vi "Clock.vi"() -> ()   [LabVIEW 2021]
doc: "Clock ver. 1 by 113550153. \nAll right reserved."
uses:
  <vilib>/sound2/lvsound2.llb/Sound Data Format.ctl
  <vilib>/sound2/lvsound2.llb/Sound File Position.ctl
  <vilib>/sound2/lvsound2.llb/Sound Output Write (DBL).vi
  <vilib>/sound2/lvsound2.llb/Sound File Read (DBL).vi
  <vilib>/sound2/lvsound2.llb/Sound File Read Open.vi
panel:
  in  "12/24":bool
  in  "Sample No. x":i32
  out "Sound playing":bool
  in  "Reset button 2":bool
  out "Chronograph":bool
  in  "Notice Content":string
  in  "Voice File":path
  in  "Alarm clock":dbl(knob) scale=0.0..12.0
  in  "Record Button":bool
  in  "GO Button":bool
  in  "Alarm clock mode\nVoice--Screen Notice":bool
  in  "Alarm clock\nOff--On":bool
  in  "Second":i32(knob) scale=0.0..59.0
  in  "Minute":i32(knob) scale=0.0..59.0
  in  "Hour":i32(knob) scale=0.0..23.0
  in  "Reset button":bool
  in  "Mode button":bool
  out "2D Picture":picture
  in  "stop":bool
  # "由於程式稍大，按下開始當下可能會略卡幾秒鐘(Labview啟動)，請見諒~\n使用說明:\n1. Mode Change按鍵: 按下後依次切換顯示的功能 (手錶->時間設定->鬧鐘設定->碼表模式)\n    手錶: 三個指針由長到短分別顯示秒針、分針、時針，第四個短指針則是鬧鐘時間\n    時間設定: 按下Reset後會設定為當下指針所顯示的時間，可用旋鈕調整三個指針\n    鬧鐘設定: 透過旋鈕按鍵調整鬧鐘時間，依照傳統鬧鐘顯示標準(時針制，不分AM/PM)，且\n                    可調整鬧鐘提醒模式、聲音檔案或文字提示內容，可用\"鬧鐘開關\"關閉聲音提醒\n    碼表模式: 按下GO後開始執行，按下Record則會顯示按下當下的秒數 (碼表會繼續跑) (參考\n                    短跑比賽碼表設計)，再按一次則會跳回目前秒數，Reset碼表歸零\n2. 顯示說明(七位顯示器與觀景窗): 依照當前的模式顯示內容\n    手錶: 顯示目前時間\n    時間設定: 顯示目前欲設定的時間\n    鬧鐘設定: 顯示目前欲設定的鬧鐘時間\n    碼表模式: 顯示目前秒數，若按下Record則顯示按下當下的秒數\n    觀景窗: 根據七位顯示器的時間顯示其對應的天色狀況\n3. 可透過按鍵切換24/12時制顯示"
  # "目前模式:"
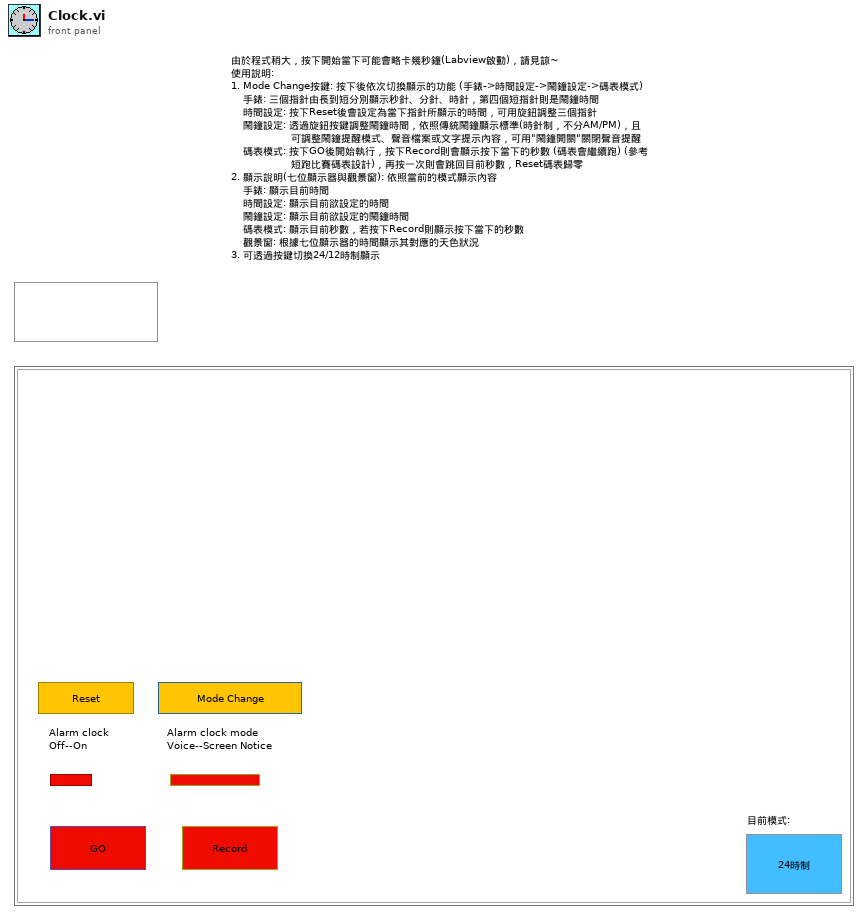
[diagram p1: front panel]
types:
  T1 = cluster{"Width":u16, "Style":enum32{"Solid", "Dash", "Dot", "DashDot", "DashDotDot"}}
  T2 = cluster{"left":i16, "top":i16, "right":i16, "bottom":i16}
  T3 = cluster{"Width":i16, "Style":enum32{"Solid", "Dash", "Dot", "DashDot", "DashDotDot"}}
  T4 = typedef "Sound Data Format.ctl" = cluster{"sample rate (S/s)":dbl, "number of channels":i32, "bits per sample":i32}
  T5 = typedef "Sound Output Task ID.ctl" = u32
  T6 = typedef "LVDateTimeRec.ctl" = cluster{"fractional second":dbl, "second":i32, "minute":i32, "hour":i32, "day of month":i32, "month":i32, "year":i32, "day of week":i32, "day of year":i32, "DST":i32}
  T7 = typedef "Sound File Position.ctl" = u16
  T8 = typedef "Sound File Refnum.ctl" = refnum<file>
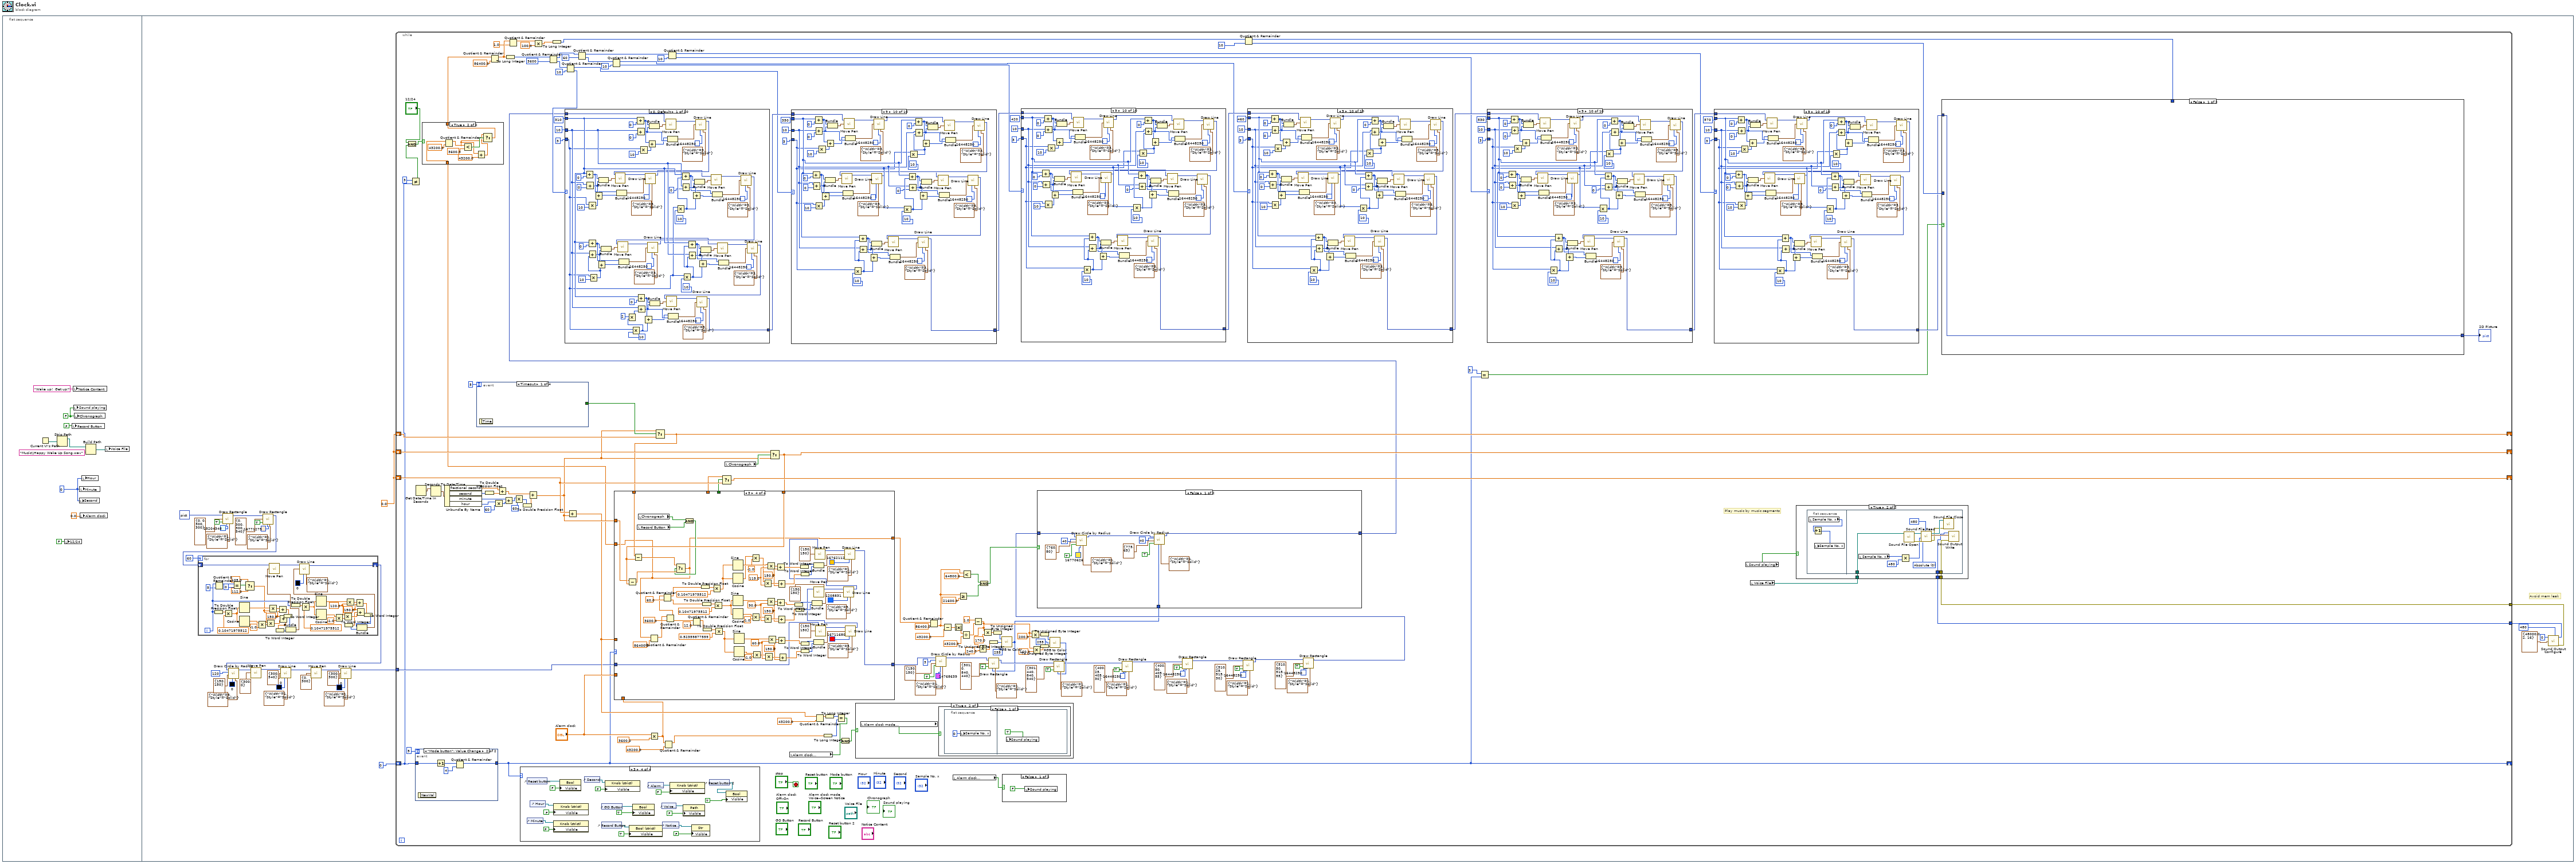
[diagram p0: block diagram]
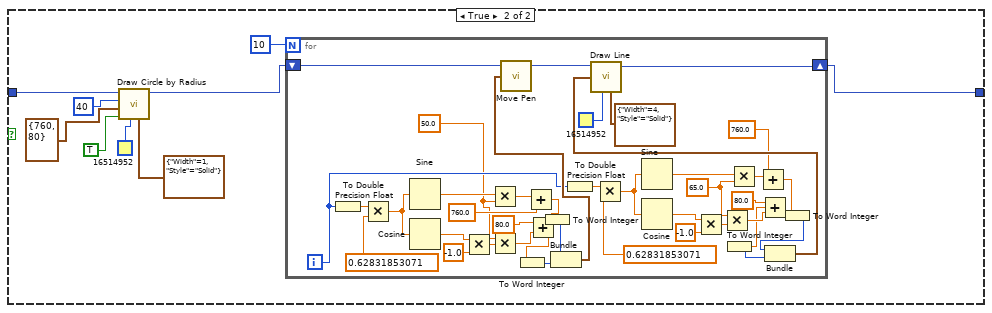
[diagram p2: hidden frame]
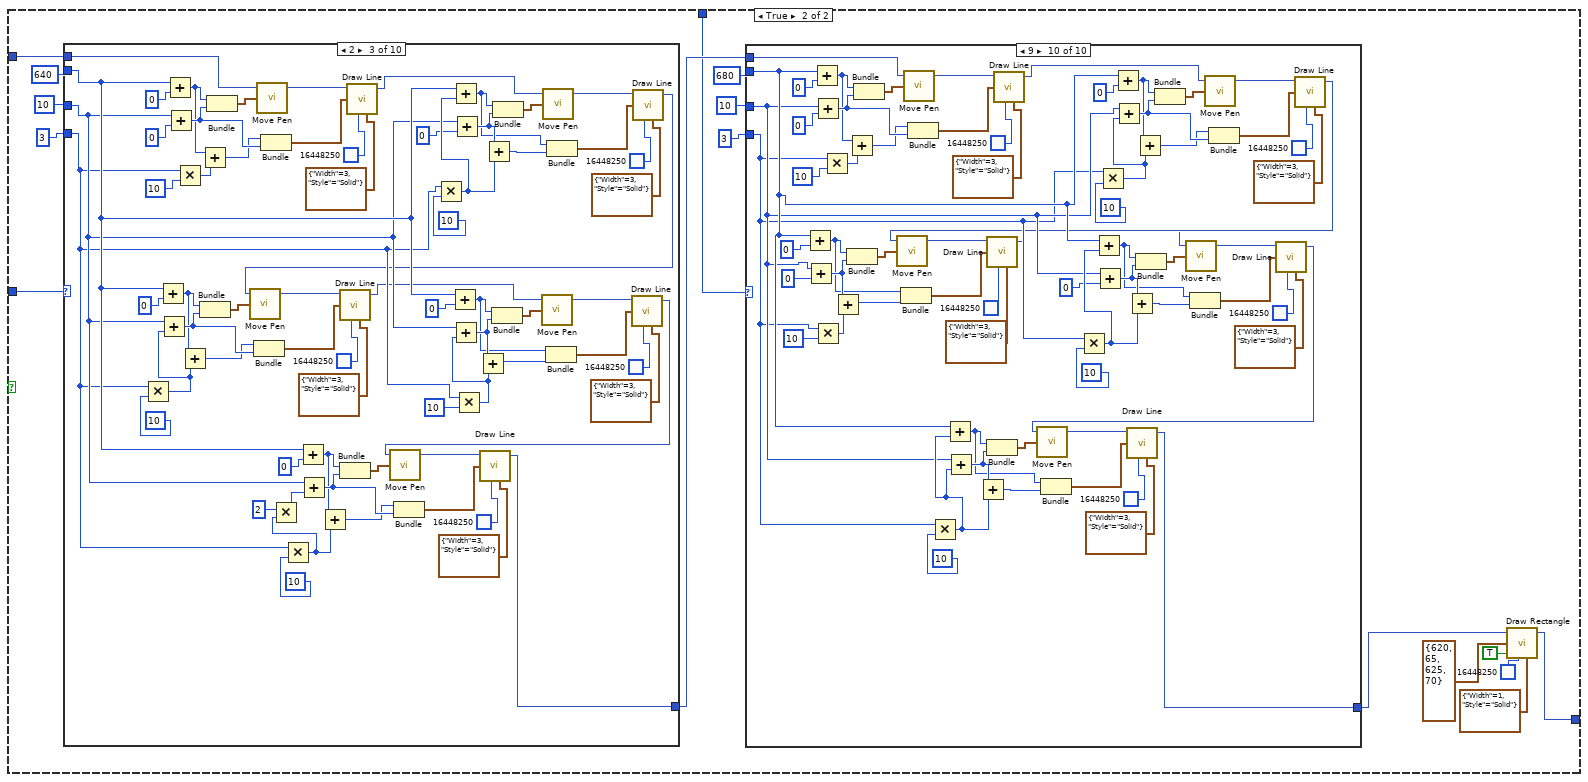
[diagram p4: hidden frame]
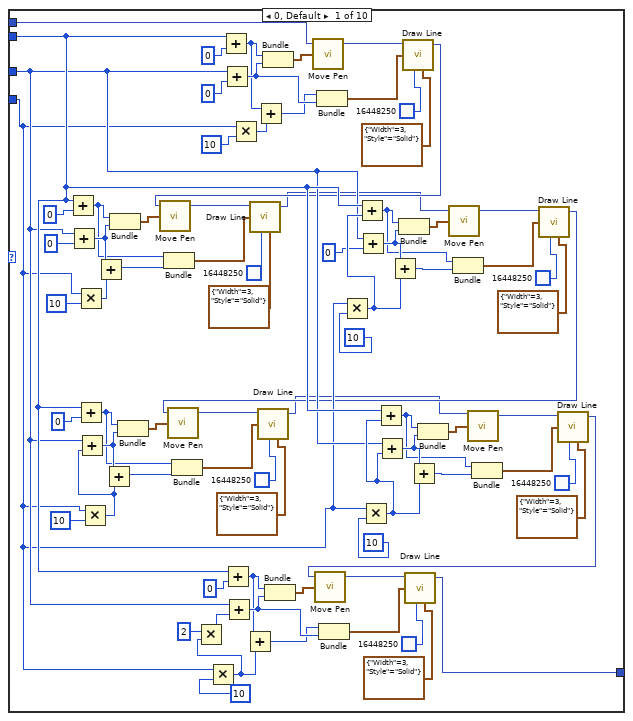
[diagram p5: hidden frame]
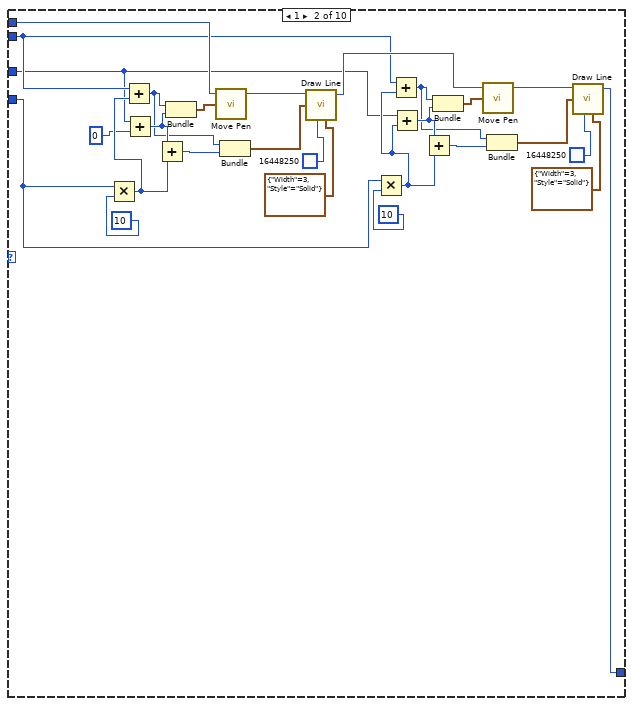
[diagram p6: hidden frame]
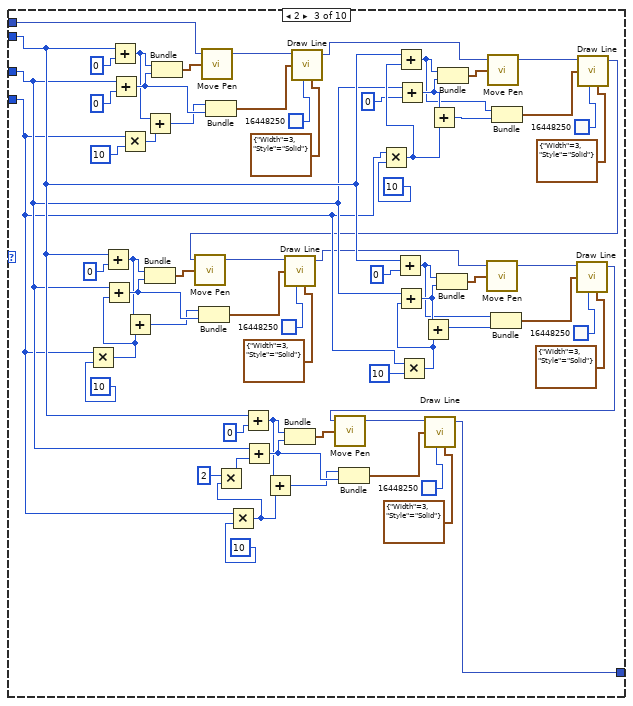
[diagram p7: hidden frame]
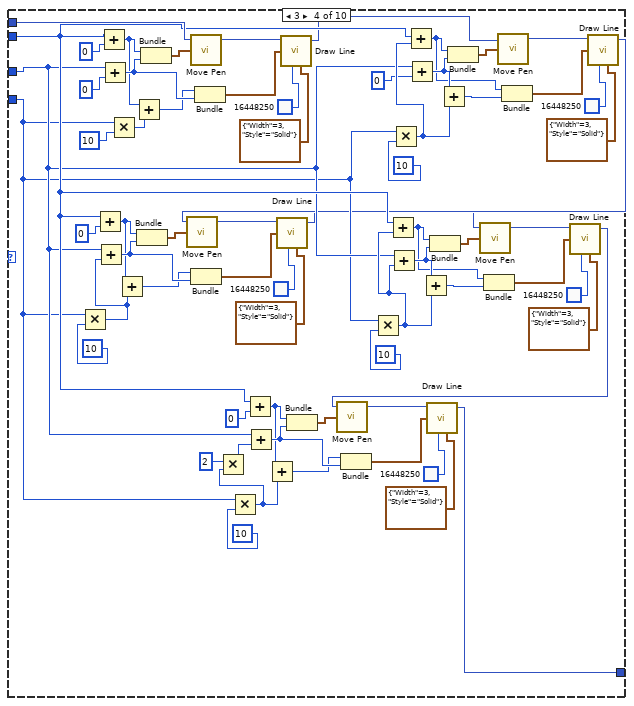
[diagram p8: hidden frame]
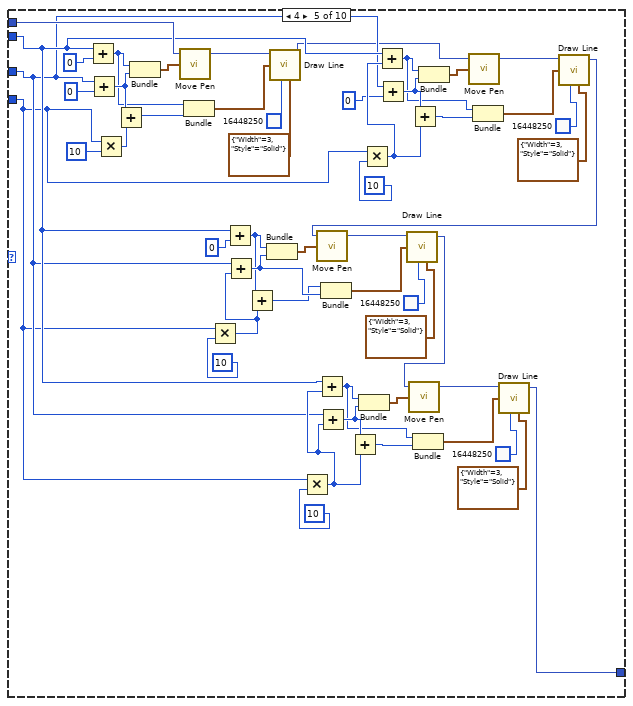
[diagram p9: hidden frame]
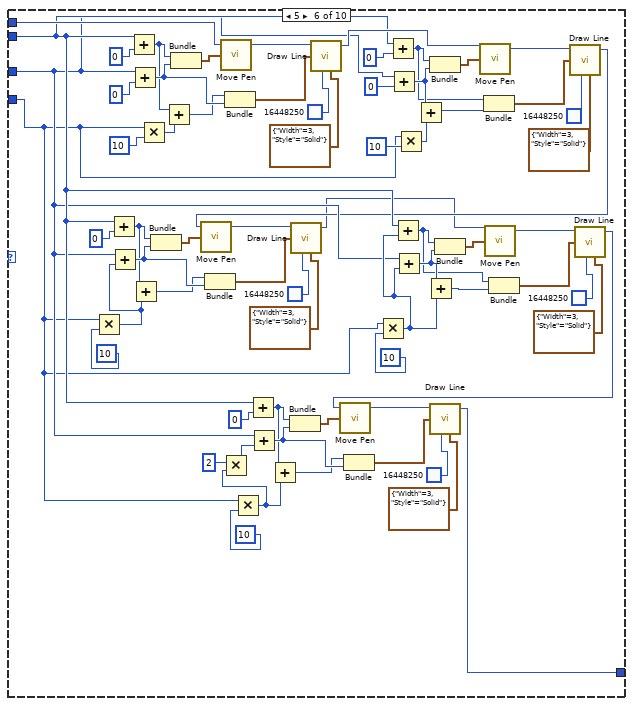
[diagram p10: hidden frame]
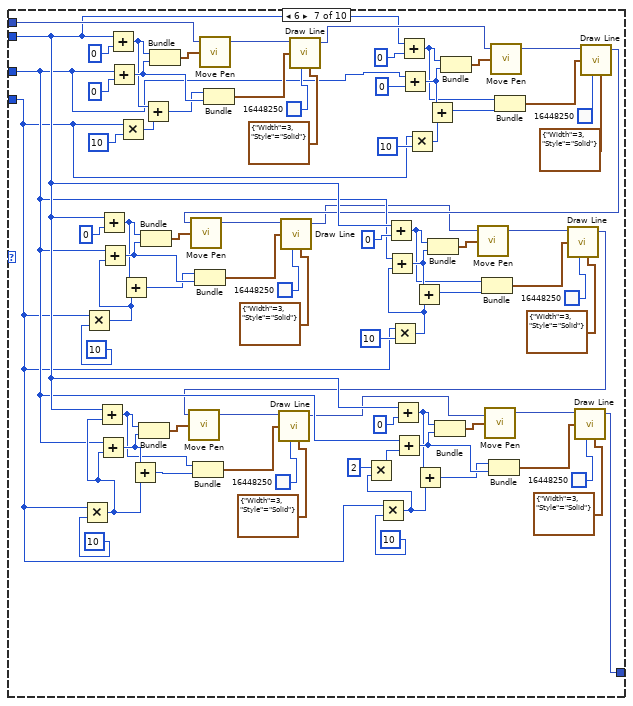
[diagram p11: hidden frame]
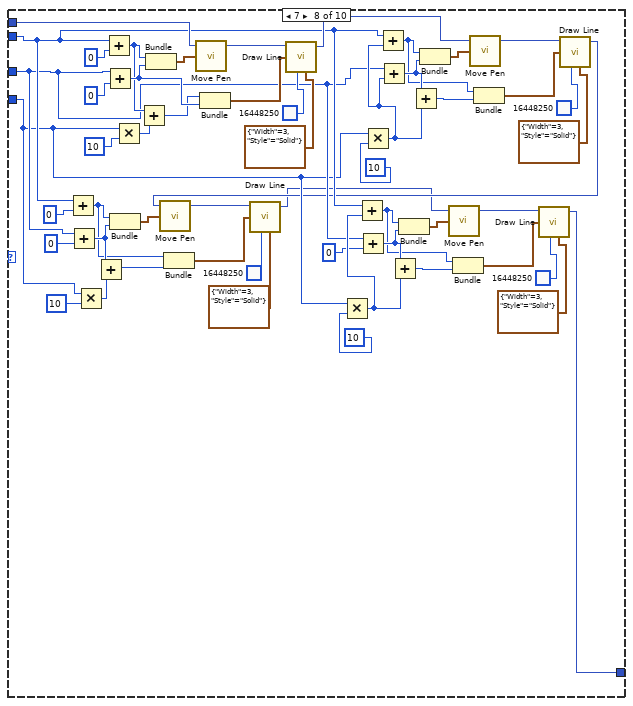
[diagram p12: hidden frame]
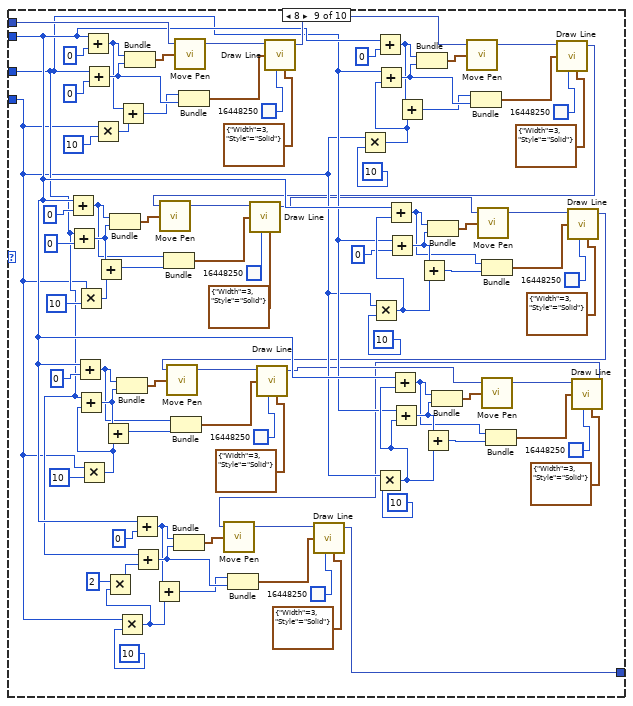
[diagram p13: hidden frame]
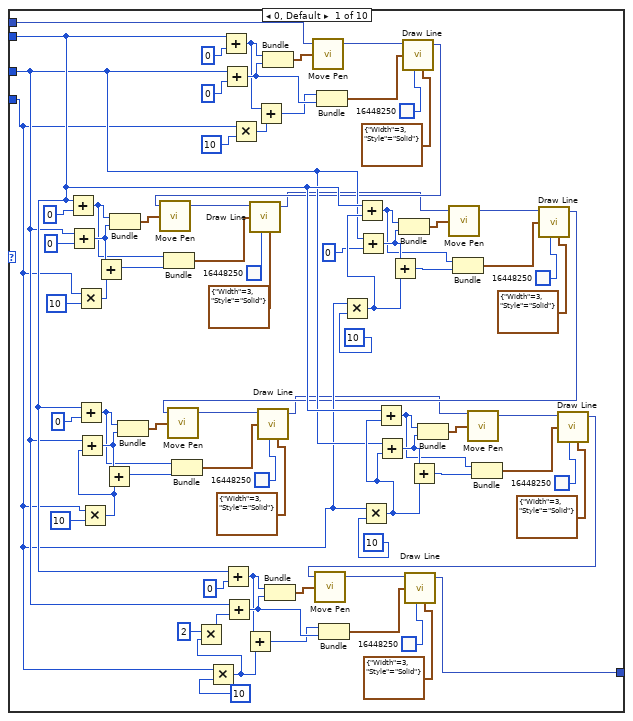
[diagram p14: hidden frame]
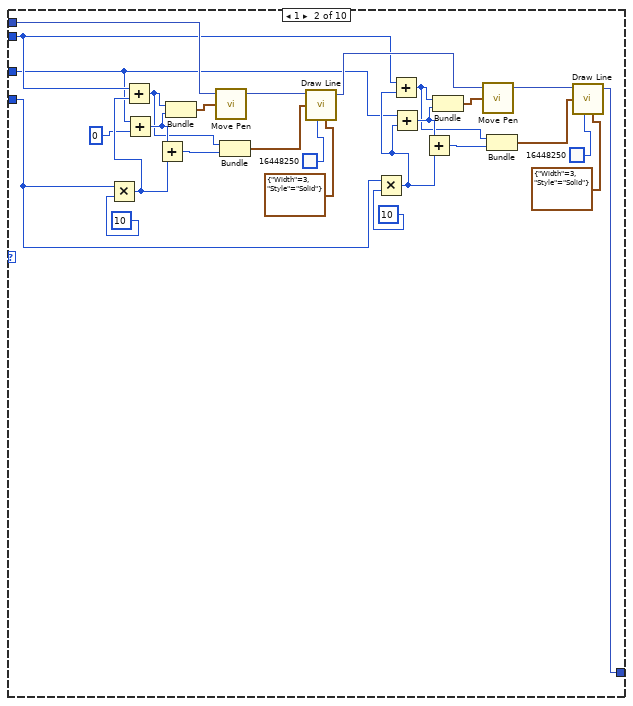
[diagram p15: hidden frame]
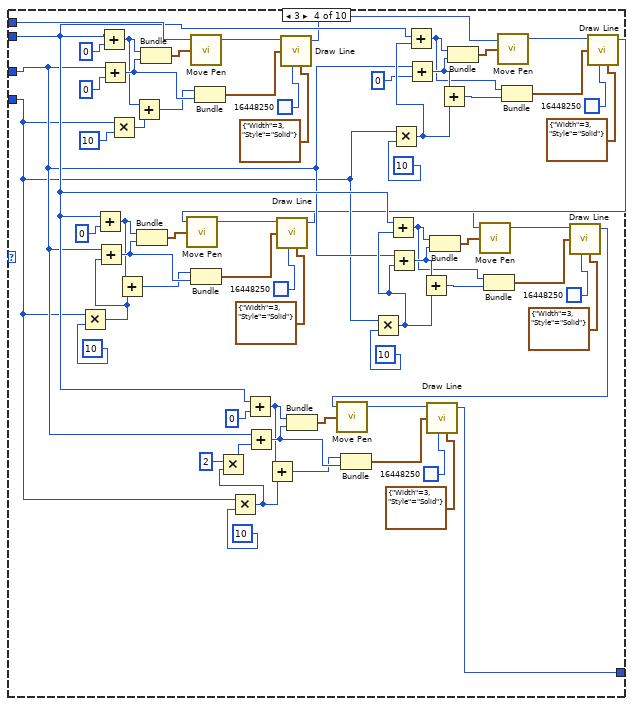
[diagram p16: hidden frame]
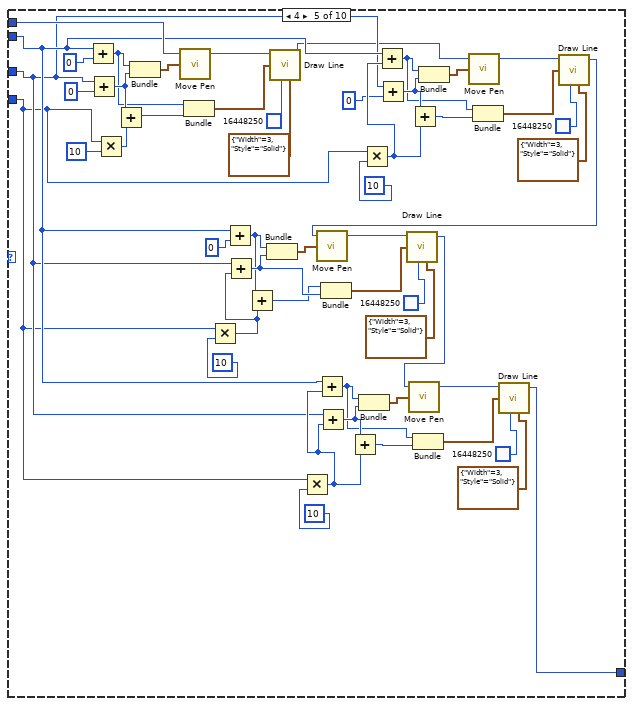
[diagram p17: hidden frame]
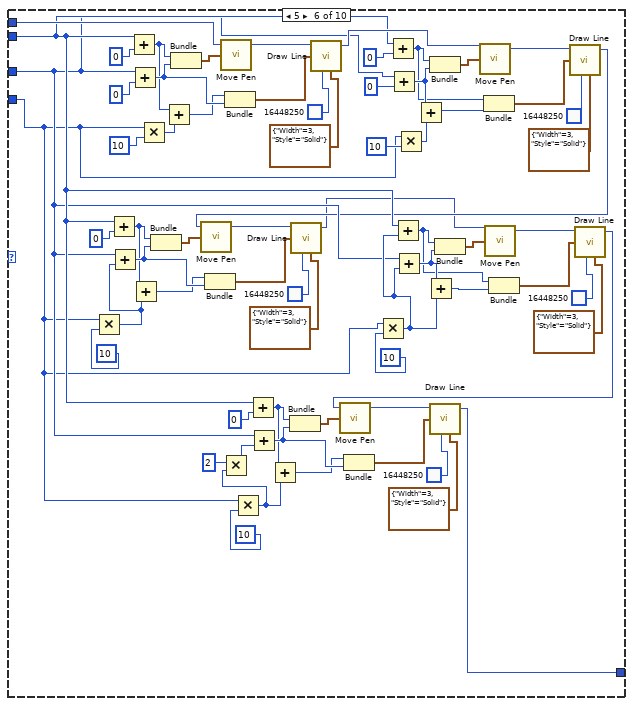
[diagram p18: hidden frame]
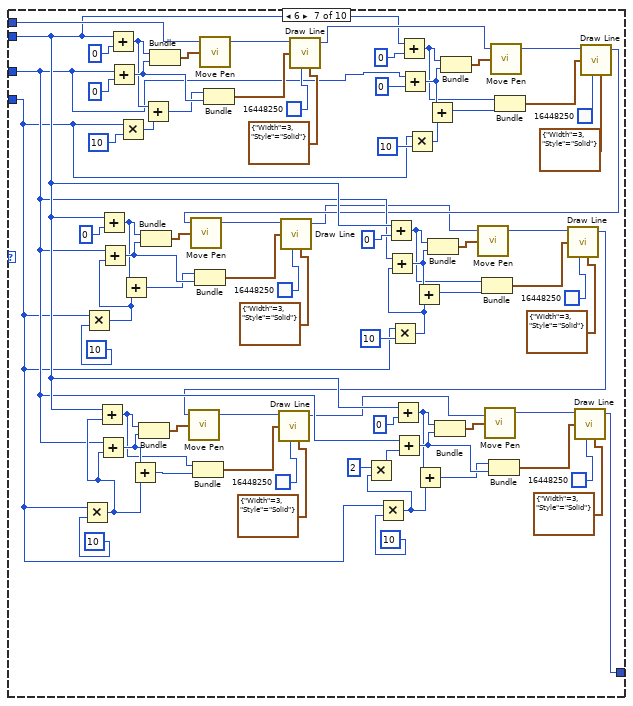
[diagram p19: hidden frame]
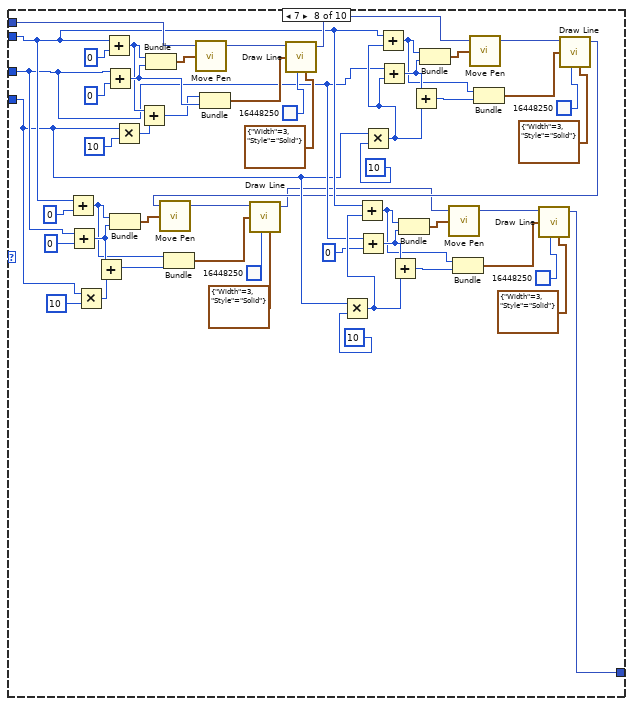
[diagram p20: hidden frame]
diagram:
  n1 = flat-sequence {
    frame #0 {
      w3 = 0
      w10 = FALSE
      n2 = Current VI's Path() -> (path=w8:path)
      n3 = Strip Path(path=w8) -> (stripped path=w7:path)  [unwired: 1 out]
      n4 = local write "12/24"(FALSE ("12/24")) -> ()
      n5 = local write "Record Button"(FALSE ("Record Button")) -> ()
      n6 = local write "Notice Content"("Wake up!  Get up!" ("Notice Content")) -> ()
      n7 = local write "Sound playing"(w10) -> ()
      n8 = local write "Chronograph"(w10) -> ()
      n9 = local write "Second"(w3) -> ()
      n10 = local write "Minute"(w3) -> ()
      n11 = local write "Alarm clock"(0.0 ("Alarm clock")) -> ()
      n12 = local write "Hour"(w3) -> ()
      n13 = Build Path(base path=w7, name or relative path="Music\\Happy Wake Up Song.wav") -> (appended path=w5:path)
      n14 = local write "Voice File"(w5) -> ()
    }
    frame #1 {
      w46 = 0.0
      # "Avoid mem leak"
      n15 = call <vilib>:"Draw Rectangle.vi"("picture"=picture data[5B], "rect"=T2 {"left"=0, "top"=0, "right"=300, "bottom"=300}, "fill?(F)"=TRUE, "color(black)"=u32 15204348, "pen"=T3 {"Width"=1, "Style"=enum."Solid"}) -> ("new picture"=w39:picture)  [unwired: 4 in]
      n16 = call <vilib>:"Draw Rectangle.vi"("picture"=w39, "rect"=T2 {"left"=0, "top"=300, "right"=300, "bottom"=540}, "fill?(F)"=TRUE, "color(black)"=u32 16771279, "pen"=T3 {"Width"=1, "Style"=enum."Solid"}) -> ("new picture"=w40:picture)  [unwired: 4 in]
      n17 = for {
        N: 60 -> [_]
        shift-right: [w65] -> w11
        shift-left: w40 -> [w66]
        i -> [w55]
        w71 = 120.0 ("y")
        w73 = 150.0 ("y")
        w85 = 150.0 ("y")
        n18 = To Double Precision Float(number=w55) -> (double precision float=w82:dbl)
        n19 = Quotient & Remainder(x=w55, y=5) -> (x-y*floor(x/y)=w53:i32)  [unwired: 1 out]
        n20 = Multiply(x=w82, y=0.10471975512) -> (x*y=w91:dbl)
        n21 = Equal?(x=w53, y=0) -> (x = y?=w51:bool)
        n22 = Sine(x=w91) -> (sin(x)=w89:dbl)
        n23 = Cosine(x=w91) -> (cos(x)=w90:dbl)
        n24 = Select(t=105.0, s=w51, f=112.0) -> (s? t:f=w48:dbl)
        n25 = Multiply(x=w90, y=-1.0) -> (x*y=w83:dbl)
        n26 = Multiply(x=w48, y=w83) -> (x*y=w84:dbl)
        n27 = Multiply(x=w89, y=w48) -> (x*y=w88:dbl)
        n28 = Add(x=w88, y=w85) -> (x+y=w68:dbl)
        n29 = Add(x=w85, y=w84) -> (x+y=w67:dbl)
        n30 = To Word Integer(number=w67) -> (16bit integer=w62:i16)
        n31 = To Word Integer(number=w68) -> (16bit integer=w63:i16)
        n32 = Bundle(w63, w62) -> (w64:cluster{i16, i16})  [unwired: 1 in]
        n33 = call <vilib>:"Move Pen.vi"("new position"=w64, "picture"=w66) -> ("new picture"=w81:picture)  [unwired: 3 in]
        n34 = To Double Precision Float(number=w55) -> (double precision float=w69:dbl)
        n35 = Multiply(x=w69, y=0.10471975512) -> (x*y=w78:dbl)
        n36 = Sine(x=w78) -> (sin(x)=w76:dbl)
        n37 = Cosine(x=w78) -> (cos(x)=w77:dbl)
        n38 = Multiply(x=w77, y=-1.0) -> (x*y=w72:dbl)
        n39 = Multiply(x=w71, y=w72) -> (x*y=w74:dbl)
        n40 = Multiply(x=w76, y=w71) -> (x*y=w75:dbl)
        n41 = Add(x=w75, y=w73) -> (x+y=w61:dbl)
        n42 = Add(x=w73, y=w74) -> (x+y=w60:dbl)
        n43 = To Word Integer(number=w60) -> (16bit integer=w58:i16)
        n44 = To Word Integer(number=w61) -> (16bit integer=w59:i16)
        n45 = Bundle(w59, w58) -> (w57:cluster{i16, i16})  [unwired: 1 in]
        n46 = call <vilib>:"Draw Line.vi"("picture"=w81, "end point"=w57, "color(black)"=u32 0, "pen"=T1 {"Width"=1, "Style"=enum."Solid"}) -> ("new picture"=w65:picture)  [unwired: 5 in]
      }
      n47 = call <vilib>:"Draw Circle by Radius.vi"("pen"=T1 {"Width"=3, "Style"=enum."Solid"}, "color(black)"=u32 0, "pixel center"=cluster{"horizontal":i16, "vertical":i16} {"horizontal"=150, "vertical"=150}, "radius"=i16 120, "picture"=w11) -> ("new picture"=w25:picture)  [unwired: 6 in]
      n48 = call <vilib>:"Move Pen.vi"("new position"=cluster{"x":i16, "y":i16} {"x"=300, "y"=0}, "picture"=w25) -> ("new picture"=w26:picture)  [unwired: 3 in]
      n49 = call <vilib>:"Draw Line.vi"("picture"=w26, "end point"=cluster{"x":i16, "y":i16} {"x"=300, "y"=540}, "color(black)"=u32 0, "pen"=T1 {"Width"=1, "Style"=enum."Solid"}) -> ("new picture"=w28:picture)  [unwired: 5 in]
      n50 = call <vilib>:"Move Pen.vi"("new position"=cluster{"x":i16, "y":i16} {"x"=0, "y"=300}, "picture"=w28) -> ("new picture"=w27:picture)  [unwired: 3 in]
      n51 = call <vilib>:"Draw Line.vi"("picture"=w27, "end point"=cluster{"x":i16, "y":i16} {"x"=300, "y"=300}, "color(black)"=u32 0, "pen"=T1 {"Width"=1, "Style"=enum."Solid"}) -> ("new picture"=w12:picture)  [unwired: 5 in]
      n52 = call <vilib>:"Sound Output Configure.vi"("number of samples/ch"=480, "sound format"=T4 {"sample rate (S/s)"=48000.0, "number of channels"=2, "bits per sample"=16}, "device ID"=u32 0) -> ("error out"=w42:errorcluster, "task ID"=w41:T5)  [unwired: 7 in]
      n53 = while {
        shift-right: [w113] -> _
        shift-left: 0 -> [w93]
        shift-right: [w250] -> _
        shift-left: w46 -> [w251]
        shift-right: [w239] -> _
        shift-left: w46 -> [w247]
        shift-right: [w236] -> _
        shift-left: w46 -> [w240]
        tunnel: w42 -> [w220]
        tunnel: w41 -> [w219]
        tunnel: w12 -> [w125]
        stop <- "stop" stop-if-true
        # "Play music by music segments"
        n54 = Not Equal?(x=3, y=w93) -> (x != y?=w94:bool)
        n55 = And(x="12/24", y=w94) -> (x .and. y?=w95:bool)
        n56 = event shown="[1] \"Mode button\": Value Change" {
          selector: _ -> [_ _]
          dyn-events: _ -> [_ _]
          timeout: 5 -> [_ _]
          tunnel: [w6002 w6003] -> w113
          tunnel: w93 -> [w6002 w6006]
          event Timeout {
            n57 = event-data() -> ()  [unwired: 1 in, 1 out]
          }
          event "Mode button": Value Change {
            n58 = event-data() -> ()  [unwired: 1 in, 1 out]
            n59 = Increment(x=w6006) -> (x+1=w6005:i32)
            n60 = Quotient & Remainder(x=w6005, y=4) -> (x-y*floor(x/y)=w6003:i32)  [unwired: 1 out]
          }
        }
        n61 = Get Date/Time In Seconds() -> (seconds since 1Jan1904=w266:timestamp)
        n62 = Seconds To Date/Time(time stamp (now)=w266) -> (date time rec=w264:T6)  [unwired: 1 in]
        n63 = Unbundle By Name(w264) -> ("fractional second"=w243:dbl, "second"=w244:i32, "minute"=w260:i32, "hour"=w263:i32)
        n64 = event shown="[0] Timeout" {
          selector: _ -> [_ _ _ _]
          dyn-events: _ -> [_ _ _ _]
          timeout: 5 -> [_ _ _ _]
          tunnel: [_ _ _ TRUE] -> w237
          event Timeout {
            n65 = event-data() -> ()  [unwired: 1 in, 1 out]
          }
          event "Reset button 2": Value Change {
            w5542 = FALSE
            n66 = event-data() -> ()  [unwired: 1 in, 1 out]
            n67 = local write "Record Button"(w5542) -> ()
            n68 = local write "Chronograph"(w5542) -> ()
          }
          event "GO Button": Value Change {
            n69 = event-data() -> ()  [unwired: 1 in, 1 out]
            n70 = flat-sequence {
              frame #0 {
                n71 = local write "Record Button"(FALSE) -> ()
              }
              frame #1 {
                n72 = local write "Chronograph"(TRUE) -> ()
              }
            }
          }
          event "Record Button": Value Change {
            n73 = event-data() -> ()  [unwired: 1 in, 1 out]
          }
        }
        n74 = To Double Precision Float(number=w244) -> (double precision float=w242:dbl)
        n75 = Multiply(x=w263, y=60) -> (x*y=w261:i32)
        n76 = Add(x=w243, y=w242) -> (x+y=w245:dbl)
        n77 = Add(x=w260, y=w261) -> (x+y=w259:i32)
        n78 = Multiply(x=w259, y=60) -> (x*y=w257:i32)
        n79 = case shown="3" w113 {
          frame 0, Default {
            n80 = control-ref of="Reset button"() -> (w5941:refnum<vi>)
            n81 = control-ref of="Minute"() -> (w5935:refnum<vi>)
            n82 = control-ref of="Hour"() -> (w5938:refnum<vi>)
            n83 = property on="Property Node" class="Knob (strict)"(reference=w5935, "Visible"=FALSE) -> ()  [unwired: 1 in, 2 out]
            n84 = property on="Property Node" class="Knob (strict)"(reference=w5938, "Visible"=FALSE) -> ()  [unwired: 1 in, 2 out]
            n85 = property on="Property Node" class="Bool"(reference=w5941, "Visible"=FALSE) -> ()  [unwired: 1 in, 2 out]
            n86 = control-ref of="Second"() -> (w5934:refnum<vi>)
            n87 = control-ref of="Record Button"() -> (w5930:refnum<vi>)
            n88 = control-ref of="GO Button"() -> (w5932:refnum<vi>)
            n89 = property on="Property Node" class="Knob (strict)"(reference=w5934, "Visible"=FALSE) -> ()  [unwired: 1 in, 2 out]
            n90 = property on="Property Node" class="Bool (strict)"(reference=w5930, "Visible"=FALSE) -> ()  [unwired: 1 in, 2 out]
            n91 = property on="Property Node" class="Bool"(reference=w5932, "Visible"=FALSE) -> ()  [unwired: 1 in, 2 out]
            n92 = control-ref of="Alarm clock"() -> (w5928:refnum<vi>)
            n93 = control-ref of="Voice File"() -> (w5926:refnum<vi>)
            n94 = control-ref of="Notice Content"() -> (w5924:refnum<vi>)
            n95 = property on="Property Node" class="Knob (strict)"(reference=w5928, "Visible"=FALSE) -> ()  [unwired: 1 in, 2 out]
            n96 = property on="Property Node" class="Path"(reference=w5926, "Visible"=FALSE) -> ()  [unwired: 1 in, 2 out]
            n97 = property on="Property Node" class="Str"(reference=w5924, "Visible"=FALSE) -> ()  [unwired: 1 in, 2 out]
            n98 = control-ref of="Reset button 2"() -> (w5922:refnum<vi>)
            n99 = property on="Property Node" class="Bool"(reference=w5922, "Visible"=FALSE) -> ()  [unwired: 1 in, 2 out]
          }
          frame 1 {
            n100 = control-ref of="Reset button"() -> (w5961:refnum<vi>)
            n101 = control-ref of="Minute"() -> (w5955:refnum<vi>)
            n102 = control-ref of="Hour"() -> (w5958:refnum<vi>)
            n103 = property on="Property Node" class="Knob (strict)"(reference=w5955, "Visible"=TRUE) -> ()  [unwired: 1 in, 2 out]
            n104 = property on="Property Node" class="Knob (strict)"(reference=w5958, "Visible"=TRUE) -> ()  [unwired: 1 in, 2 out]
            n105 = property on="Property Node" class="Bool"(reference=w5961, "Visible"=TRUE) -> ()  [unwired: 1 in, 2 out]
            n106 = control-ref of="Second"() -> (w5954:refnum<vi>)
            n107 = control-ref of="Record Button"() -> (w5950:refnum<vi>)
            n108 = control-ref of="GO Button"() -> (w5952:refnum<vi>)
            n109 = property on="Property Node" class="Knob (strict)"(reference=w5954, "Visible"=TRUE) -> ()  [unwired: 1 in, 2 out]
            n110 = property on="Property Node" class="Bool (strict)"(reference=w5950, "Visible"=FALSE) -> ()  [unwired: 1 in, 2 out]
            n111 = property on="Property Node" class="Bool"(reference=w5952, "Visible"=FALSE) -> ()  [unwired: 1 in, 2 out]
            n112 = control-ref of="Alarm clock"() -> (w5948:refnum<vi>)
            n113 = control-ref of="Voice File"() -> (w5946:refnum<vi>)
            n114 = control-ref of="Notice Content"() -> (w5944:refnum<vi>)
            n115 = property on="Property Node" class="Knob (strict)"(reference=w5948, "Visible"=FALSE) -> ()  [unwired: 1 in, 2 out]
            n116 = property on="Property Node" class="Path"(reference=w5946, "Visible"=FALSE) -> ()  [unwired: 1 in, 2 out]
            n117 = property on="Property Node" class="Str"(reference=w5944, "Visible"=FALSE) -> ()  [unwired: 1 in, 2 out]
            n118 = control-ref of="Reset button 2"() -> (w5942:refnum<vi>)
            n119 = property on="Property Node" class="Bool"(reference=w5942, "Visible"=FALSE) -> ()  [unwired: 1 in, 2 out]
          }
          frame 2 {
            n120 = control-ref of="Reset button"() -> (w5981:refnum<vi>)
            n121 = control-ref of="Minute"() -> (w5975:refnum<vi>)
            n122 = control-ref of="Hour"() -> (w5978:refnum<vi>)
            n123 = property on="Property Node" class="Knob (strict)"(reference=w5975, "Visible"=FALSE) -> ()  [unwired: 1 in, 2 out]
            n124 = property on="Property Node" class="Knob (strict)"(reference=w5978, "Visible"=FALSE) -> ()  [unwired: 1 in, 2 out]
            n125 = property on="Property Node" class="Bool"(reference=w5981, "Visible"=FALSE) -> ()  [unwired: 1 in, 2 out]
            n126 = control-ref of="Second"() -> (w5974:refnum<vi>)
            n127 = control-ref of="Record Button"() -> (w5970:refnum<vi>)
            n128 = control-ref of="GO Button"() -> (w5972:refnum<vi>)
            n129 = property on="Property Node" class="Knob (strict)"(reference=w5974, "Visible"=FALSE) -> ()  [unwired: 1 in, 2 out]
            n130 = property on="Property Node" class="Bool (strict)"(reference=w5970, "Visible"=FALSE) -> ()  [unwired: 1 in, 2 out]
            n131 = property on="Property Node" class="Bool"(reference=w5972, "Visible"=FALSE) -> ()  [unwired: 1 in, 2 out]
            n132 = control-ref of="Alarm clock"() -> (w5968:refnum<vi>)
            n133 = control-ref of="Voice File"() -> (w5966:refnum<vi>)
            n134 = control-ref of="Notice Content"() -> (w5964:refnum<vi>)
            n135 = property on="Property Node" class="Knob (strict)"(reference=w5968, "Visible"=TRUE) -> ()  [unwired: 1 in, 2 out]
            n136 = property on="Property Node" class="Path"(reference=w5966, "Visible"=TRUE) -> ()  [unwired: 1 in, 2 out]
            n137 = property on="Property Node" class="Str"(reference=w5964, "Visible"=TRUE) -> ()  [unwired: 1 in, 2 out]
            n138 = control-ref of="Reset button 2"() -> (w5962:refnum<vi>)
            n139 = property on="Property Node" class="Bool"(reference=w5962, "Visible"=FALSE) -> ()  [unwired: 1 in, 2 out]
          }
          frame 3 {
            n140 = control-ref of="Reset button"() -> (w6001:refnum<vi>)
            n141 = control-ref of="Minute"() -> (w5995:refnum<vi>)
            n142 = control-ref of="Hour"() -> (w5998:refnum<vi>)
            n143 = property on="Property Node" class="Knob (strict)"(reference=w5995, "Visible"=FALSE) -> ()  [unwired: 1 in, 2 out]
            n144 = property on="Property Node" class="Knob (strict)"(reference=w5998, "Visible"=FALSE) -> ()  [unwired: 1 in, 2 out]
            n145 = property on="Property Node" class="Bool"(reference=w6001, "Visible"=FALSE) -> ()  [unwired: 1 in, 2 out]
            n146 = control-ref of="Second"() -> (w5994:refnum<vi>)
            n147 = control-ref of="Record Button"() -> (w5990:refnum<vi>)
            n148 = control-ref of="GO Button"() -> (w5992:refnum<vi>)
            n149 = property on="Property Node" class="Knob (strict)"(reference=w5994, "Visible"=FALSE) -> ()  [unwired: 1 in, 2 out]
            n150 = property on="Property Node" class="Bool (strict)"(reference=w5990, "Visible"=TRUE) -> ()  [unwired: 1 in, 2 out]
            n151 = property on="Property Node" class="Bool"(reference=w5992, "Visible"=TRUE) -> ()  [unwired: 1 in, 2 out]
            n152 = control-ref of="Alarm clock"() -> (w5988:refnum<vi>)
            n153 = control-ref of="Voice File"() -> (w5986:refnum<vi>)
            n154 = control-ref of="Notice Content"() -> (w5984:refnum<vi>)
            n155 = property on="Property Node" class="Knob (strict)"(reference=w5988, "Visible"=FALSE) -> ()  [unwired: 1 in, 2 out]
            n156 = property on="Property Node" class="Path"(reference=w5986, "Visible"=FALSE) -> ()  [unwired: 1 in, 2 out]
            n157 = property on="Property Node" class="Str"(reference=w5984, "Visible"=FALSE) -> ()  [unwired: 1 in, 2 out]
            n158 = control-ref of="Reset button 2"() -> (w5982:refnum<vi>)
            n159 = property on="Property Node" class="Bool"(reference=w5982, "Visible"=TRUE) -> ()  [unwired: 1 in, 2 out]
          }
        }
        n160 = To Double Precision Float(number=w257) -> (double precision float=w241:dbl)
        n161 = Add(x=w245, y=w241) -> (x+y=w183:dbl)
        n162 = Add(x=w251, y=w183) -> (x+y=w162:dbl)
        n163 = Multiply(x="Alarm clock", y=3600.0) -> (x*y=w108:dbl)
        n164 = Select(t=w183, s=w237, f=w240) -> (s? t:f=w236:dbl)
        n165 = Quotient & Remainder(x=w108, y=43200.0) -> (x-y*floor(x/y)=w110:dbl)  [unwired: 1 out]
        n166 = local read "Chronograph"() -> (w246:bool)
        n167 = Select(t=w247, s=w246, f=w183) -> (s? t:f=w239:dbl)
        n168 = case shown="3" w113 {
          tunnel: w125 -> [w5554 w5651 w5748 w5850]
          tunnel: [w5553 w5650 w5749 w5851] -> w224
          tunnel: w162 -> [w5551 w5648 _ _]
          tunnel: "Alarm clock" -> [w5581 w5678 _ _]
          tunnel: [_ _ w5750 _] -> w249
          tunnel: w183 -> [_ _ w5752 w5840]
          tunnel: [_ _ w5751 _] -> w248
          tunnel: w239 -> [_ _ _ w5846]
          tunnel: w236 -> [_ _ _ w5845]
          tunnel: [w5551 w5647 w5744 w5839] -> w106
          tunnel: w108 -> [_ w5647 _ _]
          tunnel: [w5551 w5647 w5744 w5839] -> w109
          frame 0, Default {
            w5592 = 40.0 ("y")
            w5591 = 150.0 ("y")
            w5620 = 60.0 ("y")
            w5619 = 150.0 ("y")
            w5631 = 90.0 ("y")
            w5630 = 150.0 ("y")
            w5635 = 115.0 ("y")
            w5634 = 150.0 ("y")
            n169 = Quotient & Remainder(x=w5551, y=86400.0) -> (x-y*floor(x/y)=w5642:dbl)  [unwired: 1 out]
            n170 = Multiply(x=w5581, y=0.52359877559) -> (x*y=w5582:dbl)
            n171 = Quotient & Remainder(x=w5642, y=3600.0) -> (x-y*floor(x/y)=w5643:dbl, floor(x/y)=w5628:dbl)
            n172 = Quotient & Remainder(x=w5643, y=60.0) -> (x-y*floor(x/y)=w5623:dbl, floor(x/y)=w5624:dbl)
            n173 = Sine(x=w5582) -> (sin(x)=w5560:dbl)
            n174 = Cosine(x=w5582) -> (cos(x)=w5557:dbl)
            n175 = Multiply(x=w5557, y=-1.0) -> (x*y=w5558:dbl)
            n176 = Quotient & Remainder(x=w5628, y=12.0) -> (x-y*floor(x/y)=w5627:dbl)  [unwired: 1 out]
            n177 = To Double Precision Float(number=w5623) -> (double precision float=w5625:dbl)
            n178 = Multiply(x=w5558, y=w5592) -> (x*y=w5593:dbl)
            n179 = To Double Precision Float(number=w5624) -> (double precision float=w5638:dbl)
            n180 = To Double Precision Float(number=w5627) -> (double precision float=w5640:dbl)
            n181 = Multiply(x=w5560, y=w5592) -> (x*y=w5594:dbl)
            n182 = Multiply(x=w5625, y=0.10471975512) -> (x*y=w5618:dbl)
            n183 = Multiply(x=w5638, y=0.10471975512) -> (x*y=w5617:dbl)
            n184 = Multiply(x=w5640, y=0.52359877559) -> (x*y=w5616:dbl)
            n185 = Add(x=w5594, y=w5591) -> (x+y=w5574:dbl)
            n186 = Add(x=w5593, y=w5591) -> (x+y=w5573:dbl)
            n187 = To Word Integer(number=w5574) -> (16bit integer=w5586:i16)
            n188 = To Word Integer(number=w5573) -> (16bit integer=w5585:i16)
            n189 = Sine(x=w5618) -> (sin(x)=w5572:dbl)
            n190 = Cosine(x=w5618) -> (cos(x)=w5570:dbl)
            n191 = Sine(x=w5617) -> (sin(x)=w5568:dbl)
            n192 = Cosine(x=w5617) -> (cos(x)=w5565:dbl)
            n193 = Sine(x=w5616) -> (sin(x)=w5564:dbl)
            n194 = Cosine(x=w5616) -> (cos(x)=w5562:dbl)
            n195 = Bundle(w5586, w5585) -> (w5584:cluster{i16, i16})  [unwired: 1 in]
            n196 = Multiply(x=w5570, y=-1.0) -> (x*y=w5569:dbl)
            n197 = Multiply(x=w5565, y=-1.0) -> (x*y=w5566:dbl)
            n198 = Multiply(x=w5562, y=-1.0) -> (x*y=w5561:dbl)
            n199 = Multiply(x=w5569, y=w5635) -> (x*y=w5636:dbl)
            n200 = Multiply(x=w5566, y=w5631) -> (x*y=w5632:dbl)
            n201 = Multiply(x=w5561, y=w5620) -> (x*y=w5621:dbl)
            n202 = Multiply(x=w5572, y=w5635) -> (x*y=w5637:dbl)
            n203 = Multiply(x=w5568, y=w5631) -> (x*y=w5633:dbl)
            n204 = Multiply(x=w5564, y=w5620) -> (x*y=w5622:dbl)
            n205 = Add(x=w5637, y=w5634) -> (x+y=w5580:dbl)
            n206 = Add(x=w5633, y=w5630) -> (x+y=w5578:dbl)
            n207 = Add(x=w5636, y=w5634) -> (x+y=w5579:dbl)
            n208 = Add(x=w5632, y=w5630) -> (x+y=w5577:dbl)
            n209 = Add(x=w5622, y=w5619) -> (x+y=w5576:dbl)
            n210 = Add(x=w5621, y=w5619) -> (x+y=w5575:dbl)
            n211 = To Word Integer(number=w5578) -> (16bit integer=w5604:i16)
            n212 = To Word Integer(number=w5577) -> (16bit integer=w5603:i16)
            n213 = To Word Integer(number=w5580) -> (16bit integer=w5611:i16)
            n214 = To Word Integer(number=w5579) -> (16bit integer=w5610:i16)
            n215 = To Word Integer(number=w5576) -> (16bit integer=w5597:i16)
            n216 = To Word Integer(number=w5575) -> (16bit integer=w5596:i16)
            n217 = Bundle(w5604, w5603) -> (w5602:cluster{i16, i16})  [unwired: 1 in]
            n218 = Bundle(w5611, w5610) -> (w5609:cluster{i16, i16})  [unwired: 1 in]
            n219 = Bundle(w5597, w5596) -> (w5595:cluster{i16, i16})  [unwired: 1 in]
            n220 = call <vilib>:"Move Pen.vi"("new position"=cluster{"x":i16, "y":i16} {"x"=150, "y"=150}, "picture"=w5554) -> ("new picture"=w5599:picture)  [unwired: 3 in]
            n221 = call <vilib>:"Draw Line.vi"("picture"=w5599, "end point"=w5595, "color(black)"=u32 16711680, "pen"=T1 {"Width"=5, "Style"=enum."Solid"}) -> ("new picture"=w5556:picture)  [unwired: 5 in]
            n222 = call <vilib>:"Move Pen.vi"("new position"=cluster{"x":i16, "y":i16} {"x"=150, "y"=150}, "picture"=w5556) -> ("new picture"=w5606:picture)  [unwired: 3 in]
            n223 = call <vilib>:"Draw Line.vi"("picture"=w5606, "end point"=w5602, "color(black)"=u32 1208831, "pen"=T1 {"Width"=3, "Style"=enum."Solid"}) -> ("new picture"=w5555:picture)  [unwired: 5 in]
            n224 = call <vilib>:"Move Pen.vi"("new position"=cluster{"x":i16, "y":i16} {"x"=150, "y"=150}, "picture"=w5555) -> ("new picture"=w5613:picture)  [unwired: 3 in]
            n225 = call <vilib>:"Draw Line.vi"("picture"=w5613, "end point"=w5609, "color(black)"=u32 16762112, "pen"=T1 {"Width"=1, "Style"=enum."Solid"}) -> ("new picture"=w5552:picture)  [unwired: 5 in]
            n226 = call <vilib>:"Move Pen.vi"("new position"=cluster{"x":i16, "y":i16} {"x"=150, "y"=150}, "picture"=w5552) -> ("new picture"=w5588:picture)  [unwired: 3 in]
            n227 = call <vilib>:"Draw Line.vi"("picture"=w5588, "end point"=w5584, "color(black)"=u32 16318208, "pen"=T1 {"Width"=2, "Style"=enum."Solid"}) -> ("new picture"=w5553:picture)  [unwired: 5 in]
          }
          frame 2 {
            w5689 = 40.0 ("y")
            w5688 = 150.0 ("y")
            w5717 = 60.0 ("y")
            w5716 = 150.0 ("y")
            w5728 = 90.0 ("y")
            w5727 = 150.0 ("y")
            w5732 = 115.0 ("y")
            w5731 = 150.0 ("y")
            n228 = Quotient & Remainder(x=w5648, y=86400.0) -> (x-y*floor(x/y)=w5739:dbl)  [unwired: 1 out]
            n229 = Multiply(x=w5678, y=0.52359877559) -> (x*y=w5679:dbl)
            n230 = Quotient & Remainder(x=w5739, y=3600.0) -> (x-y*floor(x/y)=w5740:dbl, floor(x/y)=w5725:dbl)
            n231 = Quotient & Remainder(x=w5740, y=60.0) -> (x-y*floor(x/y)=w5720:dbl, floor(x/y)=w5721:dbl)
            n232 = Sine(x=w5679) -> (sin(x)=w5657:dbl)
            n233 = Cosine(x=w5679) -> (cos(x)=w5654:dbl)
            n234 = Multiply(x=w5654, y=-1.0) -> (x*y=w5655:dbl)
            n235 = Quotient & Remainder(x=w5725, y=12.0) -> (x-y*floor(x/y)=w5724:dbl)  [unwired: 1 out]
            n236 = To Double Precision Float(number=w5720) -> (double precision float=w5722:dbl)
            n237 = Multiply(x=w5655, y=w5689) -> (x*y=w5690:dbl)
            n238 = To Double Precision Float(number=w5721) -> (double precision float=w5735:dbl)
            n239 = To Double Precision Float(number=w5724) -> (double precision float=w5737:dbl)
            n240 = Multiply(x=w5657, y=w5689) -> (x*y=w5691:dbl)
            n241 = Multiply(x=w5722, y=0.10471975512) -> (x*y=w5715:dbl)
            n242 = Multiply(x=w5735, y=0.10471975512) -> (x*y=w5714:dbl)
            n243 = Multiply(x=w5737, y=0.52359877559) -> (x*y=w5713:dbl)
            n244 = Add(x=w5691, y=w5688) -> (x+y=w5671:dbl)
            n245 = Add(x=w5690, y=w5688) -> (x+y=w5670:dbl)
            n246 = To Word Integer(number=w5671) -> (16bit integer=w5683:i16)
            n247 = To Word Integer(number=w5670) -> (16bit integer=w5682:i16)
            n248 = Sine(x=w5715) -> (sin(x)=w5669:dbl)
            n249 = Cosine(x=w5715) -> (cos(x)=w5667:dbl)
            n250 = Sine(x=w5714) -> (sin(x)=w5665:dbl)
            n251 = Cosine(x=w5714) -> (cos(x)=w5662:dbl)
            n252 = Sine(x=w5713) -> (sin(x)=w5661:dbl)
            n253 = Cosine(x=w5713) -> (cos(x)=w5659:dbl)
            n254 = Bundle(w5683, w5682) -> (w5681:cluster{i16, i16})  [unwired: 1 in]
            n255 = Multiply(x=w5667, y=-1.0) -> (x*y=w5666:dbl)
            n256 = Multiply(x=w5662, y=-1.0) -> (x*y=w5663:dbl)
            n257 = Multiply(x=w5659, y=-1.0) -> (x*y=w5658:dbl)
            n258 = Multiply(x=w5666, y=w5732) -> (x*y=w5733:dbl)
            n259 = Multiply(x=w5663, y=w5728) -> (x*y=w5729:dbl)
            n260 = Multiply(x=w5658, y=w5717) -> (x*y=w5718:dbl)
            n261 = Multiply(x=w5669, y=w5732) -> (x*y=w5734:dbl)
            n262 = Multiply(x=w5665, y=w5728) -> (x*y=w5730:dbl)
            n263 = Multiply(x=w5661, y=w5717) -> (x*y=w5719:dbl)
            n264 = Add(x=w5734, y=w5731) -> (x+y=w5677:dbl)
            n265 = Add(x=w5730, y=w5727) -> (x+y=w5675:dbl)
            n266 = Add(x=w5733, y=w5731) -> (x+y=w5676:dbl)
            n267 = Add(x=w5729, y=w5727) -> (x+y=w5674:dbl)
            n268 = Add(x=w5719, y=w5716) -> (x+y=w5673:dbl)
            n269 = Add(x=w5718, y=w5716) -> (x+y=w5672:dbl)
            n270 = To Word Integer(number=w5675) -> (16bit integer=w5701:i16)
            n271 = To Word Integer(number=w5674) -> (16bit integer=w5700:i16)
            n272 = To Word Integer(number=w5677) -> (16bit integer=w5708:i16)
            n273 = To Word Integer(number=w5676) -> (16bit integer=w5707:i16)
            n274 = To Word Integer(number=w5673) -> (16bit integer=w5694:i16)
            n275 = To Word Integer(number=w5672) -> (16bit integer=w5693:i16)
            n276 = Bundle(w5701, w5700) -> (w5699:cluster{i16, i16})  [unwired: 1 in]
            n277 = Bundle(w5708, w5707) -> (w5706:cluster{i16, i16})  [unwired: 1 in]
            n278 = Bundle(w5694, w5693) -> (w5692:cluster{i16, i16})  [unwired: 1 in]
            n279 = call <vilib>:"Move Pen.vi"("new position"=cluster{"x":i16, "y":i16} {"x"=150, "y"=150}, "picture"=w5651) -> ("new picture"=w5696:picture)  [unwired: 3 in]
            n280 = call <vilib>:"Draw Line.vi"("picture"=w5696, "end point"=w5692, "color(black)"=u32 16711680, "pen"=T1 {"Width"=5, "Style"=enum."Solid"}) -> ("new picture"=w5653:picture)  [unwired: 5 in]
            n281 = call <vilib>:"Move Pen.vi"("new position"=cluster{"x":i16, "y":i16} {"x"=150, "y"=150}, "picture"=w5653) -> ("new picture"=w5703:picture)  [unwired: 3 in]
            n282 = call <vilib>:"Draw Line.vi"("picture"=w5703, "end point"=w5699, "color(black)"=u32 1208831, "pen"=T1 {"Width"=3, "Style"=enum."Solid"}) -> ("new picture"=w5652:picture)  [unwired: 5 in]
            n283 = call <vilib>:"Move Pen.vi"("new position"=cluster{"x":i16, "y":i16} {"x"=150, "y"=150}, "picture"=w5652) -> ("new picture"=w5710:picture)  [unwired: 3 in]
            n284 = call <vilib>:"Draw Line.vi"("picture"=w5710, "end point"=w5706, "color(black)"=u32 16762112, "pen"=T1 {"Width"=1, "Style"=enum."Solid"}) -> ("new picture"=w5649:picture)  [unwired: 5 in]
            n285 = call <vilib>:"Move Pen.vi"("new position"=cluster{"x":i16, "y":i16} {"x"=150, "y"=150}, "picture"=w5649) -> ("new picture"=w5685:picture)  [unwired: 3 in]
            n286 = call <vilib>:"Draw Line.vi"("picture"=w5685, "end point"=w5681, "color(black)"=u32 16318208, "pen"=T1 {"Width"=2, "Style"=enum."Solid"}) -> ("new picture"=w5650:picture)  [unwired: 5 in]
          }
          frame 1 {
            w5805 = 60.0 ("y")
            w5804 = 150.0 ("y")
            w5816 = 90.0 ("y")
            w5815 = 150.0 ("y")
            w5820 = 115.0 ("y")
            w5819 = 150.0 ("y")
            n287 = local read "Hour"() -> (w5756:i32)
            n288 = local read "Minute"() -> (w5755:i32)
            n289 = Multiply(x=w5756, y=60) -> (x*y=w5759:i32)
            n290 = local read "Second"() -> (w5754:i32)
            n291 = Add(x=w5755, y=w5759) -> (x+y=w5760:i32)
            n292 = Multiply(x=w5760, y=60) -> (x*y=w5761:i32)
            n293 = Add(x=w5754, y=w5761) -> (x+y=w5745:i32)
            n294 = To Double Precision Float(number=w5745) -> (double precision float=w5744:dbl)
            n295 = event shown="[1] \"Reset button\": Value Change" {
              selector: _ -> [_ _]
              dyn-events: _ -> [_ _]
              timeout: 3 -> [_ _]
              tunnel: w5745 -> [_ w5838]
              tunnel: w5752 -> [_ w5837]
              tunnel: [_ w5834] -> w5751
              tunnel: [_ TRUE ("s")] -> w5750
              event Timeout {
                n296 = event-data() -> ()  [unwired: 1 in, 1 out]
              }
              event "Reset button": Value Change {
                n297 = event-data() -> ()  [unwired: 1 in, 1 out]
                n298 = To Double Precision Float(number=w5838) -> (double precision float=w5832:dbl)
                n299 = Subtract(x=w5832, y=w5837) -> (x-y=w5835:dbl)
                n300 = Add(x=86400.0, y=w5835) -> (x+y=w5834:dbl)
              }
            }
            n301 = Quotient & Remainder(x=w5745, y=86400) -> (x-y*floor(x/y)=w5827:i32)  [unwired: 1 out]
            n302 = Quotient & Remainder(x=w5827, y=3600) -> (x-y*floor(x/y)=w5828:i32, floor(x/y)=w5813:i32)
            n303 = Quotient & Remainder(x=w5828, y=60) -> (x-y*floor(x/y)=w5808:i32, floor(x/y)=w5809:i32)
            n304 = Quotient & Remainder(x=w5813, y=12) -> (x-y*floor(x/y)=w5812:i32)  [unwired: 1 out]
            n305 = To Double Precision Float(number=w5808) -> (double precision float=w5810:dbl)
            n306 = To Double Precision Float(number=w5809) -> (double precision float=w5823:dbl)
            n307 = To Double Precision Float(number=w5812) -> (double precision float=w5825:dbl)
            n308 = Multiply(x=w5810, y=0.10471975512) -> (x*y=w5803:dbl)
            n309 = Multiply(x=w5823, y=0.10471975512) -> (x*y=w5802:dbl)
            n310 = Multiply(x=w5825, y=0.52359877559) -> (x*y=w5801:dbl)
            n311 = Sine(x=w5803) -> (sin(x)=w5773:dbl)
            n312 = Cosine(x=w5803) -> (cos(x)=w5771:dbl)
            n313 = Sine(x=w5802) -> (sin(x)=w5769:dbl)
            n314 = Cosine(x=w5802) -> (cos(x)=w5766:dbl)
            n315 = Sine(x=w5801) -> (sin(x)=w5765:dbl)
            n316 = Cosine(x=w5801) -> (cos(x)=w5763:dbl)
            n317 = Multiply(x=w5771, y=-1.0) -> (x*y=w5770:dbl)
            n318 = Multiply(x=w5766, y=-1.0) -> (x*y=w5767:dbl)
            n319 = Multiply(x=w5763, y=-1.0) -> (x*y=w5762:dbl)
            n320 = Multiply(x=w5770, y=w5820) -> (x*y=w5821:dbl)
            n321 = Multiply(x=w5767, y=w5816) -> (x*y=w5817:dbl)
            n322 = Multiply(x=w5762, y=w5805) -> (x*y=w5806:dbl)
            n323 = Multiply(x=w5773, y=w5820) -> (x*y=w5822:dbl)
            n324 = Multiply(x=w5769, y=w5816) -> (x*y=w5818:dbl)
            n325 = Multiply(x=w5765, y=w5805) -> (x*y=w5807:dbl)
            n326 = Add(x=w5822, y=w5819) -> (x+y=w5779:dbl)
            n327 = Add(x=w5818, y=w5815) -> (x+y=w5777:dbl)
            n328 = Add(x=w5821, y=w5819) -> (x+y=w5778:dbl)
            n329 = Add(x=w5817, y=w5815) -> (x+y=w5776:dbl)
            n330 = Add(x=w5807, y=w5804) -> (x+y=w5775:dbl)
            n331 = Add(x=w5806, y=w5804) -> (x+y=w5774:dbl)
            n332 = To Word Integer(number=w5777) -> (16bit integer=w5789:i16)
            n333 = To Word Integer(number=w5776) -> (16bit integer=w5788:i16)
            n334 = To Word Integer(number=w5779) -> (16bit integer=w5796:i16)
            n335 = To Word Integer(number=w5778) -> (16bit integer=w5795:i16)
            n336 = To Word Integer(number=w5775) -> (16bit integer=w5782:i16)
            n337 = To Word Integer(number=w5774) -> (16bit integer=w5781:i16)
            n338 = Bundle(w5789, w5788) -> (w5787:cluster{i16, i16})  [unwired: 1 in]
            n339 = Bundle(w5796, w5795) -> (w5794:cluster{i16, i16})  [unwired: 1 in]
            n340 = Bundle(w5782, w5781) -> (w5780:cluster{i16, i16})  [unwired: 1 in]
            n341 = call <vilib>:"Move Pen.vi"("new position"=cluster{"x":i16, "y":i16} {"x"=150, "y"=150}, "picture"=w5748) -> ("new picture"=w5784:picture)  [unwired: 3 in]
            n342 = call <vilib>:"Draw Line.vi"("picture"=w5784, "end point"=w5780, "color(black)"=u32 16711680, "pen"=T1 {"Width"=5, "Style"=enum."Solid"}) -> ("new picture"=w5747:picture)  [unwired: 5 in]
            n343 = call <vilib>:"Move Pen.vi"("new position"=cluster{"x":i16, "y":i16} {"x"=150, "y"=150}, "picture"=w5747) -> ("new picture"=w5791:picture)  [unwired: 3 in]
            n344 = call <vilib>:"Draw Line.vi"("picture"=w5791, "end point"=w5787, "color(black)"=u32 1208831, "pen"=T1 {"Width"=3, "Style"=enum."Solid"}) -> ("new picture"=w5746:picture)  [unwired: 5 in]
            n345 = call <vilib>:"Move Pen.vi"("new position"=cluster{"x":i16, "y":i16} {"x"=150, "y"=150}, "picture"=w5746) -> ("new picture"=w5798:picture)  [unwired: 3 in]
            n346 = call <vilib>:"Draw Line.vi"("picture"=w5798, "end point"=w5794, "color(black)"=u32 16762112, "pen"=T1 {"Width"=1, "Style"=enum."Solid"}) -> ("new picture"=w5749:picture)  [unwired: 5 in]
          }
          frame 3 {
            w5895 = 60.0 ("y")
            w5894 = 150.0 ("y")
            w5906 = 90.0 ("y")
            w5905 = 150.0 ("y")
            w5910 = 115.0 ("y")
            w5909 = 150.0 ("y")
            n347 = Subtract(x=w5840, y=w5846) -> (x-y=w5847:dbl)
            n348 = Subtract(x=w5845, y=w5846) -> (x-y=w5844:dbl)
            n349 = local read "Record Button"() -> (w5843:bool)
            n350 = local read "Chronograph"() -> (w5841:bool)
            n351 = And(x=w5841, y=w5843) -> (x .and. y?=w5842:bool)
            n352 = Select(t=w5844, s=w5842, f=w5847) -> (s? t:f=w5839:dbl)
            n353 = Quotient & Remainder(x=w5839, y=86400.0) -> (x-y*floor(x/y)=w5917:dbl)  [unwired: 1 out]
            n354 = Quotient & Remainder(x=w5917, y=3600.0) -> (x-y*floor(x/y)=w5918:dbl, floor(x/y)=w5903:dbl)
            n355 = Quotient & Remainder(x=w5918, y=60.0) -> (x-y*floor(x/y)=w5898:dbl, floor(x/y)=w5899:dbl)
            n356 = Quotient & Remainder(x=w5903, y=12.0) -> (x-y*floor(x/y)=w5902:dbl)  [unwired: 1 out]
            n357 = To Double Precision Float(number=w5898) -> (double precision float=w5900:dbl)
            n358 = To Double Precision Float(number=w5899) -> (double precision float=w5913:dbl)
            n359 = To Double Precision Float(number=w5902) -> (double precision float=w5915:dbl)
            n360 = Multiply(x=w5900, y=0.10471975512) -> (x*y=w5893:dbl)
            n361 = Multiply(x=w5913, y=0.10471975512) -> (x*y=w5892:dbl)
            n362 = Multiply(x=w5915, y=0.52359877559) -> (x*y=w5891:dbl)
            n363 = Sine(x=w5893) -> (sin(x)=w5863:dbl)
            n364 = Cosine(x=w5893) -> (cos(x)=w5861:dbl)
            n365 = Sine(x=w5892) -> (sin(x)=w5859:dbl)
            n366 = Cosine(x=w5892) -> (cos(x)=w5856:dbl)
            n367 = Sine(x=w5891) -> (sin(x)=w5855:dbl)
            n368 = Cosine(x=w5891) -> (cos(x)=w5853:dbl)
            n369 = Multiply(x=w5861, y=-1.0) -> (x*y=w5860:dbl)
            n370 = Multiply(x=w5856, y=-1.0) -> (x*y=w5857:dbl)
            n371 = Multiply(x=w5853, y=-1.0) -> (x*y=w5852:dbl)
            n372 = Multiply(x=w5860, y=w5910) -> (x*y=w5911:dbl)
            n373 = Multiply(x=w5857, y=w5906) -> (x*y=w5907:dbl)
            n374 = Multiply(x=w5852, y=w5895) -> (x*y=w5896:dbl)
            n375 = Multiply(x=w5863, y=w5910) -> (x*y=w5912:dbl)
            n376 = Multiply(x=w5859, y=w5906) -> (x*y=w5908:dbl)
            n377 = Multiply(x=w5855, y=w5895) -> (x*y=w5897:dbl)
            n378 = Add(x=w5912, y=w5909) -> (x+y=w5869:dbl)
            n379 = Add(x=w5908, y=w5905) -> (x+y=w5867:dbl)
            n380 = Add(x=w5911, y=w5909) -> (x+y=w5868:dbl)
            n381 = Add(x=w5907, y=w5905) -> (x+y=w5866:dbl)
            n382 = Add(x=w5897, y=w5894) -> (x+y=w5865:dbl)
            n383 = Add(x=w5896, y=w5894) -> (x+y=w5864:dbl)
            n384 = To Word Integer(number=w5867) -> (16bit integer=w5879:i16)
            n385 = To Word Integer(number=w5866) -> (16bit integer=w5878:i16)
            n386 = To Word Integer(number=w5869) -> (16bit integer=w5886:i16)
            n387 = To Word Integer(number=w5868) -> (16bit integer=w5885:i16)
            n388 = To Word Integer(number=w5865) -> (16bit integer=w5872:i16)
            n389 = To Word Integer(number=w5864) -> (16bit integer=w5871:i16)
            n390 = Bundle(w5879, w5878) -> (w5877:cluster{i16, i16})  [unwired: 1 in]
            n391 = Bundle(w5886, w5885) -> (w5884:cluster{i16, i16})  [unwired: 1 in]
            n392 = Bundle(w5872, w5871) -> (w5870:cluster{i16, i16})  [unwired: 1 in]
            n393 = call <vilib>:"Move Pen.vi"("new position"=cluster{"x":i16, "y":i16} {"x"=150, "y"=150}, "picture"=w5850) -> ("new picture"=w5874:picture)  [unwired: 3 in]
            n394 = call <vilib>:"Draw Line.vi"("picture"=w5874, "end point"=w5870, "color(black)"=u32 16711680, "pen"=T1 {"Width"=5, "Style"=enum."Solid"}) -> ("new picture"=w5849:picture)  [unwired: 5 in]
            n395 = call <vilib>:"Move Pen.vi"("new position"=cluster{"x":i16, "y":i16} {"x"=150, "y"=150}, "picture"=w5849) -> ("new picture"=w5881:picture)  [unwired: 3 in]
            n396 = call <vilib>:"Draw Line.vi"("picture"=w5881, "end point"=w5877, "color(black)"=u32 1208831, "pen"=T1 {"Width"=3, "Style"=enum."Solid"}) -> ("new picture"=w5848:picture)  [unwired: 5 in]
            n397 = call <vilib>:"Move Pen.vi"("new position"=cluster{"x":i16, "y":i16} {"x"=150, "y"=150}, "picture"=w5848) -> ("new picture"=w5888:picture)  [unwired: 3 in]
            n398 = call <vilib>:"Draw Line.vi"("picture"=w5888, "end point"=w5884, "color(black)"=u32 16762112, "pen"=T1 {"Width"=1, "Style"=enum."Solid"}) -> ("new picture"=w5851:picture)  [unwired: 5 in]
          }
        }
        n399 = case shown="True" w95 {
          tunnel: [w329 w331] -> w107
          tunnel: w106 -> [w329 w336]
          frame False {
          }
          frame True {
            n400 = Quotient & Remainder(x=w336, y=43200.0) -> (x-y*floor(x/y)=w330:dbl)  [unwired: 1 out]
            n401 = Less?(x=w330, y=3600.0) -> (x < y?=w333:bool)
            n402 = Add(x=w330, y=43200.0) -> (x+y=w332:dbl)
            n403 = Select(t=w332, s=w333, f=w330) -> (s? t:f=w331:dbl)
          }
        }
        n404 = Quotient & Remainder(x=w107, y=86400.0) -> (x-y*floor(x/y)=w124:dbl)  [unwired: 1 out]
        n405 = To Long Integer(number=w124) -> (32bit integer=w159:i32)
        n406 = Quotient & Remainder(x=w124, y=1.0) -> (x-y*floor(x/y)=w122:dbl)  [unwired: 1 out]
        n407 = Multiply(x=w122, y=100.0) -> (x*y=w120:dbl)
        n408 = Quotient & Remainder(x=w159, y=3600) -> (x-y*floor(x/y)=w158:i32, floor(x/y)=w156:i32)
        n409 = To Long Integer(number=w120) -> (32bit integer=w119:i32)
        n410 = Quotient & Remainder(x=w156, y=10) -> (x-y*floor(x/y)=w150:i32, floor(x/y)=w151:i32)
        n411 = Quotient & Remainder(x=w158, y=60) -> (x-y*floor(x/y)=w152:i32, floor(x/y)=w153:i32)
        n412 = Quotient & Remainder(x=w153, y=10) -> (x-y*floor(x/y)=w148:i32, floor(x/y)=w149:i32)
        n413 = Quotient & Remainder(x=w152, y=10) -> (x-y*floor(x/y)=w146:i32, floor(x/y)=w147:i32)
        n414 = Select(t=w248, s=w249, f=w251) -> (s? t:f=w250:dbl)
        n415 = local read "Alarm clock\nOff--On"() -> (w233:bool)
        n416 = Quotient & Remainder(x=w162, y=43200.0) -> (x-y*floor(x/y)=w253:dbl)  [unwired: 1 out]
        n417 = To Long Integer(number=w110) -> (32bit integer=w230:i32)
        n418 = To Long Integer(number=w253) -> (32bit integer=w231:i32)
        n419 = Equal?(x=w231, y=w230) -> (x = y?=w234:bool)
        n420 = And(x=w234, y=w233) -> (x .and. y?=w232:bool)
        n421 = case shown="True" w232 {
          frame False {
          }
          frame True {
            n422 = local read "Alarm clock mode\nVoice--Screen Notice"() -> (w5546:bool)
            n423 = case shown="False" w5546 {
              frame False {
                n424 = flat-sequence {
                  frame #0 {
                    n425 = local write "Sample No. x"(0 ("Sample No. x")) -> ()
                  }
                  frame #1 {
                    n426 = local write "Sound playing"(TRUE) -> ()
                  }
                }
              }
              frame True {
                n427 = local read "Notice Content"() -> (w5550:string)
                n428 = One Button Dialog(message=w5550, button name ("OK")="Got it!") -> ()  [unwired: 1 out]
              }
            }
          }
        }
        n429 = Quotient & Remainder(x=w109, y=86400.0) -> (x-y*floor(x/y)=w101:dbl)  [unwired: 1 out]
        n430 = call <vilib>:"Draw Circle by Radius.vi"("pen"=T1 {"Width"=1, "Style"=enum."Solid"}, "color(black)"=u32 14768639, "fill?(F)"=TRUE, "pixel center"=cluster{"horizontal":i16, "vertical":i16} {"horizontal"=150, "vertical"=150}, "radius"=i16 3, "picture"=w224) -> ("new picture"=w215:picture)  [unwired: 5 in]
        n431 = Subtract(x=w101, y=43200.0) -> (x-y=w207:dbl)
        n432 = local read "Alarm clock\nOff--On"() -> (w235:bool)
        n433 = Absolute Value(x=w207) -> (abs(x)=w206:dbl)
        n434 = Greater Or Equal?(x=w101, y=21600.0) -> (x >= y?=w104:bool)
        n435 = Divide(x=w206, y=43200.0) -> (x/y=w201:dbl)
        n436 = Less?(x=w101, y=64800.0) -> (x < y?=w103:bool)
        n437 = Subtract(x=1.0, y=w201) -> (x-y=w190:dbl)
        n438 = Multiply(x=w190, y=240.0) -> (x*y=w197:dbl)
        n439 = And(x=w103, y=w104) -> (x .and. y?=w100:bool)
        n440 = Multiply(x=w190, y=170.0) -> (x*y=w198:dbl)
        n441 = To Unsigned Byte Integer(number=w197) -> (unsigned 8bit integer=w196:u8)
        n442 = To Unsigned Byte Integer(number=w198) -> (unsigned 8bit integer=w195:u8)
        n443 = call <vilib>:"RGB to Color.vi"("B"=u8 255, "G"=w196, "R"=w195) -> ("Color"=w97:u32)
        n444 = call <vilib>:"Draw Rectangle.vi"("picture"=w215, "rect"=T2 {"left"=301, "top"=0, "right"=840, "bottom"=440}, "fill?(F)"=TRUE, "color(black)"=w97, "pen"=T3 {"Width"=1, "Style"=enum."Solid"}) -> ("new picture"=w211:picture)  [unwired: 4 in]
        n445 = case shown="False" w235 {
          frame False {
            n446 = local write "Sound playing"(FALSE) -> ()
          }
          frame True {
          }
        }
        n447 = Multiply(x=w190, y=200.0) -> (x*y=w194:dbl)
        n448 = Multiply(x=w190, y=160.0) -> (x*y=w193:dbl)
        n449 = To Unsigned Byte Integer(number=w194) -> (unsigned 8bit integer=w189:u8)
        n450 = To Unsigned Byte Integer(number=w193) -> (unsigned 8bit integer=w188:u8)
        n451 = call <vilib>:"RGB to Color.vi"("B"=w188, "G"=u8 255, "R"=w189) -> ("Color"=w210:u32)
        n452 = call <vilib>:"Draw Rectangle.vi"("picture"=w211, "rect"=T2 {"left"=301, "top"=440, "right"=840, "bottom"=540}, "fill?(F)"=TRUE, "color(black)"=w210, "pen"=T3 {"Width"=1, "Style"=enum."Solid"}) -> ("new picture"=w137:picture)  [unwired: 4 in]
        n453 = call <vilib>:"Draw Rectangle.vi"("picture"=w137, "rect"=T2 {"left"=400, "top"=25, "right"=405, "bottom"=30}, "fill?(F)"=TRUE, "color(black)"=u32 16448250, "pen"=T3 {"Width"=1, "Style"=enum."Solid"}) -> ("new picture"=w136:picture)  [unwired: 4 in]
        n454 = call <vilib>:"Draw Rectangle.vi"("picture"=w136, "rect"=T2 {"left"=400, "top"=50, "right"=405, "bottom"=55}, "fill?(F)"=TRUE, "color(black)"=u32 16448250, "pen"=T3 {"Width"=1, "Style"=enum."Solid"}) -> ("new picture"=w126:picture)  [unwired: 4 in]
        n455 = call <vilib>:"Draw Rectangle.vi"("picture"=w126, "rect"=T2 {"left"=510, "top"=25, "right"=515, "bottom"=30}, "fill?(F)"=TRUE, "color(black)"=u32 16448250, "pen"=T3 {"Width"=1, "Style"=enum."Solid"}) -> ("new picture"=w127:picture)  [unwired: 4 in]
        n456 = Quotient & Remainder(x=w119, y=10) -> (x-y*floor(x/y)=w116:i32, floor(x/y)=w117:i32)
        n457 = call <vilib>:"Draw Rectangle.vi"("picture"=w127, "rect"=T2 {"left"=510, "top"=50, "right"=515, "bottom"=55}, "fill?(F)"=TRUE, "color(black)"=u32 16448250, "pen"=T3 {"Width"=1, "Style"=enum."Solid"}) -> ("new picture"=w99:picture)  [unwired: 4 in]
        n458 = case shown="False" w100 {
          tunnel: w99 -> [w274 w283]
          tunnel: [w267 w280] -> w98
          tunnel: w97 -> [w268 _]
          frame False {
            n459 = call <vilib>:"Draw Circle by Radius.vi"("pen"=T1 {"Width"=1, "Style"=enum."Solid"}, "color(black)"=u32 16770626, "fill?(F)"=TRUE, "pixel center"=cluster{"horizontal":i16, "vertical":i16} {"horizontal"=760, "vertical"=80}, "radius"=i16 40, "picture"=w274) -> ("new picture"=w269:picture)  [unwired: 5 in]
            n460 = call <vilib>:"Draw Circle by Radius.vi"("pen"=T1 {"Width"=1, "Style"=enum."Solid"}, "color(black)"=w268, "fill?(F)"=TRUE, "pixel center"=cluster{"horizontal":i16, "vertical":i16} {"horizontal"=775, "vertical"=65}, "radius"=i16 40, "picture"=w269) -> ("new picture"=w267:picture)  [unwired: 5 in]
          }
          frame True {
            n461 = call <vilib>:"Draw Circle by Radius.vi"("pen"=T1 {"Width"=1, "Style"=enum."Solid"}, "color(black)"=u32 16514952, "fill?(F)"=TRUE, "pixel center"=cluster{"horizontal":i16, "vertical":i16} {"horizontal"=760, "vertical"=80}, "radius"=i16 40, "picture"=w283) -> ("new picture"=w281:picture)  [unwired: 5 in]
            n462 = for {
              N: 10 -> [_]
              shift-right: [w303] -> w280
              shift-left: w281 -> [w304]
              i -> [w293]
              w291 = 50.0 ("x")
              w309 = 65.0 ("y")
              n463 = To Double Precision Float(number=w293) -> (double precision float=w319:dbl)
              n464 = Multiply(x=w319, y=0.62831853071) -> (x*y=w328:dbl)
              n465 = Sine(x=w328) -> (sin(x)=w326:dbl)
              n466 = Cosine(x=w328) -> (cos(x)=w327:dbl)
              n467 = Multiply(x=w327, y=-1.0) -> (x*y=w320:dbl)
              n468 = Multiply(x=w326, y=w291) -> (x*y=w325:dbl)
              n469 = Multiply(x=w291, y=w320) -> (x*y=w321:dbl)
              n470 = Add(x=w325, y=760.0) -> (x+y=w306:dbl)
              n471 = Add(x=80.0 ("y"), y=w321) -> (x+y=w305:dbl)
              n472 = To Word Integer(number=w305) -> (16bit integer=w300:i16)
              n473 = To Word Integer(number=w306) -> (16bit integer=w301:i16)
              n474 = Bundle(w301, w300) -> (w302:cluster{i16, i16})  [unwired: 1 in]
              n475 = call <vilib>:"Move Pen.vi"("new position"=w302, "picture"=w304) -> ("new picture"=w318:picture)  [unwired: 3 in]
              n476 = To Double Precision Float(number=w293) -> (double precision float=w307:dbl)
              n477 = Multiply(x=w307, y=0.62831853071) -> (x*y=w315:dbl)
              n478 = Sine(x=w315) -> (sin(x)=w313:dbl)
              n479 = Cosine(x=w315) -> (cos(x)=w314:dbl)
              n480 = Multiply(x=w314, y=-1.0) -> (x*y=w310:dbl)
              n481 = Multiply(x=w309, y=w310) -> (x*y=w311:dbl)
              n482 = Multiply(x=w313, y=w309) -> (x*y=w312:dbl)
              n483 = Add(x=w312, y=760.0) -> (x+y=w299:dbl)
              n484 = Add(x=80.0, y=w311) -> (x+y=w298:dbl)
              n485 = To Word Integer(number=w298) -> (16bit integer=w296:i16)
              n486 = To Word Integer(number=w299) -> (16bit integer=w297:i16)
              n487 = Bundle(w297, w296) -> (w295:cluster{i16, i16})  [unwired: 1 in]
              n488 = call <vilib>:"Draw Line.vi"("picture"=w318, "end point"=w295, "color(black)"=u32 16514952, "pen"=T1 {"Width"=4, "Style"=enum."Solid"}) -> ("new picture"=w303:picture)  [unwired: 5 in]
            }
          }
        }
        n489 = case shown="0, Default" w151 {
          tunnel: 310 -> [w4885 w4959 w4989 w5057 w5122 w5174 w5242 w5319 w5375 w5464]
          tunnel: 10 -> [w4884 w4958 w4988 w5056 w5121 w5173 w5241 w5318 w5374 w5463]
          tunnel: 3 -> [w4883 w4957 w4987 w5055 w5120 w5172 w5240 w5317 w5373 w5462]
          tunnel: w98 -> [w4886 w4961 w4991 w5058 w5123 w5176 w5244 w5321 w5377 w5466]
          tunnel: [w4877 w4956 w4983 w5050 w5116 w5168 w5235 w5314 w5367 w5458] -> w179
          frame 0, Default {
            n490 = Add(x=w4885, y=0) -> (x+y=w4941:i32)
            n491 = Add(x=w4884, y=0) -> (x+y=w4942:i32)
            n492 = Multiply(x=w4883, y=10) -> (x*y=w4940:i32)
            n493 = Add(x=w4885, y=0) -> (x+y=w4907:i32)
            n494 = Multiply(x=w4883, y=10) -> (x*y=w4910:i32)
            n495 = Add(x=w4884, y=w4910) -> (x+y=w4908:i32)
            n496 = Add(x=w4942, y=w4940) -> (x+y=w4943:i32)
            n497 = Add(x=w4908, y=w4910) -> (x+y=w4909:i32)
            n498 = Bundle(w4941, w4942) -> (w4938:cluster{i32, i32})  [unwired: 1 in]
            n499 = Bundle(w4907, w4908) -> (w4905:cluster{i32, i32})  [unwired: 1 in]
            n500 = Bundle(w4941, w4943) -> (w4939:cluster{i32, i32})  [unwired: 1 in]
            n501 = Bundle(w4907, w4909) -> (w4906:cluster{i32, i32})  [unwired: 1 in]
            n502 = Multiply(x=w4883, y=10) -> (x*y=w4898:i32)
            n503 = Multiply(x=2, y=w4898) -> (x*y=w4899:i32)
            n504 = Add(x=w4885, y=0) -> (x+y=w4953:i32)
            n505 = Add(x=w4884, y=0) -> (x+y=w4954:i32)
            n506 = Add(x=w4885, y=0) -> (x+y=w4895:i32)
            n507 = Add(x=w4884, y=w4899) -> (x+y=w4897:i32)
            n508 = Multiply(x=w4883, y=10) -> (x*y=w4951:i32)
            n509 = Add(x=w4895, y=w4898) -> (x+y=w4894:i32)
            n510 = Add(x=w4953, y=w4951) -> (x+y=w4952:i32)
            n511 = Bundle(w4953, w4954) -> (w4950:cluster{i32, i32})  [unwired: 1 in]
            n512 = Bundle(w4895, w4897) -> (w4893:cluster{i32, i32})  [unwired: 1 in]
            n513 = call <vilib>:"Move Pen.vi"("new position"=w4950, "picture"=w4886) -> ("new picture"=w4949:picture)  [unwired: 3 in]
            n514 = Bundle(w4952, w4954) -> (w4955:cluster{i32, i32})  [unwired: 1 in]
            n515 = Bundle(w4894, w4897) -> (w4896:cluster{i32, i32})  [unwired: 1 in]
            n516 = Multiply(x=w4883, y=10) -> (x*y=w4928:i32)
            n517 = Add(x=w4885, y=w4928) -> (x+y=w4929:i32)
            n518 = Add(x=w4884, y=0) -> (x+y=w4931:i32)
            n519 = Multiply(x=w4883, y=10) -> (x*y=w4920:i32)
            n520 = Add(x=w4885, y=w4920) -> (x+y=w4917:i32)
            n521 = Add(x=w4884, y=w4920) -> (x+y=w4919:i32)
            n522 = Add(x=w4931, y=w4928) -> (x+y=w4930:i32)
            n523 = Bundle(w4929, w4931) -> (w4926:cluster{i32, i32})  [unwired: 1 in]
            n524 = call <vilib>:"Draw Line.vi"("picture"=w4949, "end point"=w4955, "color(black)"=u32 16448250, "pen"=T1 {"Width"=3, "Style"=enum."Solid"}) -> ("new picture"=w4882:picture)  [unwired: 5 in]
            n525 = call <vilib>:"Move Pen.vi"("new position"=w4938, "picture"=w4882) -> ("new picture"=w4937:picture)  [unwired: 3 in]
            n526 = call <vilib>:"Draw Line.vi"("picture"=w4937, "end point"=w4939, "color(black)"=u32 16448250, "pen"=T1 {"Width"=3, "Style"=enum."Solid"}) -> ("new picture"=w4881:picture)  [unwired: 5 in]
            n527 = Add(x=w4919, y=w4920) -> (x+y=w4918:i32)
            n528 = Bundle(w4917, w4919) -> (w4915:cluster{i32, i32})  [unwired: 1 in]
            n529 = call <vilib>:"Move Pen.vi"("new position"=w4926, "picture"=w4881) -> ("new picture"=w4925:picture)  [unwired: 3 in]
            n530 = Bundle(w4929, w4930) -> (w4927:cluster{i32, i32})  [unwired: 1 in]
            n531 = Bundle(w4917, w4918) -> (w4916:cluster{i32, i32})  [unwired: 1 in]
            n532 = call <vilib>:"Draw Line.vi"("picture"=w4925, "end point"=w4927, "color(black)"=u32 16448250, "pen"=T1 {"Width"=3, "Style"=enum."Solid"}) -> ("new picture"=w4880:picture)  [unwired: 5 in]
            n533 = call <vilib>:"Move Pen.vi"("new position"=w4905, "picture"=w4880) -> ("new picture"=w4904:picture)  [unwired: 3 in]
            n534 = call <vilib>:"Draw Line.vi"("picture"=w4904, "end point"=w4906, "color(black)"=u32 16448250, "pen"=T1 {"Width"=3, "Style"=enum."Solid"}) -> ("new picture"=w4879:picture)  [unwired: 5 in]
            n535 = call <vilib>:"Move Pen.vi"("new position"=w4915, "picture"=w4879) -> ("new picture"=w4914:picture)  [unwired: 3 in]
            n536 = call <vilib>:"Draw Line.vi"("picture"=w4914, "end point"=w4916, "color(black)"=u32 16448250, "pen"=T1 {"Width"=3, "Style"=enum."Solid"}) -> ("new picture"=w4878:picture)  [unwired: 5 in]
            n537 = call <vilib>:"Move Pen.vi"("new position"=w4893, "picture"=w4878) -> ("new picture"=w4892:picture)  [unwired: 3 in]
            n538 = call <vilib>:"Draw Line.vi"("picture"=w4892, "end point"=w4896, "color(black)"=u32 16448250, "pen"=T1 {"Width"=3, "Style"=enum."Solid"}) -> ("new picture"=w4877:picture)  [unwired: 5 in]
          }
          frame 1 {
            n539 = Multiply(x=w4957, y=10) -> (x*y=w4979:i32)
            n540 = Add(x=w4959, y=w4979) -> (x+y=w4980:i32)
            n541 = Add(x=w4958, y=0) -> (x+y=w4982:i32)
            n542 = Add(x=w4982, y=w4979) -> (x+y=w4981:i32)
            n543 = Bundle(w4980, w4982) -> (w4977:cluster{i32, i32})  [unwired: 1 in]
            n544 = call <vilib>:"Move Pen.vi"("new position"=w4977, "picture"=w4961) -> ("new picture"=w4976:picture)  [unwired: 3 in]
            n545 = Bundle(w4980, w4981) -> (w4978:cluster{i32, i32})  [unwired: 1 in]
            n546 = call <vilib>:"Draw Line.vi"("picture"=w4976, "end point"=w4978, "color(black)"=u32 16448250, "pen"=T1 {"Width"=3, "Style"=enum."Solid"}) -> ("new picture"=w4960:picture)  [unwired: 5 in]
            n547 = Multiply(x=w4957, y=10) -> (x*y=w4971:i32)
            n548 = Add(x=w4959, y=w4971) -> (x+y=w4968:i32)
            n549 = Add(x=w4958, y=w4971) -> (x+y=w4970:i32)
            n550 = Add(x=w4970, y=w4971) -> (x+y=w4969:i32)
            n551 = Bundle(w4968, w4970) -> (w4966:cluster{i32, i32})  [unwired: 1 in]
            n552 = call <vilib>:"Move Pen.vi"("new position"=w4966, "picture"=w4960) -> ("new picture"=w4965:picture)  [unwired: 3 in]
            n553 = Bundle(w4968, w4969) -> (w4967:cluster{i32, i32})  [unwired: 1 in]
            n554 = call <vilib>:"Draw Line.vi"("picture"=w4965, "end point"=w4967, "color(black)"=u32 16448250, "pen"=T1 {"Width"=3, "Style"=enum."Solid"}) -> ("new picture"=w4956:picture)  [unwired: 5 in]
          }
          frame 2 {
            n555 = Multiply(x=w4987, y=10) -> (x*y=w5025:i32)
            n556 = Add(x=w4989, y=0) -> (x+y=w5023:i32)
            n557 = Add(x=w4988, y=w5025) -> (x+y=w5026:i32)
            n558 = Add(x=w4989, y=0) -> (x+y=w5047:i32)
            n559 = Add(x=w4988, y=0) -> (x+y=w5048:i32)
            n560 = Multiply(x=w4987, y=10) -> (x*y=w5045:i32)
            n561 = Add(x=w5023, y=w5025) -> (x+y=w5022:i32)
            n562 = Add(x=w5047, y=w5045) -> (x+y=w5046:i32)
            n563 = Bundle(w5023, w5026) -> (w5021:cluster{i32, i32})  [unwired: 1 in]
            n564 = Bundle(w5047, w5048) -> (w5044:cluster{i32, i32})  [unwired: 1 in]
            n565 = Bundle(w5022, w5026) -> (w5024:cluster{i32, i32})  [unwired: 1 in]
            n566 = call <vilib>:"Move Pen.vi"("new position"=w5044, "picture"=w4991) -> ("new picture"=w5043:picture)  [unwired: 3 in]
            n567 = Bundle(w5046, w5048) -> (w5049:cluster{i32, i32})  [unwired: 1 in]
            n568 = Multiply(x=w4987, y=10) -> (x*y=w5003:i32)
            n569 = Multiply(x=2, y=w5003) -> (x*y=w5004:i32)
            n570 = Add(x=w4989, y=0) -> (x+y=w5000:i32)
            n571 = Add(x=w4988, y=w5004) -> (x+y=w5002:i32)
            n572 = Add(x=w5000, y=w5003) -> (x+y=w4999:i32)
            n573 = Bundle(w5000, w5002) -> (w4998:cluster{i32, i32})  [unwired: 1 in]
            n574 = call <vilib>:"Draw Line.vi"("picture"=w5043, "end point"=w5049, "color(black)"=u32 16448250, "pen"=T1 {"Width"=3, "Style"=enum."Solid"}) -> ("new picture"=w4990:picture)  [unwired: 5 in]
            n575 = Bundle(w4999, w5002) -> (w5001:cluster{i32, i32})  [unwired: 1 in]
            n576 = Multiply(x=w4987, y=10) -> (x*y=w5034:i32)
            n577 = Add(x=w4989, y=0) -> (x+y=w5012:i32)
            n578 = Add(x=w4989, y=w5034) -> (x+y=w5035:i32)
            n579 = Add(x=w4988, y=0) -> (x+y=w5037:i32)
            n580 = Multiply(x=w4987, y=10) -> (x*y=w5015:i32)
            n581 = Add(x=w4988, y=w5015) -> (x+y=w5013:i32)
            n582 = Add(x=w5013, y=w5015) -> (x+y=w5014:i32)
            n583 = Add(x=w5037, y=w5034) -> (x+y=w5036:i32)
            n584 = Bundle(w5012, w5013) -> (w5010:cluster{i32, i32})  [unwired: 1 in]
            n585 = Bundle(w5035, w5037) -> (w5032:cluster{i32, i32})  [unwired: 1 in]
            n586 = call <vilib>:"Move Pen.vi"("new position"=w5032, "picture"=w4990) -> ("new picture"=w5031:picture)  [unwired: 3 in]
            n587 = Bundle(w5012, w5014) -> (w5011:cluster{i32, i32})  [unwired: 1 in]
            n588 = Bundle(w5035, w5036) -> (w5033:cluster{i32, i32})  [unwired: 1 in]
            n589 = call <vilib>:"Draw Line.vi"("picture"=w5031, "end point"=w5033, "color(black)"=u32 16448250, "pen"=T1 {"Width"=3, "Style"=enum."Solid"}) -> ("new picture"=w4986:picture)  [unwired: 5 in]
            n590 = call <vilib>:"Move Pen.vi"("new position"=w5021, "picture"=w4986) -> ("new picture"=w5020:picture)  [unwired: 3 in]
            n591 = call <vilib>:"Draw Line.vi"("picture"=w5020, "end point"=w5024, "color(black)"=u32 16448250, "pen"=T1 {"Width"=3, "Style"=enum."Solid"}) -> ("new picture"=w4985:picture)  [unwired: 5 in]
            n592 = call <vilib>:"Move Pen.vi"("new position"=w5010, "picture"=w4985) -> ("new picture"=w5009:picture)  [unwired: 3 in]
            n593 = call <vilib>:"Draw Line.vi"("picture"=w5009, "end point"=w5011, "color(black)"=u32 16448250, "pen"=T1 {"Width"=3, "Style"=enum."Solid"}) -> ("new picture"=w4984:picture)  [unwired: 5 in]
            n594 = call <vilib>:"Move Pen.vi"("new position"=w4998, "picture"=w4984) -> ("new picture"=w4997:picture)  [unwired: 3 in]
            n595 = call <vilib>:"Draw Line.vi"("picture"=w4997, "end point"=w5001, "color(black)"=u32 16448250, "pen"=T1 {"Width"=3, "Style"=enum."Solid"}) -> ("new picture"=w4983:picture)  [unwired: 5 in]
          }
          frame 3 {
            n596 = Multiply(x=w5055, y=10) -> (x*y=w5091:i32)
            n597 = Add(x=w5057, y=0) -> (x+y=w5089:i32)
            n598 = Add(x=w5056, y=w5091) -> (x+y=w5092:i32)
            n599 = Add(x=w5057, y=0) -> (x+y=w5113:i32)
            n600 = Add(x=w5056, y=0) -> (x+y=w5114:i32)
            n601 = Multiply(x=w5055, y=10) -> (x*y=w5111:i32)
            n602 = Add(x=w5089, y=w5091) -> (x+y=w5088:i32)
            n603 = Add(x=w5113, y=w5111) -> (x+y=w5112:i32)
            n604 = Bundle(w5089, w5092) -> (w5087:cluster{i32, i32})  [unwired: 1 in]
            n605 = Bundle(w5113, w5114) -> (w5110:cluster{i32, i32})  [unwired: 1 in]
            n606 = call <vilib>:"Move Pen.vi"("new position"=w5110, "picture"=w5058) -> ("new picture"=w5109:picture)  [unwired: 3 in]
            n607 = Bundle(w5088, w5092) -> (w5090:cluster{i32, i32})  [unwired: 1 in]
            n608 = Bundle(w5112, w5114) -> (w5115:cluster{i32, i32})  [unwired: 1 in]
            n609 = Multiply(x=w5055, y=10) -> (x*y=w5070:i32)
            n610 = Multiply(x=2, y=w5070) -> (x*y=w5071:i32)
            n611 = Add(x=w5057, y=0) -> (x+y=w5067:i32)
            n612 = Add(x=w5056, y=w5071) -> (x+y=w5069:i32)
            n613 = Add(x=w5067, y=w5070) -> (x+y=w5066:i32)
            n614 = call <vilib>:"Draw Line.vi"("picture"=w5109, "end point"=w5115, "color(black)"=u32 16448250, "pen"=T1 {"Width"=3, "Style"=enum."Solid"}) -> ("new picture"=w5054:picture)  [unwired: 5 in]
            n615 = Bundle(w5067, w5069) -> (w5065:cluster{i32, i32})  [unwired: 1 in]
            n616 = Bundle(w5066, w5069) -> (w5068:cluster{i32, i32})  [unwired: 1 in]
            n617 = Multiply(x=w5055, y=10) -> (x*y=w5081:i32)
            n618 = Add(x=w5057, y=w5081) -> (x+y=w5078:i32)
            n619 = Add(x=w5056, y=w5081) -> (x+y=w5080:i32)
            n620 = Multiply(x=w5055, y=10) -> (x*y=w5100:i32)
            n621 = Add(x=w5057, y=w5100) -> (x+y=w5101:i32)
            n622 = Add(x=w5056, y=0) -> (x+y=w5103:i32)
            n623 = Add(x=w5080, y=w5081) -> (x+y=w5079:i32)
            n624 = Bundle(w5078, w5080) -> (w5076:cluster{i32, i32})  [unwired: 1 in]
            n625 = Add(x=w5103, y=w5100) -> (x+y=w5102:i32)
            n626 = Bundle(w5101, w5103) -> (w5098:cluster{i32, i32})  [unwired: 1 in]
            n627 = Bundle(w5078, w5079) -> (w5077:cluster{i32, i32})  [unwired: 1 in]
            n628 = call <vilib>:"Move Pen.vi"("new position"=w5098, "picture"=w5054) -> ("new picture"=w5097:picture)  [unwired: 3 in]
            n629 = Bundle(w5101, w5102) -> (w5099:cluster{i32, i32})  [unwired: 1 in]
            n630 = call <vilib>:"Draw Line.vi"("picture"=w5097, "end point"=w5099, "color(black)"=u32 16448250, "pen"=T1 {"Width"=3, "Style"=enum."Solid"}) -> ("new picture"=w5053:picture)  [unwired: 5 in]
            n631 = call <vilib>:"Move Pen.vi"("new position"=w5087, "picture"=w5053) -> ("new picture"=w5086:picture)  [unwired: 3 in]
            n632 = call <vilib>:"Draw Line.vi"("picture"=w5086, "end point"=w5090, "color(black)"=u32 16448250, "pen"=T1 {"Width"=3, "Style"=enum."Solid"}) -> ("new picture"=w5052:picture)  [unwired: 5 in]
            n633 = call <vilib>:"Move Pen.vi"("new position"=w5076, "picture"=w5052) -> ("new picture"=w5075:picture)  [unwired: 3 in]
            n634 = call <vilib>:"Draw Line.vi"("picture"=w5075, "end point"=w5077, "color(black)"=u32 16448250, "pen"=T1 {"Width"=3, "Style"=enum."Solid"}) -> ("new picture"=w5051:picture)  [unwired: 5 in]
            n635 = call <vilib>:"Move Pen.vi"("new position"=w5065, "picture"=w5051) -> ("new picture"=w5064:picture)  [unwired: 3 in]
            n636 = call <vilib>:"Draw Line.vi"("picture"=w5064, "end point"=w5068, "color(black)"=u32 16448250, "pen"=T1 {"Width"=3, "Style"=enum."Solid"}) -> ("new picture"=w5050:picture)  [unwired: 5 in]
          }
          frame 4 {
            n637 = Add(x=w5122, y=0) -> (x+y=w5165:i32)
            n638 = Add(x=w5121, y=0) -> (x+y=w5166:i32)
            n639 = Multiply(x=w5120, y=10) -> (x*y=w5164:i32)
            n640 = Add(x=w5166, y=w5164) -> (x+y=w5167:i32)
            n641 = Bundle(w5165, w5166) -> (w5162:cluster{i32, i32})  [unwired: 1 in]
            n642 = call <vilib>:"Move Pen.vi"("new position"=w5162, "picture"=w5123) -> ("new picture"=w5161:picture)  [unwired: 3 in]
            n643 = Bundle(w5165, w5167) -> (w5163:cluster{i32, i32})  [unwired: 1 in]
            n644 = Multiply(x=w5120, y=10) -> (x*y=w5143:i32)
            n645 = Add(x=w5122, y=0) -> (x+y=w5141:i32)
            n646 = Add(x=w5121, y=w5143) -> (x+y=w5144:i32)
            n647 = Add(x=w5141, y=w5143) -> (x+y=w5140:i32)
            n648 = Bundle(w5141, w5144) -> (w5139:cluster{i32, i32})  [unwired: 1 in]
            n649 = call <vilib>:"Draw Line.vi"("picture"=w5161, "end point"=w5163, "color(black)"=u32 16448250, "pen"=T1 {"Width"=3, "Style"=enum."Solid"}) -> ("new picture"=w5117:picture)  [unwired: 5 in]
            n650 = Multiply(x=w5120, y=10) -> (x*y=w5133:i32)
            n651 = Add(x=w5122, y=w5133) -> (x+y=w5130:i32)
            n652 = Add(x=w5121, y=w5133) -> (x+y=w5132:i32)
            n653 = Bundle(w5140, w5144) -> (w5142:cluster{i32, i32})  [unwired: 1 in]
            n654 = Add(x=w5132, y=w5133) -> (x+y=w5131:i32)
            n655 = Bundle(w5130, w5132) -> (w5128:cluster{i32, i32})  [unwired: 1 in]
            n656 = Multiply(x=w5120, y=10) -> (x*y=w5152:i32)
            n657 = Add(x=w5122, y=w5152) -> (x+y=w5153:i32)
            n658 = Add(x=w5121, y=0) -> (x+y=w5155:i32)
            n659 = Add(x=w5155, y=w5152) -> (x+y=w5154:i32)
            n660 = Bundle(w5130, w5131) -> (w5129:cluster{i32, i32})  [unwired: 1 in]
            n661 = Bundle(w5153, w5155) -> (w5150:cluster{i32, i32})  [unwired: 1 in]
            n662 = call <vilib>:"Move Pen.vi"("new position"=w5150, "picture"=w5117) -> ("new picture"=w5149:picture)  [unwired: 3 in]
            n663 = Bundle(w5153, w5154) -> (w5151:cluster{i32, i32})  [unwired: 1 in]
            n664 = call <vilib>:"Draw Line.vi"("picture"=w5149, "end point"=w5151, "color(black)"=u32 16448250, "pen"=T1 {"Width"=3, "Style"=enum."Solid"}) -> ("new picture"=w5119:picture)  [unwired: 5 in]
            n665 = call <vilib>:"Move Pen.vi"("new position"=w5139, "picture"=w5119) -> ("new picture"=w5138:picture)  [unwired: 3 in]
            n666 = call <vilib>:"Draw Line.vi"("picture"=w5138, "end point"=w5142, "color(black)"=u32 16448250, "pen"=T1 {"Width"=3, "Style"=enum."Solid"}) -> ("new picture"=w5118:picture)  [unwired: 5 in]
            n667 = call <vilib>:"Move Pen.vi"("new position"=w5128, "picture"=w5118) -> ("new picture"=w5127:picture)  [unwired: 3 in]
            n668 = call <vilib>:"Draw Line.vi"("picture"=w5127, "end point"=w5129, "color(black)"=u32 16448250, "pen"=T1 {"Width"=3, "Style"=enum."Solid"}) -> ("new picture"=w5116:picture)  [unwired: 5 in]
          }
          frame 5 {
            n669 = Multiply(x=w5172, y=10) -> (x*y=w5209:i32)
            n670 = Add(x=w5174, y=0) -> (x+y=w5207:i32)
            n671 = Add(x=w5173, y=w5209) -> (x+y=w5210:i32)
            n672 = Add(x=w5174, y=0) -> (x+y=w5232:i32)
            n673 = Add(x=w5173, y=0) -> (x+y=w5233:i32)
            n674 = Add(x=w5207, y=w5209) -> (x+y=w5206:i32)
            n675 = Multiply(x=w5172, y=10) -> (x*y=w5230:i32)
            n676 = Bundle(w5207, w5210) -> (w5205:cluster{i32, i32})  [unwired: 1 in]
            n677 = Add(x=w5232, y=w5230) -> (x+y=w5231:i32)
            n678 = Bundle(w5232, w5233) -> (w5229:cluster{i32, i32})  [unwired: 1 in]
            n679 = Bundle(w5206, w5210) -> (w5208:cluster{i32, i32})  [unwired: 1 in]
            n680 = call <vilib>:"Move Pen.vi"("new position"=w5229, "picture"=w5176) -> ("new picture"=w5228:picture)  [unwired: 3 in]
            n681 = Bundle(w5231, w5233) -> (w5234:cluster{i32, i32})  [unwired: 1 in]
            n682 = Multiply(x=w5172, y=10) -> (x*y=w5188:i32)
            n683 = Multiply(x=2, y=w5188) -> (x*y=w5189:i32)
            n684 = Add(x=w5174, y=0) -> (x+y=w5185:i32)
            n685 = Add(x=w5173, y=w5189) -> (x+y=w5187:i32)
            n686 = Add(x=w5185, y=w5188) -> (x+y=w5184:i32)
            n687 = Bundle(w5185, w5187) -> (w5183:cluster{i32, i32})  [unwired: 1 in]
            n688 = call <vilib>:"Draw Line.vi"("picture"=w5228, "end point"=w5234, "color(black)"=u32 16448250, "pen"=T1 {"Width"=3, "Style"=enum."Solid"}) -> ("new picture"=w5175:picture)  [unwired: 5 in]
            n689 = Bundle(w5184, w5187) -> (w5186:cluster{i32, i32})  [unwired: 1 in]
            n690 = Multiply(x=w5172, y=10) -> (x*y=w5199:i32)
            n691 = Add(x=w5174, y=0) -> (x+y=w5220:i32)
            n692 = Add(x=w5173, y=0) -> (x+y=w5221:i32)
            n693 = Add(x=w5174, y=w5199) -> (x+y=w5196:i32)
            n694 = Add(x=w5173, y=w5199) -> (x+y=w5198:i32)
            n695 = Multiply(x=w5172, y=10) -> (x*y=w5219:i32)
            n696 = Add(x=w5221, y=w5219) -> (x+y=w5222:i32)
            n697 = Add(x=w5198, y=w5199) -> (x+y=w5197:i32)
            n698 = Bundle(w5220, w5221) -> (w5217:cluster{i32, i32})  [unwired: 1 in]
            n699 = Bundle(w5196, w5198) -> (w5194:cluster{i32, i32})  [unwired: 1 in]
            n700 = call <vilib>:"Move Pen.vi"("new position"=w5217, "picture"=w5175) -> ("new picture"=w5216:picture)  [unwired: 3 in]
            n701 = Bundle(w5220, w5222) -> (w5218:cluster{i32, i32})  [unwired: 1 in]
            n702 = Bundle(w5196, w5197) -> (w5195:cluster{i32, i32})  [unwired: 1 in]
            n703 = call <vilib>:"Draw Line.vi"("picture"=w5216, "end point"=w5218, "color(black)"=u32 16448250, "pen"=T1 {"Width"=3, "Style"=enum."Solid"}) -> ("new picture"=w5171:picture)  [unwired: 5 in]
            n704 = call <vilib>:"Move Pen.vi"("new position"=w5205, "picture"=w5171) -> ("new picture"=w5204:picture)  [unwired: 3 in]
            n705 = call <vilib>:"Draw Line.vi"("picture"=w5204, "end point"=w5208, "color(black)"=u32 16448250, "pen"=T1 {"Width"=3, "Style"=enum."Solid"}) -> ("new picture"=w5170:picture)  [unwired: 5 in]
            n706 = call <vilib>:"Move Pen.vi"("new position"=w5194, "picture"=w5170) -> ("new picture"=w5193:picture)  [unwired: 3 in]
            n707 = call <vilib>:"Draw Line.vi"("picture"=w5193, "end point"=w5195, "color(black)"=u32 16448250, "pen"=T1 {"Width"=3, "Style"=enum."Solid"}) -> ("new picture"=w5169:picture)  [unwired: 5 in]
            n708 = call <vilib>:"Move Pen.vi"("new position"=w5183, "picture"=w5169) -> ("new picture"=w5182:picture)  [unwired: 3 in]
            n709 = call <vilib>:"Draw Line.vi"("picture"=w5182, "end point"=w5186, "color(black)"=u32 16448250, "pen"=T1 {"Width"=3, "Style"=enum."Solid"}) -> ("new picture"=w5168:picture)  [unwired: 5 in]
          }
          frame 6 {
            n710 = Multiply(x=w5240, y=10) -> (x*y=w5278:i32)
            n711 = Multiply(x=w5240, y=10) -> (x*y=w5288:i32)
            n712 = Add(x=w5242, y=w5278) -> (x+y=w5275:i32)
            n713 = Add(x=w5241, y=w5278) -> (x+y=w5277:i32)
            n714 = Add(x=w5242, y=0) -> (x+y=w5286:i32)
            n715 = Add(x=w5241, y=w5288) -> (x+y=w5289:i32)
            n716 = Add(x=w5242, y=0) -> (x+y=w5311:i32)
            n717 = Add(x=w5241, y=0) -> (x+y=w5312:i32)
            n718 = Multiply(x=w5240, y=10) -> (x*y=w5309:i32)
            n719 = Add(x=w5286, y=w5288) -> (x+y=w5285:i32)
            n720 = Add(x=w5277, y=w5278) -> (x+y=w5276:i32)
            n721 = Bundle(w5275, w5277) -> (w5273:cluster{i32, i32})  [unwired: 1 in]
            n722 = Bundle(w5286, w5289) -> (w5284:cluster{i32, i32})  [unwired: 1 in]
            n723 = Add(x=w5311, y=w5309) -> (x+y=w5310:i32)
            n724 = Bundle(w5311, w5312) -> (w5308:cluster{i32, i32})  [unwired: 1 in]
            n725 = Bundle(w5275, w5276) -> (w5274:cluster{i32, i32})  [unwired: 1 in]
            n726 = Bundle(w5285, w5289) -> (w5287:cluster{i32, i32})  [unwired: 1 in]
            n727 = call <vilib>:"Move Pen.vi"("new position"=w5308, "picture"=w5244) -> ("new picture"=w5307:picture)  [unwired: 3 in]
            n728 = Bundle(w5310, w5312) -> (w5313:cluster{i32, i32})  [unwired: 1 in]
            n729 = call <vilib>:"Draw Line.vi"("picture"=w5307, "end point"=w5313, "color(black)"=u32 16448250, "pen"=T1 {"Width"=3, "Style"=enum."Solid"}) -> ("new picture"=w5243:picture)  [unwired: 5 in]
            n730 = Multiply(x=w5240, y=10) -> (x*y=w5256:i32)
            n731 = Multiply(x=2, y=w5256) -> (x*y=w5257:i32)
            n732 = Add(x=w5242, y=0) -> (x+y=w5265:i32)
            n733 = Multiply(x=w5240, y=10) -> (x*y=w5268:i32)
            n734 = Add(x=w5241, y=w5268) -> (x+y=w5266:i32)
            n735 = Add(x=w5242, y=0) -> (x+y=w5253:i32)
            n736 = Add(x=w5241, y=w5257) -> (x+y=w5255:i32)
            n737 = Add(x=w5242, y=0) -> (x+y=w5299:i32)
            n738 = Add(x=w5241, y=0) -> (x+y=w5300:i32)
            n739 = Multiply(x=w5240, y=10) -> (x*y=w5298:i32)
            n740 = Add(x=w5266, y=w5268) -> (x+y=w5267:i32)
            n741 = Add(x=w5253, y=w5256) -> (x+y=w5252:i32)
            n742 = Add(x=w5300, y=w5298) -> (x+y=w5301:i32)
            n743 = Bundle(w5265, w5266) -> (w5263:cluster{i32, i32})  [unwired: 1 in]
            n744 = Bundle(w5253, w5255) -> (w5251:cluster{i32, i32})  [unwired: 1 in]
            n745 = Bundle(w5299, w5300) -> (w5296:cluster{i32, i32})  [unwired: 1 in]
            n746 = Bundle(w5265, w5267) -> (w5264:cluster{i32, i32})  [unwired: 1 in]
            n747 = Bundle(w5252, w5255) -> (w5254:cluster{i32, i32})  [unwired: 1 in]
            n748 = call <vilib>:"Move Pen.vi"("new position"=w5296, "picture"=w5243) -> ("new picture"=w5295:picture)  [unwired: 3 in]
            n749 = Bundle(w5299, w5301) -> (w5297:cluster{i32, i32})  [unwired: 1 in]
            n750 = call <vilib>:"Draw Line.vi"("picture"=w5295, "end point"=w5297, "color(black)"=u32 16448250, "pen"=T1 {"Width"=3, "Style"=enum."Solid"}) -> ("new picture"=w5239:picture)  [unwired: 5 in]
            n751 = call <vilib>:"Move Pen.vi"("new position"=w5284, "picture"=w5239) -> ("new picture"=w5283:picture)  [unwired: 3 in]
            n752 = call <vilib>:"Draw Line.vi"("picture"=w5283, "end point"=w5287, "color(black)"=u32 16448250, "pen"=T1 {"Width"=3, "Style"=enum."Solid"}) -> ("new picture"=w5238:picture)  [unwired: 5 in]
            n753 = call <vilib>:"Move Pen.vi"("new position"=w5263, "picture"=w5238) -> ("new picture"=w5262:picture)  [unwired: 3 in]
            n754 = call <vilib>:"Draw Line.vi"("picture"=w5262, "end point"=w5264, "color(black)"=u32 16448250, "pen"=T1 {"Width"=3, "Style"=enum."Solid"}) -> ("new picture"=w5237:picture)  [unwired: 5 in]
            n755 = call <vilib>:"Move Pen.vi"("new position"=w5273, "picture"=w5237) -> ("new picture"=w5272:picture)  [unwired: 3 in]
            n756 = call <vilib>:"Draw Line.vi"("picture"=w5272, "end point"=w5274, "color(black)"=u32 16448250, "pen"=T1 {"Width"=3, "Style"=enum."Solid"}) -> ("new picture"=w5236:picture)  [unwired: 5 in]
            n757 = call <vilib>:"Move Pen.vi"("new position"=w5251, "picture"=w5236) -> ("new picture"=w5250:picture)  [unwired: 3 in]
            n758 = call <vilib>:"Draw Line.vi"("picture"=w5250, "end point"=w5254, "color(black)"=u32 16448250, "pen"=T1 {"Width"=3, "Style"=enum."Solid"}) -> ("new picture"=w5235:picture)  [unwired: 5 in]
          }
          frame 7 {
            n759 = Add(x=w5319, y=0) -> (x+y=w5352:i32)
            n760 = Add(x=w5318, y=0) -> (x+y=w5353:i32)
            n761 = Multiply(x=w5317, y=10) -> (x*y=w5351:i32)
            n762 = Add(x=w5353, y=w5351) -> (x+y=w5354:i32)
            n763 = Add(x=w5319, y=0) -> (x+y=w5364:i32)
            n764 = Add(x=w5318, y=0) -> (x+y=w5365:i32)
            n765 = Bundle(w5352, w5353) -> (w5349:cluster{i32, i32})  [unwired: 1 in]
            n766 = Multiply(x=w5317, y=10) -> (x*y=w5362:i32)
            n767 = Add(x=w5364, y=w5362) -> (x+y=w5363:i32)
            n768 = Bundle(w5364, w5365) -> (w5361:cluster{i32, i32})  [unwired: 1 in]
            n769 = Bundle(w5352, w5354) -> (w5350:cluster{i32, i32})  [unwired: 1 in]
            n770 = call <vilib>:"Move Pen.vi"("new position"=w5361, "picture"=w5321) -> ("new picture"=w5360:picture)  [unwired: 3 in]
            n771 = Bundle(w5363, w5365) -> (w5366:cluster{i32, i32})  [unwired: 1 in]
            n772 = call <vilib>:"Draw Line.vi"("picture"=w5360, "end point"=w5366, "color(black)"=u32 16448250, "pen"=T1 {"Width"=3, "Style"=enum."Solid"}) -> ("new picture"=w5320:picture)  [unwired: 5 in]
            n773 = Multiply(x=w5317, y=10) -> (x*y=w5339:i32)
            n774 = Add(x=w5319, y=w5339) -> (x+y=w5340:i32)
            n775 = Add(x=w5318, y=0) -> (x+y=w5342:i32)
            n776 = Multiply(x=w5317, y=10) -> (x*y=w5331:i32)
            n777 = Add(x=w5319, y=w5331) -> (x+y=w5328:i32)
            n778 = Add(x=w5318, y=w5331) -> (x+y=w5330:i32)
            n779 = Add(x=w5342, y=w5339) -> (x+y=w5341:i32)
            n780 = Bundle(w5340, w5342) -> (w5337:cluster{i32, i32})  [unwired: 1 in]
            n781 = Add(x=w5330, y=w5331) -> (x+y=w5329:i32)
            n782 = Bundle(w5328, w5330) -> (w5326:cluster{i32, i32})  [unwired: 1 in]
            n783 = Bundle(w5340, w5341) -> (w5338:cluster{i32, i32})  [unwired: 1 in]
            n784 = call <vilib>:"Move Pen.vi"("new position"=w5326, "picture"=w5320) -> ("new picture"=w5325:picture)  [unwired: 3 in]
            n785 = Bundle(w5328, w5329) -> (w5327:cluster{i32, i32})  [unwired: 1 in]
            n786 = call <vilib>:"Draw Line.vi"("picture"=w5325, "end point"=w5327, "color(black)"=u32 16448250, "pen"=T1 {"Width"=3, "Style"=enum."Solid"}) -> ("new picture"=w5316:picture)  [unwired: 5 in]
            n787 = call <vilib>:"Move Pen.vi"("new position"=w5349, "picture"=w5316) -> ("new picture"=w5348:picture)  [unwired: 3 in]
            n788 = call <vilib>:"Draw Line.vi"("picture"=w5348, "end point"=w5350, "color(black)"=u32 16448250, "pen"=T1 {"Width"=3, "Style"=enum."Solid"}) -> ("new picture"=w5315:picture)  [unwired: 5 in]
            n789 = call <vilib>:"Move Pen.vi"("new position"=w5337, "picture"=w5315) -> ("new picture"=w5336:picture)  [unwired: 3 in]
            n790 = call <vilib>:"Draw Line.vi"("picture"=w5336, "end point"=w5338, "color(black)"=u32 16448250, "pen"=T1 {"Width"=3, "Style"=enum."Solid"}) -> ("new picture"=w5314:picture)  [unwired: 5 in]
          }
          frame 8 {
            n791 = Add(x=w5375, y=0) -> (x+y=w5443:i32)
            n792 = Add(x=w5374, y=0) -> (x+y=w5444:i32)
            n793 = Add(x=w5375, y=0) -> (x+y=w5398:i32)
            n794 = Multiply(x=w5373, y=10) -> (x*y=w5442:i32)
            n795 = Multiply(x=w5373, y=10) -> (x*y=w5401:i32)
            n796 = Add(x=w5374, y=w5401) -> (x+y=w5399:i32)
            n797 = Add(x=w5375, y=0) -> (x+y=w5455:i32)
            n798 = Add(x=w5374, y=0) -> (x+y=w5456:i32)
            n799 = Multiply(x=w5373, y=10) -> (x*y=w5453:i32)
            n800 = Add(x=w5444, y=w5442) -> (x+y=w5445:i32)
            n801 = Add(x=w5399, y=w5401) -> (x+y=w5400:i32)
            n802 = Bundle(w5443, w5444) -> (w5440:cluster{i32, i32})  [unwired: 1 in]
            n803 = Bundle(w5398, w5399) -> (w5396:cluster{i32, i32})  [unwired: 1 in]
            n804 = Multiply(x=w5373, y=10) -> (x*y=w5389:i32)
            n805 = Multiply(x=2, y=w5389) -> (x*y=w5390:i32)
            n806 = Add(x=w5455, y=w5453) -> (x+y=w5454:i32)
            n807 = Bundle(w5455, w5456) -> (w5452:cluster{i32, i32})  [unwired: 1 in]
            n808 = Add(x=w5375, y=0) -> (x+y=w5386:i32)
            n809 = Add(x=w5374, y=w5390) -> (x+y=w5388:i32)
            n810 = Add(x=w5386, y=w5389) -> (x+y=w5385:i32)
            n811 = Bundle(w5443, w5445) -> (w5441:cluster{i32, i32})  [unwired: 1 in]
            n812 = Bundle(w5398, w5400) -> (w5397:cluster{i32, i32})  [unwired: 1 in]
            n813 = Bundle(w5386, w5388) -> (w5384:cluster{i32, i32})  [unwired: 1 in]
            n814 = call <vilib>:"Move Pen.vi"("new position"=w5452, "picture"=w5377) -> ("new picture"=w5451:picture)  [unwired: 3 in]
            n815 = Bundle(w5454, w5456) -> (w5457:cluster{i32, i32})  [unwired: 1 in]
            n816 = Bundle(w5385, w5388) -> (w5387:cluster{i32, i32})  [unwired: 1 in]
            n817 = call <vilib>:"Draw Line.vi"("picture"=w5451, "end point"=w5457, "color(black)"=u32 16448250, "pen"=T1 {"Width"=3, "Style"=enum."Solid"}) -> ("new picture"=w5376:picture)  [unwired: 5 in]
            n818 = Multiply(x=w5373, y=10) -> (x*y=w5421:i32)
            n819 = Multiply(x=w5373, y=10) -> (x*y=w5430:i32)
            n820 = Add(x=w5375, y=0) -> (x+y=w5419:i32)
            n821 = Multiply(x=w5373, y=10) -> (x*y=w5411:i32)
            n822 = Add(x=w5374, y=w5421) -> (x+y=w5422:i32)
            n823 = Add(x=w5375, y=w5430) -> (x+y=w5431:i32)
            n824 = Add(x=w5374, y=0) -> (x+y=w5433:i32)
            n825 = Add(x=w5375, y=w5411) -> (x+y=w5408:i32)
            n826 = Add(x=w5374, y=w5411) -> (x+y=w5410:i32)
            n827 = Add(x=w5419, y=w5421) -> (x+y=w5418:i32)
            n828 = Bundle(w5419, w5422) -> (w5417:cluster{i32, i32})  [unwired: 1 in]
            n829 = Add(x=w5433, y=w5430) -> (x+y=w5432:i32)
            n830 = Add(x=w5410, y=w5411) -> (x+y=w5409:i32)
            n831 = Bundle(w5431, w5433) -> (w5428:cluster{i32, i32})  [unwired: 1 in]
            n832 = Bundle(w5408, w5410) -> (w5406:cluster{i32, i32})  [unwired: 1 in]
            n833 = call <vilib>:"Move Pen.vi"("new position"=w5417, "picture"=w5376) -> ("new picture"=w5416:picture)  [unwired: 3 in]
            n834 = Bundle(w5418, w5422) -> (w5420:cluster{i32, i32})  [unwired: 1 in]
            n835 = Bundle(w5431, w5432) -> (w5429:cluster{i32, i32})  [unwired: 1 in]
            n836 = Bundle(w5408, w5409) -> (w5407:cluster{i32, i32})  [unwired: 1 in]
            n837 = call <vilib>:"Draw Line.vi"("picture"=w5416, "end point"=w5420, "color(black)"=u32 16448250, "pen"=T1 {"Width"=3, "Style"=enum."Solid"}) -> ("new picture"=w5372:picture)  [unwired: 5 in]
            n838 = call <vilib>:"Move Pen.vi"("new position"=w5440, "picture"=w5372) -> ("new picture"=w5439:picture)  [unwired: 3 in]
            n839 = call <vilib>:"Draw Line.vi"("picture"=w5439, "end point"=w5441, "color(black)"=u32 16448250, "pen"=T1 {"Width"=3, "Style"=enum."Solid"}) -> ("new picture"=w5371:picture)  [unwired: 5 in]
            n840 = call <vilib>:"Move Pen.vi"("new position"=w5428, "picture"=w5371) -> ("new picture"=w5427:picture)  [unwired: 3 in]
            n841 = call <vilib>:"Draw Line.vi"("picture"=w5427, "end point"=w5429, "color(black)"=u32 16448250, "pen"=T1 {"Width"=3, "Style"=enum."Solid"}) -> ("new picture"=w5370:picture)  [unwired: 5 in]
            n842 = call <vilib>:"Move Pen.vi"("new position"=w5396, "picture"=w5370) -> ("new picture"=w5395:picture)  [unwired: 3 in]
            n843 = call <vilib>:"Draw Line.vi"("picture"=w5395, "end point"=w5397, "color(black)"=u32 16448250, "pen"=T1 {"Width"=3, "Style"=enum."Solid"}) -> ("new picture"=w5369:picture)  [unwired: 5 in]
            n844 = call <vilib>:"Move Pen.vi"("new position"=w5406, "picture"=w5369) -> ("new picture"=w5405:picture)  [unwired: 3 in]
            n845 = call <vilib>:"Draw Line.vi"("picture"=w5405, "end point"=w5407, "color(black)"=u32 16448250, "pen"=T1 {"Width"=3, "Style"=enum."Solid"}) -> ("new picture"=w5368:picture)  [unwired: 5 in]
            n846 = call <vilib>:"Move Pen.vi"("new position"=w5384, "picture"=w5368) -> ("new picture"=w5383:picture)  [unwired: 3 in]
            n847 = call <vilib>:"Draw Line.vi"("picture"=w5383, "end point"=w5387, "color(black)"=u32 16448250, "pen"=T1 {"Width"=3, "Style"=enum."Solid"}) -> ("new picture"=w5367:picture)  [unwired: 5 in]
          }
          frame 9 {
            n848 = Add(x=w5464, y=0) -> (x+y=w5508:i32)
            n849 = Add(x=w5463, y=0) -> (x+y=w5509:i32)
            n850 = Add(x=w5464, y=0) -> (x+y=w5520:i32)
            n851 = Add(x=w5463, y=0) -> (x+y=w5521:i32)
            n852 = Multiply(x=w5462, y=10) -> (x*y=w5507:i32)
            n853 = Multiply(x=w5462, y=10) -> (x*y=w5518:i32)
            n854 = Add(x=w5509, y=w5507) -> (x+y=w5510:i32)
            n855 = Add(x=w5520, y=w5518) -> (x+y=w5519:i32)
            n856 = Bundle(w5508, w5509) -> (w5505:cluster{i32, i32})  [unwired: 1 in]
            n857 = Bundle(w5520, w5521) -> (w5517:cluster{i32, i32})  [unwired: 1 in]
            n858 = Bundle(w5508, w5510) -> (w5506:cluster{i32, i32})  [unwired: 1 in]
            n859 = call <vilib>:"Move Pen.vi"("new position"=w5517, "picture"=w5466) -> ("new picture"=w5516:picture)  [unwired: 3 in]
            n860 = Bundle(w5519, w5521) -> (w5522:cluster{i32, i32})  [unwired: 1 in]
            n861 = Multiply(x=w5462, y=10) -> (x*y=w5476:i32)
            n862 = Add(x=w5464, y=w5476) -> (x+y=w5473:i32)
            n863 = Add(x=w5463, y=w5476) -> (x+y=w5475:i32)
            n864 = Add(x=w5475, y=w5476) -> (x+y=w5474:i32)
            n865 = Bundle(w5473, w5475) -> (w5471:cluster{i32, i32})  [unwired: 1 in]
            n866 = call <vilib>:"Draw Line.vi"("picture"=w5516, "end point"=w5522, "color(black)"=u32 16448250, "pen"=T1 {"Width"=3, "Style"=enum."Solid"}) -> ("new picture"=w5465:picture)  [unwired: 5 in]
            n867 = Bundle(w5473, w5474) -> (w5472:cluster{i32, i32})  [unwired: 1 in]
            n868 = Multiply(x=w5462, y=10) -> (x*y=w5495:i32)
            n869 = Add(x=w5464, y=w5495) -> (x+y=w5496:i32)
            n870 = Add(x=w5463, y=0) -> (x+y=w5498:i32)
            n871 = Multiply(x=w5462, y=10) -> (x*y=w5486:i32)
            n872 = Add(x=w5464, y=0) -> (x+y=w5484:i32)
            n873 = Add(x=w5463, y=w5486) -> (x+y=w5487:i32)
            n874 = Add(x=w5498, y=w5495) -> (x+y=w5497:i32)
            n875 = Add(x=w5484, y=w5486) -> (x+y=w5483:i32)
            n876 = Bundle(w5496, w5498) -> (w5493:cluster{i32, i32})  [unwired: 1 in]
            n877 = Bundle(w5484, w5487) -> (w5482:cluster{i32, i32})  [unwired: 1 in]
            n878 = Bundle(w5496, w5497) -> (w5494:cluster{i32, i32})  [unwired: 1 in]
            n879 = call <vilib>:"Move Pen.vi"("new position"=w5482, "picture"=w5465) -> ("new picture"=w5481:picture)  [unwired: 3 in]
            n880 = Bundle(w5483, w5487) -> (w5485:cluster{i32, i32})  [unwired: 1 in]
            n881 = call <vilib>:"Draw Line.vi"("picture"=w5481, "end point"=w5485, "color(black)"=u32 16448250, "pen"=T1 {"Width"=3, "Style"=enum."Solid"}) -> ("new picture"=w5461:picture)  [unwired: 5 in]
            n882 = call <vilib>:"Move Pen.vi"("new position"=w5505, "picture"=w5461) -> ("new picture"=w5504:picture)  [unwired: 3 in]
            n883 = call <vilib>:"Draw Line.vi"("picture"=w5504, "end point"=w5506, "color(black)"=u32 16448250, "pen"=T1 {"Width"=3, "Style"=enum."Solid"}) -> ("new picture"=w5460:picture)  [unwired: 5 in]
            n884 = call <vilib>:"Move Pen.vi"("new position"=w5493, "picture"=w5460) -> ("new picture"=w5492:picture)  [unwired: 3 in]
            n885 = call <vilib>:"Draw Line.vi"("picture"=w5492, "end point"=w5494, "color(black)"=u32 16448250, "pen"=T1 {"Width"=3, "Style"=enum."Solid"}) -> ("new picture"=w5459:picture)  [unwired: 5 in]
            n886 = call <vilib>:"Move Pen.vi"("new position"=w5471, "picture"=w5459) -> ("new picture"=w5470:picture)  [unwired: 3 in]
            n887 = call <vilib>:"Draw Line.vi"("picture"=w5470, "end point"=w5472, "color(black)"=u32 16448250, "pen"=T1 {"Width"=3, "Style"=enum."Solid"}) -> ("new picture"=w5458:picture)  [unwired: 5 in]
          }
        }
        n888 = case shown="9" w150 {
          tunnel: 350 -> [w4239 w4313 w4343 w4411 w4476 w4528 w4596 w4673 w4729 w4818]
          tunnel: 10 -> [w4238 w4312 w4342 w4410 w4475 w4527 w4595 w4672 w4728 w4817]
          tunnel: 3 -> [w4237 w4311 w4341 w4409 w4474 w4526 w4594 w4671 w4727 w4816]
          tunnel: w179 -> [w4240 w4315 w4345 w4412 w4477 w4530 w4598 w4675 w4731 w4820]
          tunnel: [w4231 w4310 w4337 w4404 w4470 w4522 w4589 w4668 w4721 w4812] -> w164
          frame 0, Default {
            n889 = Add(x=w4239, y=0) -> (x+y=w4295:i32)
            n890 = Add(x=w4238, y=0) -> (x+y=w4296:i32)
            n891 = Multiply(x=w4237, y=10) -> (x*y=w4294:i32)
            n892 = Add(x=w4239, y=0) -> (x+y=w4261:i32)
            n893 = Multiply(x=w4237, y=10) -> (x*y=w4264:i32)
            n894 = Add(x=w4238, y=w4264) -> (x+y=w4262:i32)
            n895 = Add(x=w4296, y=w4294) -> (x+y=w4297:i32)
            n896 = Add(x=w4262, y=w4264) -> (x+y=w4263:i32)
            n897 = Bundle(w4295, w4296) -> (w4292:cluster{i32, i32})  [unwired: 1 in]
            n898 = Bundle(w4261, w4262) -> (w4259:cluster{i32, i32})  [unwired: 1 in]
            n899 = Bundle(w4295, w4297) -> (w4293:cluster{i32, i32})  [unwired: 1 in]
            n900 = Bundle(w4261, w4263) -> (w4260:cluster{i32, i32})  [unwired: 1 in]
            n901 = Multiply(x=w4237, y=10) -> (x*y=w4252:i32)
            n902 = Multiply(x=2, y=w4252) -> (x*y=w4253:i32)
            n903 = Add(x=w4239, y=0) -> (x+y=w4307:i32)
            n904 = Add(x=w4238, y=0) -> (x+y=w4308:i32)
            n905 = Add(x=w4239, y=0) -> (x+y=w4249:i32)
            n906 = Add(x=w4238, y=w4253) -> (x+y=w4251:i32)
            n907 = Multiply(x=w4237, y=10) -> (x*y=w4305:i32)
            n908 = Add(x=w4249, y=w4252) -> (x+y=w4248:i32)
            n909 = Add(x=w4307, y=w4305) -> (x+y=w4306:i32)
            n910 = Bundle(w4307, w4308) -> (w4304:cluster{i32, i32})  [unwired: 1 in]
            n911 = Bundle(w4249, w4251) -> (w4247:cluster{i32, i32})  [unwired: 1 in]
            n912 = call <vilib>:"Move Pen.vi"("new position"=w4304, "picture"=w4240) -> ("new picture"=w4303:picture)  [unwired: 3 in]
            n913 = Bundle(w4306, w4308) -> (w4309:cluster{i32, i32})  [unwired: 1 in]
            n914 = Bundle(w4248, w4251) -> (w4250:cluster{i32, i32})  [unwired: 1 in]
            n915 = Multiply(x=w4237, y=10) -> (x*y=w4282:i32)
            n916 = Add(x=w4239, y=w4282) -> (x+y=w4283:i32)
            n917 = Add(x=w4238, y=0) -> (x+y=w4285:i32)
            n918 = Multiply(x=w4237, y=10) -> (x*y=w4274:i32)
            n919 = Add(x=w4239, y=w4274) -> (x+y=w4271:i32)
            n920 = Add(x=w4238, y=w4274) -> (x+y=w4273:i32)
            n921 = Add(x=w4285, y=w4282) -> (x+y=w4284:i32)
            n922 = Bundle(w4283, w4285) -> (w4280:cluster{i32, i32})  [unwired: 1 in]
            n923 = call <vilib>:"Draw Line.vi"("picture"=w4303, "end point"=w4309, "color(black)"=u32 16448250, "pen"=T1 {"Width"=3, "Style"=enum."Solid"}) -> ("new picture"=w4236:picture)  [unwired: 5 in]
            n924 = call <vilib>:"Move Pen.vi"("new position"=w4292, "picture"=w4236) -> ("new picture"=w4291:picture)  [unwired: 3 in]
            n925 = call <vilib>:"Draw Line.vi"("picture"=w4291, "end point"=w4293, "color(black)"=u32 16448250, "pen"=T1 {"Width"=3, "Style"=enum."Solid"}) -> ("new picture"=w4235:picture)  [unwired: 5 in]
            n926 = Add(x=w4273, y=w4274) -> (x+y=w4272:i32)
            n927 = Bundle(w4271, w4273) -> (w4269:cluster{i32, i32})  [unwired: 1 in]
            n928 = call <vilib>:"Move Pen.vi"("new position"=w4280, "picture"=w4235) -> ("new picture"=w4279:picture)  [unwired: 3 in]
            n929 = Bundle(w4283, w4284) -> (w4281:cluster{i32, i32})  [unwired: 1 in]
            n930 = Bundle(w4271, w4272) -> (w4270:cluster{i32, i32})  [unwired: 1 in]
            n931 = call <vilib>:"Draw Line.vi"("picture"=w4279, "end point"=w4281, "color(black)"=u32 16448250, "pen"=T1 {"Width"=3, "Style"=enum."Solid"}) -> ("new picture"=w4234:picture)  [unwired: 5 in]
            n932 = call <vilib>:"Move Pen.vi"("new position"=w4259, "picture"=w4234) -> ("new picture"=w4258:picture)  [unwired: 3 in]
            n933 = call <vilib>:"Draw Line.vi"("picture"=w4258, "end point"=w4260, "color(black)"=u32 16448250, "pen"=T1 {"Width"=3, "Style"=enum."Solid"}) -> ("new picture"=w4233:picture)  [unwired: 5 in]
            n934 = call <vilib>:"Move Pen.vi"("new position"=w4269, "picture"=w4233) -> ("new picture"=w4268:picture)  [unwired: 3 in]
            n935 = call <vilib>:"Draw Line.vi"("picture"=w4268, "end point"=w4270, "color(black)"=u32 16448250, "pen"=T1 {"Width"=3, "Style"=enum."Solid"}) -> ("new picture"=w4232:picture)  [unwired: 5 in]
            n936 = call <vilib>:"Move Pen.vi"("new position"=w4247, "picture"=w4232) -> ("new picture"=w4246:picture)  [unwired: 3 in]
            n937 = call <vilib>:"Draw Line.vi"("picture"=w4246, "end point"=w4250, "color(black)"=u32 16448250, "pen"=T1 {"Width"=3, "Style"=enum."Solid"}) -> ("new picture"=w4231:picture)  [unwired: 5 in]
          }
          frame 1 {
            n938 = Multiply(x=w4311, y=10) -> (x*y=w4333:i32)
            n939 = Add(x=w4313, y=w4333) -> (x+y=w4334:i32)
            n940 = Add(x=w4312, y=0) -> (x+y=w4336:i32)
            n941 = Add(x=w4336, y=w4333) -> (x+y=w4335:i32)
            n942 = Bundle(w4334, w4336) -> (w4331:cluster{i32, i32})  [unwired: 1 in]
            n943 = call <vilib>:"Move Pen.vi"("new position"=w4331, "picture"=w4315) -> ("new picture"=w4330:picture)  [unwired: 3 in]
            n944 = Bundle(w4334, w4335) -> (w4332:cluster{i32, i32})  [unwired: 1 in]
            n945 = call <vilib>:"Draw Line.vi"("picture"=w4330, "end point"=w4332, "color(black)"=u32 16448250, "pen"=T1 {"Width"=3, "Style"=enum."Solid"}) -> ("new picture"=w4314:picture)  [unwired: 5 in]
            n946 = Multiply(x=w4311, y=10) -> (x*y=w4325:i32)
            n947 = Add(x=w4313, y=w4325) -> (x+y=w4322:i32)
            n948 = Add(x=w4312, y=w4325) -> (x+y=w4324:i32)
            n949 = Add(x=w4324, y=w4325) -> (x+y=w4323:i32)
            n950 = Bundle(w4322, w4324) -> (w4320:cluster{i32, i32})  [unwired: 1 in]
            n951 = call <vilib>:"Move Pen.vi"("new position"=w4320, "picture"=w4314) -> ("new picture"=w4319:picture)  [unwired: 3 in]
            n952 = Bundle(w4322, w4323) -> (w4321:cluster{i32, i32})  [unwired: 1 in]
            n953 = call <vilib>:"Draw Line.vi"("picture"=w4319, "end point"=w4321, "color(black)"=u32 16448250, "pen"=T1 {"Width"=3, "Style"=enum."Solid"}) -> ("new picture"=w4310:picture)  [unwired: 5 in]
          }
          frame 2 {
            n954 = Multiply(x=w4341, y=10) -> (x*y=w4379:i32)
            n955 = Add(x=w4343, y=0) -> (x+y=w4377:i32)
            n956 = Add(x=w4342, y=w4379) -> (x+y=w4380:i32)
            n957 = Add(x=w4343, y=0) -> (x+y=w4401:i32)
            n958 = Add(x=w4342, y=0) -> (x+y=w4402:i32)
            n959 = Multiply(x=w4341, y=10) -> (x*y=w4399:i32)
            n960 = Add(x=w4377, y=w4379) -> (x+y=w4376:i32)
            n961 = Add(x=w4401, y=w4399) -> (x+y=w4400:i32)
            n962 = Bundle(w4377, w4380) -> (w4375:cluster{i32, i32})  [unwired: 1 in]
            n963 = Bundle(w4401, w4402) -> (w4398:cluster{i32, i32})  [unwired: 1 in]
            n964 = Bundle(w4376, w4380) -> (w4378:cluster{i32, i32})  [unwired: 1 in]
            n965 = call <vilib>:"Move Pen.vi"("new position"=w4398, "picture"=w4345) -> ("new picture"=w4397:picture)  [unwired: 3 in]
            n966 = Bundle(w4400, w4402) -> (w4403:cluster{i32, i32})  [unwired: 1 in]
            n967 = Multiply(x=w4341, y=10) -> (x*y=w4357:i32)
            n968 = Multiply(x=2, y=w4357) -> (x*y=w4358:i32)
            n969 = Add(x=w4343, y=0) -> (x+y=w4354:i32)
            n970 = Add(x=w4342, y=w4358) -> (x+y=w4356:i32)
            n971 = Add(x=w4354, y=w4357) -> (x+y=w4353:i32)
            n972 = Bundle(w4354, w4356) -> (w4352:cluster{i32, i32})  [unwired: 1 in]
            n973 = call <vilib>:"Draw Line.vi"("picture"=w4397, "end point"=w4403, "color(black)"=u32 16448250, "pen"=T1 {"Width"=3, "Style"=enum."Solid"}) -> ("new picture"=w4344:picture)  [unwired: 5 in]
            n974 = Bundle(w4353, w4356) -> (w4355:cluster{i32, i32})  [unwired: 1 in]
            n975 = Multiply(x=w4341, y=10) -> (x*y=w4388:i32)
            n976 = Add(x=w4343, y=0) -> (x+y=w4366:i32)
            n977 = Add(x=w4343, y=w4388) -> (x+y=w4389:i32)
            n978 = Add(x=w4342, y=0) -> (x+y=w4391:i32)
            n979 = Multiply(x=w4341, y=10) -> (x*y=w4369:i32)
            n980 = Add(x=w4342, y=w4369) -> (x+y=w4367:i32)
            n981 = Add(x=w4367, y=w4369) -> (x+y=w4368:i32)
            n982 = Add(x=w4391, y=w4388) -> (x+y=w4390:i32)
            n983 = Bundle(w4366, w4367) -> (w4364:cluster{i32, i32})  [unwired: 1 in]
            n984 = Bundle(w4389, w4391) -> (w4386:cluster{i32, i32})  [unwired: 1 in]
            n985 = call <vilib>:"Move Pen.vi"("new position"=w4386, "picture"=w4344) -> ("new picture"=w4385:picture)  [unwired: 3 in]
            n986 = Bundle(w4366, w4368) -> (w4365:cluster{i32, i32})  [unwired: 1 in]
            n987 = Bundle(w4389, w4390) -> (w4387:cluster{i32, i32})  [unwired: 1 in]
            n988 = call <vilib>:"Draw Line.vi"("picture"=w4385, "end point"=w4387, "color(black)"=u32 16448250, "pen"=T1 {"Width"=3, "Style"=enum."Solid"}) -> ("new picture"=w4340:picture)  [unwired: 5 in]
            n989 = call <vilib>:"Move Pen.vi"("new position"=w4375, "picture"=w4340) -> ("new picture"=w4374:picture)  [unwired: 3 in]
            n990 = call <vilib>:"Draw Line.vi"("picture"=w4374, "end point"=w4378, "color(black)"=u32 16448250, "pen"=T1 {"Width"=3, "Style"=enum."Solid"}) -> ("new picture"=w4339:picture)  [unwired: 5 in]
            n991 = call <vilib>:"Move Pen.vi"("new position"=w4364, "picture"=w4339) -> ("new picture"=w4363:picture)  [unwired: 3 in]
            n992 = call <vilib>:"Draw Line.vi"("picture"=w4363, "end point"=w4365, "color(black)"=u32 16448250, "pen"=T1 {"Width"=3, "Style"=enum."Solid"}) -> ("new picture"=w4338:picture)  [unwired: 5 in]
            n993 = call <vilib>:"Move Pen.vi"("new position"=w4352, "picture"=w4338) -> ("new picture"=w4351:picture)  [unwired: 3 in]
            n994 = call <vilib>:"Draw Line.vi"("picture"=w4351, "end point"=w4355, "color(black)"=u32 16448250, "pen"=T1 {"Width"=3, "Style"=enum."Solid"}) -> ("new picture"=w4337:picture)  [unwired: 5 in]
          }
          frame 3 {
            n995 = Multiply(x=w4409, y=10) -> (x*y=w4445:i32)
            n996 = Add(x=w4411, y=0) -> (x+y=w4443:i32)
            n997 = Add(x=w4410, y=w4445) -> (x+y=w4446:i32)
            n998 = Add(x=w4411, y=0) -> (x+y=w4467:i32)
            n999 = Add(x=w4410, y=0) -> (x+y=w4468:i32)
            n1000 = Multiply(x=w4409, y=10) -> (x*y=w4465:i32)
            n1001 = Add(x=w4443, y=w4445) -> (x+y=w4442:i32)
            n1002 = Add(x=w4467, y=w4465) -> (x+y=w4466:i32)
            n1003 = Bundle(w4443, w4446) -> (w4441:cluster{i32, i32})  [unwired: 1 in]
            n1004 = Bundle(w4467, w4468) -> (w4464:cluster{i32, i32})  [unwired: 1 in]
            n1005 = call <vilib>:"Move Pen.vi"("new position"=w4464, "picture"=w4412) -> ("new picture"=w4463:picture)  [unwired: 3 in]
            n1006 = Bundle(w4442, w4446) -> (w4444:cluster{i32, i32})  [unwired: 1 in]
            n1007 = Bundle(w4466, w4468) -> (w4469:cluster{i32, i32})  [unwired: 1 in]
            n1008 = Multiply(x=w4409, y=10) -> (x*y=w4424:i32)
            n1009 = Multiply(x=2, y=w4424) -> (x*y=w4425:i32)
            n1010 = Add(x=w4411, y=0) -> (x+y=w4421:i32)
            n1011 = Add(x=w4410, y=w4425) -> (x+y=w4423:i32)
            n1012 = Add(x=w4421, y=w4424) -> (x+y=w4420:i32)
            n1013 = call <vilib>:"Draw Line.vi"("picture"=w4463, "end point"=w4469, "color(black)"=u32 16448250, "pen"=T1 {"Width"=3, "Style"=enum."Solid"}) -> ("new picture"=w4408:picture)  [unwired: 5 in]
            n1014 = Bundle(w4421, w4423) -> (w4419:cluster{i32, i32})  [unwired: 1 in]
            n1015 = Bundle(w4420, w4423) -> (w4422:cluster{i32, i32})  [unwired: 1 in]
            n1016 = Multiply(x=w4409, y=10) -> (x*y=w4435:i32)
            n1017 = Add(x=w4411, y=w4435) -> (x+y=w4432:i32)
            n1018 = Add(x=w4410, y=w4435) -> (x+y=w4434:i32)
            n1019 = Multiply(x=w4409, y=10) -> (x*y=w4454:i32)
            n1020 = Add(x=w4411, y=w4454) -> (x+y=w4455:i32)
            n1021 = Add(x=w4410, y=0) -> (x+y=w4457:i32)
            n1022 = Add(x=w4434, y=w4435) -> (x+y=w4433:i32)
            n1023 = Bundle(w4432, w4434) -> (w4430:cluster{i32, i32})  [unwired: 1 in]
            n1024 = Add(x=w4457, y=w4454) -> (x+y=w4456:i32)
            n1025 = Bundle(w4455, w4457) -> (w4452:cluster{i32, i32})  [unwired: 1 in]
            n1026 = Bundle(w4432, w4433) -> (w4431:cluster{i32, i32})  [unwired: 1 in]
            n1027 = call <vilib>:"Move Pen.vi"("new position"=w4452, "picture"=w4408) -> ("new picture"=w4451:picture)  [unwired: 3 in]
            n1028 = Bundle(w4455, w4456) -> (w4453:cluster{i32, i32})  [unwired: 1 in]
            n1029 = call <vilib>:"Draw Line.vi"("picture"=w4451, "end point"=w4453, "color(black)"=u32 16448250, "pen"=T1 {"Width"=3, "Style"=enum."Solid"}) -> ("new picture"=w4407:picture)  [unwired: 5 in]
            n1030 = call <vilib>:"Move Pen.vi"("new position"=w4441, "picture"=w4407) -> ("new picture"=w4440:picture)  [unwired: 3 in]
            n1031 = call <vilib>:"Draw Line.vi"("picture"=w4440, "end point"=w4444, "color(black)"=u32 16448250, "pen"=T1 {"Width"=3, "Style"=enum."Solid"}) -> ("new picture"=w4406:picture)  [unwired: 5 in]
            n1032 = call <vilib>:"Move Pen.vi"("new position"=w4430, "picture"=w4406) -> ("new picture"=w4429:picture)  [unwired: 3 in]
            n1033 = call <vilib>:"Draw Line.vi"("picture"=w4429, "end point"=w4431, "color(black)"=u32 16448250, "pen"=T1 {"Width"=3, "Style"=enum."Solid"}) -> ("new picture"=w4405:picture)  [unwired: 5 in]
            n1034 = call <vilib>:"Move Pen.vi"("new position"=w4419, "picture"=w4405) -> ("new picture"=w4418:picture)  [unwired: 3 in]
            n1035 = call <vilib>:"Draw Line.vi"("picture"=w4418, "end point"=w4422, "color(black)"=u32 16448250, "pen"=T1 {"Width"=3, "Style"=enum."Solid"}) -> ("new picture"=w4404:picture)  [unwired: 5 in]
          }
          frame 4 {
            n1036 = Add(x=w4476, y=0) -> (x+y=w4519:i32)
            n1037 = Add(x=w4475, y=0) -> (x+y=w4520:i32)
            n1038 = Multiply(x=w4474, y=10) -> (x*y=w4518:i32)
            n1039 = Add(x=w4520, y=w4518) -> (x+y=w4521:i32)
            n1040 = Bundle(w4519, w4520) -> (w4516:cluster{i32, i32})  [unwired: 1 in]
            n1041 = call <vilib>:"Move Pen.vi"("new position"=w4516, "picture"=w4477) -> ("new picture"=w4515:picture)  [unwired: 3 in]
            n1042 = Bundle(w4519, w4521) -> (w4517:cluster{i32, i32})  [unwired: 1 in]
            n1043 = Multiply(x=w4474, y=10) -> (x*y=w4497:i32)
            n1044 = Add(x=w4476, y=0) -> (x+y=w4495:i32)
            n1045 = Add(x=w4475, y=w4497) -> (x+y=w4498:i32)
            n1046 = Add(x=w4495, y=w4497) -> (x+y=w4494:i32)
            n1047 = Bundle(w4495, w4498) -> (w4493:cluster{i32, i32})  [unwired: 1 in]
            n1048 = call <vilib>:"Draw Line.vi"("picture"=w4515, "end point"=w4517, "color(black)"=u32 16448250, "pen"=T1 {"Width"=3, "Style"=enum."Solid"}) -> ("new picture"=w4471:picture)  [unwired: 5 in]
            n1049 = Multiply(x=w4474, y=10) -> (x*y=w4487:i32)
            n1050 = Add(x=w4476, y=w4487) -> (x+y=w4484:i32)
            n1051 = Add(x=w4475, y=w4487) -> (x+y=w4486:i32)
            n1052 = Bundle(w4494, w4498) -> (w4496:cluster{i32, i32})  [unwired: 1 in]
            n1053 = Add(x=w4486, y=w4487) -> (x+y=w4485:i32)
            n1054 = Bundle(w4484, w4486) -> (w4482:cluster{i32, i32})  [unwired: 1 in]
            n1055 = Multiply(x=w4474, y=10) -> (x*y=w4506:i32)
            n1056 = Add(x=w4476, y=w4506) -> (x+y=w4507:i32)
            n1057 = Add(x=w4475, y=0) -> (x+y=w4509:i32)
            n1058 = Add(x=w4509, y=w4506) -> (x+y=w4508:i32)
            n1059 = Bundle(w4484, w4485) -> (w4483:cluster{i32, i32})  [unwired: 1 in]
            n1060 = Bundle(w4507, w4509) -> (w4504:cluster{i32, i32})  [unwired: 1 in]
            n1061 = call <vilib>:"Move Pen.vi"("new position"=w4504, "picture"=w4471) -> ("new picture"=w4503:picture)  [unwired: 3 in]
            n1062 = Bundle(w4507, w4508) -> (w4505:cluster{i32, i32})  [unwired: 1 in]
            n1063 = call <vilib>:"Draw Line.vi"("picture"=w4503, "end point"=w4505, "color(black)"=u32 16448250, "pen"=T1 {"Width"=3, "Style"=enum."Solid"}) -> ("new picture"=w4473:picture)  [unwired: 5 in]
            n1064 = call <vilib>:"Move Pen.vi"("new position"=w4493, "picture"=w4473) -> ("new picture"=w4492:picture)  [unwired: 3 in]
            n1065 = call <vilib>:"Draw Line.vi"("picture"=w4492, "end point"=w4496, "color(black)"=u32 16448250, "pen"=T1 {"Width"=3, "Style"=enum."Solid"}) -> ("new picture"=w4472:picture)  [unwired: 5 in]
            n1066 = call <vilib>:"Move Pen.vi"("new position"=w4482, "picture"=w4472) -> ("new picture"=w4481:picture)  [unwired: 3 in]
            n1067 = call <vilib>:"Draw Line.vi"("picture"=w4481, "end point"=w4483, "color(black)"=u32 16448250, "pen"=T1 {"Width"=3, "Style"=enum."Solid"}) -> ("new picture"=w4470:picture)  [unwired: 5 in]
          }
          frame 5 {
            n1068 = Multiply(x=w4526, y=10) -> (x*y=w4563:i32)
            n1069 = Add(x=w4528, y=0) -> (x+y=w4561:i32)
            n1070 = Add(x=w4527, y=w4563) -> (x+y=w4564:i32)
            n1071 = Add(x=w4528, y=0) -> (x+y=w4586:i32)
            n1072 = Add(x=w4527, y=0) -> (x+y=w4587:i32)
            n1073 = Add(x=w4561, y=w4563) -> (x+y=w4560:i32)
            n1074 = Multiply(x=w4526, y=10) -> (x*y=w4584:i32)
            n1075 = Bundle(w4561, w4564) -> (w4559:cluster{i32, i32})  [unwired: 1 in]
            n1076 = Add(x=w4586, y=w4584) -> (x+y=w4585:i32)
            n1077 = Bundle(w4586, w4587) -> (w4583:cluster{i32, i32})  [unwired: 1 in]
            n1078 = Bundle(w4560, w4564) -> (w4562:cluster{i32, i32})  [unwired: 1 in]
            n1079 = call <vilib>:"Move Pen.vi"("new position"=w4583, "picture"=w4530) -> ("new picture"=w4582:picture)  [unwired: 3 in]
            n1080 = Bundle(w4585, w4587) -> (w4588:cluster{i32, i32})  [unwired: 1 in]
            n1081 = Multiply(x=w4526, y=10) -> (x*y=w4542:i32)
            n1082 = Multiply(x=2, y=w4542) -> (x*y=w4543:i32)
            n1083 = Add(x=w4528, y=0) -> (x+y=w4539:i32)
            n1084 = Add(x=w4527, y=w4543) -> (x+y=w4541:i32)
            n1085 = Add(x=w4539, y=w4542) -> (x+y=w4538:i32)
            n1086 = Bundle(w4539, w4541) -> (w4537:cluster{i32, i32})  [unwired: 1 in]
            n1087 = call <vilib>:"Draw Line.vi"("picture"=w4582, "end point"=w4588, "color(black)"=u32 16448250, "pen"=T1 {"Width"=3, "Style"=enum."Solid"}) -> ("new picture"=w4529:picture)  [unwired: 5 in]
            n1088 = Bundle(w4538, w4541) -> (w4540:cluster{i32, i32})  [unwired: 1 in]
            n1089 = Multiply(x=w4526, y=10) -> (x*y=w4553:i32)
            n1090 = Add(x=w4528, y=0) -> (x+y=w4574:i32)
            n1091 = Add(x=w4527, y=0) -> (x+y=w4575:i32)
            n1092 = Add(x=w4528, y=w4553) -> (x+y=w4550:i32)
            n1093 = Add(x=w4527, y=w4553) -> (x+y=w4552:i32)
            n1094 = Multiply(x=w4526, y=10) -> (x*y=w4573:i32)
            n1095 = Add(x=w4575, y=w4573) -> (x+y=w4576:i32)
            n1096 = Add(x=w4552, y=w4553) -> (x+y=w4551:i32)
            n1097 = Bundle(w4574, w4575) -> (w4571:cluster{i32, i32})  [unwired: 1 in]
            n1098 = Bundle(w4550, w4552) -> (w4548:cluster{i32, i32})  [unwired: 1 in]
            n1099 = call <vilib>:"Move Pen.vi"("new position"=w4571, "picture"=w4529) -> ("new picture"=w4570:picture)  [unwired: 3 in]
            n1100 = Bundle(w4574, w4576) -> (w4572:cluster{i32, i32})  [unwired: 1 in]
            n1101 = Bundle(w4550, w4551) -> (w4549:cluster{i32, i32})  [unwired: 1 in]
            n1102 = call <vilib>:"Draw Line.vi"("picture"=w4570, "end point"=w4572, "color(black)"=u32 16448250, "pen"=T1 {"Width"=3, "Style"=enum."Solid"}) -> ("new picture"=w4525:picture)  [unwired: 5 in]
            n1103 = call <vilib>:"Move Pen.vi"("new position"=w4559, "picture"=w4525) -> ("new picture"=w4558:picture)  [unwired: 3 in]
            n1104 = call <vilib>:"Draw Line.vi"("picture"=w4558, "end point"=w4562, "color(black)"=u32 16448250, "pen"=T1 {"Width"=3, "Style"=enum."Solid"}) -> ("new picture"=w4524:picture)  [unwired: 5 in]
            n1105 = call <vilib>:"Move Pen.vi"("new position"=w4548, "picture"=w4524) -> ("new picture"=w4547:picture)  [unwired: 3 in]
            n1106 = call <vilib>:"Draw Line.vi"("picture"=w4547, "end point"=w4549, "color(black)"=u32 16448250, "pen"=T1 {"Width"=3, "Style"=enum."Solid"}) -> ("new picture"=w4523:picture)  [unwired: 5 in]
            n1107 = call <vilib>:"Move Pen.vi"("new position"=w4537, "picture"=w4523) -> ("new picture"=w4536:picture)  [unwired: 3 in]
            n1108 = call <vilib>:"Draw Line.vi"("picture"=w4536, "end point"=w4540, "color(black)"=u32 16448250, "pen"=T1 {"Width"=3, "Style"=enum."Solid"}) -> ("new picture"=w4522:picture)  [unwired: 5 in]
          }
          frame 6 {
            n1109 = Multiply(x=w4594, y=10) -> (x*y=w4632:i32)
            n1110 = Multiply(x=w4594, y=10) -> (x*y=w4642:i32)
            n1111 = Add(x=w4596, y=w4632) -> (x+y=w4629:i32)
            n1112 = Add(x=w4595, y=w4632) -> (x+y=w4631:i32)
            n1113 = Add(x=w4596, y=0) -> (x+y=w4640:i32)
            n1114 = Add(x=w4595, y=w4642) -> (x+y=w4643:i32)
            n1115 = Add(x=w4596, y=0) -> (x+y=w4665:i32)
            n1116 = Add(x=w4595, y=0) -> (x+y=w4666:i32)
            n1117 = Multiply(x=w4594, y=10) -> (x*y=w4663:i32)
            n1118 = Add(x=w4640, y=w4642) -> (x+y=w4639:i32)
            n1119 = Add(x=w4631, y=w4632) -> (x+y=w4630:i32)
            n1120 = Bundle(w4629, w4631) -> (w4627:cluster{i32, i32})  [unwired: 1 in]
            n1121 = Bundle(w4640, w4643) -> (w4638:cluster{i32, i32})  [unwired: 1 in]
            n1122 = Add(x=w4665, y=w4663) -> (x+y=w4664:i32)
            n1123 = Bundle(w4665, w4666) -> (w4662:cluster{i32, i32})  [unwired: 1 in]
            n1124 = Bundle(w4629, w4630) -> (w4628:cluster{i32, i32})  [unwired: 1 in]
            n1125 = Bundle(w4639, w4643) -> (w4641:cluster{i32, i32})  [unwired: 1 in]
            n1126 = call <vilib>:"Move Pen.vi"("new position"=w4662, "picture"=w4598) -> ("new picture"=w4661:picture)  [unwired: 3 in]
            n1127 = Bundle(w4664, w4666) -> (w4667:cluster{i32, i32})  [unwired: 1 in]
            n1128 = call <vilib>:"Draw Line.vi"("picture"=w4661, "end point"=w4667, "color(black)"=u32 16448250, "pen"=T1 {"Width"=3, "Style"=enum."Solid"}) -> ("new picture"=w4597:picture)  [unwired: 5 in]
            n1129 = Multiply(x=w4594, y=10) -> (x*y=w4610:i32)
            n1130 = Multiply(x=2, y=w4610) -> (x*y=w4611:i32)
            n1131 = Add(x=w4596, y=0) -> (x+y=w4619:i32)
            n1132 = Multiply(x=w4594, y=10) -> (x*y=w4622:i32)
            n1133 = Add(x=w4595, y=w4622) -> (x+y=w4620:i32)
            n1134 = Add(x=w4596, y=0) -> (x+y=w4607:i32)
            n1135 = Add(x=w4595, y=w4611) -> (x+y=w4609:i32)
            n1136 = Add(x=w4596, y=0) -> (x+y=w4653:i32)
            n1137 = Add(x=w4595, y=0) -> (x+y=w4654:i32)
            n1138 = Multiply(x=w4594, y=10) -> (x*y=w4652:i32)
            n1139 = Add(x=w4620, y=w4622) -> (x+y=w4621:i32)
            n1140 = Add(x=w4607, y=w4610) -> (x+y=w4606:i32)
            n1141 = Add(x=w4654, y=w4652) -> (x+y=w4655:i32)
            n1142 = Bundle(w4619, w4620) -> (w4617:cluster{i32, i32})  [unwired: 1 in]
            n1143 = Bundle(w4607, w4609) -> (w4605:cluster{i32, i32})  [unwired: 1 in]
            n1144 = Bundle(w4653, w4654) -> (w4650:cluster{i32, i32})  [unwired: 1 in]
            n1145 = Bundle(w4619, w4621) -> (w4618:cluster{i32, i32})  [unwired: 1 in]
            n1146 = Bundle(w4606, w4609) -> (w4608:cluster{i32, i32})  [unwired: 1 in]
            n1147 = call <vilib>:"Move Pen.vi"("new position"=w4650, "picture"=w4597) -> ("new picture"=w4649:picture)  [unwired: 3 in]
            n1148 = Bundle(w4653, w4655) -> (w4651:cluster{i32, i32})  [unwired: 1 in]
            n1149 = call <vilib>:"Draw Line.vi"("picture"=w4649, "end point"=w4651, "color(black)"=u32 16448250, "pen"=T1 {"Width"=3, "Style"=enum."Solid"}) -> ("new picture"=w4593:picture)  [unwired: 5 in]
            n1150 = call <vilib>:"Move Pen.vi"("new position"=w4638, "picture"=w4593) -> ("new picture"=w4637:picture)  [unwired: 3 in]
            n1151 = call <vilib>:"Draw Line.vi"("picture"=w4637, "end point"=w4641, "color(black)"=u32 16448250, "pen"=T1 {"Width"=3, "Style"=enum."Solid"}) -> ("new picture"=w4592:picture)  [unwired: 5 in]
            n1152 = call <vilib>:"Move Pen.vi"("new position"=w4617, "picture"=w4592) -> ("new picture"=w4616:picture)  [unwired: 3 in]
            n1153 = call <vilib>:"Draw Line.vi"("picture"=w4616, "end point"=w4618, "color(black)"=u32 16448250, "pen"=T1 {"Width"=3, "Style"=enum."Solid"}) -> ("new picture"=w4591:picture)  [unwired: 5 in]
            n1154 = call <vilib>:"Move Pen.vi"("new position"=w4627, "picture"=w4591) -> ("new picture"=w4626:picture)  [unwired: 3 in]
            n1155 = call <vilib>:"Draw Line.vi"("picture"=w4626, "end point"=w4628, "color(black)"=u32 16448250, "pen"=T1 {"Width"=3, "Style"=enum."Solid"}) -> ("new picture"=w4590:picture)  [unwired: 5 in]
            n1156 = call <vilib>:"Move Pen.vi"("new position"=w4605, "picture"=w4590) -> ("new picture"=w4604:picture)  [unwired: 3 in]
            n1157 = call <vilib>:"Draw Line.vi"("picture"=w4604, "end point"=w4608, "color(black)"=u32 16448250, "pen"=T1 {"Width"=3, "Style"=enum."Solid"}) -> ("new picture"=w4589:picture)  [unwired: 5 in]
          }
          frame 7 {
            n1158 = Add(x=w4673, y=0) -> (x+y=w4706:i32)
            n1159 = Add(x=w4672, y=0) -> (x+y=w4707:i32)
            n1160 = Multiply(x=w4671, y=10) -> (x*y=w4705:i32)
            n1161 = Add(x=w4707, y=w4705) -> (x+y=w4708:i32)
            n1162 = Add(x=w4673, y=0) -> (x+y=w4718:i32)
            n1163 = Add(x=w4672, y=0) -> (x+y=w4719:i32)
            n1164 = Bundle(w4706, w4707) -> (w4703:cluster{i32, i32})  [unwired: 1 in]
            n1165 = Multiply(x=w4671, y=10) -> (x*y=w4716:i32)
            n1166 = Add(x=w4718, y=w4716) -> (x+y=w4717:i32)
            n1167 = Bundle(w4718, w4719) -> (w4715:cluster{i32, i32})  [unwired: 1 in]
            n1168 = Bundle(w4706, w4708) -> (w4704:cluster{i32, i32})  [unwired: 1 in]
            n1169 = call <vilib>:"Move Pen.vi"("new position"=w4715, "picture"=w4675) -> ("new picture"=w4714:picture)  [unwired: 3 in]
            n1170 = Bundle(w4717, w4719) -> (w4720:cluster{i32, i32})  [unwired: 1 in]
            n1171 = call <vilib>:"Draw Line.vi"("picture"=w4714, "end point"=w4720, "color(black)"=u32 16448250, "pen"=T1 {"Width"=3, "Style"=enum."Solid"}) -> ("new picture"=w4674:picture)  [unwired: 5 in]
            n1172 = Multiply(x=w4671, y=10) -> (x*y=w4693:i32)
            n1173 = Add(x=w4673, y=w4693) -> (x+y=w4694:i32)
            n1174 = Add(x=w4672, y=0) -> (x+y=w4696:i32)
            n1175 = Multiply(x=w4671, y=10) -> (x*y=w4685:i32)
            n1176 = Add(x=w4673, y=w4685) -> (x+y=w4682:i32)
            n1177 = Add(x=w4672, y=w4685) -> (x+y=w4684:i32)
            n1178 = Add(x=w4696, y=w4693) -> (x+y=w4695:i32)
            n1179 = Bundle(w4694, w4696) -> (w4691:cluster{i32, i32})  [unwired: 1 in]
            n1180 = Add(x=w4684, y=w4685) -> (x+y=w4683:i32)
            n1181 = Bundle(w4682, w4684) -> (w4680:cluster{i32, i32})  [unwired: 1 in]
            n1182 = Bundle(w4694, w4695) -> (w4692:cluster{i32, i32})  [unwired: 1 in]
            n1183 = call <vilib>:"Move Pen.vi"("new position"=w4680, "picture"=w4674) -> ("new picture"=w4679:picture)  [unwired: 3 in]
            n1184 = Bundle(w4682, w4683) -> (w4681:cluster{i32, i32})  [unwired: 1 in]
            n1185 = call <vilib>:"Draw Line.vi"("picture"=w4679, "end point"=w4681, "color(black)"=u32 16448250, "pen"=T1 {"Width"=3, "Style"=enum."Solid"}) -> ("new picture"=w4670:picture)  [unwired: 5 in]
            n1186 = call <vilib>:"Move Pen.vi"("new position"=w4703, "picture"=w4670) -> ("new picture"=w4702:picture)  [unwired: 3 in]
            n1187 = call <vilib>:"Draw Line.vi"("picture"=w4702, "end point"=w4704, "color(black)"=u32 16448250, "pen"=T1 {"Width"=3, "Style"=enum."Solid"}) -> ("new picture"=w4669:picture)  [unwired: 5 in]
            n1188 = call <vilib>:"Move Pen.vi"("new position"=w4691, "picture"=w4669) -> ("new picture"=w4690:picture)  [unwired: 3 in]
            n1189 = call <vilib>:"Draw Line.vi"("picture"=w4690, "end point"=w4692, "color(black)"=u32 16448250, "pen"=T1 {"Width"=3, "Style"=enum."Solid"}) -> ("new picture"=w4668:picture)  [unwired: 5 in]
          }
          frame 8 {
            n1190 = Add(x=w4729, y=0) -> (x+y=w4797:i32)
            n1191 = Add(x=w4728, y=0) -> (x+y=w4798:i32)
            n1192 = Add(x=w4729, y=0) -> (x+y=w4752:i32)
            n1193 = Multiply(x=w4727, y=10) -> (x*y=w4796:i32)
            n1194 = Multiply(x=w4727, y=10) -> (x*y=w4755:i32)
            n1195 = Add(x=w4728, y=w4755) -> (x+y=w4753:i32)
            n1196 = Add(x=w4729, y=0) -> (x+y=w4809:i32)
            n1197 = Add(x=w4728, y=0) -> (x+y=w4810:i32)
            n1198 = Multiply(x=w4727, y=10) -> (x*y=w4807:i32)
            n1199 = Add(x=w4798, y=w4796) -> (x+y=w4799:i32)
            n1200 = Add(x=w4753, y=w4755) -> (x+y=w4754:i32)
            n1201 = Bundle(w4797, w4798) -> (w4794:cluster{i32, i32})  [unwired: 1 in]
            n1202 = Bundle(w4752, w4753) -> (w4750:cluster{i32, i32})  [unwired: 1 in]
            n1203 = Multiply(x=w4727, y=10) -> (x*y=w4743:i32)
            n1204 = Multiply(x=2, y=w4743) -> (x*y=w4744:i32)
            n1205 = Add(x=w4809, y=w4807) -> (x+y=w4808:i32)
            n1206 = Bundle(w4809, w4810) -> (w4806:cluster{i32, i32})  [unwired: 1 in]
            n1207 = Add(x=w4729, y=0) -> (x+y=w4740:i32)
            n1208 = Add(x=w4728, y=w4744) -> (x+y=w4742:i32)
            n1209 = Add(x=w4740, y=w4743) -> (x+y=w4739:i32)
            n1210 = Bundle(w4797, w4799) -> (w4795:cluster{i32, i32})  [unwired: 1 in]
            n1211 = Bundle(w4752, w4754) -> (w4751:cluster{i32, i32})  [unwired: 1 in]
            n1212 = Bundle(w4740, w4742) -> (w4738:cluster{i32, i32})  [unwired: 1 in]
            n1213 = call <vilib>:"Move Pen.vi"("new position"=w4806, "picture"=w4731) -> ("new picture"=w4805:picture)  [unwired: 3 in]
            n1214 = Bundle(w4808, w4810) -> (w4811:cluster{i32, i32})  [unwired: 1 in]
            n1215 = Bundle(w4739, w4742) -> (w4741:cluster{i32, i32})  [unwired: 1 in]
            n1216 = call <vilib>:"Draw Line.vi"("picture"=w4805, "end point"=w4811, "color(black)"=u32 16448250, "pen"=T1 {"Width"=3, "Style"=enum."Solid"}) -> ("new picture"=w4730:picture)  [unwired: 5 in]
            n1217 = Multiply(x=w4727, y=10) -> (x*y=w4775:i32)
            n1218 = Multiply(x=w4727, y=10) -> (x*y=w4784:i32)
            n1219 = Add(x=w4729, y=0) -> (x+y=w4773:i32)
            n1220 = Multiply(x=w4727, y=10) -> (x*y=w4765:i32)
            n1221 = Add(x=w4728, y=w4775) -> (x+y=w4776:i32)
            n1222 = Add(x=w4729, y=w4784) -> (x+y=w4785:i32)
            n1223 = Add(x=w4728, y=0) -> (x+y=w4787:i32)
            n1224 = Add(x=w4729, y=w4765) -> (x+y=w4762:i32)
            n1225 = Add(x=w4728, y=w4765) -> (x+y=w4764:i32)
            n1226 = Add(x=w4773, y=w4775) -> (x+y=w4772:i32)
            n1227 = Bundle(w4773, w4776) -> (w4771:cluster{i32, i32})  [unwired: 1 in]
            n1228 = Add(x=w4787, y=w4784) -> (x+y=w4786:i32)
            n1229 = Add(x=w4764, y=w4765) -> (x+y=w4763:i32)
            n1230 = Bundle(w4785, w4787) -> (w4782:cluster{i32, i32})  [unwired: 1 in]
            n1231 = Bundle(w4762, w4764) -> (w4760:cluster{i32, i32})  [unwired: 1 in]
            n1232 = call <vilib>:"Move Pen.vi"("new position"=w4771, "picture"=w4730) -> ("new picture"=w4770:picture)  [unwired: 3 in]
            n1233 = Bundle(w4772, w4776) -> (w4774:cluster{i32, i32})  [unwired: 1 in]
            n1234 = Bundle(w4785, w4786) -> (w4783:cluster{i32, i32})  [unwired: 1 in]
            n1235 = Bundle(w4762, w4763) -> (w4761:cluster{i32, i32})  [unwired: 1 in]
            n1236 = call <vilib>:"Draw Line.vi"("picture"=w4770, "end point"=w4774, "color(black)"=u32 16448250, "pen"=T1 {"Width"=3, "Style"=enum."Solid"}) -> ("new picture"=w4726:picture)  [unwired: 5 in]
            n1237 = call <vilib>:"Move Pen.vi"("new position"=w4794, "picture"=w4726) -> ("new picture"=w4793:picture)  [unwired: 3 in]
            n1238 = call <vilib>:"Draw Line.vi"("picture"=w4793, "end point"=w4795, "color(black)"=u32 16448250, "pen"=T1 {"Width"=3, "Style"=enum."Solid"}) -> ("new picture"=w4725:picture)  [unwired: 5 in]
            n1239 = call <vilib>:"Move Pen.vi"("new position"=w4782, "picture"=w4725) -> ("new picture"=w4781:picture)  [unwired: 3 in]
            n1240 = call <vilib>:"Draw Line.vi"("picture"=w4781, "end point"=w4783, "color(black)"=u32 16448250, "pen"=T1 {"Width"=3, "Style"=enum."Solid"}) -> ("new picture"=w4724:picture)  [unwired: 5 in]
            n1241 = call <vilib>:"Move Pen.vi"("new position"=w4750, "picture"=w4724) -> ("new picture"=w4749:picture)  [unwired: 3 in]
            n1242 = call <vilib>:"Draw Line.vi"("picture"=w4749, "end point"=w4751, "color(black)"=u32 16448250, "pen"=T1 {"Width"=3, "Style"=enum."Solid"}) -> ("new picture"=w4723:picture)  [unwired: 5 in]
            n1243 = call <vilib>:"Move Pen.vi"("new position"=w4760, "picture"=w4723) -> ("new picture"=w4759:picture)  [unwired: 3 in]
            n1244 = call <vilib>:"Draw Line.vi"("picture"=w4759, "end point"=w4761, "color(black)"=u32 16448250, "pen"=T1 {"Width"=3, "Style"=enum."Solid"}) -> ("new picture"=w4722:picture)  [unwired: 5 in]
            n1245 = call <vilib>:"Move Pen.vi"("new position"=w4738, "picture"=w4722) -> ("new picture"=w4737:picture)  [unwired: 3 in]
            n1246 = call <vilib>:"Draw Line.vi"("picture"=w4737, "end point"=w4741, "color(black)"=u32 16448250, "pen"=T1 {"Width"=3, "Style"=enum."Solid"}) -> ("new picture"=w4721:picture)  [unwired: 5 in]
          }
          frame 9 {
            n1247 = Add(x=w4818, y=0) -> (x+y=w4862:i32)
            n1248 = Add(x=w4817, y=0) -> (x+y=w4863:i32)
            n1249 = Add(x=w4818, y=0) -> (x+y=w4874:i32)
            n1250 = Add(x=w4817, y=0) -> (x+y=w4875:i32)
            n1251 = Multiply(x=w4816, y=10) -> (x*y=w4861:i32)
            n1252 = Multiply(x=w4816, y=10) -> (x*y=w4872:i32)
            n1253 = Add(x=w4863, y=w4861) -> (x+y=w4864:i32)
            n1254 = Add(x=w4874, y=w4872) -> (x+y=w4873:i32)
            n1255 = Bundle(w4862, w4863) -> (w4859:cluster{i32, i32})  [unwired: 1 in]
            n1256 = Bundle(w4874, w4875) -> (w4871:cluster{i32, i32})  [unwired: 1 in]
            n1257 = Bundle(w4862, w4864) -> (w4860:cluster{i32, i32})  [unwired: 1 in]
            n1258 = call <vilib>:"Move Pen.vi"("new position"=w4871, "picture"=w4820) -> ("new picture"=w4870:picture)  [unwired: 3 in]
            n1259 = Bundle(w4873, w4875) -> (w4876:cluster{i32, i32})  [unwired: 1 in]
            n1260 = Multiply(x=w4816, y=10) -> (x*y=w4830:i32)
            n1261 = Add(x=w4818, y=w4830) -> (x+y=w4827:i32)
            n1262 = Add(x=w4817, y=w4830) -> (x+y=w4829:i32)
            n1263 = Add(x=w4829, y=w4830) -> (x+y=w4828:i32)
            n1264 = Bundle(w4827, w4829) -> (w4825:cluster{i32, i32})  [unwired: 1 in]
            n1265 = call <vilib>:"Draw Line.vi"("picture"=w4870, "end point"=w4876, "color(black)"=u32 16448250, "pen"=T1 {"Width"=3, "Style"=enum."Solid"}) -> ("new picture"=w4819:picture)  [unwired: 5 in]
            n1266 = Bundle(w4827, w4828) -> (w4826:cluster{i32, i32})  [unwired: 1 in]
            n1267 = Multiply(x=w4816, y=10) -> (x*y=w4849:i32)
            n1268 = Add(x=w4818, y=w4849) -> (x+y=w4850:i32)
            n1269 = Add(x=w4817, y=0) -> (x+y=w4852:i32)
            n1270 = Multiply(x=w4816, y=10) -> (x*y=w4840:i32)
            n1271 = Add(x=w4818, y=0) -> (x+y=w4838:i32)
            n1272 = Add(x=w4817, y=w4840) -> (x+y=w4841:i32)
            n1273 = Add(x=w4852, y=w4849) -> (x+y=w4851:i32)
            n1274 = Add(x=w4838, y=w4840) -> (x+y=w4837:i32)
            n1275 = Bundle(w4850, w4852) -> (w4847:cluster{i32, i32})  [unwired: 1 in]
            n1276 = Bundle(w4838, w4841) -> (w4836:cluster{i32, i32})  [unwired: 1 in]
            n1277 = Bundle(w4850, w4851) -> (w4848:cluster{i32, i32})  [unwired: 1 in]
            n1278 = call <vilib>:"Move Pen.vi"("new position"=w4836, "picture"=w4819) -> ("new picture"=w4835:picture)  [unwired: 3 in]
            n1279 = Bundle(w4837, w4841) -> (w4839:cluster{i32, i32})  [unwired: 1 in]
            n1280 = call <vilib>:"Draw Line.vi"("picture"=w4835, "end point"=w4839, "color(black)"=u32 16448250, "pen"=T1 {"Width"=3, "Style"=enum."Solid"}) -> ("new picture"=w4815:picture)  [unwired: 5 in]
            n1281 = call <vilib>:"Move Pen.vi"("new position"=w4859, "picture"=w4815) -> ("new picture"=w4858:picture)  [unwired: 3 in]
            n1282 = call <vilib>:"Draw Line.vi"("picture"=w4858, "end point"=w4860, "color(black)"=u32 16448250, "pen"=T1 {"Width"=3, "Style"=enum."Solid"}) -> ("new picture"=w4814:picture)  [unwired: 5 in]
            n1283 = call <vilib>:"Move Pen.vi"("new position"=w4847, "picture"=w4814) -> ("new picture"=w4846:picture)  [unwired: 3 in]
            n1284 = call <vilib>:"Draw Line.vi"("picture"=w4846, "end point"=w4848, "color(black)"=u32 16448250, "pen"=T1 {"Width"=3, "Style"=enum."Solid"}) -> ("new picture"=w4813:picture)  [unwired: 5 in]
            n1285 = call <vilib>:"Move Pen.vi"("new position"=w4825, "picture"=w4813) -> ("new picture"=w4824:picture)  [unwired: 3 in]
            n1286 = call <vilib>:"Draw Line.vi"("picture"=w4824, "end point"=w4826, "color(black)"=u32 16448250, "pen"=T1 {"Width"=3, "Style"=enum."Solid"}) -> ("new picture"=w4812:picture)  [unwired: 5 in]
          }
        }
        n1287 = case shown="9" w149 {
          tunnel: 420 -> [w3593 w3667 w3697 w3765 w3830 w3882 w3950 w4027 w4083 w4172]
          tunnel: 10 -> [w3592 w3666 w3696 w3764 w3829 w3881 w3949 w4026 w4082 w4171]
          tunnel: 3 -> [w3591 w3665 w3695 w3763 w3828 w3880 w3948 w4025 w4081 w4170]
          tunnel: w164 -> [w3594 w3669 w3699 w3766 w3831 w3884 w3952 w4029 w4085 w4174]
          tunnel: [w3585 w3664 w3691 w3758 w3824 w3876 w3943 w4022 w4075 w4166] -> w172
          frame 0, Default {
            n1288 = Add(x=w3593, y=0) -> (x+y=w3649:i32)
            n1289 = Add(x=w3592, y=0) -> (x+y=w3650:i32)
            n1290 = Multiply(x=w3591, y=10) -> (x*y=w3648:i32)
            n1291 = Add(x=w3593, y=0) -> (x+y=w3615:i32)
            n1292 = Multiply(x=w3591, y=10) -> (x*y=w3618:i32)
            n1293 = Add(x=w3592, y=w3618) -> (x+y=w3616:i32)
            n1294 = Add(x=w3650, y=w3648) -> (x+y=w3651:i32)
            n1295 = Add(x=w3616, y=w3618) -> (x+y=w3617:i32)
            n1296 = Bundle(w3649, w3650) -> (w3646:cluster{i32, i32})  [unwired: 1 in]
            n1297 = Bundle(w3615, w3616) -> (w3613:cluster{i32, i32})  [unwired: 1 in]
            n1298 = Bundle(w3649, w3651) -> (w3647:cluster{i32, i32})  [unwired: 1 in]
            n1299 = Bundle(w3615, w3617) -> (w3614:cluster{i32, i32})  [unwired: 1 in]
            n1300 = Multiply(x=w3591, y=10) -> (x*y=w3606:i32)
            n1301 = Multiply(x=2, y=w3606) -> (x*y=w3607:i32)
            n1302 = Add(x=w3593, y=0) -> (x+y=w3661:i32)
            n1303 = Add(x=w3592, y=0) -> (x+y=w3662:i32)
            n1304 = Add(x=w3593, y=0) -> (x+y=w3603:i32)
            n1305 = Add(x=w3592, y=w3607) -> (x+y=w3605:i32)
            n1306 = Multiply(x=w3591, y=10) -> (x*y=w3659:i32)
            n1307 = Add(x=w3603, y=w3606) -> (x+y=w3602:i32)
            n1308 = Add(x=w3661, y=w3659) -> (x+y=w3660:i32)
            n1309 = Bundle(w3661, w3662) -> (w3658:cluster{i32, i32})  [unwired: 1 in]
            n1310 = Bundle(w3603, w3605) -> (w3601:cluster{i32, i32})  [unwired: 1 in]
            n1311 = call <vilib>:"Move Pen.vi"("new position"=w3658, "picture"=w3594) -> ("new picture"=w3657:picture)  [unwired: 3 in]
            n1312 = Bundle(w3660, w3662) -> (w3663:cluster{i32, i32})  [unwired: 1 in]
            n1313 = Bundle(w3602, w3605) -> (w3604:cluster{i32, i32})  [unwired: 1 in]
            n1314 = Multiply(x=w3591, y=10) -> (x*y=w3636:i32)
            n1315 = Add(x=w3593, y=w3636) -> (x+y=w3637:i32)
            n1316 = Add(x=w3592, y=0) -> (x+y=w3639:i32)
            n1317 = Multiply(x=w3591, y=10) -> (x*y=w3628:i32)
            n1318 = Add(x=w3593, y=w3628) -> (x+y=w3625:i32)
            n1319 = Add(x=w3592, y=w3628) -> (x+y=w3627:i32)
            n1320 = Add(x=w3639, y=w3636) -> (x+y=w3638:i32)
            n1321 = Bundle(w3637, w3639) -> (w3634:cluster{i32, i32})  [unwired: 1 in]
            n1322 = call <vilib>:"Draw Line.vi"("picture"=w3657, "end point"=w3663, "color(black)"=u32 16448250, "pen"=T1 {"Width"=3, "Style"=enum."Solid"}) -> ("new picture"=w3590:picture)  [unwired: 5 in]
            n1323 = call <vilib>:"Move Pen.vi"("new position"=w3646, "picture"=w3590) -> ("new picture"=w3645:picture)  [unwired: 3 in]
            n1324 = call <vilib>:"Draw Line.vi"("picture"=w3645, "end point"=w3647, "color(black)"=u32 16448250, "pen"=T1 {"Width"=3, "Style"=enum."Solid"}) -> ("new picture"=w3589:picture)  [unwired: 5 in]
            n1325 = Add(x=w3627, y=w3628) -> (x+y=w3626:i32)
            n1326 = Bundle(w3625, w3627) -> (w3623:cluster{i32, i32})  [unwired: 1 in]
            n1327 = call <vilib>:"Move Pen.vi"("new position"=w3634, "picture"=w3589) -> ("new picture"=w3633:picture)  [unwired: 3 in]
            n1328 = Bundle(w3637, w3638) -> (w3635:cluster{i32, i32})  [unwired: 1 in]
            n1329 = Bundle(w3625, w3626) -> (w3624:cluster{i32, i32})  [unwired: 1 in]
            n1330 = call <vilib>:"Draw Line.vi"("picture"=w3633, "end point"=w3635, "color(black)"=u32 16448250, "pen"=T1 {"Width"=3, "Style"=enum."Solid"}) -> ("new picture"=w3588:picture)  [unwired: 5 in]
            n1331 = call <vilib>:"Move Pen.vi"("new position"=w3613, "picture"=w3588) -> ("new picture"=w3612:picture)  [unwired: 3 in]
            n1332 = call <vilib>:"Draw Line.vi"("picture"=w3612, "end point"=w3614, "color(black)"=u32 16448250, "pen"=T1 {"Width"=3, "Style"=enum."Solid"}) -> ("new picture"=w3587:picture)  [unwired: 5 in]
            n1333 = call <vilib>:"Move Pen.vi"("new position"=w3623, "picture"=w3587) -> ("new picture"=w3622:picture)  [unwired: 3 in]
            n1334 = call <vilib>:"Draw Line.vi"("picture"=w3622, "end point"=w3624, "color(black)"=u32 16448250, "pen"=T1 {"Width"=3, "Style"=enum."Solid"}) -> ("new picture"=w3586:picture)  [unwired: 5 in]
            n1335 = call <vilib>:"Move Pen.vi"("new position"=w3601, "picture"=w3586) -> ("new picture"=w3600:picture)  [unwired: 3 in]
            n1336 = call <vilib>:"Draw Line.vi"("picture"=w3600, "end point"=w3604, "color(black)"=u32 16448250, "pen"=T1 {"Width"=3, "Style"=enum."Solid"}) -> ("new picture"=w3585:picture)  [unwired: 5 in]
          }
          frame 1 {
            n1337 = Multiply(x=w3665, y=10) -> (x*y=w3687:i32)
            n1338 = Add(x=w3667, y=w3687) -> (x+y=w3688:i32)
            n1339 = Add(x=w3666, y=0) -> (x+y=w3690:i32)
            n1340 = Add(x=w3690, y=w3687) -> (x+y=w3689:i32)
            n1341 = Bundle(w3688, w3690) -> (w3685:cluster{i32, i32})  [unwired: 1 in]
            n1342 = call <vilib>:"Move Pen.vi"("new position"=w3685, "picture"=w3669) -> ("new picture"=w3684:picture)  [unwired: 3 in]
            n1343 = Bundle(w3688, w3689) -> (w3686:cluster{i32, i32})  [unwired: 1 in]
            n1344 = call <vilib>:"Draw Line.vi"("picture"=w3684, "end point"=w3686, "color(black)"=u32 16448250, "pen"=T1 {"Width"=3, "Style"=enum."Solid"}) -> ("new picture"=w3668:picture)  [unwired: 5 in]
            n1345 = Multiply(x=w3665, y=10) -> (x*y=w3679:i32)
            n1346 = Add(x=w3667, y=w3679) -> (x+y=w3676:i32)
            n1347 = Add(x=w3666, y=w3679) -> (x+y=w3678:i32)
            n1348 = Add(x=w3678, y=w3679) -> (x+y=w3677:i32)
            n1349 = Bundle(w3676, w3678) -> (w3674:cluster{i32, i32})  [unwired: 1 in]
            n1350 = call <vilib>:"Move Pen.vi"("new position"=w3674, "picture"=w3668) -> ("new picture"=w3673:picture)  [unwired: 3 in]
            n1351 = Bundle(w3676, w3677) -> (w3675:cluster{i32, i32})  [unwired: 1 in]
            n1352 = call <vilib>:"Draw Line.vi"("picture"=w3673, "end point"=w3675, "color(black)"=u32 16448250, "pen"=T1 {"Width"=3, "Style"=enum."Solid"}) -> ("new picture"=w3664:picture)  [unwired: 5 in]
          }
          frame 2 {
            n1353 = Multiply(x=w3695, y=10) -> (x*y=w3733:i32)
            n1354 = Add(x=w3697, y=0) -> (x+y=w3731:i32)
            n1355 = Add(x=w3696, y=w3733) -> (x+y=w3734:i32)
            n1356 = Add(x=w3697, y=0) -> (x+y=w3755:i32)
            n1357 = Add(x=w3696, y=0) -> (x+y=w3756:i32)
            n1358 = Multiply(x=w3695, y=10) -> (x*y=w3753:i32)
            n1359 = Add(x=w3731, y=w3733) -> (x+y=w3730:i32)
            n1360 = Add(x=w3755, y=w3753) -> (x+y=w3754:i32)
            n1361 = Bundle(w3731, w3734) -> (w3729:cluster{i32, i32})  [unwired: 1 in]
            n1362 = Bundle(w3755, w3756) -> (w3752:cluster{i32, i32})  [unwired: 1 in]
            n1363 = Bundle(w3730, w3734) -> (w3732:cluster{i32, i32})  [unwired: 1 in]
            n1364 = call <vilib>:"Move Pen.vi"("new position"=w3752, "picture"=w3699) -> ("new picture"=w3751:picture)  [unwired: 3 in]
            n1365 = Bundle(w3754, w3756) -> (w3757:cluster{i32, i32})  [unwired: 1 in]
            n1366 = Multiply(x=w3695, y=10) -> (x*y=w3711:i32)
            n1367 = Multiply(x=2, y=w3711) -> (x*y=w3712:i32)
            n1368 = Add(x=w3697, y=0) -> (x+y=w3708:i32)
            n1369 = Add(x=w3696, y=w3712) -> (x+y=w3710:i32)
            n1370 = Add(x=w3708, y=w3711) -> (x+y=w3707:i32)
            n1371 = Bundle(w3708, w3710) -> (w3706:cluster{i32, i32})  [unwired: 1 in]
            n1372 = call <vilib>:"Draw Line.vi"("picture"=w3751, "end point"=w3757, "color(black)"=u32 16448250, "pen"=T1 {"Width"=3, "Style"=enum."Solid"}) -> ("new picture"=w3698:picture)  [unwired: 5 in]
            n1373 = Bundle(w3707, w3710) -> (w3709:cluster{i32, i32})  [unwired: 1 in]
            n1374 = Multiply(x=w3695, y=10) -> (x*y=w3742:i32)
            n1375 = Add(x=w3697, y=0) -> (x+y=w3720:i32)
            n1376 = Add(x=w3697, y=w3742) -> (x+y=w3743:i32)
            n1377 = Add(x=w3696, y=0) -> (x+y=w3745:i32)
            n1378 = Multiply(x=w3695, y=10) -> (x*y=w3723:i32)
            n1379 = Add(x=w3696, y=w3723) -> (x+y=w3721:i32)
            n1380 = Add(x=w3721, y=w3723) -> (x+y=w3722:i32)
            n1381 = Add(x=w3745, y=w3742) -> (x+y=w3744:i32)
            n1382 = Bundle(w3720, w3721) -> (w3718:cluster{i32, i32})  [unwired: 1 in]
            n1383 = Bundle(w3743, w3745) -> (w3740:cluster{i32, i32})  [unwired: 1 in]
            n1384 = call <vilib>:"Move Pen.vi"("new position"=w3740, "picture"=w3698) -> ("new picture"=w3739:picture)  [unwired: 3 in]
            n1385 = Bundle(w3720, w3722) -> (w3719:cluster{i32, i32})  [unwired: 1 in]
            n1386 = Bundle(w3743, w3744) -> (w3741:cluster{i32, i32})  [unwired: 1 in]
            n1387 = call <vilib>:"Draw Line.vi"("picture"=w3739, "end point"=w3741, "color(black)"=u32 16448250, "pen"=T1 {"Width"=3, "Style"=enum."Solid"}) -> ("new picture"=w3694:picture)  [unwired: 5 in]
            n1388 = call <vilib>:"Move Pen.vi"("new position"=w3729, "picture"=w3694) -> ("new picture"=w3728:picture)  [unwired: 3 in]
            n1389 = call <vilib>:"Draw Line.vi"("picture"=w3728, "end point"=w3732, "color(black)"=u32 16448250, "pen"=T1 {"Width"=3, "Style"=enum."Solid"}) -> ("new picture"=w3693:picture)  [unwired: 5 in]
            n1390 = call <vilib>:"Move Pen.vi"("new position"=w3718, "picture"=w3693) -> ("new picture"=w3717:picture)  [unwired: 3 in]
            n1391 = call <vilib>:"Draw Line.vi"("picture"=w3717, "end point"=w3719, "color(black)"=u32 16448250, "pen"=T1 {"Width"=3, "Style"=enum."Solid"}) -> ("new picture"=w3692:picture)  [unwired: 5 in]
            n1392 = call <vilib>:"Move Pen.vi"("new position"=w3706, "picture"=w3692) -> ("new picture"=w3705:picture)  [unwired: 3 in]
            n1393 = call <vilib>:"Draw Line.vi"("picture"=w3705, "end point"=w3709, "color(black)"=u32 16448250, "pen"=T1 {"Width"=3, "Style"=enum."Solid"}) -> ("new picture"=w3691:picture)  [unwired: 5 in]
          }
          frame 3 {
            n1394 = Multiply(x=w3763, y=10) -> (x*y=w3799:i32)
            n1395 = Add(x=w3765, y=0) -> (x+y=w3797:i32)
            n1396 = Add(x=w3764, y=w3799) -> (x+y=w3800:i32)
            n1397 = Add(x=w3765, y=0) -> (x+y=w3821:i32)
            n1398 = Add(x=w3764, y=0) -> (x+y=w3822:i32)
            n1399 = Multiply(x=w3763, y=10) -> (x*y=w3819:i32)
            n1400 = Add(x=w3797, y=w3799) -> (x+y=w3796:i32)
            n1401 = Add(x=w3821, y=w3819) -> (x+y=w3820:i32)
            n1402 = Bundle(w3797, w3800) -> (w3795:cluster{i32, i32})  [unwired: 1 in]
            n1403 = Bundle(w3821, w3822) -> (w3818:cluster{i32, i32})  [unwired: 1 in]
            n1404 = call <vilib>:"Move Pen.vi"("new position"=w3818, "picture"=w3766) -> ("new picture"=w3817:picture)  [unwired: 3 in]
            n1405 = Bundle(w3796, w3800) -> (w3798:cluster{i32, i32})  [unwired: 1 in]
            n1406 = Bundle(w3820, w3822) -> (w3823:cluster{i32, i32})  [unwired: 1 in]
            n1407 = Multiply(x=w3763, y=10) -> (x*y=w3778:i32)
            n1408 = Multiply(x=2, y=w3778) -> (x*y=w3779:i32)
            n1409 = Add(x=w3765, y=0) -> (x+y=w3775:i32)
            n1410 = Add(x=w3764, y=w3779) -> (x+y=w3777:i32)
            n1411 = Add(x=w3775, y=w3778) -> (x+y=w3774:i32)
            n1412 = call <vilib>:"Draw Line.vi"("picture"=w3817, "end point"=w3823, "color(black)"=u32 16448250, "pen"=T1 {"Width"=3, "Style"=enum."Solid"}) -> ("new picture"=w3762:picture)  [unwired: 5 in]
            n1413 = Bundle(w3775, w3777) -> (w3773:cluster{i32, i32})  [unwired: 1 in]
            n1414 = Bundle(w3774, w3777) -> (w3776:cluster{i32, i32})  [unwired: 1 in]
            n1415 = Multiply(x=w3763, y=10) -> (x*y=w3789:i32)
            n1416 = Add(x=w3765, y=w3789) -> (x+y=w3786:i32)
            n1417 = Add(x=w3764, y=w3789) -> (x+y=w3788:i32)
            n1418 = Multiply(x=w3763, y=10) -> (x*y=w3808:i32)
            n1419 = Add(x=w3765, y=w3808) -> (x+y=w3809:i32)
            n1420 = Add(x=w3764, y=0) -> (x+y=w3811:i32)
            n1421 = Add(x=w3788, y=w3789) -> (x+y=w3787:i32)
            n1422 = Bundle(w3786, w3788) -> (w3784:cluster{i32, i32})  [unwired: 1 in]
            n1423 = Add(x=w3811, y=w3808) -> (x+y=w3810:i32)
            n1424 = Bundle(w3809, w3811) -> (w3806:cluster{i32, i32})  [unwired: 1 in]
            n1425 = Bundle(w3786, w3787) -> (w3785:cluster{i32, i32})  [unwired: 1 in]
            n1426 = call <vilib>:"Move Pen.vi"("new position"=w3806, "picture"=w3762) -> ("new picture"=w3805:picture)  [unwired: 3 in]
            n1427 = Bundle(w3809, w3810) -> (w3807:cluster{i32, i32})  [unwired: 1 in]
            n1428 = call <vilib>:"Draw Line.vi"("picture"=w3805, "end point"=w3807, "color(black)"=u32 16448250, "pen"=T1 {"Width"=3, "Style"=enum."Solid"}) -> ("new picture"=w3761:picture)  [unwired: 5 in]
            n1429 = call <vilib>:"Move Pen.vi"("new position"=w3795, "picture"=w3761) -> ("new picture"=w3794:picture)  [unwired: 3 in]
            n1430 = call <vilib>:"Draw Line.vi"("picture"=w3794, "end point"=w3798, "color(black)"=u32 16448250, "pen"=T1 {"Width"=3, "Style"=enum."Solid"}) -> ("new picture"=w3760:picture)  [unwired: 5 in]
            n1431 = call <vilib>:"Move Pen.vi"("new position"=w3784, "picture"=w3760) -> ("new picture"=w3783:picture)  [unwired: 3 in]
            n1432 = call <vilib>:"Draw Line.vi"("picture"=w3783, "end point"=w3785, "color(black)"=u32 16448250, "pen"=T1 {"Width"=3, "Style"=enum."Solid"}) -> ("new picture"=w3759:picture)  [unwired: 5 in]
            n1433 = call <vilib>:"Move Pen.vi"("new position"=w3773, "picture"=w3759) -> ("new picture"=w3772:picture)  [unwired: 3 in]
            n1434 = call <vilib>:"Draw Line.vi"("picture"=w3772, "end point"=w3776, "color(black)"=u32 16448250, "pen"=T1 {"Width"=3, "Style"=enum."Solid"}) -> ("new picture"=w3758:picture)  [unwired: 5 in]
          }
          frame 4 {
            n1435 = Add(x=w3830, y=0) -> (x+y=w3873:i32)
            n1436 = Add(x=w3829, y=0) -> (x+y=w3874:i32)
            n1437 = Multiply(x=w3828, y=10) -> (x*y=w3872:i32)
            n1438 = Add(x=w3874, y=w3872) -> (x+y=w3875:i32)
            n1439 = Bundle(w3873, w3874) -> (w3870:cluster{i32, i32})  [unwired: 1 in]
            n1440 = call <vilib>:"Move Pen.vi"("new position"=w3870, "picture"=w3831) -> ("new picture"=w3869:picture)  [unwired: 3 in]
            n1441 = Bundle(w3873, w3875) -> (w3871:cluster{i32, i32})  [unwired: 1 in]
            n1442 = Multiply(x=w3828, y=10) -> (x*y=w3851:i32)
            n1443 = Add(x=w3830, y=0) -> (x+y=w3849:i32)
            n1444 = Add(x=w3829, y=w3851) -> (x+y=w3852:i32)
            n1445 = Add(x=w3849, y=w3851) -> (x+y=w3848:i32)
            n1446 = Bundle(w3849, w3852) -> (w3847:cluster{i32, i32})  [unwired: 1 in]
            n1447 = call <vilib>:"Draw Line.vi"("picture"=w3869, "end point"=w3871, "color(black)"=u32 16448250, "pen"=T1 {"Width"=3, "Style"=enum."Solid"}) -> ("new picture"=w3825:picture)  [unwired: 5 in]
            n1448 = Multiply(x=w3828, y=10) -> (x*y=w3841:i32)
            n1449 = Add(x=w3830, y=w3841) -> (x+y=w3838:i32)
            n1450 = Add(x=w3829, y=w3841) -> (x+y=w3840:i32)
            n1451 = Bundle(w3848, w3852) -> (w3850:cluster{i32, i32})  [unwired: 1 in]
            n1452 = Add(x=w3840, y=w3841) -> (x+y=w3839:i32)
            n1453 = Bundle(w3838, w3840) -> (w3836:cluster{i32, i32})  [unwired: 1 in]
            n1454 = Multiply(x=w3828, y=10) -> (x*y=w3860:i32)
            n1455 = Add(x=w3830, y=w3860) -> (x+y=w3861:i32)
            n1456 = Add(x=w3829, y=0) -> (x+y=w3863:i32)
            n1457 = Add(x=w3863, y=w3860) -> (x+y=w3862:i32)
            n1458 = Bundle(w3838, w3839) -> (w3837:cluster{i32, i32})  [unwired: 1 in]
            n1459 = Bundle(w3861, w3863) -> (w3858:cluster{i32, i32})  [unwired: 1 in]
            n1460 = call <vilib>:"Move Pen.vi"("new position"=w3858, "picture"=w3825) -> ("new picture"=w3857:picture)  [unwired: 3 in]
            n1461 = Bundle(w3861, w3862) -> (w3859:cluster{i32, i32})  [unwired: 1 in]
            n1462 = call <vilib>:"Draw Line.vi"("picture"=w3857, "end point"=w3859, "color(black)"=u32 16448250, "pen"=T1 {"Width"=3, "Style"=enum."Solid"}) -> ("new picture"=w3827:picture)  [unwired: 5 in]
            n1463 = call <vilib>:"Move Pen.vi"("new position"=w3847, "picture"=w3827) -> ("new picture"=w3846:picture)  [unwired: 3 in]
            n1464 = call <vilib>:"Draw Line.vi"("picture"=w3846, "end point"=w3850, "color(black)"=u32 16448250, "pen"=T1 {"Width"=3, "Style"=enum."Solid"}) -> ("new picture"=w3826:picture)  [unwired: 5 in]
            n1465 = call <vilib>:"Move Pen.vi"("new position"=w3836, "picture"=w3826) -> ("new picture"=w3835:picture)  [unwired: 3 in]
            n1466 = call <vilib>:"Draw Line.vi"("picture"=w3835, "end point"=w3837, "color(black)"=u32 16448250, "pen"=T1 {"Width"=3, "Style"=enum."Solid"}) -> ("new picture"=w3824:picture)  [unwired: 5 in]
          }
          frame 5 {
            n1467 = Multiply(x=w3880, y=10) -> (x*y=w3917:i32)
            n1468 = Add(x=w3882, y=0) -> (x+y=w3915:i32)
            n1469 = Add(x=w3881, y=w3917) -> (x+y=w3918:i32)
            n1470 = Add(x=w3882, y=0) -> (x+y=w3940:i32)
            n1471 = Add(x=w3881, y=0) -> (x+y=w3941:i32)
            n1472 = Add(x=w3915, y=w3917) -> (x+y=w3914:i32)
            n1473 = Multiply(x=w3880, y=10) -> (x*y=w3938:i32)
            n1474 = Bundle(w3915, w3918) -> (w3913:cluster{i32, i32})  [unwired: 1 in]
            n1475 = Add(x=w3940, y=w3938) -> (x+y=w3939:i32)
            n1476 = Bundle(w3940, w3941) -> (w3937:cluster{i32, i32})  [unwired: 1 in]
            n1477 = Bundle(w3914, w3918) -> (w3916:cluster{i32, i32})  [unwired: 1 in]
            n1478 = call <vilib>:"Move Pen.vi"("new position"=w3937, "picture"=w3884) -> ("new picture"=w3936:picture)  [unwired: 3 in]
            n1479 = Bundle(w3939, w3941) -> (w3942:cluster{i32, i32})  [unwired: 1 in]
            n1480 = Multiply(x=w3880, y=10) -> (x*y=w3896:i32)
            n1481 = Multiply(x=2, y=w3896) -> (x*y=w3897:i32)
            n1482 = Add(x=w3882, y=0) -> (x+y=w3893:i32)
            n1483 = Add(x=w3881, y=w3897) -> (x+y=w3895:i32)
            n1484 = Add(x=w3893, y=w3896) -> (x+y=w3892:i32)
            n1485 = Bundle(w3893, w3895) -> (w3891:cluster{i32, i32})  [unwired: 1 in]
            n1486 = call <vilib>:"Draw Line.vi"("picture"=w3936, "end point"=w3942, "color(black)"=u32 16448250, "pen"=T1 {"Width"=3, "Style"=enum."Solid"}) -> ("new picture"=w3883:picture)  [unwired: 5 in]
            n1487 = Bundle(w3892, w3895) -> (w3894:cluster{i32, i32})  [unwired: 1 in]
            n1488 = Multiply(x=w3880, y=10) -> (x*y=w3907:i32)
            n1489 = Add(x=w3882, y=0) -> (x+y=w3928:i32)
            n1490 = Add(x=w3881, y=0) -> (x+y=w3929:i32)
            n1491 = Add(x=w3882, y=w3907) -> (x+y=w3904:i32)
            n1492 = Add(x=w3881, y=w3907) -> (x+y=w3906:i32)
            n1493 = Multiply(x=w3880, y=10) -> (x*y=w3927:i32)
            n1494 = Add(x=w3929, y=w3927) -> (x+y=w3930:i32)
            n1495 = Add(x=w3906, y=w3907) -> (x+y=w3905:i32)
            n1496 = Bundle(w3928, w3929) -> (w3925:cluster{i32, i32})  [unwired: 1 in]
            n1497 = Bundle(w3904, w3906) -> (w3902:cluster{i32, i32})  [unwired: 1 in]
            n1498 = call <vilib>:"Move Pen.vi"("new position"=w3925, "picture"=w3883) -> ("new picture"=w3924:picture)  [unwired: 3 in]
            n1499 = Bundle(w3928, w3930) -> (w3926:cluster{i32, i32})  [unwired: 1 in]
            n1500 = Bundle(w3904, w3905) -> (w3903:cluster{i32, i32})  [unwired: 1 in]
            n1501 = call <vilib>:"Draw Line.vi"("picture"=w3924, "end point"=w3926, "color(black)"=u32 16448250, "pen"=T1 {"Width"=3, "Style"=enum."Solid"}) -> ("new picture"=w3879:picture)  [unwired: 5 in]
            n1502 = call <vilib>:"Move Pen.vi"("new position"=w3913, "picture"=w3879) -> ("new picture"=w3912:picture)  [unwired: 3 in]
            n1503 = call <vilib>:"Draw Line.vi"("picture"=w3912, "end point"=w3916, "color(black)"=u32 16448250, "pen"=T1 {"Width"=3, "Style"=enum."Solid"}) -> ("new picture"=w3878:picture)  [unwired: 5 in]
            n1504 = call <vilib>:"Move Pen.vi"("new position"=w3902, "picture"=w3878) -> ("new picture"=w3901:picture)  [unwired: 3 in]
            n1505 = call <vilib>:"Draw Line.vi"("picture"=w3901, "end point"=w3903, "color(black)"=u32 16448250, "pen"=T1 {"Width"=3, "Style"=enum."Solid"}) -> ("new picture"=w3877:picture)  [unwired: 5 in]
            n1506 = call <vilib>:"Move Pen.vi"("new position"=w3891, "picture"=w3877) -> ("new picture"=w3890:picture)  [unwired: 3 in]
            n1507 = call <vilib>:"Draw Line.vi"("picture"=w3890, "end point"=w3894, "color(black)"=u32 16448250, "pen"=T1 {"Width"=3, "Style"=enum."Solid"}) -> ("new picture"=w3876:picture)  [unwired: 5 in]
          }
          frame 6 {
            n1508 = Multiply(x=w3948, y=10) -> (x*y=w3986:i32)
            n1509 = Multiply(x=w3948, y=10) -> (x*y=w3996:i32)
            n1510 = Add(x=w3950, y=w3986) -> (x+y=w3983:i32)
            n1511 = Add(x=w3949, y=w3986) -> (x+y=w3985:i32)
            n1512 = Add(x=w3950, y=0) -> (x+y=w3994:i32)
            n1513 = Add(x=w3949, y=w3996) -> (x+y=w3997:i32)
            n1514 = Add(x=w3950, y=0) -> (x+y=w4019:i32)
            n1515 = Add(x=w3949, y=0) -> (x+y=w4020:i32)
            n1516 = Multiply(x=w3948, y=10) -> (x*y=w4017:i32)
            n1517 = Add(x=w3994, y=w3996) -> (x+y=w3993:i32)
            n1518 = Add(x=w3985, y=w3986) -> (x+y=w3984:i32)
            n1519 = Bundle(w3983, w3985) -> (w3981:cluster{i32, i32})  [unwired: 1 in]
            n1520 = Bundle(w3994, w3997) -> (w3992:cluster{i32, i32})  [unwired: 1 in]
            n1521 = Add(x=w4019, y=w4017) -> (x+y=w4018:i32)
            n1522 = Bundle(w4019, w4020) -> (w4016:cluster{i32, i32})  [unwired: 1 in]
            n1523 = Bundle(w3983, w3984) -> (w3982:cluster{i32, i32})  [unwired: 1 in]
            n1524 = Bundle(w3993, w3997) -> (w3995:cluster{i32, i32})  [unwired: 1 in]
            n1525 = call <vilib>:"Move Pen.vi"("new position"=w4016, "picture"=w3952) -> ("new picture"=w4015:picture)  [unwired: 3 in]
            n1526 = Bundle(w4018, w4020) -> (w4021:cluster{i32, i32})  [unwired: 1 in]
            n1527 = call <vilib>:"Draw Line.vi"("picture"=w4015, "end point"=w4021, "color(black)"=u32 16448250, "pen"=T1 {"Width"=3, "Style"=enum."Solid"}) -> ("new picture"=w3951:picture)  [unwired: 5 in]
            n1528 = Multiply(x=w3948, y=10) -> (x*y=w3964:i32)
            n1529 = Multiply(x=2, y=w3964) -> (x*y=w3965:i32)
            n1530 = Add(x=w3950, y=0) -> (x+y=w3973:i32)
            n1531 = Multiply(x=w3948, y=10) -> (x*y=w3976:i32)
            n1532 = Add(x=w3949, y=w3976) -> (x+y=w3974:i32)
            n1533 = Add(x=w3950, y=0) -> (x+y=w3961:i32)
            n1534 = Add(x=w3949, y=w3965) -> (x+y=w3963:i32)
            n1535 = Add(x=w3950, y=0) -> (x+y=w4007:i32)
            n1536 = Add(x=w3949, y=0) -> (x+y=w4008:i32)
            n1537 = Multiply(x=w3948, y=10) -> (x*y=w4006:i32)
            n1538 = Add(x=w3974, y=w3976) -> (x+y=w3975:i32)
            n1539 = Add(x=w3961, y=w3964) -> (x+y=w3960:i32)
            n1540 = Add(x=w4008, y=w4006) -> (x+y=w4009:i32)
            n1541 = Bundle(w3973, w3974) -> (w3971:cluster{i32, i32})  [unwired: 1 in]
            n1542 = Bundle(w3961, w3963) -> (w3959:cluster{i32, i32})  [unwired: 1 in]
            n1543 = Bundle(w4007, w4008) -> (w4004:cluster{i32, i32})  [unwired: 1 in]
            n1544 = Bundle(w3973, w3975) -> (w3972:cluster{i32, i32})  [unwired: 1 in]
            n1545 = Bundle(w3960, w3963) -> (w3962:cluster{i32, i32})  [unwired: 1 in]
            n1546 = call <vilib>:"Move Pen.vi"("new position"=w4004, "picture"=w3951) -> ("new picture"=w4003:picture)  [unwired: 3 in]
            n1547 = Bundle(w4007, w4009) -> (w4005:cluster{i32, i32})  [unwired: 1 in]
            n1548 = call <vilib>:"Draw Line.vi"("picture"=w4003, "end point"=w4005, "color(black)"=u32 16448250, "pen"=T1 {"Width"=3, "Style"=enum."Solid"}) -> ("new picture"=w3947:picture)  [unwired: 5 in]
            n1549 = call <vilib>:"Move Pen.vi"("new position"=w3992, "picture"=w3947) -> ("new picture"=w3991:picture)  [unwired: 3 in]
            n1550 = call <vilib>:"Draw Line.vi"("picture"=w3991, "end point"=w3995, "color(black)"=u32 16448250, "pen"=T1 {"Width"=3, "Style"=enum."Solid"}) -> ("new picture"=w3946:picture)  [unwired: 5 in]
            n1551 = call <vilib>:"Move Pen.vi"("new position"=w3971, "picture"=w3946) -> ("new picture"=w3970:picture)  [unwired: 3 in]
            n1552 = call <vilib>:"Draw Line.vi"("picture"=w3970, "end point"=w3972, "color(black)"=u32 16448250, "pen"=T1 {"Width"=3, "Style"=enum."Solid"}) -> ("new picture"=w3945:picture)  [unwired: 5 in]
            n1553 = call <vilib>:"Move Pen.vi"("new position"=w3981, "picture"=w3945) -> ("new picture"=w3980:picture)  [unwired: 3 in]
            n1554 = call <vilib>:"Draw Line.vi"("picture"=w3980, "end point"=w3982, "color(black)"=u32 16448250, "pen"=T1 {"Width"=3, "Style"=enum."Solid"}) -> ("new picture"=w3944:picture)  [unwired: 5 in]
            n1555 = call <vilib>:"Move Pen.vi"("new position"=w3959, "picture"=w3944) -> ("new picture"=w3958:picture)  [unwired: 3 in]
            n1556 = call <vilib>:"Draw Line.vi"("picture"=w3958, "end point"=w3962, "color(black)"=u32 16448250, "pen"=T1 {"Width"=3, "Style"=enum."Solid"}) -> ("new picture"=w3943:picture)  [unwired: 5 in]
          }
          frame 7 {
            n1557 = Add(x=w4027, y=0) -> (x+y=w4060:i32)
            n1558 = Add(x=w4026, y=0) -> (x+y=w4061:i32)
            n1559 = Multiply(x=w4025, y=10) -> (x*y=w4059:i32)
            n1560 = Add(x=w4061, y=w4059) -> (x+y=w4062:i32)
            n1561 = Add(x=w4027, y=0) -> (x+y=w4072:i32)
            n1562 = Add(x=w4026, y=0) -> (x+y=w4073:i32)
            n1563 = Bundle(w4060, w4061) -> (w4057:cluster{i32, i32})  [unwired: 1 in]
            n1564 = Multiply(x=w4025, y=10) -> (x*y=w4070:i32)
            n1565 = Add(x=w4072, y=w4070) -> (x+y=w4071:i32)
            n1566 = Bundle(w4072, w4073) -> (w4069:cluster{i32, i32})  [unwired: 1 in]
            n1567 = Bundle(w4060, w4062) -> (w4058:cluster{i32, i32})  [unwired: 1 in]
            n1568 = call <vilib>:"Move Pen.vi"("new position"=w4069, "picture"=w4029) -> ("new picture"=w4068:picture)  [unwired: 3 in]
            n1569 = Bundle(w4071, w4073) -> (w4074:cluster{i32, i32})  [unwired: 1 in]
            n1570 = call <vilib>:"Draw Line.vi"("picture"=w4068, "end point"=w4074, "color(black)"=u32 16448250, "pen"=T1 {"Width"=3, "Style"=enum."Solid"}) -> ("new picture"=w4028:picture)  [unwired: 5 in]
            n1571 = Multiply(x=w4025, y=10) -> (x*y=w4047:i32)
            n1572 = Add(x=w4027, y=w4047) -> (x+y=w4048:i32)
            n1573 = Add(x=w4026, y=0) -> (x+y=w4050:i32)
            n1574 = Multiply(x=w4025, y=10) -> (x*y=w4039:i32)
            n1575 = Add(x=w4027, y=w4039) -> (x+y=w4036:i32)
            n1576 = Add(x=w4026, y=w4039) -> (x+y=w4038:i32)
            n1577 = Add(x=w4050, y=w4047) -> (x+y=w4049:i32)
            n1578 = Bundle(w4048, w4050) -> (w4045:cluster{i32, i32})  [unwired: 1 in]
            n1579 = Add(x=w4038, y=w4039) -> (x+y=w4037:i32)
            n1580 = Bundle(w4036, w4038) -> (w4034:cluster{i32, i32})  [unwired: 1 in]
            n1581 = Bundle(w4048, w4049) -> (w4046:cluster{i32, i32})  [unwired: 1 in]
            n1582 = call <vilib>:"Move Pen.vi"("new position"=w4034, "picture"=w4028) -> ("new picture"=w4033:picture)  [unwired: 3 in]
            n1583 = Bundle(w4036, w4037) -> (w4035:cluster{i32, i32})  [unwired: 1 in]
            n1584 = call <vilib>:"Draw Line.vi"("picture"=w4033, "end point"=w4035, "color(black)"=u32 16448250, "pen"=T1 {"Width"=3, "Style"=enum."Solid"}) -> ("new picture"=w4024:picture)  [unwired: 5 in]
            n1585 = call <vilib>:"Move Pen.vi"("new position"=w4057, "picture"=w4024) -> ("new picture"=w4056:picture)  [unwired: 3 in]
            n1586 = call <vilib>:"Draw Line.vi"("picture"=w4056, "end point"=w4058, "color(black)"=u32 16448250, "pen"=T1 {"Width"=3, "Style"=enum."Solid"}) -> ("new picture"=w4023:picture)  [unwired: 5 in]
            n1587 = call <vilib>:"Move Pen.vi"("new position"=w4045, "picture"=w4023) -> ("new picture"=w4044:picture)  [unwired: 3 in]
            n1588 = call <vilib>:"Draw Line.vi"("picture"=w4044, "end point"=w4046, "color(black)"=u32 16448250, "pen"=T1 {"Width"=3, "Style"=enum."Solid"}) -> ("new picture"=w4022:picture)  [unwired: 5 in]
          }
          frame 8 {
            n1589 = Add(x=w4083, y=0) -> (x+y=w4151:i32)
            n1590 = Add(x=w4082, y=0) -> (x+y=w4152:i32)
            n1591 = Add(x=w4083, y=0) -> (x+y=w4106:i32)
            n1592 = Multiply(x=w4081, y=10) -> (x*y=w4150:i32)
            n1593 = Multiply(x=w4081, y=10) -> (x*y=w4109:i32)
            n1594 = Add(x=w4082, y=w4109) -> (x+y=w4107:i32)
            n1595 = Add(x=w4083, y=0) -> (x+y=w4163:i32)
            n1596 = Add(x=w4082, y=0) -> (x+y=w4164:i32)
            n1597 = Multiply(x=w4081, y=10) -> (x*y=w4161:i32)
            n1598 = Add(x=w4152, y=w4150) -> (x+y=w4153:i32)
            n1599 = Add(x=w4107, y=w4109) -> (x+y=w4108:i32)
            n1600 = Bundle(w4151, w4152) -> (w4148:cluster{i32, i32})  [unwired: 1 in]
            n1601 = Bundle(w4106, w4107) -> (w4104:cluster{i32, i32})  [unwired: 1 in]
            n1602 = Multiply(x=w4081, y=10) -> (x*y=w4097:i32)
            n1603 = Multiply(x=2, y=w4097) -> (x*y=w4098:i32)
            n1604 = Add(x=w4163, y=w4161) -> (x+y=w4162:i32)
            n1605 = Bundle(w4163, w4164) -> (w4160:cluster{i32, i32})  [unwired: 1 in]
            n1606 = Add(x=w4083, y=0) -> (x+y=w4094:i32)
            n1607 = Add(x=w4082, y=w4098) -> (x+y=w4096:i32)
            n1608 = Add(x=w4094, y=w4097) -> (x+y=w4093:i32)
            n1609 = Bundle(w4151, w4153) -> (w4149:cluster{i32, i32})  [unwired: 1 in]
            n1610 = Bundle(w4106, w4108) -> (w4105:cluster{i32, i32})  [unwired: 1 in]
            n1611 = Bundle(w4094, w4096) -> (w4092:cluster{i32, i32})  [unwired: 1 in]
            n1612 = call <vilib>:"Move Pen.vi"("new position"=w4160, "picture"=w4085) -> ("new picture"=w4159:picture)  [unwired: 3 in]
            n1613 = Bundle(w4162, w4164) -> (w4165:cluster{i32, i32})  [unwired: 1 in]
            n1614 = Bundle(w4093, w4096) -> (w4095:cluster{i32, i32})  [unwired: 1 in]
            n1615 = call <vilib>:"Draw Line.vi"("picture"=w4159, "end point"=w4165, "color(black)"=u32 16448250, "pen"=T1 {"Width"=3, "Style"=enum."Solid"}) -> ("new picture"=w4084:picture)  [unwired: 5 in]
            n1616 = Multiply(x=w4081, y=10) -> (x*y=w4129:i32)
            n1617 = Multiply(x=w4081, y=10) -> (x*y=w4138:i32)
            n1618 = Add(x=w4083, y=0) -> (x+y=w4127:i32)
            n1619 = Multiply(x=w4081, y=10) -> (x*y=w4119:i32)
            n1620 = Add(x=w4082, y=w4129) -> (x+y=w4130:i32)
            n1621 = Add(x=w4083, y=w4138) -> (x+y=w4139:i32)
            n1622 = Add(x=w4082, y=0) -> (x+y=w4141:i32)
            n1623 = Add(x=w4083, y=w4119) -> (x+y=w4116:i32)
            n1624 = Add(x=w4082, y=w4119) -> (x+y=w4118:i32)
            n1625 = Add(x=w4127, y=w4129) -> (x+y=w4126:i32)
            n1626 = Bundle(w4127, w4130) -> (w4125:cluster{i32, i32})  [unwired: 1 in]
            n1627 = Add(x=w4141, y=w4138) -> (x+y=w4140:i32)
            n1628 = Add(x=w4118, y=w4119) -> (x+y=w4117:i32)
            n1629 = Bundle(w4139, w4141) -> (w4136:cluster{i32, i32})  [unwired: 1 in]
            n1630 = Bundle(w4116, w4118) -> (w4114:cluster{i32, i32})  [unwired: 1 in]
            n1631 = call <vilib>:"Move Pen.vi"("new position"=w4125, "picture"=w4084) -> ("new picture"=w4124:picture)  [unwired: 3 in]
            n1632 = Bundle(w4126, w4130) -> (w4128:cluster{i32, i32})  [unwired: 1 in]
            n1633 = Bundle(w4139, w4140) -> (w4137:cluster{i32, i32})  [unwired: 1 in]
            n1634 = Bundle(w4116, w4117) -> (w4115:cluster{i32, i32})  [unwired: 1 in]
            n1635 = call <vilib>:"Draw Line.vi"("picture"=w4124, "end point"=w4128, "color(black)"=u32 16448250, "pen"=T1 {"Width"=3, "Style"=enum."Solid"}) -> ("new picture"=w4080:picture)  [unwired: 5 in]
            n1636 = call <vilib>:"Move Pen.vi"("new position"=w4148, "picture"=w4080) -> ("new picture"=w4147:picture)  [unwired: 3 in]
            n1637 = call <vilib>:"Draw Line.vi"("picture"=w4147, "end point"=w4149, "color(black)"=u32 16448250, "pen"=T1 {"Width"=3, "Style"=enum."Solid"}) -> ("new picture"=w4079:picture)  [unwired: 5 in]
            n1638 = call <vilib>:"Move Pen.vi"("new position"=w4136, "picture"=w4079) -> ("new picture"=w4135:picture)  [unwired: 3 in]
            n1639 = call <vilib>:"Draw Line.vi"("picture"=w4135, "end point"=w4137, "color(black)"=u32 16448250, "pen"=T1 {"Width"=3, "Style"=enum."Solid"}) -> ("new picture"=w4078:picture)  [unwired: 5 in]
            n1640 = call <vilib>:"Move Pen.vi"("new position"=w4104, "picture"=w4078) -> ("new picture"=w4103:picture)  [unwired: 3 in]
            n1641 = call <vilib>:"Draw Line.vi"("picture"=w4103, "end point"=w4105, "color(black)"=u32 16448250, "pen"=T1 {"Width"=3, "Style"=enum."Solid"}) -> ("new picture"=w4077:picture)  [unwired: 5 in]
            n1642 = call <vilib>:"Move Pen.vi"("new position"=w4114, "picture"=w4077) -> ("new picture"=w4113:picture)  [unwired: 3 in]
            n1643 = call <vilib>:"Draw Line.vi"("picture"=w4113, "end point"=w4115, "color(black)"=u32 16448250, "pen"=T1 {"Width"=3, "Style"=enum."Solid"}) -> ("new picture"=w4076:picture)  [unwired: 5 in]
            n1644 = call <vilib>:"Move Pen.vi"("new position"=w4092, "picture"=w4076) -> ("new picture"=w4091:picture)  [unwired: 3 in]
            n1645 = call <vilib>:"Draw Line.vi"("picture"=w4091, "end point"=w4095, "color(black)"=u32 16448250, "pen"=T1 {"Width"=3, "Style"=enum."Solid"}) -> ("new picture"=w4075:picture)  [unwired: 5 in]
          }
          frame 9 {
            n1646 = Add(x=w4172, y=0) -> (x+y=w4216:i32)
            n1647 = Add(x=w4171, y=0) -> (x+y=w4217:i32)
            n1648 = Add(x=w4172, y=0) -> (x+y=w4228:i32)
            n1649 = Add(x=w4171, y=0) -> (x+y=w4229:i32)
            n1650 = Multiply(x=w4170, y=10) -> (x*y=w4215:i32)
            n1651 = Multiply(x=w4170, y=10) -> (x*y=w4226:i32)
            n1652 = Add(x=w4217, y=w4215) -> (x+y=w4218:i32)
            n1653 = Add(x=w4228, y=w4226) -> (x+y=w4227:i32)
            n1654 = Bundle(w4216, w4217) -> (w4213:cluster{i32, i32})  [unwired: 1 in]
            n1655 = Bundle(w4228, w4229) -> (w4225:cluster{i32, i32})  [unwired: 1 in]
            n1656 = Bundle(w4216, w4218) -> (w4214:cluster{i32, i32})  [unwired: 1 in]
            n1657 = call <vilib>:"Move Pen.vi"("new position"=w4225, "picture"=w4174) -> ("new picture"=w4224:picture)  [unwired: 3 in]
            n1658 = Bundle(w4227, w4229) -> (w4230:cluster{i32, i32})  [unwired: 1 in]
            n1659 = Multiply(x=w4170, y=10) -> (x*y=w4184:i32)
            n1660 = Add(x=w4172, y=w4184) -> (x+y=w4181:i32)
            n1661 = Add(x=w4171, y=w4184) -> (x+y=w4183:i32)
            n1662 = Add(x=w4183, y=w4184) -> (x+y=w4182:i32)
            n1663 = Bundle(w4181, w4183) -> (w4179:cluster{i32, i32})  [unwired: 1 in]
            n1664 = call <vilib>:"Draw Line.vi"("picture"=w4224, "end point"=w4230, "color(black)"=u32 16448250, "pen"=T1 {"Width"=3, "Style"=enum."Solid"}) -> ("new picture"=w4173:picture)  [unwired: 5 in]
            n1665 = Bundle(w4181, w4182) -> (w4180:cluster{i32, i32})  [unwired: 1 in]
            n1666 = Multiply(x=w4170, y=10) -> (x*y=w4203:i32)
            n1667 = Add(x=w4172, y=w4203) -> (x+y=w4204:i32)
            n1668 = Add(x=w4171, y=0) -> (x+y=w4206:i32)
            n1669 = Multiply(x=w4170, y=10) -> (x*y=w4194:i32)
            n1670 = Add(x=w4172, y=0) -> (x+y=w4192:i32)
            n1671 = Add(x=w4171, y=w4194) -> (x+y=w4195:i32)
            n1672 = Add(x=w4206, y=w4203) -> (x+y=w4205:i32)
            n1673 = Add(x=w4192, y=w4194) -> (x+y=w4191:i32)
            n1674 = Bundle(w4204, w4206) -> (w4201:cluster{i32, i32})  [unwired: 1 in]
            n1675 = Bundle(w4192, w4195) -> (w4190:cluster{i32, i32})  [unwired: 1 in]
            n1676 = Bundle(w4204, w4205) -> (w4202:cluster{i32, i32})  [unwired: 1 in]
            n1677 = call <vilib>:"Move Pen.vi"("new position"=w4190, "picture"=w4173) -> ("new picture"=w4189:picture)  [unwired: 3 in]
            n1678 = Bundle(w4191, w4195) -> (w4193:cluster{i32, i32})  [unwired: 1 in]
            n1679 = call <vilib>:"Draw Line.vi"("picture"=w4189, "end point"=w4193, "color(black)"=u32 16448250, "pen"=T1 {"Width"=3, "Style"=enum."Solid"}) -> ("new picture"=w4169:picture)  [unwired: 5 in]
            n1680 = call <vilib>:"Move Pen.vi"("new position"=w4213, "picture"=w4169) -> ("new picture"=w4212:picture)  [unwired: 3 in]
            n1681 = call <vilib>:"Draw Line.vi"("picture"=w4212, "end point"=w4214, "color(black)"=u32 16448250, "pen"=T1 {"Width"=3, "Style"=enum."Solid"}) -> ("new picture"=w4168:picture)  [unwired: 5 in]
            n1682 = call <vilib>:"Move Pen.vi"("new position"=w4201, "picture"=w4168) -> ("new picture"=w4200:picture)  [unwired: 3 in]
            n1683 = call <vilib>:"Draw Line.vi"("picture"=w4200, "end point"=w4202, "color(black)"=u32 16448250, "pen"=T1 {"Width"=3, "Style"=enum."Solid"}) -> ("new picture"=w4167:picture)  [unwired: 5 in]
            n1684 = call <vilib>:"Move Pen.vi"("new position"=w4179, "picture"=w4167) -> ("new picture"=w4178:picture)  [unwired: 3 in]
            n1685 = call <vilib>:"Draw Line.vi"("picture"=w4178, "end point"=w4180, "color(black)"=u32 16448250, "pen"=T1 {"Width"=3, "Style"=enum."Solid"}) -> ("new picture"=w4166:picture)  [unwired: 5 in]
          }
        }
        n1686 = case shown="9" w148 {
          tunnel: 460 -> [w2947 w3021 w3051 w3119 w3184 w3236 w3304 w3381 w3437 w3526]
          tunnel: 10 -> [w2946 w3020 w3050 w3118 w3183 w3235 w3303 w3380 w3436 w3525]
          tunnel: 3 -> [w2945 w3019 w3049 w3117 w3182 w3234 w3302 w3379 w3435 w3524]
          tunnel: w172 -> [w2948 w3023 w3053 w3120 w3185 w3238 w3306 w3383 w3439 w3528]
          tunnel: [w2939 w3018 w3045 w3112 w3178 w3230 w3297 w3376 w3429 w3520] -> w163
          frame 0, Default {
            n1687 = Add(x=w2947, y=0) -> (x+y=w3003:i32)
            n1688 = Add(x=w2946, y=0) -> (x+y=w3004:i32)
            n1689 = Multiply(x=w2945, y=10) -> (x*y=w3002:i32)
            n1690 = Add(x=w2947, y=0) -> (x+y=w2969:i32)
            n1691 = Multiply(x=w2945, y=10) -> (x*y=w2972:i32)
            n1692 = Add(x=w2946, y=w2972) -> (x+y=w2970:i32)
            n1693 = Add(x=w3004, y=w3002) -> (x+y=w3005:i32)
            n1694 = Add(x=w2970, y=w2972) -> (x+y=w2971:i32)
            n1695 = Bundle(w3003, w3004) -> (w3000:cluster{i32, i32})  [unwired: 1 in]
            n1696 = Bundle(w2969, w2970) -> (w2967:cluster{i32, i32})  [unwired: 1 in]
            n1697 = Bundle(w3003, w3005) -> (w3001:cluster{i32, i32})  [unwired: 1 in]
            n1698 = Bundle(w2969, w2971) -> (w2968:cluster{i32, i32})  [unwired: 1 in]
            n1699 = Multiply(x=w2945, y=10) -> (x*y=w2960:i32)
            n1700 = Multiply(x=2, y=w2960) -> (x*y=w2961:i32)
            n1701 = Add(x=w2947, y=0) -> (x+y=w3015:i32)
            n1702 = Add(x=w2946, y=0) -> (x+y=w3016:i32)
            n1703 = Add(x=w2947, y=0) -> (x+y=w2957:i32)
            n1704 = Add(x=w2946, y=w2961) -> (x+y=w2959:i32)
            n1705 = Multiply(x=w2945, y=10) -> (x*y=w3013:i32)
            n1706 = Add(x=w2957, y=w2960) -> (x+y=w2956:i32)
            n1707 = Add(x=w3015, y=w3013) -> (x+y=w3014:i32)
            n1708 = Bundle(w3015, w3016) -> (w3012:cluster{i32, i32})  [unwired: 1 in]
            n1709 = Bundle(w2957, w2959) -> (w2955:cluster{i32, i32})  [unwired: 1 in]
            n1710 = call <vilib>:"Move Pen.vi"("new position"=w3012, "picture"=w2948) -> ("new picture"=w3011:picture)  [unwired: 3 in]
            n1711 = Bundle(w3014, w3016) -> (w3017:cluster{i32, i32})  [unwired: 1 in]
            n1712 = Bundle(w2956, w2959) -> (w2958:cluster{i32, i32})  [unwired: 1 in]
            n1713 = Multiply(x=w2945, y=10) -> (x*y=w2990:i32)
            n1714 = Add(x=w2947, y=w2990) -> (x+y=w2991:i32)
            n1715 = Add(x=w2946, y=0) -> (x+y=w2993:i32)
            n1716 = Multiply(x=w2945, y=10) -> (x*y=w2982:i32)
            n1717 = Add(x=w2947, y=w2982) -> (x+y=w2979:i32)
            n1718 = Add(x=w2946, y=w2982) -> (x+y=w2981:i32)
            n1719 = Add(x=w2993, y=w2990) -> (x+y=w2992:i32)
            n1720 = Bundle(w2991, w2993) -> (w2988:cluster{i32, i32})  [unwired: 1 in]
            n1721 = call <vilib>:"Draw Line.vi"("picture"=w3011, "end point"=w3017, "color(black)"=u32 16448250, "pen"=T1 {"Width"=3, "Style"=enum."Solid"}) -> ("new picture"=w2944:picture)  [unwired: 5 in]
            n1722 = call <vilib>:"Move Pen.vi"("new position"=w3000, "picture"=w2944) -> ("new picture"=w2999:picture)  [unwired: 3 in]
            n1723 = call <vilib>:"Draw Line.vi"("picture"=w2999, "end point"=w3001, "color(black)"=u32 16448250, "pen"=T1 {"Width"=3, "Style"=enum."Solid"}) -> ("new picture"=w2943:picture)  [unwired: 5 in]
            n1724 = Add(x=w2981, y=w2982) -> (x+y=w2980:i32)
            n1725 = Bundle(w2979, w2981) -> (w2977:cluster{i32, i32})  [unwired: 1 in]
            n1726 = call <vilib>:"Move Pen.vi"("new position"=w2988, "picture"=w2943) -> ("new picture"=w2987:picture)  [unwired: 3 in]
            n1727 = Bundle(w2991, w2992) -> (w2989:cluster{i32, i32})  [unwired: 1 in]
            n1728 = Bundle(w2979, w2980) -> (w2978:cluster{i32, i32})  [unwired: 1 in]
            n1729 = call <vilib>:"Draw Line.vi"("picture"=w2987, "end point"=w2989, "color(black)"=u32 16448250, "pen"=T1 {"Width"=3, "Style"=enum."Solid"}) -> ("new picture"=w2942:picture)  [unwired: 5 in]
            n1730 = call <vilib>:"Move Pen.vi"("new position"=w2967, "picture"=w2942) -> ("new picture"=w2966:picture)  [unwired: 3 in]
            n1731 = call <vilib>:"Draw Line.vi"("picture"=w2966, "end point"=w2968, "color(black)"=u32 16448250, "pen"=T1 {"Width"=3, "Style"=enum."Solid"}) -> ("new picture"=w2941:picture)  [unwired: 5 in]
            n1732 = call <vilib>:"Move Pen.vi"("new position"=w2977, "picture"=w2941) -> ("new picture"=w2976:picture)  [unwired: 3 in]
            n1733 = call <vilib>:"Draw Line.vi"("picture"=w2976, "end point"=w2978, "color(black)"=u32 16448250, "pen"=T1 {"Width"=3, "Style"=enum."Solid"}) -> ("new picture"=w2940:picture)  [unwired: 5 in]
            n1734 = call <vilib>:"Move Pen.vi"("new position"=w2955, "picture"=w2940) -> ("new picture"=w2954:picture)  [unwired: 3 in]
            n1735 = call <vilib>:"Draw Line.vi"("picture"=w2954, "end point"=w2958, "color(black)"=u32 16448250, "pen"=T1 {"Width"=3, "Style"=enum."Solid"}) -> ("new picture"=w2939:picture)  [unwired: 5 in]
          }
          frame 1 {
            n1736 = Multiply(x=w3019, y=10) -> (x*y=w3041:i32)
            n1737 = Add(x=w3021, y=w3041) -> (x+y=w3042:i32)
            n1738 = Add(x=w3020, y=0) -> (x+y=w3044:i32)
            n1739 = Add(x=w3044, y=w3041) -> (x+y=w3043:i32)
            n1740 = Bundle(w3042, w3044) -> (w3039:cluster{i32, i32})  [unwired: 1 in]
            n1741 = call <vilib>:"Move Pen.vi"("new position"=w3039, "picture"=w3023) -> ("new picture"=w3038:picture)  [unwired: 3 in]
            n1742 = Bundle(w3042, w3043) -> (w3040:cluster{i32, i32})  [unwired: 1 in]
            n1743 = call <vilib>:"Draw Line.vi"("picture"=w3038, "end point"=w3040, "color(black)"=u32 16448250, "pen"=T1 {"Width"=3, "Style"=enum."Solid"}) -> ("new picture"=w3022:picture)  [unwired: 5 in]
            n1744 = Multiply(x=w3019, y=10) -> (x*y=w3033:i32)
            n1745 = Add(x=w3021, y=w3033) -> (x+y=w3030:i32)
            n1746 = Add(x=w3020, y=w3033) -> (x+y=w3032:i32)
            n1747 = Add(x=w3032, y=w3033) -> (x+y=w3031:i32)
            n1748 = Bundle(w3030, w3032) -> (w3028:cluster{i32, i32})  [unwired: 1 in]
            n1749 = call <vilib>:"Move Pen.vi"("new position"=w3028, "picture"=w3022) -> ("new picture"=w3027:picture)  [unwired: 3 in]
            n1750 = Bundle(w3030, w3031) -> (w3029:cluster{i32, i32})  [unwired: 1 in]
            n1751 = call <vilib>:"Draw Line.vi"("picture"=w3027, "end point"=w3029, "color(black)"=u32 16448250, "pen"=T1 {"Width"=3, "Style"=enum."Solid"}) -> ("new picture"=w3018:picture)  [unwired: 5 in]
          }
          frame 2 {
            n1752 = Multiply(x=w3049, y=10) -> (x*y=w3087:i32)
            n1753 = Add(x=w3051, y=0) -> (x+y=w3085:i32)
            n1754 = Add(x=w3050, y=w3087) -> (x+y=w3088:i32)
            n1755 = Add(x=w3051, y=0) -> (x+y=w3109:i32)
            n1756 = Add(x=w3050, y=0) -> (x+y=w3110:i32)
            n1757 = Multiply(x=w3049, y=10) -> (x*y=w3107:i32)
            n1758 = Add(x=w3085, y=w3087) -> (x+y=w3084:i32)
            n1759 = Add(x=w3109, y=w3107) -> (x+y=w3108:i32)
            n1760 = Bundle(w3085, w3088) -> (w3083:cluster{i32, i32})  [unwired: 1 in]
            n1761 = Bundle(w3109, w3110) -> (w3106:cluster{i32, i32})  [unwired: 1 in]
            n1762 = Bundle(w3084, w3088) -> (w3086:cluster{i32, i32})  [unwired: 1 in]
            n1763 = call <vilib>:"Move Pen.vi"("new position"=w3106, "picture"=w3053) -> ("new picture"=w3105:picture)  [unwired: 3 in]
            n1764 = Bundle(w3108, w3110) -> (w3111:cluster{i32, i32})  [unwired: 1 in]
            n1765 = Multiply(x=w3049, y=10) -> (x*y=w3065:i32)
            n1766 = Multiply(x=2, y=w3065) -> (x*y=w3066:i32)
            n1767 = Add(x=w3051, y=0) -> (x+y=w3062:i32)
            n1768 = Add(x=w3050, y=w3066) -> (x+y=w3064:i32)
            n1769 = Add(x=w3062, y=w3065) -> (x+y=w3061:i32)
            n1770 = Bundle(w3062, w3064) -> (w3060:cluster{i32, i32})  [unwired: 1 in]
            n1771 = call <vilib>:"Draw Line.vi"("picture"=w3105, "end point"=w3111, "color(black)"=u32 16448250, "pen"=T1 {"Width"=3, "Style"=enum."Solid"}) -> ("new picture"=w3052:picture)  [unwired: 5 in]
            n1772 = Bundle(w3061, w3064) -> (w3063:cluster{i32, i32})  [unwired: 1 in]
            n1773 = Multiply(x=w3049, y=10) -> (x*y=w3096:i32)
            n1774 = Add(x=w3051, y=0) -> (x+y=w3074:i32)
            n1775 = Add(x=w3051, y=w3096) -> (x+y=w3097:i32)
            n1776 = Add(x=w3050, y=0) -> (x+y=w3099:i32)
            n1777 = Multiply(x=w3049, y=10) -> (x*y=w3077:i32)
            n1778 = Add(x=w3050, y=w3077) -> (x+y=w3075:i32)
            n1779 = Add(x=w3075, y=w3077) -> (x+y=w3076:i32)
            n1780 = Add(x=w3099, y=w3096) -> (x+y=w3098:i32)
            n1781 = Bundle(w3074, w3075) -> (w3072:cluster{i32, i32})  [unwired: 1 in]
            n1782 = Bundle(w3097, w3099) -> (w3094:cluster{i32, i32})  [unwired: 1 in]
            n1783 = call <vilib>:"Move Pen.vi"("new position"=w3094, "picture"=w3052) -> ("new picture"=w3093:picture)  [unwired: 3 in]
            n1784 = Bundle(w3074, w3076) -> (w3073:cluster{i32, i32})  [unwired: 1 in]
            n1785 = Bundle(w3097, w3098) -> (w3095:cluster{i32, i32})  [unwired: 1 in]
            n1786 = call <vilib>:"Draw Line.vi"("picture"=w3093, "end point"=w3095, "color(black)"=u32 16448250, "pen"=T1 {"Width"=3, "Style"=enum."Solid"}) -> ("new picture"=w3048:picture)  [unwired: 5 in]
            n1787 = call <vilib>:"Move Pen.vi"("new position"=w3083, "picture"=w3048) -> ("new picture"=w3082:picture)  [unwired: 3 in]
            n1788 = call <vilib>:"Draw Line.vi"("picture"=w3082, "end point"=w3086, "color(black)"=u32 16448250, "pen"=T1 {"Width"=3, "Style"=enum."Solid"}) -> ("new picture"=w3047:picture)  [unwired: 5 in]
            n1789 = call <vilib>:"Move Pen.vi"("new position"=w3072, "picture"=w3047) -> ("new picture"=w3071:picture)  [unwired: 3 in]
            n1790 = call <vilib>:"Draw Line.vi"("picture"=w3071, "end point"=w3073, "color(black)"=u32 16448250, "pen"=T1 {"Width"=3, "Style"=enum."Solid"}) -> ("new picture"=w3046:picture)  [unwired: 5 in]
            n1791 = call <vilib>:"Move Pen.vi"("new position"=w3060, "picture"=w3046) -> ("new picture"=w3059:picture)  [unwired: 3 in]
            n1792 = call <vilib>:"Draw Line.vi"("picture"=w3059, "end point"=w3063, "color(black)"=u32 16448250, "pen"=T1 {"Width"=3, "Style"=enum."Solid"}) -> ("new picture"=w3045:picture)  [unwired: 5 in]
          }
          frame 3 {
            n1793 = Multiply(x=w3117, y=10) -> (x*y=w3153:i32)
            n1794 = Add(x=w3119, y=0) -> (x+y=w3151:i32)
            n1795 = Add(x=w3118, y=w3153) -> (x+y=w3154:i32)
            n1796 = Add(x=w3119, y=0) -> (x+y=w3175:i32)
            n1797 = Add(x=w3118, y=0) -> (x+y=w3176:i32)
            n1798 = Multiply(x=w3117, y=10) -> (x*y=w3173:i32)
            n1799 = Add(x=w3151, y=w3153) -> (x+y=w3150:i32)
            n1800 = Add(x=w3175, y=w3173) -> (x+y=w3174:i32)
            n1801 = Bundle(w3151, w3154) -> (w3149:cluster{i32, i32})  [unwired: 1 in]
            n1802 = Bundle(w3175, w3176) -> (w3172:cluster{i32, i32})  [unwired: 1 in]
            n1803 = call <vilib>:"Move Pen.vi"("new position"=w3172, "picture"=w3120) -> ("new picture"=w3171:picture)  [unwired: 3 in]
            n1804 = Bundle(w3150, w3154) -> (w3152:cluster{i32, i32})  [unwired: 1 in]
            n1805 = Bundle(w3174, w3176) -> (w3177:cluster{i32, i32})  [unwired: 1 in]
            n1806 = Multiply(x=w3117, y=10) -> (x*y=w3132:i32)
            n1807 = Multiply(x=2, y=w3132) -> (x*y=w3133:i32)
            n1808 = Add(x=w3119, y=0) -> (x+y=w3129:i32)
            n1809 = Add(x=w3118, y=w3133) -> (x+y=w3131:i32)
            n1810 = Add(x=w3129, y=w3132) -> (x+y=w3128:i32)
            n1811 = call <vilib>:"Draw Line.vi"("picture"=w3171, "end point"=w3177, "color(black)"=u32 16448250, "pen"=T1 {"Width"=3, "Style"=enum."Solid"}) -> ("new picture"=w3116:picture)  [unwired: 5 in]
            n1812 = Bundle(w3129, w3131) -> (w3127:cluster{i32, i32})  [unwired: 1 in]
            n1813 = Bundle(w3128, w3131) -> (w3130:cluster{i32, i32})  [unwired: 1 in]
            n1814 = Multiply(x=w3117, y=10) -> (x*y=w3143:i32)
            n1815 = Add(x=w3119, y=w3143) -> (x+y=w3140:i32)
            n1816 = Add(x=w3118, y=w3143) -> (x+y=w3142:i32)
            n1817 = Multiply(x=w3117, y=10) -> (x*y=w3162:i32)
            n1818 = Add(x=w3119, y=w3162) -> (x+y=w3163:i32)
            n1819 = Add(x=w3118, y=0) -> (x+y=w3165:i32)
            n1820 = Add(x=w3142, y=w3143) -> (x+y=w3141:i32)
            n1821 = Bundle(w3140, w3142) -> (w3138:cluster{i32, i32})  [unwired: 1 in]
            n1822 = Add(x=w3165, y=w3162) -> (x+y=w3164:i32)
            n1823 = Bundle(w3163, w3165) -> (w3160:cluster{i32, i32})  [unwired: 1 in]
            n1824 = Bundle(w3140, w3141) -> (w3139:cluster{i32, i32})  [unwired: 1 in]
            n1825 = call <vilib>:"Move Pen.vi"("new position"=w3160, "picture"=w3116) -> ("new picture"=w3159:picture)  [unwired: 3 in]
            n1826 = Bundle(w3163, w3164) -> (w3161:cluster{i32, i32})  [unwired: 1 in]
            n1827 = call <vilib>:"Draw Line.vi"("picture"=w3159, "end point"=w3161, "color(black)"=u32 16448250, "pen"=T1 {"Width"=3, "Style"=enum."Solid"}) -> ("new picture"=w3115:picture)  [unwired: 5 in]
            n1828 = call <vilib>:"Move Pen.vi"("new position"=w3149, "picture"=w3115) -> ("new picture"=w3148:picture)  [unwired: 3 in]
            n1829 = call <vilib>:"Draw Line.vi"("picture"=w3148, "end point"=w3152, "color(black)"=u32 16448250, "pen"=T1 {"Width"=3, "Style"=enum."Solid"}) -> ("new picture"=w3114:picture)  [unwired: 5 in]
            n1830 = call <vilib>:"Move Pen.vi"("new position"=w3138, "picture"=w3114) -> ("new picture"=w3137:picture)  [unwired: 3 in]
            n1831 = call <vilib>:"Draw Line.vi"("picture"=w3137, "end point"=w3139, "color(black)"=u32 16448250, "pen"=T1 {"Width"=3, "Style"=enum."Solid"}) -> ("new picture"=w3113:picture)  [unwired: 5 in]
            n1832 = call <vilib>:"Move Pen.vi"("new position"=w3127, "picture"=w3113) -> ("new picture"=w3126:picture)  [unwired: 3 in]
            n1833 = call <vilib>:"Draw Line.vi"("picture"=w3126, "end point"=w3130, "color(black)"=u32 16448250, "pen"=T1 {"Width"=3, "Style"=enum."Solid"}) -> ("new picture"=w3112:picture)  [unwired: 5 in]
          }
          frame 4 {
            n1834 = Add(x=w3184, y=0) -> (x+y=w3227:i32)
            n1835 = Add(x=w3183, y=0) -> (x+y=w3228:i32)
            n1836 = Multiply(x=w3182, y=10) -> (x*y=w3226:i32)
            n1837 = Add(x=w3228, y=w3226) -> (x+y=w3229:i32)
            n1838 = Bundle(w3227, w3228) -> (w3224:cluster{i32, i32})  [unwired: 1 in]
            n1839 = call <vilib>:"Move Pen.vi"("new position"=w3224, "picture"=w3185) -> ("new picture"=w3223:picture)  [unwired: 3 in]
            n1840 = Bundle(w3227, w3229) -> (w3225:cluster{i32, i32})  [unwired: 1 in]
            n1841 = Multiply(x=w3182, y=10) -> (x*y=w3205:i32)
            n1842 = Add(x=w3184, y=0) -> (x+y=w3203:i32)
            n1843 = Add(x=w3183, y=w3205) -> (x+y=w3206:i32)
            n1844 = Add(x=w3203, y=w3205) -> (x+y=w3202:i32)
            n1845 = Bundle(w3203, w3206) -> (w3201:cluster{i32, i32})  [unwired: 1 in]
            n1846 = call <vilib>:"Draw Line.vi"("picture"=w3223, "end point"=w3225, "color(black)"=u32 16448250, "pen"=T1 {"Width"=3, "Style"=enum."Solid"}) -> ("new picture"=w3179:picture)  [unwired: 5 in]
            n1847 = Multiply(x=w3182, y=10) -> (x*y=w3195:i32)
            n1848 = Add(x=w3184, y=w3195) -> (x+y=w3192:i32)
            n1849 = Add(x=w3183, y=w3195) -> (x+y=w3194:i32)
            n1850 = Bundle(w3202, w3206) -> (w3204:cluster{i32, i32})  [unwired: 1 in]
            n1851 = Add(x=w3194, y=w3195) -> (x+y=w3193:i32)
            n1852 = Bundle(w3192, w3194) -> (w3190:cluster{i32, i32})  [unwired: 1 in]
            n1853 = Multiply(x=w3182, y=10) -> (x*y=w3214:i32)
            n1854 = Add(x=w3184, y=w3214) -> (x+y=w3215:i32)
            n1855 = Add(x=w3183, y=0) -> (x+y=w3217:i32)
            n1856 = Add(x=w3217, y=w3214) -> (x+y=w3216:i32)
            n1857 = Bundle(w3192, w3193) -> (w3191:cluster{i32, i32})  [unwired: 1 in]
            n1858 = Bundle(w3215, w3217) -> (w3212:cluster{i32, i32})  [unwired: 1 in]
            n1859 = call <vilib>:"Move Pen.vi"("new position"=w3212, "picture"=w3179) -> ("new picture"=w3211:picture)  [unwired: 3 in]
            n1860 = Bundle(w3215, w3216) -> (w3213:cluster{i32, i32})  [unwired: 1 in]
            n1861 = call <vilib>:"Draw Line.vi"("picture"=w3211, "end point"=w3213, "color(black)"=u32 16448250, "pen"=T1 {"Width"=3, "Style"=enum."Solid"}) -> ("new picture"=w3181:picture)  [unwired: 5 in]
            n1862 = call <vilib>:"Move Pen.vi"("new position"=w3201, "picture"=w3181) -> ("new picture"=w3200:picture)  [unwired: 3 in]
            n1863 = call <vilib>:"Draw Line.vi"("picture"=w3200, "end point"=w3204, "color(black)"=u32 16448250, "pen"=T1 {"Width"=3, "Style"=enum."Solid"}) -> ("new picture"=w3180:picture)  [unwired: 5 in]
            n1864 = call <vilib>:"Move Pen.vi"("new position"=w3190, "picture"=w3180) -> ("new picture"=w3189:picture)  [unwired: 3 in]
            n1865 = call <vilib>:"Draw Line.vi"("picture"=w3189, "end point"=w3191, "color(black)"=u32 16448250, "pen"=T1 {"Width"=3, "Style"=enum."Solid"}) -> ("new picture"=w3178:picture)  [unwired: 5 in]
          }
          frame 5 {
            n1866 = Multiply(x=w3234, y=10) -> (x*y=w3271:i32)
            n1867 = Add(x=w3236, y=0) -> (x+y=w3269:i32)
            n1868 = Add(x=w3235, y=w3271) -> (x+y=w3272:i32)
            n1869 = Add(x=w3236, y=0) -> (x+y=w3294:i32)
            n1870 = Add(x=w3235, y=0) -> (x+y=w3295:i32)
            n1871 = Add(x=w3269, y=w3271) -> (x+y=w3268:i32)
            n1872 = Multiply(x=w3234, y=10) -> (x*y=w3292:i32)
            n1873 = Bundle(w3269, w3272) -> (w3267:cluster{i32, i32})  [unwired: 1 in]
            n1874 = Add(x=w3294, y=w3292) -> (x+y=w3293:i32)
            n1875 = Bundle(w3294, w3295) -> (w3291:cluster{i32, i32})  [unwired: 1 in]
            n1876 = Bundle(w3268, w3272) -> (w3270:cluster{i32, i32})  [unwired: 1 in]
            n1877 = call <vilib>:"Move Pen.vi"("new position"=w3291, "picture"=w3238) -> ("new picture"=w3290:picture)  [unwired: 3 in]
            n1878 = Bundle(w3293, w3295) -> (w3296:cluster{i32, i32})  [unwired: 1 in]
            n1879 = Multiply(x=w3234, y=10) -> (x*y=w3250:i32)
            n1880 = Multiply(x=2, y=w3250) -> (x*y=w3251:i32)
            n1881 = Add(x=w3236, y=0) -> (x+y=w3247:i32)
            n1882 = Add(x=w3235, y=w3251) -> (x+y=w3249:i32)
            n1883 = Add(x=w3247, y=w3250) -> (x+y=w3246:i32)
            n1884 = Bundle(w3247, w3249) -> (w3245:cluster{i32, i32})  [unwired: 1 in]
            n1885 = call <vilib>:"Draw Line.vi"("picture"=w3290, "end point"=w3296, "color(black)"=u32 16448250, "pen"=T1 {"Width"=3, "Style"=enum."Solid"}) -> ("new picture"=w3237:picture)  [unwired: 5 in]
            n1886 = Bundle(w3246, w3249) -> (w3248:cluster{i32, i32})  [unwired: 1 in]
            n1887 = Multiply(x=w3234, y=10) -> (x*y=w3261:i32)
            n1888 = Add(x=w3236, y=0) -> (x+y=w3282:i32)
            n1889 = Add(x=w3235, y=0) -> (x+y=w3283:i32)
            n1890 = Add(x=w3236, y=w3261) -> (x+y=w3258:i32)
            n1891 = Add(x=w3235, y=w3261) -> (x+y=w3260:i32)
            n1892 = Multiply(x=w3234, y=10) -> (x*y=w3281:i32)
            n1893 = Add(x=w3283, y=w3281) -> (x+y=w3284:i32)
            n1894 = Add(x=w3260, y=w3261) -> (x+y=w3259:i32)
            n1895 = Bundle(w3282, w3283) -> (w3279:cluster{i32, i32})  [unwired: 1 in]
            n1896 = Bundle(w3258, w3260) -> (w3256:cluster{i32, i32})  [unwired: 1 in]
            n1897 = call <vilib>:"Move Pen.vi"("new position"=w3279, "picture"=w3237) -> ("new picture"=w3278:picture)  [unwired: 3 in]
            n1898 = Bundle(w3282, w3284) -> (w3280:cluster{i32, i32})  [unwired: 1 in]
            n1899 = Bundle(w3258, w3259) -> (w3257:cluster{i32, i32})  [unwired: 1 in]
            n1900 = call <vilib>:"Draw Line.vi"("picture"=w3278, "end point"=w3280, "color(black)"=u32 16448250, "pen"=T1 {"Width"=3, "Style"=enum."Solid"}) -> ("new picture"=w3233:picture)  [unwired: 5 in]
            n1901 = call <vilib>:"Move Pen.vi"("new position"=w3267, "picture"=w3233) -> ("new picture"=w3266:picture)  [unwired: 3 in]
            n1902 = call <vilib>:"Draw Line.vi"("picture"=w3266, "end point"=w3270, "color(black)"=u32 16448250, "pen"=T1 {"Width"=3, "Style"=enum."Solid"}) -> ("new picture"=w3232:picture)  [unwired: 5 in]
            n1903 = call <vilib>:"Move Pen.vi"("new position"=w3256, "picture"=w3232) -> ("new picture"=w3255:picture)  [unwired: 3 in]
            n1904 = call <vilib>:"Draw Line.vi"("picture"=w3255, "end point"=w3257, "color(black)"=u32 16448250, "pen"=T1 {"Width"=3, "Style"=enum."Solid"}) -> ("new picture"=w3231:picture)  [unwired: 5 in]
            n1905 = call <vilib>:"Move Pen.vi"("new position"=w3245, "picture"=w3231) -> ("new picture"=w3244:picture)  [unwired: 3 in]
            n1906 = call <vilib>:"Draw Line.vi"("picture"=w3244, "end point"=w3248, "color(black)"=u32 16448250, "pen"=T1 {"Width"=3, "Style"=enum."Solid"}) -> ("new picture"=w3230:picture)  [unwired: 5 in]
          }
          frame 6 {
            n1907 = Multiply(x=w3302, y=10) -> (x*y=w3340:i32)
            n1908 = Multiply(x=w3302, y=10) -> (x*y=w3350:i32)
            n1909 = Add(x=w3304, y=w3340) -> (x+y=w3337:i32)
            n1910 = Add(x=w3303, y=w3340) -> (x+y=w3339:i32)
            n1911 = Add(x=w3304, y=0) -> (x+y=w3348:i32)
            n1912 = Add(x=w3303, y=w3350) -> (x+y=w3351:i32)
            n1913 = Add(x=w3304, y=0) -> (x+y=w3373:i32)
            n1914 = Add(x=w3303, y=0) -> (x+y=w3374:i32)
            n1915 = Multiply(x=w3302, y=10) -> (x*y=w3371:i32)
            n1916 = Add(x=w3348, y=w3350) -> (x+y=w3347:i32)
            n1917 = Add(x=w3339, y=w3340) -> (x+y=w3338:i32)
            n1918 = Bundle(w3337, w3339) -> (w3335:cluster{i32, i32})  [unwired: 1 in]
            n1919 = Bundle(w3348, w3351) -> (w3346:cluster{i32, i32})  [unwired: 1 in]
            n1920 = Add(x=w3373, y=w3371) -> (x+y=w3372:i32)
            n1921 = Bundle(w3373, w3374) -> (w3370:cluster{i32, i32})  [unwired: 1 in]
            n1922 = Bundle(w3337, w3338) -> (w3336:cluster{i32, i32})  [unwired: 1 in]
            n1923 = Bundle(w3347, w3351) -> (w3349:cluster{i32, i32})  [unwired: 1 in]
            n1924 = call <vilib>:"Move Pen.vi"("new position"=w3370, "picture"=w3306) -> ("new picture"=w3369:picture)  [unwired: 3 in]
            n1925 = Bundle(w3372, w3374) -> (w3375:cluster{i32, i32})  [unwired: 1 in]
            n1926 = call <vilib>:"Draw Line.vi"("picture"=w3369, "end point"=w3375, "color(black)"=u32 16448250, "pen"=T1 {"Width"=3, "Style"=enum."Solid"}) -> ("new picture"=w3305:picture)  [unwired: 5 in]
            n1927 = Multiply(x=w3302, y=10) -> (x*y=w3318:i32)
            n1928 = Multiply(x=2, y=w3318) -> (x*y=w3319:i32)
            n1929 = Add(x=w3304, y=0) -> (x+y=w3327:i32)
            n1930 = Multiply(x=w3302, y=10) -> (x*y=w3330:i32)
            n1931 = Add(x=w3303, y=w3330) -> (x+y=w3328:i32)
            n1932 = Add(x=w3304, y=0) -> (x+y=w3315:i32)
            n1933 = Add(x=w3303, y=w3319) -> (x+y=w3317:i32)
            n1934 = Add(x=w3304, y=0) -> (x+y=w3361:i32)
            n1935 = Add(x=w3303, y=0) -> (x+y=w3362:i32)
            n1936 = Multiply(x=w3302, y=10) -> (x*y=w3360:i32)
            n1937 = Add(x=w3328, y=w3330) -> (x+y=w3329:i32)
            n1938 = Add(x=w3315, y=w3318) -> (x+y=w3314:i32)
            n1939 = Add(x=w3362, y=w3360) -> (x+y=w3363:i32)
            n1940 = Bundle(w3327, w3328) -> (w3325:cluster{i32, i32})  [unwired: 1 in]
            n1941 = Bundle(w3315, w3317) -> (w3313:cluster{i32, i32})  [unwired: 1 in]
            n1942 = Bundle(w3361, w3362) -> (w3358:cluster{i32, i32})  [unwired: 1 in]
            n1943 = Bundle(w3327, w3329) -> (w3326:cluster{i32, i32})  [unwired: 1 in]
            n1944 = Bundle(w3314, w3317) -> (w3316:cluster{i32, i32})  [unwired: 1 in]
            n1945 = call <vilib>:"Move Pen.vi"("new position"=w3358, "picture"=w3305) -> ("new picture"=w3357:picture)  [unwired: 3 in]
            n1946 = Bundle(w3361, w3363) -> (w3359:cluster{i32, i32})  [unwired: 1 in]
            n1947 = call <vilib>:"Draw Line.vi"("picture"=w3357, "end point"=w3359, "color(black)"=u32 16448250, "pen"=T1 {"Width"=3, "Style"=enum."Solid"}) -> ("new picture"=w3301:picture)  [unwired: 5 in]
            n1948 = call <vilib>:"Move Pen.vi"("new position"=w3346, "picture"=w3301) -> ("new picture"=w3345:picture)  [unwired: 3 in]
            n1949 = call <vilib>:"Draw Line.vi"("picture"=w3345, "end point"=w3349, "color(black)"=u32 16448250, "pen"=T1 {"Width"=3, "Style"=enum."Solid"}) -> ("new picture"=w3300:picture)  [unwired: 5 in]
            n1950 = call <vilib>:"Move Pen.vi"("new position"=w3325, "picture"=w3300) -> ("new picture"=w3324:picture)  [unwired: 3 in]
            n1951 = call <vilib>:"Draw Line.vi"("picture"=w3324, "end point"=w3326, "color(black)"=u32 16448250, "pen"=T1 {"Width"=3, "Style"=enum."Solid"}) -> ("new picture"=w3299:picture)  [unwired: 5 in]
            n1952 = call <vilib>:"Move Pen.vi"("new position"=w3335, "picture"=w3299) -> ("new picture"=w3334:picture)  [unwired: 3 in]
            n1953 = call <vilib>:"Draw Line.vi"("picture"=w3334, "end point"=w3336, "color(black)"=u32 16448250, "pen"=T1 {"Width"=3, "Style"=enum."Solid"}) -> ("new picture"=w3298:picture)  [unwired: 5 in]
            n1954 = call <vilib>:"Move Pen.vi"("new position"=w3313, "picture"=w3298) -> ("new picture"=w3312:picture)  [unwired: 3 in]
            n1955 = call <vilib>:"Draw Line.vi"("picture"=w3312, "end point"=w3316, "color(black)"=u32 16448250, "pen"=T1 {"Width"=3, "Style"=enum."Solid"}) -> ("new picture"=w3297:picture)  [unwired: 5 in]
          }
          frame 7 {
            n1956 = Add(x=w3381, y=0) -> (x+y=w3414:i32)
            n1957 = Add(x=w3380, y=0) -> (x+y=w3415:i32)
            n1958 = Multiply(x=w3379, y=10) -> (x*y=w3413:i32)
            n1959 = Add(x=w3415, y=w3413) -> (x+y=w3416:i32)
            n1960 = Add(x=w3381, y=0) -> (x+y=w3426:i32)
            n1961 = Add(x=w3380, y=0) -> (x+y=w3427:i32)
            n1962 = Bundle(w3414, w3415) -> (w3411:cluster{i32, i32})  [unwired: 1 in]
            n1963 = Multiply(x=w3379, y=10) -> (x*y=w3424:i32)
            n1964 = Add(x=w3426, y=w3424) -> (x+y=w3425:i32)
            n1965 = Bundle(w3426, w3427) -> (w3423:cluster{i32, i32})  [unwired: 1 in]
            n1966 = Bundle(w3414, w3416) -> (w3412:cluster{i32, i32})  [unwired: 1 in]
            n1967 = call <vilib>:"Move Pen.vi"("new position"=w3423, "picture"=w3383) -> ("new picture"=w3422:picture)  [unwired: 3 in]
            n1968 = Bundle(w3425, w3427) -> (w3428:cluster{i32, i32})  [unwired: 1 in]
            n1969 = call <vilib>:"Draw Line.vi"("picture"=w3422, "end point"=w3428, "color(black)"=u32 16448250, "pen"=T1 {"Width"=3, "Style"=enum."Solid"}) -> ("new picture"=w3382:picture)  [unwired: 5 in]
            n1970 = Multiply(x=w3379, y=10) -> (x*y=w3401:i32)
            n1971 = Add(x=w3381, y=w3401) -> (x+y=w3402:i32)
            n1972 = Add(x=w3380, y=0) -> (x+y=w3404:i32)
            n1973 = Multiply(x=w3379, y=10) -> (x*y=w3393:i32)
            n1974 = Add(x=w3381, y=w3393) -> (x+y=w3390:i32)
            n1975 = Add(x=w3380, y=w3393) -> (x+y=w3392:i32)
            n1976 = Add(x=w3404, y=w3401) -> (x+y=w3403:i32)
            n1977 = Bundle(w3402, w3404) -> (w3399:cluster{i32, i32})  [unwired: 1 in]
            n1978 = Add(x=w3392, y=w3393) -> (x+y=w3391:i32)
            n1979 = Bundle(w3390, w3392) -> (w3388:cluster{i32, i32})  [unwired: 1 in]
            n1980 = Bundle(w3402, w3403) -> (w3400:cluster{i32, i32})  [unwired: 1 in]
            n1981 = call <vilib>:"Move Pen.vi"("new position"=w3388, "picture"=w3382) -> ("new picture"=w3387:picture)  [unwired: 3 in]
            n1982 = Bundle(w3390, w3391) -> (w3389:cluster{i32, i32})  [unwired: 1 in]
            n1983 = call <vilib>:"Draw Line.vi"("picture"=w3387, "end point"=w3389, "color(black)"=u32 16448250, "pen"=T1 {"Width"=3, "Style"=enum."Solid"}) -> ("new picture"=w3378:picture)  [unwired: 5 in]
            n1984 = call <vilib>:"Move Pen.vi"("new position"=w3411, "picture"=w3378) -> ("new picture"=w3410:picture)  [unwired: 3 in]
            n1985 = call <vilib>:"Draw Line.vi"("picture"=w3410, "end point"=w3412, "color(black)"=u32 16448250, "pen"=T1 {"Width"=3, "Style"=enum."Solid"}) -> ("new picture"=w3377:picture)  [unwired: 5 in]
            n1986 = call <vilib>:"Move Pen.vi"("new position"=w3399, "picture"=w3377) -> ("new picture"=w3398:picture)  [unwired: 3 in]
            n1987 = call <vilib>:"Draw Line.vi"("picture"=w3398, "end point"=w3400, "color(black)"=u32 16448250, "pen"=T1 {"Width"=3, "Style"=enum."Solid"}) -> ("new picture"=w3376:picture)  [unwired: 5 in]
          }
          frame 8 {
            n1988 = Add(x=w3437, y=0) -> (x+y=w3505:i32)
            n1989 = Add(x=w3436, y=0) -> (x+y=w3506:i32)
            n1990 = Add(x=w3437, y=0) -> (x+y=w3460:i32)
            n1991 = Multiply(x=w3435, y=10) -> (x*y=w3504:i32)
            n1992 = Multiply(x=w3435, y=10) -> (x*y=w3463:i32)
            n1993 = Add(x=w3436, y=w3463) -> (x+y=w3461:i32)
            n1994 = Add(x=w3437, y=0) -> (x+y=w3517:i32)
            n1995 = Add(x=w3436, y=0) -> (x+y=w3518:i32)
            n1996 = Multiply(x=w3435, y=10) -> (x*y=w3515:i32)
            n1997 = Add(x=w3506, y=w3504) -> (x+y=w3507:i32)
            n1998 = Add(x=w3461, y=w3463) -> (x+y=w3462:i32)
            n1999 = Bundle(w3505, w3506) -> (w3502:cluster{i32, i32})  [unwired: 1 in]
            n2000 = Bundle(w3460, w3461) -> (w3458:cluster{i32, i32})  [unwired: 1 in]
            n2001 = Multiply(x=w3435, y=10) -> (x*y=w3451:i32)
            n2002 = Multiply(x=2, y=w3451) -> (x*y=w3452:i32)
            n2003 = Add(x=w3517, y=w3515) -> (x+y=w3516:i32)
            n2004 = Bundle(w3517, w3518) -> (w3514:cluster{i32, i32})  [unwired: 1 in]
            n2005 = Add(x=w3437, y=0) -> (x+y=w3448:i32)
            n2006 = Add(x=w3436, y=w3452) -> (x+y=w3450:i32)
            n2007 = Add(x=w3448, y=w3451) -> (x+y=w3447:i32)
            n2008 = Bundle(w3505, w3507) -> (w3503:cluster{i32, i32})  [unwired: 1 in]
            n2009 = Bundle(w3460, w3462) -> (w3459:cluster{i32, i32})  [unwired: 1 in]
            n2010 = Bundle(w3448, w3450) -> (w3446:cluster{i32, i32})  [unwired: 1 in]
            n2011 = call <vilib>:"Move Pen.vi"("new position"=w3514, "picture"=w3439) -> ("new picture"=w3513:picture)  [unwired: 3 in]
            n2012 = Bundle(w3516, w3518) -> (w3519:cluster{i32, i32})  [unwired: 1 in]
            n2013 = Bundle(w3447, w3450) -> (w3449:cluster{i32, i32})  [unwired: 1 in]
            n2014 = call <vilib>:"Draw Line.vi"("picture"=w3513, "end point"=w3519, "color(black)"=u32 16448250, "pen"=T1 {"Width"=3, "Style"=enum."Solid"}) -> ("new picture"=w3438:picture)  [unwired: 5 in]
            n2015 = Multiply(x=w3435, y=10) -> (x*y=w3483:i32)
            n2016 = Multiply(x=w3435, y=10) -> (x*y=w3492:i32)
            n2017 = Add(x=w3437, y=0) -> (x+y=w3481:i32)
            n2018 = Multiply(x=w3435, y=10) -> (x*y=w3473:i32)
            n2019 = Add(x=w3436, y=w3483) -> (x+y=w3484:i32)
            n2020 = Add(x=w3437, y=w3492) -> (x+y=w3493:i32)
            n2021 = Add(x=w3436, y=0) -> (x+y=w3495:i32)
            n2022 = Add(x=w3437, y=w3473) -> (x+y=w3470:i32)
            n2023 = Add(x=w3436, y=w3473) -> (x+y=w3472:i32)
            n2024 = Add(x=w3481, y=w3483) -> (x+y=w3480:i32)
            n2025 = Bundle(w3481, w3484) -> (w3479:cluster{i32, i32})  [unwired: 1 in]
            n2026 = Add(x=w3495, y=w3492) -> (x+y=w3494:i32)
            n2027 = Add(x=w3472, y=w3473) -> (x+y=w3471:i32)
            n2028 = Bundle(w3493, w3495) -> (w3490:cluster{i32, i32})  [unwired: 1 in]
            n2029 = Bundle(w3470, w3472) -> (w3468:cluster{i32, i32})  [unwired: 1 in]
            n2030 = call <vilib>:"Move Pen.vi"("new position"=w3479, "picture"=w3438) -> ("new picture"=w3478:picture)  [unwired: 3 in]
            n2031 = Bundle(w3480, w3484) -> (w3482:cluster{i32, i32})  [unwired: 1 in]
            n2032 = Bundle(w3493, w3494) -> (w3491:cluster{i32, i32})  [unwired: 1 in]
            n2033 = Bundle(w3470, w3471) -> (w3469:cluster{i32, i32})  [unwired: 1 in]
            n2034 = call <vilib>:"Draw Line.vi"("picture"=w3478, "end point"=w3482, "color(black)"=u32 16448250, "pen"=T1 {"Width"=3, "Style"=enum."Solid"}) -> ("new picture"=w3434:picture)  [unwired: 5 in]
            n2035 = call <vilib>:"Move Pen.vi"("new position"=w3502, "picture"=w3434) -> ("new picture"=w3501:picture)  [unwired: 3 in]
            n2036 = call <vilib>:"Draw Line.vi"("picture"=w3501, "end point"=w3503, "color(black)"=u32 16448250, "pen"=T1 {"Width"=3, "Style"=enum."Solid"}) -> ("new picture"=w3433:picture)  [unwired: 5 in]
            n2037 = call <vilib>:"Move Pen.vi"("new position"=w3490, "picture"=w3433) -> ("new picture"=w3489:picture)  [unwired: 3 in]
            n2038 = call <vilib>:"Draw Line.vi"("picture"=w3489, "end point"=w3491, "color(black)"=u32 16448250, "pen"=T1 {"Width"=3, "Style"=enum."Solid"}) -> ("new picture"=w3432:picture)  [unwired: 5 in]
            n2039 = call <vilib>:"Move Pen.vi"("new position"=w3458, "picture"=w3432) -> ("new picture"=w3457:picture)  [unwired: 3 in]
            n2040 = call <vilib>:"Draw Line.vi"("picture"=w3457, "end point"=w3459, "color(black)"=u32 16448250, "pen"=T1 {"Width"=3, "Style"=enum."Solid"}) -> ("new picture"=w3431:picture)  [unwired: 5 in]
            n2041 = call <vilib>:"Move Pen.vi"("new position"=w3468, "picture"=w3431) -> ("new picture"=w3467:picture)  [unwired: 3 in]
            n2042 = call <vilib>:"Draw Line.vi"("picture"=w3467, "end point"=w3469, "color(black)"=u32 16448250, "pen"=T1 {"Width"=3, "Style"=enum."Solid"}) -> ("new picture"=w3430:picture)  [unwired: 5 in]
            n2043 = call <vilib>:"Move Pen.vi"("new position"=w3446, "picture"=w3430) -> ("new picture"=w3445:picture)  [unwired: 3 in]
            n2044 = call <vilib>:"Draw Line.vi"("picture"=w3445, "end point"=w3449, "color(black)"=u32 16448250, "pen"=T1 {"Width"=3, "Style"=enum."Solid"}) -> ("new picture"=w3429:picture)  [unwired: 5 in]
          }
          frame 9 {
            n2045 = Add(x=w3526, y=0) -> (x+y=w3570:i32)
            n2046 = Add(x=w3525, y=0) -> (x+y=w3571:i32)
            n2047 = Add(x=w3526, y=0) -> (x+y=w3582:i32)
            n2048 = Add(x=w3525, y=0) -> (x+y=w3583:i32)
            n2049 = Multiply(x=w3524, y=10) -> (x*y=w3569:i32)
            n2050 = Multiply(x=w3524, y=10) -> (x*y=w3580:i32)
            n2051 = Add(x=w3571, y=w3569) -> (x+y=w3572:i32)
            n2052 = Add(x=w3582, y=w3580) -> (x+y=w3581:i32)
            n2053 = Bundle(w3570, w3571) -> (w3567:cluster{i32, i32})  [unwired: 1 in]
            n2054 = Bundle(w3582, w3583) -> (w3579:cluster{i32, i32})  [unwired: 1 in]
            n2055 = Bundle(w3570, w3572) -> (w3568:cluster{i32, i32})  [unwired: 1 in]
            n2056 = call <vilib>:"Move Pen.vi"("new position"=w3579, "picture"=w3528) -> ("new picture"=w3578:picture)  [unwired: 3 in]
            n2057 = Bundle(w3581, w3583) -> (w3584:cluster{i32, i32})  [unwired: 1 in]
            n2058 = Multiply(x=w3524, y=10) -> (x*y=w3538:i32)
            n2059 = Add(x=w3526, y=w3538) -> (x+y=w3535:i32)
            n2060 = Add(x=w3525, y=w3538) -> (x+y=w3537:i32)
            n2061 = Add(x=w3537, y=w3538) -> (x+y=w3536:i32)
            n2062 = Bundle(w3535, w3537) -> (w3533:cluster{i32, i32})  [unwired: 1 in]
            n2063 = call <vilib>:"Draw Line.vi"("picture"=w3578, "end point"=w3584, "color(black)"=u32 16448250, "pen"=T1 {"Width"=3, "Style"=enum."Solid"}) -> ("new picture"=w3527:picture)  [unwired: 5 in]
            n2064 = Bundle(w3535, w3536) -> (w3534:cluster{i32, i32})  [unwired: 1 in]
            n2065 = Multiply(x=w3524, y=10) -> (x*y=w3557:i32)
            n2066 = Add(x=w3526, y=w3557) -> (x+y=w3558:i32)
            n2067 = Add(x=w3525, y=0) -> (x+y=w3560:i32)
            n2068 = Multiply(x=w3524, y=10) -> (x*y=w3548:i32)
            n2069 = Add(x=w3526, y=0) -> (x+y=w3546:i32)
            n2070 = Add(x=w3525, y=w3548) -> (x+y=w3549:i32)
            n2071 = Add(x=w3560, y=w3557) -> (x+y=w3559:i32)
            n2072 = Add(x=w3546, y=w3548) -> (x+y=w3545:i32)
            n2073 = Bundle(w3558, w3560) -> (w3555:cluster{i32, i32})  [unwired: 1 in]
            n2074 = Bundle(w3546, w3549) -> (w3544:cluster{i32, i32})  [unwired: 1 in]
            n2075 = Bundle(w3558, w3559) -> (w3556:cluster{i32, i32})  [unwired: 1 in]
            n2076 = call <vilib>:"Move Pen.vi"("new position"=w3544, "picture"=w3527) -> ("new picture"=w3543:picture)  [unwired: 3 in]
            n2077 = Bundle(w3545, w3549) -> (w3547:cluster{i32, i32})  [unwired: 1 in]
            n2078 = call <vilib>:"Draw Line.vi"("picture"=w3543, "end point"=w3547, "color(black)"=u32 16448250, "pen"=T1 {"Width"=3, "Style"=enum."Solid"}) -> ("new picture"=w3523:picture)  [unwired: 5 in]
            n2079 = call <vilib>:"Move Pen.vi"("new position"=w3567, "picture"=w3523) -> ("new picture"=w3566:picture)  [unwired: 3 in]
            n2080 = call <vilib>:"Draw Line.vi"("picture"=w3566, "end point"=w3568, "color(black)"=u32 16448250, "pen"=T1 {"Width"=3, "Style"=enum."Solid"}) -> ("new picture"=w3522:picture)  [unwired: 5 in]
            n2081 = call <vilib>:"Move Pen.vi"("new position"=w3555, "picture"=w3522) -> ("new picture"=w3554:picture)  [unwired: 3 in]
            n2082 = call <vilib>:"Draw Line.vi"("picture"=w3554, "end point"=w3556, "color(black)"=u32 16448250, "pen"=T1 {"Width"=3, "Style"=enum."Solid"}) -> ("new picture"=w3521:picture)  [unwired: 5 in]
            n2083 = call <vilib>:"Move Pen.vi"("new position"=w3533, "picture"=w3521) -> ("new picture"=w3532:picture)  [unwired: 3 in]
            n2084 = call <vilib>:"Draw Line.vi"("picture"=w3532, "end point"=w3534, "color(black)"=u32 16448250, "pen"=T1 {"Width"=3, "Style"=enum."Solid"}) -> ("new picture"=w3520:picture)  [unwired: 5 in]
          }
        }
        n2085 = Equal?(x=3, y=w113) -> (x = y?=w111:bool)
        n2086 = case shown="9" w147 {
          tunnel: 530 -> [w2301 w2375 w2405 w2473 w2538 w2590 w2658 w2735 w2791 w2880]
          tunnel: 10 -> [w2300 w2374 w2404 w2472 w2537 w2589 w2657 w2734 w2790 w2879]
          tunnel: 3 -> [w2299 w2373 w2403 w2471 w2536 w2588 w2656 w2733 w2789 w2878]
          tunnel: w163 -> [w2302 w2377 w2407 w2474 w2539 w2592 w2660 w2737 w2793 w2882]
          tunnel: [w2293 w2372 w2399 w2466 w2532 w2584 w2651 w2730 w2783 w2874] -> w171
          frame 0, Default {
            n2087 = Add(x=w2301, y=0) -> (x+y=w2357:i32)
            n2088 = Add(x=w2300, y=0) -> (x+y=w2358:i32)
            n2089 = Multiply(x=w2299, y=10) -> (x*y=w2356:i32)
            n2090 = Add(x=w2301, y=0) -> (x+y=w2323:i32)
            n2091 = Multiply(x=w2299, y=10) -> (x*y=w2326:i32)
            n2092 = Add(x=w2300, y=w2326) -> (x+y=w2324:i32)
            n2093 = Add(x=w2358, y=w2356) -> (x+y=w2359:i32)
            n2094 = Add(x=w2324, y=w2326) -> (x+y=w2325:i32)
            n2095 = Bundle(w2357, w2358) -> (w2354:cluster{i32, i32})  [unwired: 1 in]
            n2096 = Bundle(w2323, w2324) -> (w2321:cluster{i32, i32})  [unwired: 1 in]
            n2097 = Bundle(w2357, w2359) -> (w2355:cluster{i32, i32})  [unwired: 1 in]
            n2098 = Bundle(w2323, w2325) -> (w2322:cluster{i32, i32})  [unwired: 1 in]
            n2099 = Multiply(x=w2299, y=10) -> (x*y=w2314:i32)
            n2100 = Multiply(x=2, y=w2314) -> (x*y=w2315:i32)
            n2101 = Add(x=w2301, y=0) -> (x+y=w2369:i32)
            n2102 = Add(x=w2300, y=0) -> (x+y=w2370:i32)
            n2103 = Add(x=w2301, y=0) -> (x+y=w2311:i32)
            n2104 = Add(x=w2300, y=w2315) -> (x+y=w2313:i32)
            n2105 = Multiply(x=w2299, y=10) -> (x*y=w2367:i32)
            n2106 = Add(x=w2311, y=w2314) -> (x+y=w2310:i32)
            n2107 = Add(x=w2369, y=w2367) -> (x+y=w2368:i32)
            n2108 = Bundle(w2369, w2370) -> (w2366:cluster{i32, i32})  [unwired: 1 in]
            n2109 = Bundle(w2311, w2313) -> (w2309:cluster{i32, i32})  [unwired: 1 in]
            n2110 = call <vilib>:"Move Pen.vi"("new position"=w2366, "picture"=w2302) -> ("new picture"=w2365:picture)  [unwired: 3 in]
            n2111 = Bundle(w2368, w2370) -> (w2371:cluster{i32, i32})  [unwired: 1 in]
            n2112 = Bundle(w2310, w2313) -> (w2312:cluster{i32, i32})  [unwired: 1 in]
            n2113 = Multiply(x=w2299, y=10) -> (x*y=w2344:i32)
            n2114 = Add(x=w2301, y=w2344) -> (x+y=w2345:i32)
            n2115 = Add(x=w2300, y=0) -> (x+y=w2347:i32)
            n2116 = Multiply(x=w2299, y=10) -> (x*y=w2336:i32)
            n2117 = Add(x=w2301, y=w2336) -> (x+y=w2333:i32)
            n2118 = Add(x=w2300, y=w2336) -> (x+y=w2335:i32)
            n2119 = Add(x=w2347, y=w2344) -> (x+y=w2346:i32)
            n2120 = Bundle(w2345, w2347) -> (w2342:cluster{i32, i32})  [unwired: 1 in]
            n2121 = call <vilib>:"Draw Line.vi"("picture"=w2365, "end point"=w2371, "color(black)"=u32 16448250, "pen"=T1 {"Width"=3, "Style"=enum."Solid"}) -> ("new picture"=w2298:picture)  [unwired: 5 in]
            n2122 = call <vilib>:"Move Pen.vi"("new position"=w2354, "picture"=w2298) -> ("new picture"=w2353:picture)  [unwired: 3 in]
            n2123 = call <vilib>:"Draw Line.vi"("picture"=w2353, "end point"=w2355, "color(black)"=u32 16448250, "pen"=T1 {"Width"=3, "Style"=enum."Solid"}) -> ("new picture"=w2297:picture)  [unwired: 5 in]
            n2124 = Add(x=w2335, y=w2336) -> (x+y=w2334:i32)
            n2125 = Bundle(w2333, w2335) -> (w2331:cluster{i32, i32})  [unwired: 1 in]
            n2126 = call <vilib>:"Move Pen.vi"("new position"=w2342, "picture"=w2297) -> ("new picture"=w2341:picture)  [unwired: 3 in]
            n2127 = Bundle(w2345, w2346) -> (w2343:cluster{i32, i32})  [unwired: 1 in]
            n2128 = Bundle(w2333, w2334) -> (w2332:cluster{i32, i32})  [unwired: 1 in]
            n2129 = call <vilib>:"Draw Line.vi"("picture"=w2341, "end point"=w2343, "color(black)"=u32 16448250, "pen"=T1 {"Width"=3, "Style"=enum."Solid"}) -> ("new picture"=w2296:picture)  [unwired: 5 in]
            n2130 = call <vilib>:"Move Pen.vi"("new position"=w2321, "picture"=w2296) -> ("new picture"=w2320:picture)  [unwired: 3 in]
            n2131 = call <vilib>:"Draw Line.vi"("picture"=w2320, "end point"=w2322, "color(black)"=u32 16448250, "pen"=T1 {"Width"=3, "Style"=enum."Solid"}) -> ("new picture"=w2295:picture)  [unwired: 5 in]
            n2132 = call <vilib>:"Move Pen.vi"("new position"=w2331, "picture"=w2295) -> ("new picture"=w2330:picture)  [unwired: 3 in]
            n2133 = call <vilib>:"Draw Line.vi"("picture"=w2330, "end point"=w2332, "color(black)"=u32 16448250, "pen"=T1 {"Width"=3, "Style"=enum."Solid"}) -> ("new picture"=w2294:picture)  [unwired: 5 in]
            n2134 = call <vilib>:"Move Pen.vi"("new position"=w2309, "picture"=w2294) -> ("new picture"=w2308:picture)  [unwired: 3 in]
            n2135 = call <vilib>:"Draw Line.vi"("picture"=w2308, "end point"=w2312, "color(black)"=u32 16448250, "pen"=T1 {"Width"=3, "Style"=enum."Solid"}) -> ("new picture"=w2293:picture)  [unwired: 5 in]
          }
          frame 1 {
            n2136 = Multiply(x=w2373, y=10) -> (x*y=w2395:i32)
            n2137 = Add(x=w2375, y=w2395) -> (x+y=w2396:i32)
            n2138 = Add(x=w2374, y=0) -> (x+y=w2398:i32)
            n2139 = Add(x=w2398, y=w2395) -> (x+y=w2397:i32)
            n2140 = Bundle(w2396, w2398) -> (w2393:cluster{i32, i32})  [unwired: 1 in]
            n2141 = call <vilib>:"Move Pen.vi"("new position"=w2393, "picture"=w2377) -> ("new picture"=w2392:picture)  [unwired: 3 in]
            n2142 = Bundle(w2396, w2397) -> (w2394:cluster{i32, i32})  [unwired: 1 in]
            n2143 = call <vilib>:"Draw Line.vi"("picture"=w2392, "end point"=w2394, "color(black)"=u32 16448250, "pen"=T1 {"Width"=3, "Style"=enum."Solid"}) -> ("new picture"=w2376:picture)  [unwired: 5 in]
            n2144 = Multiply(x=w2373, y=10) -> (x*y=w2387:i32)
            n2145 = Add(x=w2375, y=w2387) -> (x+y=w2384:i32)
            n2146 = Add(x=w2374, y=w2387) -> (x+y=w2386:i32)
            n2147 = Add(x=w2386, y=w2387) -> (x+y=w2385:i32)
            n2148 = Bundle(w2384, w2386) -> (w2382:cluster{i32, i32})  [unwired: 1 in]
            n2149 = call <vilib>:"Move Pen.vi"("new position"=w2382, "picture"=w2376) -> ("new picture"=w2381:picture)  [unwired: 3 in]
            n2150 = Bundle(w2384, w2385) -> (w2383:cluster{i32, i32})  [unwired: 1 in]
            n2151 = call <vilib>:"Draw Line.vi"("picture"=w2381, "end point"=w2383, "color(black)"=u32 16448250, "pen"=T1 {"Width"=3, "Style"=enum."Solid"}) -> ("new picture"=w2372:picture)  [unwired: 5 in]
          }
          frame 2 {
            n2152 = Multiply(x=w2403, y=10) -> (x*y=w2441:i32)
            n2153 = Add(x=w2405, y=0) -> (x+y=w2439:i32)
            n2154 = Add(x=w2404, y=w2441) -> (x+y=w2442:i32)
            n2155 = Add(x=w2405, y=0) -> (x+y=w2463:i32)
            n2156 = Add(x=w2404, y=0) -> (x+y=w2464:i32)
            n2157 = Multiply(x=w2403, y=10) -> (x*y=w2461:i32)
            n2158 = Add(x=w2439, y=w2441) -> (x+y=w2438:i32)
            n2159 = Add(x=w2463, y=w2461) -> (x+y=w2462:i32)
            n2160 = Bundle(w2439, w2442) -> (w2437:cluster{i32, i32})  [unwired: 1 in]
            n2161 = Bundle(w2463, w2464) -> (w2460:cluster{i32, i32})  [unwired: 1 in]
            n2162 = Bundle(w2438, w2442) -> (w2440:cluster{i32, i32})  [unwired: 1 in]
            n2163 = call <vilib>:"Move Pen.vi"("new position"=w2460, "picture"=w2407) -> ("new picture"=w2459:picture)  [unwired: 3 in]
            n2164 = Bundle(w2462, w2464) -> (w2465:cluster{i32, i32})  [unwired: 1 in]
            n2165 = Multiply(x=w2403, y=10) -> (x*y=w2419:i32)
            n2166 = Multiply(x=2, y=w2419) -> (x*y=w2420:i32)
            n2167 = Add(x=w2405, y=0) -> (x+y=w2416:i32)
            n2168 = Add(x=w2404, y=w2420) -> (x+y=w2418:i32)
            n2169 = Add(x=w2416, y=w2419) -> (x+y=w2415:i32)
            n2170 = Bundle(w2416, w2418) -> (w2414:cluster{i32, i32})  [unwired: 1 in]
            n2171 = call <vilib>:"Draw Line.vi"("picture"=w2459, "end point"=w2465, "color(black)"=u32 16448250, "pen"=T1 {"Width"=3, "Style"=enum."Solid"}) -> ("new picture"=w2406:picture)  [unwired: 5 in]
            n2172 = Bundle(w2415, w2418) -> (w2417:cluster{i32, i32})  [unwired: 1 in]
            n2173 = Multiply(x=w2403, y=10) -> (x*y=w2450:i32)
            n2174 = Add(x=w2405, y=0) -> (x+y=w2428:i32)
            n2175 = Add(x=w2405, y=w2450) -> (x+y=w2451:i32)
            n2176 = Add(x=w2404, y=0) -> (x+y=w2453:i32)
            n2177 = Multiply(x=w2403, y=10) -> (x*y=w2431:i32)
            n2178 = Add(x=w2404, y=w2431) -> (x+y=w2429:i32)
            n2179 = Add(x=w2429, y=w2431) -> (x+y=w2430:i32)
            n2180 = Add(x=w2453, y=w2450) -> (x+y=w2452:i32)
            n2181 = Bundle(w2428, w2429) -> (w2426:cluster{i32, i32})  [unwired: 1 in]
            n2182 = Bundle(w2451, w2453) -> (w2448:cluster{i32, i32})  [unwired: 1 in]
            n2183 = call <vilib>:"Move Pen.vi"("new position"=w2448, "picture"=w2406) -> ("new picture"=w2447:picture)  [unwired: 3 in]
            n2184 = Bundle(w2428, w2430) -> (w2427:cluster{i32, i32})  [unwired: 1 in]
            n2185 = Bundle(w2451, w2452) -> (w2449:cluster{i32, i32})  [unwired: 1 in]
            n2186 = call <vilib>:"Draw Line.vi"("picture"=w2447, "end point"=w2449, "color(black)"=u32 16448250, "pen"=T1 {"Width"=3, "Style"=enum."Solid"}) -> ("new picture"=w2402:picture)  [unwired: 5 in]
            n2187 = call <vilib>:"Move Pen.vi"("new position"=w2437, "picture"=w2402) -> ("new picture"=w2436:picture)  [unwired: 3 in]
            n2188 = call <vilib>:"Draw Line.vi"("picture"=w2436, "end point"=w2440, "color(black)"=u32 16448250, "pen"=T1 {"Width"=3, "Style"=enum."Solid"}) -> ("new picture"=w2401:picture)  [unwired: 5 in]
            n2189 = call <vilib>:"Move Pen.vi"("new position"=w2426, "picture"=w2401) -> ("new picture"=w2425:picture)  [unwired: 3 in]
            n2190 = call <vilib>:"Draw Line.vi"("picture"=w2425, "end point"=w2427, "color(black)"=u32 16448250, "pen"=T1 {"Width"=3, "Style"=enum."Solid"}) -> ("new picture"=w2400:picture)  [unwired: 5 in]
            n2191 = call <vilib>:"Move Pen.vi"("new position"=w2414, "picture"=w2400) -> ("new picture"=w2413:picture)  [unwired: 3 in]
            n2192 = call <vilib>:"Draw Line.vi"("picture"=w2413, "end point"=w2417, "color(black)"=u32 16448250, "pen"=T1 {"Width"=3, "Style"=enum."Solid"}) -> ("new picture"=w2399:picture)  [unwired: 5 in]
          }
          frame 3 {
            n2193 = Multiply(x=w2471, y=10) -> (x*y=w2507:i32)
            n2194 = Add(x=w2473, y=0) -> (x+y=w2505:i32)
            n2195 = Add(x=w2472, y=w2507) -> (x+y=w2508:i32)
            n2196 = Add(x=w2473, y=0) -> (x+y=w2529:i32)
            n2197 = Add(x=w2472, y=0) -> (x+y=w2530:i32)
            n2198 = Multiply(x=w2471, y=10) -> (x*y=w2527:i32)
            n2199 = Add(x=w2505, y=w2507) -> (x+y=w2504:i32)
            n2200 = Add(x=w2529, y=w2527) -> (x+y=w2528:i32)
            n2201 = Bundle(w2505, w2508) -> (w2503:cluster{i32, i32})  [unwired: 1 in]
            n2202 = Bundle(w2529, w2530) -> (w2526:cluster{i32, i32})  [unwired: 1 in]
            n2203 = call <vilib>:"Move Pen.vi"("new position"=w2526, "picture"=w2474) -> ("new picture"=w2525:picture)  [unwired: 3 in]
            n2204 = Bundle(w2504, w2508) -> (w2506:cluster{i32, i32})  [unwired: 1 in]
            n2205 = Bundle(w2528, w2530) -> (w2531:cluster{i32, i32})  [unwired: 1 in]
            n2206 = Multiply(x=w2471, y=10) -> (x*y=w2486:i32)
            n2207 = Multiply(x=2, y=w2486) -> (x*y=w2487:i32)
            n2208 = Add(x=w2473, y=0) -> (x+y=w2483:i32)
            n2209 = Add(x=w2472, y=w2487) -> (x+y=w2485:i32)
            n2210 = Add(x=w2483, y=w2486) -> (x+y=w2482:i32)
            n2211 = call <vilib>:"Draw Line.vi"("picture"=w2525, "end point"=w2531, "color(black)"=u32 16448250, "pen"=T1 {"Width"=3, "Style"=enum."Solid"}) -> ("new picture"=w2470:picture)  [unwired: 5 in]
            n2212 = Bundle(w2483, w2485) -> (w2481:cluster{i32, i32})  [unwired: 1 in]
            n2213 = Bundle(w2482, w2485) -> (w2484:cluster{i32, i32})  [unwired: 1 in]
            n2214 = Multiply(x=w2471, y=10) -> (x*y=w2497:i32)
            n2215 = Add(x=w2473, y=w2497) -> (x+y=w2494:i32)
            n2216 = Add(x=w2472, y=w2497) -> (x+y=w2496:i32)
            n2217 = Multiply(x=w2471, y=10) -> (x*y=w2516:i32)
            n2218 = Add(x=w2473, y=w2516) -> (x+y=w2517:i32)
            n2219 = Add(x=w2472, y=0) -> (x+y=w2519:i32)
            n2220 = Add(x=w2496, y=w2497) -> (x+y=w2495:i32)
            n2221 = Bundle(w2494, w2496) -> (w2492:cluster{i32, i32})  [unwired: 1 in]
            n2222 = Add(x=w2519, y=w2516) -> (x+y=w2518:i32)
            n2223 = Bundle(w2517, w2519) -> (w2514:cluster{i32, i32})  [unwired: 1 in]
            n2224 = Bundle(w2494, w2495) -> (w2493:cluster{i32, i32})  [unwired: 1 in]
            n2225 = call <vilib>:"Move Pen.vi"("new position"=w2514, "picture"=w2470) -> ("new picture"=w2513:picture)  [unwired: 3 in]
            n2226 = Bundle(w2517, w2518) -> (w2515:cluster{i32, i32})  [unwired: 1 in]
            n2227 = call <vilib>:"Draw Line.vi"("picture"=w2513, "end point"=w2515, "color(black)"=u32 16448250, "pen"=T1 {"Width"=3, "Style"=enum."Solid"}) -> ("new picture"=w2469:picture)  [unwired: 5 in]
            n2228 = call <vilib>:"Move Pen.vi"("new position"=w2503, "picture"=w2469) -> ("new picture"=w2502:picture)  [unwired: 3 in]
            n2229 = call <vilib>:"Draw Line.vi"("picture"=w2502, "end point"=w2506, "color(black)"=u32 16448250, "pen"=T1 {"Width"=3, "Style"=enum."Solid"}) -> ("new picture"=w2468:picture)  [unwired: 5 in]
            n2230 = call <vilib>:"Move Pen.vi"("new position"=w2492, "picture"=w2468) -> ("new picture"=w2491:picture)  [unwired: 3 in]
            n2231 = call <vilib>:"Draw Line.vi"("picture"=w2491, "end point"=w2493, "color(black)"=u32 16448250, "pen"=T1 {"Width"=3, "Style"=enum."Solid"}) -> ("new picture"=w2467:picture)  [unwired: 5 in]
            n2232 = call <vilib>:"Move Pen.vi"("new position"=w2481, "picture"=w2467) -> ("new picture"=w2480:picture)  [unwired: 3 in]
            n2233 = call <vilib>:"Draw Line.vi"("picture"=w2480, "end point"=w2484, "color(black)"=u32 16448250, "pen"=T1 {"Width"=3, "Style"=enum."Solid"}) -> ("new picture"=w2466:picture)  [unwired: 5 in]
          }
          frame 4 {
            n2234 = Add(x=w2538, y=0) -> (x+y=w2581:i32)
            n2235 = Add(x=w2537, y=0) -> (x+y=w2582:i32)
            n2236 = Multiply(x=w2536, y=10) -> (x*y=w2580:i32)
            n2237 = Add(x=w2582, y=w2580) -> (x+y=w2583:i32)
            n2238 = Bundle(w2581, w2582) -> (w2578:cluster{i32, i32})  [unwired: 1 in]
            n2239 = call <vilib>:"Move Pen.vi"("new position"=w2578, "picture"=w2539) -> ("new picture"=w2577:picture)  [unwired: 3 in]
            n2240 = Bundle(w2581, w2583) -> (w2579:cluster{i32, i32})  [unwired: 1 in]
            n2241 = Multiply(x=w2536, y=10) -> (x*y=w2559:i32)
            n2242 = Add(x=w2538, y=0) -> (x+y=w2557:i32)
            n2243 = Add(x=w2537, y=w2559) -> (x+y=w2560:i32)
            n2244 = Add(x=w2557, y=w2559) -> (x+y=w2556:i32)
            n2245 = Bundle(w2557, w2560) -> (w2555:cluster{i32, i32})  [unwired: 1 in]
            n2246 = call <vilib>:"Draw Line.vi"("picture"=w2577, "end point"=w2579, "color(black)"=u32 16448250, "pen"=T1 {"Width"=3, "Style"=enum."Solid"}) -> ("new picture"=w2533:picture)  [unwired: 5 in]
            n2247 = Multiply(x=w2536, y=10) -> (x*y=w2549:i32)
            n2248 = Add(x=w2538, y=w2549) -> (x+y=w2546:i32)
            n2249 = Add(x=w2537, y=w2549) -> (x+y=w2548:i32)
            n2250 = Bundle(w2556, w2560) -> (w2558:cluster{i32, i32})  [unwired: 1 in]
            n2251 = Add(x=w2548, y=w2549) -> (x+y=w2547:i32)
            n2252 = Bundle(w2546, w2548) -> (w2544:cluster{i32, i32})  [unwired: 1 in]
            n2253 = Multiply(x=w2536, y=10) -> (x*y=w2568:i32)
            n2254 = Add(x=w2538, y=w2568) -> (x+y=w2569:i32)
            n2255 = Add(x=w2537, y=0) -> (x+y=w2571:i32)
            n2256 = Add(x=w2571, y=w2568) -> (x+y=w2570:i32)
            n2257 = Bundle(w2546, w2547) -> (w2545:cluster{i32, i32})  [unwired: 1 in]
            n2258 = Bundle(w2569, w2571) -> (w2566:cluster{i32, i32})  [unwired: 1 in]
            n2259 = call <vilib>:"Move Pen.vi"("new position"=w2566, "picture"=w2533) -> ("new picture"=w2565:picture)  [unwired: 3 in]
            n2260 = Bundle(w2569, w2570) -> (w2567:cluster{i32, i32})  [unwired: 1 in]
            n2261 = call <vilib>:"Draw Line.vi"("picture"=w2565, "end point"=w2567, "color(black)"=u32 16448250, "pen"=T1 {"Width"=3, "Style"=enum."Solid"}) -> ("new picture"=w2535:picture)  [unwired: 5 in]
            n2262 = call <vilib>:"Move Pen.vi"("new position"=w2555, "picture"=w2535) -> ("new picture"=w2554:picture)  [unwired: 3 in]
            n2263 = call <vilib>:"Draw Line.vi"("picture"=w2554, "end point"=w2558, "color(black)"=u32 16448250, "pen"=T1 {"Width"=3, "Style"=enum."Solid"}) -> ("new picture"=w2534:picture)  [unwired: 5 in]
            n2264 = call <vilib>:"Move Pen.vi"("new position"=w2544, "picture"=w2534) -> ("new picture"=w2543:picture)  [unwired: 3 in]
            n2265 = call <vilib>:"Draw Line.vi"("picture"=w2543, "end point"=w2545, "color(black)"=u32 16448250, "pen"=T1 {"Width"=3, "Style"=enum."Solid"}) -> ("new picture"=w2532:picture)  [unwired: 5 in]
          }
          frame 5 {
            n2266 = Multiply(x=w2588, y=10) -> (x*y=w2625:i32)
            n2267 = Add(x=w2590, y=0) -> (x+y=w2623:i32)
            n2268 = Add(x=w2589, y=w2625) -> (x+y=w2626:i32)
            n2269 = Add(x=w2590, y=0) -> (x+y=w2648:i32)
            n2270 = Add(x=w2589, y=0) -> (x+y=w2649:i32)
            n2271 = Add(x=w2623, y=w2625) -> (x+y=w2622:i32)
            n2272 = Multiply(x=w2588, y=10) -> (x*y=w2646:i32)
            n2273 = Bundle(w2623, w2626) -> (w2621:cluster{i32, i32})  [unwired: 1 in]
            n2274 = Add(x=w2648, y=w2646) -> (x+y=w2647:i32)
            n2275 = Bundle(w2648, w2649) -> (w2645:cluster{i32, i32})  [unwired: 1 in]
            n2276 = Bundle(w2622, w2626) -> (w2624:cluster{i32, i32})  [unwired: 1 in]
            n2277 = call <vilib>:"Move Pen.vi"("new position"=w2645, "picture"=w2592) -> ("new picture"=w2644:picture)  [unwired: 3 in]
            n2278 = Bundle(w2647, w2649) -> (w2650:cluster{i32, i32})  [unwired: 1 in]
            n2279 = Multiply(x=w2588, y=10) -> (x*y=w2604:i32)
            n2280 = Multiply(x=2, y=w2604) -> (x*y=w2605:i32)
            n2281 = Add(x=w2590, y=0) -> (x+y=w2601:i32)
            n2282 = Add(x=w2589, y=w2605) -> (x+y=w2603:i32)
            n2283 = Add(x=w2601, y=w2604) -> (x+y=w2600:i32)
            n2284 = Bundle(w2601, w2603) -> (w2599:cluster{i32, i32})  [unwired: 1 in]
            n2285 = call <vilib>:"Draw Line.vi"("picture"=w2644, "end point"=w2650, "color(black)"=u32 16448250, "pen"=T1 {"Width"=3, "Style"=enum."Solid"}) -> ("new picture"=w2591:picture)  [unwired: 5 in]
            n2286 = Bundle(w2600, w2603) -> (w2602:cluster{i32, i32})  [unwired: 1 in]
            n2287 = Multiply(x=w2588, y=10) -> (x*y=w2615:i32)
            n2288 = Add(x=w2590, y=0) -> (x+y=w2636:i32)
            n2289 = Add(x=w2589, y=0) -> (x+y=w2637:i32)
            n2290 = Add(x=w2590, y=w2615) -> (x+y=w2612:i32)
            n2291 = Add(x=w2589, y=w2615) -> (x+y=w2614:i32)
            n2292 = Multiply(x=w2588, y=10) -> (x*y=w2635:i32)
            n2293 = Add(x=w2637, y=w2635) -> (x+y=w2638:i32)
            n2294 = Add(x=w2614, y=w2615) -> (x+y=w2613:i32)
            n2295 = Bundle(w2636, w2637) -> (w2633:cluster{i32, i32})  [unwired: 1 in]
            n2296 = Bundle(w2612, w2614) -> (w2610:cluster{i32, i32})  [unwired: 1 in]
            n2297 = call <vilib>:"Move Pen.vi"("new position"=w2633, "picture"=w2591) -> ("new picture"=w2632:picture)  [unwired: 3 in]
            n2298 = Bundle(w2636, w2638) -> (w2634:cluster{i32, i32})  [unwired: 1 in]
            n2299 = Bundle(w2612, w2613) -> (w2611:cluster{i32, i32})  [unwired: 1 in]
            n2300 = call <vilib>:"Draw Line.vi"("picture"=w2632, "end point"=w2634, "color(black)"=u32 16448250, "pen"=T1 {"Width"=3, "Style"=enum."Solid"}) -> ("new picture"=w2587:picture)  [unwired: 5 in]
            n2301 = call <vilib>:"Move Pen.vi"("new position"=w2621, "picture"=w2587) -> ("new picture"=w2620:picture)  [unwired: 3 in]
            n2302 = call <vilib>:"Draw Line.vi"("picture"=w2620, "end point"=w2624, "color(black)"=u32 16448250, "pen"=T1 {"Width"=3, "Style"=enum."Solid"}) -> ("new picture"=w2586:picture)  [unwired: 5 in]
            n2303 = call <vilib>:"Move Pen.vi"("new position"=w2610, "picture"=w2586) -> ("new picture"=w2609:picture)  [unwired: 3 in]
            n2304 = call <vilib>:"Draw Line.vi"("picture"=w2609, "end point"=w2611, "color(black)"=u32 16448250, "pen"=T1 {"Width"=3, "Style"=enum."Solid"}) -> ("new picture"=w2585:picture)  [unwired: 5 in]
            n2305 = call <vilib>:"Move Pen.vi"("new position"=w2599, "picture"=w2585) -> ("new picture"=w2598:picture)  [unwired: 3 in]
            n2306 = call <vilib>:"Draw Line.vi"("picture"=w2598, "end point"=w2602, "color(black)"=u32 16448250, "pen"=T1 {"Width"=3, "Style"=enum."Solid"}) -> ("new picture"=w2584:picture)  [unwired: 5 in]
          }
          frame 6 {
            n2307 = Multiply(x=w2656, y=10) -> (x*y=w2694:i32)
            n2308 = Multiply(x=w2656, y=10) -> (x*y=w2704:i32)
            n2309 = Add(x=w2658, y=w2694) -> (x+y=w2691:i32)
            n2310 = Add(x=w2657, y=w2694) -> (x+y=w2693:i32)
            n2311 = Add(x=w2658, y=0) -> (x+y=w2702:i32)
            n2312 = Add(x=w2657, y=w2704) -> (x+y=w2705:i32)
            n2313 = Add(x=w2658, y=0) -> (x+y=w2727:i32)
            n2314 = Add(x=w2657, y=0) -> (x+y=w2728:i32)
            n2315 = Multiply(x=w2656, y=10) -> (x*y=w2725:i32)
            n2316 = Add(x=w2702, y=w2704) -> (x+y=w2701:i32)
            n2317 = Add(x=w2693, y=w2694) -> (x+y=w2692:i32)
            n2318 = Bundle(w2691, w2693) -> (w2689:cluster{i32, i32})  [unwired: 1 in]
            n2319 = Bundle(w2702, w2705) -> (w2700:cluster{i32, i32})  [unwired: 1 in]
            n2320 = Add(x=w2727, y=w2725) -> (x+y=w2726:i32)
            n2321 = Bundle(w2727, w2728) -> (w2724:cluster{i32, i32})  [unwired: 1 in]
            n2322 = Bundle(w2691, w2692) -> (w2690:cluster{i32, i32})  [unwired: 1 in]
            n2323 = Bundle(w2701, w2705) -> (w2703:cluster{i32, i32})  [unwired: 1 in]
            n2324 = call <vilib>:"Move Pen.vi"("new position"=w2724, "picture"=w2660) -> ("new picture"=w2723:picture)  [unwired: 3 in]
            n2325 = Bundle(w2726, w2728) -> (w2729:cluster{i32, i32})  [unwired: 1 in]
            n2326 = call <vilib>:"Draw Line.vi"("picture"=w2723, "end point"=w2729, "color(black)"=u32 16448250, "pen"=T1 {"Width"=3, "Style"=enum."Solid"}) -> ("new picture"=w2659:picture)  [unwired: 5 in]
            n2327 = Multiply(x=w2656, y=10) -> (x*y=w2672:i32)
            n2328 = Multiply(x=2, y=w2672) -> (x*y=w2673:i32)
            n2329 = Add(x=w2658, y=0) -> (x+y=w2681:i32)
            n2330 = Multiply(x=w2656, y=10) -> (x*y=w2684:i32)
            n2331 = Add(x=w2657, y=w2684) -> (x+y=w2682:i32)
            n2332 = Add(x=w2658, y=0) -> (x+y=w2669:i32)
            n2333 = Add(x=w2657, y=w2673) -> (x+y=w2671:i32)
            n2334 = Add(x=w2658, y=0) -> (x+y=w2715:i32)
            n2335 = Add(x=w2657, y=0) -> (x+y=w2716:i32)
            n2336 = Multiply(x=w2656, y=10) -> (x*y=w2714:i32)
            n2337 = Add(x=w2682, y=w2684) -> (x+y=w2683:i32)
            n2338 = Add(x=w2669, y=w2672) -> (x+y=w2668:i32)
            n2339 = Add(x=w2716, y=w2714) -> (x+y=w2717:i32)
            n2340 = Bundle(w2681, w2682) -> (w2679:cluster{i32, i32})  [unwired: 1 in]
            n2341 = Bundle(w2669, w2671) -> (w2667:cluster{i32, i32})  [unwired: 1 in]
            n2342 = Bundle(w2715, w2716) -> (w2712:cluster{i32, i32})  [unwired: 1 in]
            n2343 = Bundle(w2681, w2683) -> (w2680:cluster{i32, i32})  [unwired: 1 in]
            n2344 = Bundle(w2668, w2671) -> (w2670:cluster{i32, i32})  [unwired: 1 in]
            n2345 = call <vilib>:"Move Pen.vi"("new position"=w2712, "picture"=w2659) -> ("new picture"=w2711:picture)  [unwired: 3 in]
            n2346 = Bundle(w2715, w2717) -> (w2713:cluster{i32, i32})  [unwired: 1 in]
            n2347 = call <vilib>:"Draw Line.vi"("picture"=w2711, "end point"=w2713, "color(black)"=u32 16448250, "pen"=T1 {"Width"=3, "Style"=enum."Solid"}) -> ("new picture"=w2655:picture)  [unwired: 5 in]
            n2348 = call <vilib>:"Move Pen.vi"("new position"=w2700, "picture"=w2655) -> ("new picture"=w2699:picture)  [unwired: 3 in]
            n2349 = call <vilib>:"Draw Line.vi"("picture"=w2699, "end point"=w2703, "color(black)"=u32 16448250, "pen"=T1 {"Width"=3, "Style"=enum."Solid"}) -> ("new picture"=w2654:picture)  [unwired: 5 in]
            n2350 = call <vilib>:"Move Pen.vi"("new position"=w2679, "picture"=w2654) -> ("new picture"=w2678:picture)  [unwired: 3 in]
            n2351 = call <vilib>:"Draw Line.vi"("picture"=w2678, "end point"=w2680, "color(black)"=u32 16448250, "pen"=T1 {"Width"=3, "Style"=enum."Solid"}) -> ("new picture"=w2653:picture)  [unwired: 5 in]
            n2352 = call <vilib>:"Move Pen.vi"("new position"=w2689, "picture"=w2653) -> ("new picture"=w2688:picture)  [unwired: 3 in]
            n2353 = call <vilib>:"Draw Line.vi"("picture"=w2688, "end point"=w2690, "color(black)"=u32 16448250, "pen"=T1 {"Width"=3, "Style"=enum."Solid"}) -> ("new picture"=w2652:picture)  [unwired: 5 in]
            n2354 = call <vilib>:"Move Pen.vi"("new position"=w2667, "picture"=w2652) -> ("new picture"=w2666:picture)  [unwired: 3 in]
            n2355 = call <vilib>:"Draw Line.vi"("picture"=w2666, "end point"=w2670, "color(black)"=u32 16448250, "pen"=T1 {"Width"=3, "Style"=enum."Solid"}) -> ("new picture"=w2651:picture)  [unwired: 5 in]
          }
          frame 7 {
            n2356 = Add(x=w2735, y=0) -> (x+y=w2768:i32)
            n2357 = Add(x=w2734, y=0) -> (x+y=w2769:i32)
            n2358 = Multiply(x=w2733, y=10) -> (x*y=w2767:i32)
            n2359 = Add(x=w2769, y=w2767) -> (x+y=w2770:i32)
            n2360 = Add(x=w2735, y=0) -> (x+y=w2780:i32)
            n2361 = Add(x=w2734, y=0) -> (x+y=w2781:i32)
            n2362 = Bundle(w2768, w2769) -> (w2765:cluster{i32, i32})  [unwired: 1 in]
            n2363 = Multiply(x=w2733, y=10) -> (x*y=w2778:i32)
            n2364 = Add(x=w2780, y=w2778) -> (x+y=w2779:i32)
            n2365 = Bundle(w2780, w2781) -> (w2777:cluster{i32, i32})  [unwired: 1 in]
            n2366 = Bundle(w2768, w2770) -> (w2766:cluster{i32, i32})  [unwired: 1 in]
            n2367 = call <vilib>:"Move Pen.vi"("new position"=w2777, "picture"=w2737) -> ("new picture"=w2776:picture)  [unwired: 3 in]
            n2368 = Bundle(w2779, w2781) -> (w2782:cluster{i32, i32})  [unwired: 1 in]
            n2369 = call <vilib>:"Draw Line.vi"("picture"=w2776, "end point"=w2782, "color(black)"=u32 16448250, "pen"=T1 {"Width"=3, "Style"=enum."Solid"}) -> ("new picture"=w2736:picture)  [unwired: 5 in]
            n2370 = Multiply(x=w2733, y=10) -> (x*y=w2755:i32)
            n2371 = Add(x=w2735, y=w2755) -> (x+y=w2756:i32)
            n2372 = Add(x=w2734, y=0) -> (x+y=w2758:i32)
            n2373 = Multiply(x=w2733, y=10) -> (x*y=w2747:i32)
            n2374 = Add(x=w2735, y=w2747) -> (x+y=w2744:i32)
            n2375 = Add(x=w2734, y=w2747) -> (x+y=w2746:i32)
            n2376 = Add(x=w2758, y=w2755) -> (x+y=w2757:i32)
            n2377 = Bundle(w2756, w2758) -> (w2753:cluster{i32, i32})  [unwired: 1 in]
            n2378 = Add(x=w2746, y=w2747) -> (x+y=w2745:i32)
            n2379 = Bundle(w2744, w2746) -> (w2742:cluster{i32, i32})  [unwired: 1 in]
            n2380 = Bundle(w2756, w2757) -> (w2754:cluster{i32, i32})  [unwired: 1 in]
            n2381 = call <vilib>:"Move Pen.vi"("new position"=w2742, "picture"=w2736) -> ("new picture"=w2741:picture)  [unwired: 3 in]
            n2382 = Bundle(w2744, w2745) -> (w2743:cluster{i32, i32})  [unwired: 1 in]
            n2383 = call <vilib>:"Draw Line.vi"("picture"=w2741, "end point"=w2743, "color(black)"=u32 16448250, "pen"=T1 {"Width"=3, "Style"=enum."Solid"}) -> ("new picture"=w2732:picture)  [unwired: 5 in]
            n2384 = call <vilib>:"Move Pen.vi"("new position"=w2765, "picture"=w2732) -> ("new picture"=w2764:picture)  [unwired: 3 in]
            n2385 = call <vilib>:"Draw Line.vi"("picture"=w2764, "end point"=w2766, "color(black)"=u32 16448250, "pen"=T1 {"Width"=3, "Style"=enum."Solid"}) -> ("new picture"=w2731:picture)  [unwired: 5 in]
            n2386 = call <vilib>:"Move Pen.vi"("new position"=w2753, "picture"=w2731) -> ("new picture"=w2752:picture)  [unwired: 3 in]
            n2387 = call <vilib>:"Draw Line.vi"("picture"=w2752, "end point"=w2754, "color(black)"=u32 16448250, "pen"=T1 {"Width"=3, "Style"=enum."Solid"}) -> ("new picture"=w2730:picture)  [unwired: 5 in]
          }
          frame 8 {
            n2388 = Add(x=w2791, y=0) -> (x+y=w2859:i32)
            n2389 = Add(x=w2790, y=0) -> (x+y=w2860:i32)
            n2390 = Add(x=w2791, y=0) -> (x+y=w2814:i32)
            n2391 = Multiply(x=w2789, y=10) -> (x*y=w2858:i32)
            n2392 = Multiply(x=w2789, y=10) -> (x*y=w2817:i32)
            n2393 = Add(x=w2790, y=w2817) -> (x+y=w2815:i32)
            n2394 = Add(x=w2791, y=0) -> (x+y=w2871:i32)
            n2395 = Add(x=w2790, y=0) -> (x+y=w2872:i32)
            n2396 = Multiply(x=w2789, y=10) -> (x*y=w2869:i32)
            n2397 = Add(x=w2860, y=w2858) -> (x+y=w2861:i32)
            n2398 = Add(x=w2815, y=w2817) -> (x+y=w2816:i32)
            n2399 = Bundle(w2859, w2860) -> (w2856:cluster{i32, i32})  [unwired: 1 in]
            n2400 = Bundle(w2814, w2815) -> (w2812:cluster{i32, i32})  [unwired: 1 in]
            n2401 = Multiply(x=w2789, y=10) -> (x*y=w2805:i32)
            n2402 = Multiply(x=2, y=w2805) -> (x*y=w2806:i32)
            n2403 = Add(x=w2871, y=w2869) -> (x+y=w2870:i32)
            n2404 = Bundle(w2871, w2872) -> (w2868:cluster{i32, i32})  [unwired: 1 in]
            n2405 = Add(x=w2791, y=0) -> (x+y=w2802:i32)
            n2406 = Add(x=w2790, y=w2806) -> (x+y=w2804:i32)
            n2407 = Add(x=w2802, y=w2805) -> (x+y=w2801:i32)
            n2408 = Bundle(w2859, w2861) -> (w2857:cluster{i32, i32})  [unwired: 1 in]
            n2409 = Bundle(w2814, w2816) -> (w2813:cluster{i32, i32})  [unwired: 1 in]
            n2410 = Bundle(w2802, w2804) -> (w2800:cluster{i32, i32})  [unwired: 1 in]
            n2411 = call <vilib>:"Move Pen.vi"("new position"=w2868, "picture"=w2793) -> ("new picture"=w2867:picture)  [unwired: 3 in]
            n2412 = Bundle(w2870, w2872) -> (w2873:cluster{i32, i32})  [unwired: 1 in]
            n2413 = Bundle(w2801, w2804) -> (w2803:cluster{i32, i32})  [unwired: 1 in]
            n2414 = call <vilib>:"Draw Line.vi"("picture"=w2867, "end point"=w2873, "color(black)"=u32 16448250, "pen"=T1 {"Width"=3, "Style"=enum."Solid"}) -> ("new picture"=w2792:picture)  [unwired: 5 in]
            n2415 = Multiply(x=w2789, y=10) -> (x*y=w2837:i32)
            n2416 = Multiply(x=w2789, y=10) -> (x*y=w2846:i32)
            n2417 = Add(x=w2791, y=0) -> (x+y=w2835:i32)
            n2418 = Multiply(x=w2789, y=10) -> (x*y=w2827:i32)
            n2419 = Add(x=w2790, y=w2837) -> (x+y=w2838:i32)
            n2420 = Add(x=w2791, y=w2846) -> (x+y=w2847:i32)
            n2421 = Add(x=w2790, y=0) -> (x+y=w2849:i32)
            n2422 = Add(x=w2791, y=w2827) -> (x+y=w2824:i32)
            n2423 = Add(x=w2790, y=w2827) -> (x+y=w2826:i32)
            n2424 = Add(x=w2835, y=w2837) -> (x+y=w2834:i32)
            n2425 = Bundle(w2835, w2838) -> (w2833:cluster{i32, i32})  [unwired: 1 in]
            n2426 = Add(x=w2849, y=w2846) -> (x+y=w2848:i32)
            n2427 = Add(x=w2826, y=w2827) -> (x+y=w2825:i32)
            n2428 = Bundle(w2847, w2849) -> (w2844:cluster{i32, i32})  [unwired: 1 in]
            n2429 = Bundle(w2824, w2826) -> (w2822:cluster{i32, i32})  [unwired: 1 in]
            n2430 = call <vilib>:"Move Pen.vi"("new position"=w2833, "picture"=w2792) -> ("new picture"=w2832:picture)  [unwired: 3 in]
            n2431 = Bundle(w2834, w2838) -> (w2836:cluster{i32, i32})  [unwired: 1 in]
            n2432 = Bundle(w2847, w2848) -> (w2845:cluster{i32, i32})  [unwired: 1 in]
            n2433 = Bundle(w2824, w2825) -> (w2823:cluster{i32, i32})  [unwired: 1 in]
            n2434 = call <vilib>:"Draw Line.vi"("picture"=w2832, "end point"=w2836, "color(black)"=u32 16448250, "pen"=T1 {"Width"=3, "Style"=enum."Solid"}) -> ("new picture"=w2788:picture)  [unwired: 5 in]
            n2435 = call <vilib>:"Move Pen.vi"("new position"=w2856, "picture"=w2788) -> ("new picture"=w2855:picture)  [unwired: 3 in]
            n2436 = call <vilib>:"Draw Line.vi"("picture"=w2855, "end point"=w2857, "color(black)"=u32 16448250, "pen"=T1 {"Width"=3, "Style"=enum."Solid"}) -> ("new picture"=w2787:picture)  [unwired: 5 in]
            n2437 = call <vilib>:"Move Pen.vi"("new position"=w2844, "picture"=w2787) -> ("new picture"=w2843:picture)  [unwired: 3 in]
            n2438 = call <vilib>:"Draw Line.vi"("picture"=w2843, "end point"=w2845, "color(black)"=u32 16448250, "pen"=T1 {"Width"=3, "Style"=enum."Solid"}) -> ("new picture"=w2786:picture)  [unwired: 5 in]
            n2439 = call <vilib>:"Move Pen.vi"("new position"=w2812, "picture"=w2786) -> ("new picture"=w2811:picture)  [unwired: 3 in]
            n2440 = call <vilib>:"Draw Line.vi"("picture"=w2811, "end point"=w2813, "color(black)"=u32 16448250, "pen"=T1 {"Width"=3, "Style"=enum."Solid"}) -> ("new picture"=w2785:picture)  [unwired: 5 in]
            n2441 = call <vilib>:"Move Pen.vi"("new position"=w2822, "picture"=w2785) -> ("new picture"=w2821:picture)  [unwired: 3 in]
            n2442 = call <vilib>:"Draw Line.vi"("picture"=w2821, "end point"=w2823, "color(black)"=u32 16448250, "pen"=T1 {"Width"=3, "Style"=enum."Solid"}) -> ("new picture"=w2784:picture)  [unwired: 5 in]
            n2443 = call <vilib>:"Move Pen.vi"("new position"=w2800, "picture"=w2784) -> ("new picture"=w2799:picture)  [unwired: 3 in]
            n2444 = call <vilib>:"Draw Line.vi"("picture"=w2799, "end point"=w2803, "color(black)"=u32 16448250, "pen"=T1 {"Width"=3, "Style"=enum."Solid"}) -> ("new picture"=w2783:picture)  [unwired: 5 in]
          }
          frame 9 {
            n2445 = Add(x=w2880, y=0) -> (x+y=w2924:i32)
            n2446 = Add(x=w2879, y=0) -> (x+y=w2925:i32)
            n2447 = Add(x=w2880, y=0) -> (x+y=w2936:i32)
            n2448 = Add(x=w2879, y=0) -> (x+y=w2937:i32)
            n2449 = Multiply(x=w2878, y=10) -> (x*y=w2923:i32)
            n2450 = Multiply(x=w2878, y=10) -> (x*y=w2934:i32)
            n2451 = Add(x=w2925, y=w2923) -> (x+y=w2926:i32)
            n2452 = Add(x=w2936, y=w2934) -> (x+y=w2935:i32)
            n2453 = Bundle(w2924, w2925) -> (w2921:cluster{i32, i32})  [unwired: 1 in]
            n2454 = Bundle(w2936, w2937) -> (w2933:cluster{i32, i32})  [unwired: 1 in]
            n2455 = Bundle(w2924, w2926) -> (w2922:cluster{i32, i32})  [unwired: 1 in]
            n2456 = call <vilib>:"Move Pen.vi"("new position"=w2933, "picture"=w2882) -> ("new picture"=w2932:picture)  [unwired: 3 in]
            n2457 = Bundle(w2935, w2937) -> (w2938:cluster{i32, i32})  [unwired: 1 in]
            n2458 = Multiply(x=w2878, y=10) -> (x*y=w2892:i32)
            n2459 = Add(x=w2880, y=w2892) -> (x+y=w2889:i32)
            n2460 = Add(x=w2879, y=w2892) -> (x+y=w2891:i32)
            n2461 = Add(x=w2891, y=w2892) -> (x+y=w2890:i32)
            n2462 = Bundle(w2889, w2891) -> (w2887:cluster{i32, i32})  [unwired: 1 in]
            n2463 = call <vilib>:"Draw Line.vi"("picture"=w2932, "end point"=w2938, "color(black)"=u32 16448250, "pen"=T1 {"Width"=3, "Style"=enum."Solid"}) -> ("new picture"=w2881:picture)  [unwired: 5 in]
            n2464 = Bundle(w2889, w2890) -> (w2888:cluster{i32, i32})  [unwired: 1 in]
            n2465 = Multiply(x=w2878, y=10) -> (x*y=w2911:i32)
            n2466 = Add(x=w2880, y=w2911) -> (x+y=w2912:i32)
            n2467 = Add(x=w2879, y=0) -> (x+y=w2914:i32)
            n2468 = Multiply(x=w2878, y=10) -> (x*y=w2902:i32)
            n2469 = Add(x=w2880, y=0) -> (x+y=w2900:i32)
            n2470 = Add(x=w2879, y=w2902) -> (x+y=w2903:i32)
            n2471 = Add(x=w2914, y=w2911) -> (x+y=w2913:i32)
            n2472 = Add(x=w2900, y=w2902) -> (x+y=w2899:i32)
            n2473 = Bundle(w2912, w2914) -> (w2909:cluster{i32, i32})  [unwired: 1 in]
            n2474 = Bundle(w2900, w2903) -> (w2898:cluster{i32, i32})  [unwired: 1 in]
            n2475 = Bundle(w2912, w2913) -> (w2910:cluster{i32, i32})  [unwired: 1 in]
            n2476 = call <vilib>:"Move Pen.vi"("new position"=w2898, "picture"=w2881) -> ("new picture"=w2897:picture)  [unwired: 3 in]
            n2477 = Bundle(w2899, w2903) -> (w2901:cluster{i32, i32})  [unwired: 1 in]
            n2478 = call <vilib>:"Draw Line.vi"("picture"=w2897, "end point"=w2901, "color(black)"=u32 16448250, "pen"=T1 {"Width"=3, "Style"=enum."Solid"}) -> ("new picture"=w2877:picture)  [unwired: 5 in]
            n2479 = call <vilib>:"Move Pen.vi"("new position"=w2921, "picture"=w2877) -> ("new picture"=w2920:picture)  [unwired: 3 in]
            n2480 = call <vilib>:"Draw Line.vi"("picture"=w2920, "end point"=w2922, "color(black)"=u32 16448250, "pen"=T1 {"Width"=3, "Style"=enum."Solid"}) -> ("new picture"=w2876:picture)  [unwired: 5 in]
            n2481 = call <vilib>:"Move Pen.vi"("new position"=w2909, "picture"=w2876) -> ("new picture"=w2908:picture)  [unwired: 3 in]
            n2482 = call <vilib>:"Draw Line.vi"("picture"=w2908, "end point"=w2910, "color(black)"=u32 16448250, "pen"=T1 {"Width"=3, "Style"=enum."Solid"}) -> ("new picture"=w2875:picture)  [unwired: 5 in]
            n2483 = call <vilib>:"Move Pen.vi"("new position"=w2887, "picture"=w2875) -> ("new picture"=w2886:picture)  [unwired: 3 in]
            n2484 = call <vilib>:"Draw Line.vi"("picture"=w2886, "end point"=w2888, "color(black)"=u32 16448250, "pen"=T1 {"Width"=3, "Style"=enum."Solid"}) -> ("new picture"=w2874:picture)  [unwired: 5 in]
          }
        }
        n2485 = case shown="9" w146 {
          tunnel: 570 -> [w1655 w1729 w1759 w1827 w1892 w1944 w2012 w2089 w2145 w2234]
          tunnel: 10 -> [w1654 w1728 w1758 w1826 w1891 w1943 w2011 w2088 w2144 w2233]
          tunnel: 3 -> [w1653 w1727 w1757 w1825 w1890 w1942 w2010 w2087 w2143 w2232]
          tunnel: w171 -> [w1656 w1731 w1761 w1828 w1893 w1946 w2014 w2091 w2147 w2236]
          tunnel: [w1647 w1726 w1753 w1820 w1886 w1938 w2005 w2084 w2137 w2228] -> w115
          frame 0, Default {
            n2486 = Add(x=w1655, y=0) -> (x+y=w1711:i32)
            n2487 = Add(x=w1654, y=0) -> (x+y=w1712:i32)
            n2488 = Multiply(x=w1653, y=10) -> (x*y=w1710:i32)
            n2489 = Add(x=w1655, y=0) -> (x+y=w1677:i32)
            n2490 = Multiply(x=w1653, y=10) -> (x*y=w1680:i32)
            n2491 = Add(x=w1654, y=w1680) -> (x+y=w1678:i32)
            n2492 = Add(x=w1712, y=w1710) -> (x+y=w1713:i32)
            n2493 = Add(x=w1678, y=w1680) -> (x+y=w1679:i32)
            n2494 = Bundle(w1711, w1712) -> (w1708:cluster{i32, i32})  [unwired: 1 in]
            n2495 = Bundle(w1677, w1678) -> (w1675:cluster{i32, i32})  [unwired: 1 in]
            n2496 = Bundle(w1711, w1713) -> (w1709:cluster{i32, i32})  [unwired: 1 in]
            n2497 = Bundle(w1677, w1679) -> (w1676:cluster{i32, i32})  [unwired: 1 in]
            n2498 = Multiply(x=w1653, y=10) -> (x*y=w1668:i32)
            n2499 = Multiply(x=2, y=w1668) -> (x*y=w1669:i32)
            n2500 = Add(x=w1655, y=0) -> (x+y=w1723:i32)
            n2501 = Add(x=w1654, y=0) -> (x+y=w1724:i32)
            n2502 = Add(x=w1655, y=0) -> (x+y=w1665:i32)
            n2503 = Add(x=w1654, y=w1669) -> (x+y=w1667:i32)
            n2504 = Multiply(x=w1653, y=10) -> (x*y=w1721:i32)
            n2505 = Add(x=w1665, y=w1668) -> (x+y=w1664:i32)
            n2506 = Add(x=w1723, y=w1721) -> (x+y=w1722:i32)
            n2507 = Bundle(w1723, w1724) -> (w1720:cluster{i32, i32})  [unwired: 1 in]
            n2508 = Bundle(w1665, w1667) -> (w1663:cluster{i32, i32})  [unwired: 1 in]
            n2509 = call <vilib>:"Move Pen.vi"("new position"=w1720, "picture"=w1656) -> ("new picture"=w1719:picture)  [unwired: 3 in]
            n2510 = Bundle(w1722, w1724) -> (w1725:cluster{i32, i32})  [unwired: 1 in]
            n2511 = Bundle(w1664, w1667) -> (w1666:cluster{i32, i32})  [unwired: 1 in]
            n2512 = Multiply(x=w1653, y=10) -> (x*y=w1698:i32)
            n2513 = Add(x=w1655, y=w1698) -> (x+y=w1699:i32)
            n2514 = Add(x=w1654, y=0) -> (x+y=w1701:i32)
            n2515 = Multiply(x=w1653, y=10) -> (x*y=w1690:i32)
            n2516 = Add(x=w1655, y=w1690) -> (x+y=w1687:i32)
            n2517 = Add(x=w1654, y=w1690) -> (x+y=w1689:i32)
            n2518 = Add(x=w1701, y=w1698) -> (x+y=w1700:i32)
            n2519 = Bundle(w1699, w1701) -> (w1696:cluster{i32, i32})  [unwired: 1 in]
            n2520 = call <vilib>:"Draw Line.vi"("picture"=w1719, "end point"=w1725, "color(black)"=u32 16448250, "pen"=T1 {"Width"=3, "Style"=enum."Solid"}) -> ("new picture"=w1652:picture)  [unwired: 5 in]
            n2521 = call <vilib>:"Move Pen.vi"("new position"=w1708, "picture"=w1652) -> ("new picture"=w1707:picture)  [unwired: 3 in]
            n2522 = call <vilib>:"Draw Line.vi"("picture"=w1707, "end point"=w1709, "color(black)"=u32 16448250, "pen"=T1 {"Width"=3, "Style"=enum."Solid"}) -> ("new picture"=w1651:picture)  [unwired: 5 in]
            n2523 = Add(x=w1689, y=w1690) -> (x+y=w1688:i32)
            n2524 = Bundle(w1687, w1689) -> (w1685:cluster{i32, i32})  [unwired: 1 in]
            n2525 = call <vilib>:"Move Pen.vi"("new position"=w1696, "picture"=w1651) -> ("new picture"=w1695:picture)  [unwired: 3 in]
            n2526 = Bundle(w1699, w1700) -> (w1697:cluster{i32, i32})  [unwired: 1 in]
            n2527 = Bundle(w1687, w1688) -> (w1686:cluster{i32, i32})  [unwired: 1 in]
            n2528 = call <vilib>:"Draw Line.vi"("picture"=w1695, "end point"=w1697, "color(black)"=u32 16448250, "pen"=T1 {"Width"=3, "Style"=enum."Solid"}) -> ("new picture"=w1650:picture)  [unwired: 5 in]
            n2529 = call <vilib>:"Move Pen.vi"("new position"=w1675, "picture"=w1650) -> ("new picture"=w1674:picture)  [unwired: 3 in]
            n2530 = call <vilib>:"Draw Line.vi"("picture"=w1674, "end point"=w1676, "color(black)"=u32 16448250, "pen"=T1 {"Width"=3, "Style"=enum."Solid"}) -> ("new picture"=w1649:picture)  [unwired: 5 in]
            n2531 = call <vilib>:"Move Pen.vi"("new position"=w1685, "picture"=w1649) -> ("new picture"=w1684:picture)  [unwired: 3 in]
            n2532 = call <vilib>:"Draw Line.vi"("picture"=w1684, "end point"=w1686, "color(black)"=u32 16448250, "pen"=T1 {"Width"=3, "Style"=enum."Solid"}) -> ("new picture"=w1648:picture)  [unwired: 5 in]
            n2533 = call <vilib>:"Move Pen.vi"("new position"=w1663, "picture"=w1648) -> ("new picture"=w1662:picture)  [unwired: 3 in]
            n2534 = call <vilib>:"Draw Line.vi"("picture"=w1662, "end point"=w1666, "color(black)"=u32 16448250, "pen"=T1 {"Width"=3, "Style"=enum."Solid"}) -> ("new picture"=w1647:picture)  [unwired: 5 in]
          }
          frame 1 {
            n2535 = Multiply(x=w1727, y=10) -> (x*y=w1749:i32)
            n2536 = Add(x=w1729, y=w1749) -> (x+y=w1750:i32)
            n2537 = Add(x=w1728, y=0) -> (x+y=w1752:i32)
            n2538 = Add(x=w1752, y=w1749) -> (x+y=w1751:i32)
            n2539 = Bundle(w1750, w1752) -> (w1747:cluster{i32, i32})  [unwired: 1 in]
            n2540 = call <vilib>:"Move Pen.vi"("new position"=w1747, "picture"=w1731) -> ("new picture"=w1746:picture)  [unwired: 3 in]
            n2541 = Bundle(w1750, w1751) -> (w1748:cluster{i32, i32})  [unwired: 1 in]
            n2542 = call <vilib>:"Draw Line.vi"("picture"=w1746, "end point"=w1748, "color(black)"=u32 16448250, "pen"=T1 {"Width"=3, "Style"=enum."Solid"}) -> ("new picture"=w1730:picture)  [unwired: 5 in]
            n2543 = Multiply(x=w1727, y=10) -> (x*y=w1741:i32)
            n2544 = Add(x=w1729, y=w1741) -> (x+y=w1738:i32)
            n2545 = Add(x=w1728, y=w1741) -> (x+y=w1740:i32)
            n2546 = Add(x=w1740, y=w1741) -> (x+y=w1739:i32)
            n2547 = Bundle(w1738, w1740) -> (w1736:cluster{i32, i32})  [unwired: 1 in]
            n2548 = call <vilib>:"Move Pen.vi"("new position"=w1736, "picture"=w1730) -> ("new picture"=w1735:picture)  [unwired: 3 in]
            n2549 = Bundle(w1738, w1739) -> (w1737:cluster{i32, i32})  [unwired: 1 in]
            n2550 = call <vilib>:"Draw Line.vi"("picture"=w1735, "end point"=w1737, "color(black)"=u32 16448250, "pen"=T1 {"Width"=3, "Style"=enum."Solid"}) -> ("new picture"=w1726:picture)  [unwired: 5 in]
          }
          frame 2 {
            n2551 = Multiply(x=w1757, y=10) -> (x*y=w1795:i32)
            n2552 = Add(x=w1759, y=0) -> (x+y=w1793:i32)
            n2553 = Add(x=w1758, y=w1795) -> (x+y=w1796:i32)
            n2554 = Add(x=w1759, y=0) -> (x+y=w1817:i32)
            n2555 = Add(x=w1758, y=0) -> (x+y=w1818:i32)
            n2556 = Multiply(x=w1757, y=10) -> (x*y=w1815:i32)
            n2557 = Add(x=w1793, y=w1795) -> (x+y=w1792:i32)
            n2558 = Add(x=w1817, y=w1815) -> (x+y=w1816:i32)
            n2559 = Bundle(w1793, w1796) -> (w1791:cluster{i32, i32})  [unwired: 1 in]
            n2560 = Bundle(w1817, w1818) -> (w1814:cluster{i32, i32})  [unwired: 1 in]
            n2561 = Bundle(w1792, w1796) -> (w1794:cluster{i32, i32})  [unwired: 1 in]
            n2562 = call <vilib>:"Move Pen.vi"("new position"=w1814, "picture"=w1761) -> ("new picture"=w1813:picture)  [unwired: 3 in]
            n2563 = Bundle(w1816, w1818) -> (w1819:cluster{i32, i32})  [unwired: 1 in]
            n2564 = Multiply(x=w1757, y=10) -> (x*y=w1773:i32)
            n2565 = Multiply(x=2, y=w1773) -> (x*y=w1774:i32)
            n2566 = Add(x=w1759, y=0) -> (x+y=w1770:i32)
            n2567 = Add(x=w1758, y=w1774) -> (x+y=w1772:i32)
            n2568 = Add(x=w1770, y=w1773) -> (x+y=w1769:i32)
            n2569 = Bundle(w1770, w1772) -> (w1768:cluster{i32, i32})  [unwired: 1 in]
            n2570 = call <vilib>:"Draw Line.vi"("picture"=w1813, "end point"=w1819, "color(black)"=u32 16448250, "pen"=T1 {"Width"=3, "Style"=enum."Solid"}) -> ("new picture"=w1760:picture)  [unwired: 5 in]
            n2571 = Bundle(w1769, w1772) -> (w1771:cluster{i32, i32})  [unwired: 1 in]
            n2572 = Multiply(x=w1757, y=10) -> (x*y=w1804:i32)
            n2573 = Add(x=w1759, y=0) -> (x+y=w1782:i32)
            n2574 = Add(x=w1759, y=w1804) -> (x+y=w1805:i32)
            n2575 = Add(x=w1758, y=0) -> (x+y=w1807:i32)
            n2576 = Multiply(x=w1757, y=10) -> (x*y=w1785:i32)
            n2577 = Add(x=w1758, y=w1785) -> (x+y=w1783:i32)
            n2578 = Add(x=w1783, y=w1785) -> (x+y=w1784:i32)
            n2579 = Add(x=w1807, y=w1804) -> (x+y=w1806:i32)
            n2580 = Bundle(w1782, w1783) -> (w1780:cluster{i32, i32})  [unwired: 1 in]
            n2581 = Bundle(w1805, w1807) -> (w1802:cluster{i32, i32})  [unwired: 1 in]
            n2582 = call <vilib>:"Move Pen.vi"("new position"=w1802, "picture"=w1760) -> ("new picture"=w1801:picture)  [unwired: 3 in]
            n2583 = Bundle(w1782, w1784) -> (w1781:cluster{i32, i32})  [unwired: 1 in]
            n2584 = Bundle(w1805, w1806) -> (w1803:cluster{i32, i32})  [unwired: 1 in]
            n2585 = call <vilib>:"Draw Line.vi"("picture"=w1801, "end point"=w1803, "color(black)"=u32 16448250, "pen"=T1 {"Width"=3, "Style"=enum."Solid"}) -> ("new picture"=w1756:picture)  [unwired: 5 in]
            n2586 = call <vilib>:"Move Pen.vi"("new position"=w1791, "picture"=w1756) -> ("new picture"=w1790:picture)  [unwired: 3 in]
            n2587 = call <vilib>:"Draw Line.vi"("picture"=w1790, "end point"=w1794, "color(black)"=u32 16448250, "pen"=T1 {"Width"=3, "Style"=enum."Solid"}) -> ("new picture"=w1755:picture)  [unwired: 5 in]
            n2588 = call <vilib>:"Move Pen.vi"("new position"=w1780, "picture"=w1755) -> ("new picture"=w1779:picture)  [unwired: 3 in]
            n2589 = call <vilib>:"Draw Line.vi"("picture"=w1779, "end point"=w1781, "color(black)"=u32 16448250, "pen"=T1 {"Width"=3, "Style"=enum."Solid"}) -> ("new picture"=w1754:picture)  [unwired: 5 in]
            n2590 = call <vilib>:"Move Pen.vi"("new position"=w1768, "picture"=w1754) -> ("new picture"=w1767:picture)  [unwired: 3 in]
            n2591 = call <vilib>:"Draw Line.vi"("picture"=w1767, "end point"=w1771, "color(black)"=u32 16448250, "pen"=T1 {"Width"=3, "Style"=enum."Solid"}) -> ("new picture"=w1753:picture)  [unwired: 5 in]
          }
          frame 3 {
            n2592 = Multiply(x=w1825, y=10) -> (x*y=w1861:i32)
            n2593 = Add(x=w1827, y=0) -> (x+y=w1859:i32)
            n2594 = Add(x=w1826, y=w1861) -> (x+y=w1862:i32)
            n2595 = Add(x=w1827, y=0) -> (x+y=w1883:i32)
            n2596 = Add(x=w1826, y=0) -> (x+y=w1884:i32)
            n2597 = Multiply(x=w1825, y=10) -> (x*y=w1881:i32)
            n2598 = Add(x=w1859, y=w1861) -> (x+y=w1858:i32)
            n2599 = Add(x=w1883, y=w1881) -> (x+y=w1882:i32)
            n2600 = Bundle(w1859, w1862) -> (w1857:cluster{i32, i32})  [unwired: 1 in]
            n2601 = Bundle(w1883, w1884) -> (w1880:cluster{i32, i32})  [unwired: 1 in]
            n2602 = call <vilib>:"Move Pen.vi"("new position"=w1880, "picture"=w1828) -> ("new picture"=w1879:picture)  [unwired: 3 in]
            n2603 = Bundle(w1858, w1862) -> (w1860:cluster{i32, i32})  [unwired: 1 in]
            n2604 = Bundle(w1882, w1884) -> (w1885:cluster{i32, i32})  [unwired: 1 in]
            n2605 = Multiply(x=w1825, y=10) -> (x*y=w1840:i32)
            n2606 = Multiply(x=2, y=w1840) -> (x*y=w1841:i32)
            n2607 = Add(x=w1827, y=0) -> (x+y=w1837:i32)
            n2608 = Add(x=w1826, y=w1841) -> (x+y=w1839:i32)
            n2609 = Add(x=w1837, y=w1840) -> (x+y=w1836:i32)
            n2610 = call <vilib>:"Draw Line.vi"("picture"=w1879, "end point"=w1885, "color(black)"=u32 16448250, "pen"=T1 {"Width"=3, "Style"=enum."Solid"}) -> ("new picture"=w1824:picture)  [unwired: 5 in]
            n2611 = Bundle(w1837, w1839) -> (w1835:cluster{i32, i32})  [unwired: 1 in]
            n2612 = Bundle(w1836, w1839) -> (w1838:cluster{i32, i32})  [unwired: 1 in]
            n2613 = Multiply(x=w1825, y=10) -> (x*y=w1851:i32)
            n2614 = Add(x=w1827, y=w1851) -> (x+y=w1848:i32)
            n2615 = Add(x=w1826, y=w1851) -> (x+y=w1850:i32)
            n2616 = Multiply(x=w1825, y=10) -> (x*y=w1870:i32)
            n2617 = Add(x=w1827, y=w1870) -> (x+y=w1871:i32)
            n2618 = Add(x=w1826, y=0) -> (x+y=w1873:i32)
            n2619 = Add(x=w1850, y=w1851) -> (x+y=w1849:i32)
            n2620 = Bundle(w1848, w1850) -> (w1846:cluster{i32, i32})  [unwired: 1 in]
            n2621 = Add(x=w1873, y=w1870) -> (x+y=w1872:i32)
            n2622 = Bundle(w1871, w1873) -> (w1868:cluster{i32, i32})  [unwired: 1 in]
            n2623 = Bundle(w1848, w1849) -> (w1847:cluster{i32, i32})  [unwired: 1 in]
            n2624 = call <vilib>:"Move Pen.vi"("new position"=w1868, "picture"=w1824) -> ("new picture"=w1867:picture)  [unwired: 3 in]
            n2625 = Bundle(w1871, w1872) -> (w1869:cluster{i32, i32})  [unwired: 1 in]
            n2626 = call <vilib>:"Draw Line.vi"("picture"=w1867, "end point"=w1869, "color(black)"=u32 16448250, "pen"=T1 {"Width"=3, "Style"=enum."Solid"}) -> ("new picture"=w1823:picture)  [unwired: 5 in]
            n2627 = call <vilib>:"Move Pen.vi"("new position"=w1857, "picture"=w1823) -> ("new picture"=w1856:picture)  [unwired: 3 in]
            n2628 = call <vilib>:"Draw Line.vi"("picture"=w1856, "end point"=w1860, "color(black)"=u32 16448250, "pen"=T1 {"Width"=3, "Style"=enum."Solid"}) -> ("new picture"=w1822:picture)  [unwired: 5 in]
            n2629 = call <vilib>:"Move Pen.vi"("new position"=w1846, "picture"=w1822) -> ("new picture"=w1845:picture)  [unwired: 3 in]
            n2630 = call <vilib>:"Draw Line.vi"("picture"=w1845, "end point"=w1847, "color(black)"=u32 16448250, "pen"=T1 {"Width"=3, "Style"=enum."Solid"}) -> ("new picture"=w1821:picture)  [unwired: 5 in]
            n2631 = call <vilib>:"Move Pen.vi"("new position"=w1835, "picture"=w1821) -> ("new picture"=w1834:picture)  [unwired: 3 in]
            n2632 = call <vilib>:"Draw Line.vi"("picture"=w1834, "end point"=w1838, "color(black)"=u32 16448250, "pen"=T1 {"Width"=3, "Style"=enum."Solid"}) -> ("new picture"=w1820:picture)  [unwired: 5 in]
          }
          frame 4 {
            n2633 = Add(x=w1892, y=0) -> (x+y=w1935:i32)
            n2634 = Add(x=w1891, y=0) -> (x+y=w1936:i32)
            n2635 = Multiply(x=w1890, y=10) -> (x*y=w1934:i32)
            n2636 = Add(x=w1936, y=w1934) -> (x+y=w1937:i32)
            n2637 = Bundle(w1935, w1936) -> (w1932:cluster{i32, i32})  [unwired: 1 in]
            n2638 = call <vilib>:"Move Pen.vi"("new position"=w1932, "picture"=w1893) -> ("new picture"=w1931:picture)  [unwired: 3 in]
            n2639 = Bundle(w1935, w1937) -> (w1933:cluster{i32, i32})  [unwired: 1 in]
            n2640 = Multiply(x=w1890, y=10) -> (x*y=w1913:i32)
            n2641 = Add(x=w1892, y=0) -> (x+y=w1911:i32)
            n2642 = Add(x=w1891, y=w1913) -> (x+y=w1914:i32)
            n2643 = Add(x=w1911, y=w1913) -> (x+y=w1910:i32)
            n2644 = Bundle(w1911, w1914) -> (w1909:cluster{i32, i32})  [unwired: 1 in]
            n2645 = call <vilib>:"Draw Line.vi"("picture"=w1931, "end point"=w1933, "color(black)"=u32 16448250, "pen"=T1 {"Width"=3, "Style"=enum."Solid"}) -> ("new picture"=w1887:picture)  [unwired: 5 in]
            n2646 = Multiply(x=w1890, y=10) -> (x*y=w1903:i32)
            n2647 = Add(x=w1892, y=w1903) -> (x+y=w1900:i32)
            n2648 = Add(x=w1891, y=w1903) -> (x+y=w1902:i32)
            n2649 = Bundle(w1910, w1914) -> (w1912:cluster{i32, i32})  [unwired: 1 in]
            n2650 = Add(x=w1902, y=w1903) -> (x+y=w1901:i32)
            n2651 = Bundle(w1900, w1902) -> (w1898:cluster{i32, i32})  [unwired: 1 in]
            n2652 = Multiply(x=w1890, y=10) -> (x*y=w1922:i32)
            n2653 = Add(x=w1892, y=w1922) -> (x+y=w1923:i32)
            n2654 = Add(x=w1891, y=0) -> (x+y=w1925:i32)
            n2655 = Add(x=w1925, y=w1922) -> (x+y=w1924:i32)
            n2656 = Bundle(w1900, w1901) -> (w1899:cluster{i32, i32})  [unwired: 1 in]
            n2657 = Bundle(w1923, w1925) -> (w1920:cluster{i32, i32})  [unwired: 1 in]
            n2658 = call <vilib>:"Move Pen.vi"("new position"=w1920, "picture"=w1887) -> ("new picture"=w1919:picture)  [unwired: 3 in]
            n2659 = Bundle(w1923, w1924) -> (w1921:cluster{i32, i32})  [unwired: 1 in]
            n2660 = call <vilib>:"Draw Line.vi"("picture"=w1919, "end point"=w1921, "color(black)"=u32 16448250, "pen"=T1 {"Width"=3, "Style"=enum."Solid"}) -> ("new picture"=w1889:picture)  [unwired: 5 in]
            n2661 = call <vilib>:"Move Pen.vi"("new position"=w1909, "picture"=w1889) -> ("new picture"=w1908:picture)  [unwired: 3 in]
            n2662 = call <vilib>:"Draw Line.vi"("picture"=w1908, "end point"=w1912, "color(black)"=u32 16448250, "pen"=T1 {"Width"=3, "Style"=enum."Solid"}) -> ("new picture"=w1888:picture)  [unwired: 5 in]
            n2663 = call <vilib>:"Move Pen.vi"("new position"=w1898, "picture"=w1888) -> ("new picture"=w1897:picture)  [unwired: 3 in]
            n2664 = call <vilib>:"Draw Line.vi"("picture"=w1897, "end point"=w1899, "color(black)"=u32 16448250, "pen"=T1 {"Width"=3, "Style"=enum."Solid"}) -> ("new picture"=w1886:picture)  [unwired: 5 in]
          }
          frame 5 {
            n2665 = Multiply(x=w1942, y=10) -> (x*y=w1979:i32)
            n2666 = Add(x=w1944, y=0) -> (x+y=w1977:i32)
            n2667 = Add(x=w1943, y=w1979) -> (x+y=w1980:i32)
            n2668 = Add(x=w1944, y=0) -> (x+y=w2002:i32)
            n2669 = Add(x=w1943, y=0) -> (x+y=w2003:i32)
            n2670 = Add(x=w1977, y=w1979) -> (x+y=w1976:i32)
            n2671 = Multiply(x=w1942, y=10) -> (x*y=w2000:i32)
            n2672 = Bundle(w1977, w1980) -> (w1975:cluster{i32, i32})  [unwired: 1 in]
            n2673 = Add(x=w2002, y=w2000) -> (x+y=w2001:i32)
            n2674 = Bundle(w2002, w2003) -> (w1999:cluster{i32, i32})  [unwired: 1 in]
            n2675 = Bundle(w1976, w1980) -> (w1978:cluster{i32, i32})  [unwired: 1 in]
            n2676 = call <vilib>:"Move Pen.vi"("new position"=w1999, "picture"=w1946) -> ("new picture"=w1998:picture)  [unwired: 3 in]
            n2677 = Bundle(w2001, w2003) -> (w2004:cluster{i32, i32})  [unwired: 1 in]
            n2678 = Multiply(x=w1942, y=10) -> (x*y=w1958:i32)
            n2679 = Multiply(x=2, y=w1958) -> (x*y=w1959:i32)
            n2680 = Add(x=w1944, y=0) -> (x+y=w1955:i32)
            n2681 = Add(x=w1943, y=w1959) -> (x+y=w1957:i32)
            n2682 = Add(x=w1955, y=w1958) -> (x+y=w1954:i32)
            n2683 = Bundle(w1955, w1957) -> (w1953:cluster{i32, i32})  [unwired: 1 in]
            n2684 = call <vilib>:"Draw Line.vi"("picture"=w1998, "end point"=w2004, "color(black)"=u32 16448250, "pen"=T1 {"Width"=3, "Style"=enum."Solid"}) -> ("new picture"=w1945:picture)  [unwired: 5 in]
            n2685 = Bundle(w1954, w1957) -> (w1956:cluster{i32, i32})  [unwired: 1 in]
            n2686 = Multiply(x=w1942, y=10) -> (x*y=w1969:i32)
            n2687 = Add(x=w1944, y=0) -> (x+y=w1990:i32)
            n2688 = Add(x=w1943, y=0) -> (x+y=w1991:i32)
            n2689 = Add(x=w1944, y=w1969) -> (x+y=w1966:i32)
            n2690 = Add(x=w1943, y=w1969) -> (x+y=w1968:i32)
            n2691 = Multiply(x=w1942, y=10) -> (x*y=w1989:i32)
            n2692 = Add(x=w1991, y=w1989) -> (x+y=w1992:i32)
            n2693 = Add(x=w1968, y=w1969) -> (x+y=w1967:i32)
            n2694 = Bundle(w1990, w1991) -> (w1987:cluster{i32, i32})  [unwired: 1 in]
            n2695 = Bundle(w1966, w1968) -> (w1964:cluster{i32, i32})  [unwired: 1 in]
            n2696 = call <vilib>:"Move Pen.vi"("new position"=w1987, "picture"=w1945) -> ("new picture"=w1986:picture)  [unwired: 3 in]
            n2697 = Bundle(w1990, w1992) -> (w1988:cluster{i32, i32})  [unwired: 1 in]
            n2698 = Bundle(w1966, w1967) -> (w1965:cluster{i32, i32})  [unwired: 1 in]
            n2699 = call <vilib>:"Draw Line.vi"("picture"=w1986, "end point"=w1988, "color(black)"=u32 16448250, "pen"=T1 {"Width"=3, "Style"=enum."Solid"}) -> ("new picture"=w1941:picture)  [unwired: 5 in]
            n2700 = call <vilib>:"Move Pen.vi"("new position"=w1975, "picture"=w1941) -> ("new picture"=w1974:picture)  [unwired: 3 in]
            n2701 = call <vilib>:"Draw Line.vi"("picture"=w1974, "end point"=w1978, "color(black)"=u32 16448250, "pen"=T1 {"Width"=3, "Style"=enum."Solid"}) -> ("new picture"=w1940:picture)  [unwired: 5 in]
            n2702 = call <vilib>:"Move Pen.vi"("new position"=w1964, "picture"=w1940) -> ("new picture"=w1963:picture)  [unwired: 3 in]
            n2703 = call <vilib>:"Draw Line.vi"("picture"=w1963, "end point"=w1965, "color(black)"=u32 16448250, "pen"=T1 {"Width"=3, "Style"=enum."Solid"}) -> ("new picture"=w1939:picture)  [unwired: 5 in]
            n2704 = call <vilib>:"Move Pen.vi"("new position"=w1953, "picture"=w1939) -> ("new picture"=w1952:picture)  [unwired: 3 in]
            n2705 = call <vilib>:"Draw Line.vi"("picture"=w1952, "end point"=w1956, "color(black)"=u32 16448250, "pen"=T1 {"Width"=3, "Style"=enum."Solid"}) -> ("new picture"=w1938:picture)  [unwired: 5 in]
          }
          frame 6 {
            n2706 = Multiply(x=w2010, y=10) -> (x*y=w2048:i32)
            n2707 = Multiply(x=w2010, y=10) -> (x*y=w2058:i32)
            n2708 = Add(x=w2012, y=w2048) -> (x+y=w2045:i32)
            n2709 = Add(x=w2011, y=w2048) -> (x+y=w2047:i32)
            n2710 = Add(x=w2012, y=0) -> (x+y=w2056:i32)
            n2711 = Add(x=w2011, y=w2058) -> (x+y=w2059:i32)
            n2712 = Add(x=w2012, y=0) -> (x+y=w2081:i32)
            n2713 = Add(x=w2011, y=0) -> (x+y=w2082:i32)
            n2714 = Multiply(x=w2010, y=10) -> (x*y=w2079:i32)
            n2715 = Add(x=w2056, y=w2058) -> (x+y=w2055:i32)
            n2716 = Add(x=w2047, y=w2048) -> (x+y=w2046:i32)
            n2717 = Bundle(w2045, w2047) -> (w2043:cluster{i32, i32})  [unwired: 1 in]
            n2718 = Bundle(w2056, w2059) -> (w2054:cluster{i32, i32})  [unwired: 1 in]
            n2719 = Add(x=w2081, y=w2079) -> (x+y=w2080:i32)
            n2720 = Bundle(w2081, w2082) -> (w2078:cluster{i32, i32})  [unwired: 1 in]
            n2721 = Bundle(w2045, w2046) -> (w2044:cluster{i32, i32})  [unwired: 1 in]
            n2722 = Bundle(w2055, w2059) -> (w2057:cluster{i32, i32})  [unwired: 1 in]
            n2723 = call <vilib>:"Move Pen.vi"("new position"=w2078, "picture"=w2014) -> ("new picture"=w2077:picture)  [unwired: 3 in]
            n2724 = Bundle(w2080, w2082) -> (w2083:cluster{i32, i32})  [unwired: 1 in]
            n2725 = call <vilib>:"Draw Line.vi"("picture"=w2077, "end point"=w2083, "color(black)"=u32 16448250, "pen"=T1 {"Width"=3, "Style"=enum."Solid"}) -> ("new picture"=w2013:picture)  [unwired: 5 in]
            n2726 = Multiply(x=w2010, y=10) -> (x*y=w2026:i32)
            n2727 = Multiply(x=2, y=w2026) -> (x*y=w2027:i32)
            n2728 = Add(x=w2012, y=0) -> (x+y=w2035:i32)
            n2729 = Multiply(x=w2010, y=10) -> (x*y=w2038:i32)
            n2730 = Add(x=w2011, y=w2038) -> (x+y=w2036:i32)
            n2731 = Add(x=w2012, y=0) -> (x+y=w2023:i32)
            n2732 = Add(x=w2011, y=w2027) -> (x+y=w2025:i32)
            n2733 = Add(x=w2012, y=0) -> (x+y=w2069:i32)
            n2734 = Add(x=w2011, y=0) -> (x+y=w2070:i32)
            n2735 = Multiply(x=w2010, y=10) -> (x*y=w2068:i32)
            n2736 = Add(x=w2036, y=w2038) -> (x+y=w2037:i32)
            n2737 = Add(x=w2023, y=w2026) -> (x+y=w2022:i32)
            n2738 = Add(x=w2070, y=w2068) -> (x+y=w2071:i32)
            n2739 = Bundle(w2035, w2036) -> (w2033:cluster{i32, i32})  [unwired: 1 in]
            n2740 = Bundle(w2023, w2025) -> (w2021:cluster{i32, i32})  [unwired: 1 in]
            n2741 = Bundle(w2069, w2070) -> (w2066:cluster{i32, i32})  [unwired: 1 in]
            n2742 = Bundle(w2035, w2037) -> (w2034:cluster{i32, i32})  [unwired: 1 in]
            n2743 = Bundle(w2022, w2025) -> (w2024:cluster{i32, i32})  [unwired: 1 in]
            n2744 = call <vilib>:"Move Pen.vi"("new position"=w2066, "picture"=w2013) -> ("new picture"=w2065:picture)  [unwired: 3 in]
            n2745 = Bundle(w2069, w2071) -> (w2067:cluster{i32, i32})  [unwired: 1 in]
            n2746 = call <vilib>:"Draw Line.vi"("picture"=w2065, "end point"=w2067, "color(black)"=u32 16448250, "pen"=T1 {"Width"=3, "Style"=enum."Solid"}) -> ("new picture"=w2009:picture)  [unwired: 5 in]
            n2747 = call <vilib>:"Move Pen.vi"("new position"=w2054, "picture"=w2009) -> ("new picture"=w2053:picture)  [unwired: 3 in]
            n2748 = call <vilib>:"Draw Line.vi"("picture"=w2053, "end point"=w2057, "color(black)"=u32 16448250, "pen"=T1 {"Width"=3, "Style"=enum."Solid"}) -> ("new picture"=w2008:picture)  [unwired: 5 in]
            n2749 = call <vilib>:"Move Pen.vi"("new position"=w2033, "picture"=w2008) -> ("new picture"=w2032:picture)  [unwired: 3 in]
            n2750 = call <vilib>:"Draw Line.vi"("picture"=w2032, "end point"=w2034, "color(black)"=u32 16448250, "pen"=T1 {"Width"=3, "Style"=enum."Solid"}) -> ("new picture"=w2007:picture)  [unwired: 5 in]
            n2751 = call <vilib>:"Move Pen.vi"("new position"=w2043, "picture"=w2007) -> ("new picture"=w2042:picture)  [unwired: 3 in]
            n2752 = call <vilib>:"Draw Line.vi"("picture"=w2042, "end point"=w2044, "color(black)"=u32 16448250, "pen"=T1 {"Width"=3, "Style"=enum."Solid"}) -> ("new picture"=w2006:picture)  [unwired: 5 in]
            n2753 = call <vilib>:"Move Pen.vi"("new position"=w2021, "picture"=w2006) -> ("new picture"=w2020:picture)  [unwired: 3 in]
            n2754 = call <vilib>:"Draw Line.vi"("picture"=w2020, "end point"=w2024, "color(black)"=u32 16448250, "pen"=T1 {"Width"=3, "Style"=enum."Solid"}) -> ("new picture"=w2005:picture)  [unwired: 5 in]
          }
          frame 7 {
            n2755 = Add(x=w2089, y=0) -> (x+y=w2122:i32)
            n2756 = Add(x=w2088, y=0) -> (x+y=w2123:i32)
            n2757 = Multiply(x=w2087, y=10) -> (x*y=w2121:i32)
            n2758 = Add(x=w2123, y=w2121) -> (x+y=w2124:i32)
            n2759 = Add(x=w2089, y=0) -> (x+y=w2134:i32)
            n2760 = Add(x=w2088, y=0) -> (x+y=w2135:i32)
            n2761 = Bundle(w2122, w2123) -> (w2119:cluster{i32, i32})  [unwired: 1 in]
            n2762 = Multiply(x=w2087, y=10) -> (x*y=w2132:i32)
            n2763 = Add(x=w2134, y=w2132) -> (x+y=w2133:i32)
            n2764 = Bundle(w2134, w2135) -> (w2131:cluster{i32, i32})  [unwired: 1 in]
            n2765 = Bundle(w2122, w2124) -> (w2120:cluster{i32, i32})  [unwired: 1 in]
            n2766 = call <vilib>:"Move Pen.vi"("new position"=w2131, "picture"=w2091) -> ("new picture"=w2130:picture)  [unwired: 3 in]
            n2767 = Bundle(w2133, w2135) -> (w2136:cluster{i32, i32})  [unwired: 1 in]
            n2768 = call <vilib>:"Draw Line.vi"("picture"=w2130, "end point"=w2136, "color(black)"=u32 16448250, "pen"=T1 {"Width"=3, "Style"=enum."Solid"}) -> ("new picture"=w2090:picture)  [unwired: 5 in]
            n2769 = Multiply(x=w2087, y=10) -> (x*y=w2109:i32)
            n2770 = Add(x=w2089, y=w2109) -> (x+y=w2110:i32)
            n2771 = Add(x=w2088, y=0) -> (x+y=w2112:i32)
            n2772 = Multiply(x=w2087, y=10) -> (x*y=w2101:i32)
            n2773 = Add(x=w2089, y=w2101) -> (x+y=w2098:i32)
            n2774 = Add(x=w2088, y=w2101) -> (x+y=w2100:i32)
            n2775 = Add(x=w2112, y=w2109) -> (x+y=w2111:i32)
            n2776 = Bundle(w2110, w2112) -> (w2107:cluster{i32, i32})  [unwired: 1 in]
            n2777 = Add(x=w2100, y=w2101) -> (x+y=w2099:i32)
            n2778 = Bundle(w2098, w2100) -> (w2096:cluster{i32, i32})  [unwired: 1 in]
            n2779 = Bundle(w2110, w2111) -> (w2108:cluster{i32, i32})  [unwired: 1 in]
            n2780 = call <vilib>:"Move Pen.vi"("new position"=w2096, "picture"=w2090) -> ("new picture"=w2095:picture)  [unwired: 3 in]
            n2781 = Bundle(w2098, w2099) -> (w2097:cluster{i32, i32})  [unwired: 1 in]
            n2782 = call <vilib>:"Draw Line.vi"("picture"=w2095, "end point"=w2097, "color(black)"=u32 16448250, "pen"=T1 {"Width"=3, "Style"=enum."Solid"}) -> ("new picture"=w2086:picture)  [unwired: 5 in]
            n2783 = call <vilib>:"Move Pen.vi"("new position"=w2119, "picture"=w2086) -> ("new picture"=w2118:picture)  [unwired: 3 in]
            n2784 = call <vilib>:"Draw Line.vi"("picture"=w2118, "end point"=w2120, "color(black)"=u32 16448250, "pen"=T1 {"Width"=3, "Style"=enum."Solid"}) -> ("new picture"=w2085:picture)  [unwired: 5 in]
            n2785 = call <vilib>:"Move Pen.vi"("new position"=w2107, "picture"=w2085) -> ("new picture"=w2106:picture)  [unwired: 3 in]
            n2786 = call <vilib>:"Draw Line.vi"("picture"=w2106, "end point"=w2108, "color(black)"=u32 16448250, "pen"=T1 {"Width"=3, "Style"=enum."Solid"}) -> ("new picture"=w2084:picture)  [unwired: 5 in]
          }
          frame 8 {
            n2787 = Add(x=w2145, y=0) -> (x+y=w2213:i32)
            n2788 = Add(x=w2144, y=0) -> (x+y=w2214:i32)
            n2789 = Add(x=w2145, y=0) -> (x+y=w2168:i32)
            n2790 = Multiply(x=w2143, y=10) -> (x*y=w2212:i32)
            n2791 = Multiply(x=w2143, y=10) -> (x*y=w2171:i32)
            n2792 = Add(x=w2144, y=w2171) -> (x+y=w2169:i32)
            n2793 = Add(x=w2145, y=0) -> (x+y=w2225:i32)
            n2794 = Add(x=w2144, y=0) -> (x+y=w2226:i32)
            n2795 = Multiply(x=w2143, y=10) -> (x*y=w2223:i32)
            n2796 = Add(x=w2214, y=w2212) -> (x+y=w2215:i32)
            n2797 = Add(x=w2169, y=w2171) -> (x+y=w2170:i32)
            n2798 = Bundle(w2213, w2214) -> (w2210:cluster{i32, i32})  [unwired: 1 in]
            n2799 = Bundle(w2168, w2169) -> (w2166:cluster{i32, i32})  [unwired: 1 in]
            n2800 = Multiply(x=w2143, y=10) -> (x*y=w2159:i32)
            n2801 = Multiply(x=2, y=w2159) -> (x*y=w2160:i32)
            n2802 = Add(x=w2225, y=w2223) -> (x+y=w2224:i32)
            n2803 = Bundle(w2225, w2226) -> (w2222:cluster{i32, i32})  [unwired: 1 in]
            n2804 = Add(x=w2145, y=0) -> (x+y=w2156:i32)
            n2805 = Add(x=w2144, y=w2160) -> (x+y=w2158:i32)
            n2806 = Add(x=w2156, y=w2159) -> (x+y=w2155:i32)
            n2807 = Bundle(w2213, w2215) -> (w2211:cluster{i32, i32})  [unwired: 1 in]
            n2808 = Bundle(w2168, w2170) -> (w2167:cluster{i32, i32})  [unwired: 1 in]
            n2809 = Bundle(w2156, w2158) -> (w2154:cluster{i32, i32})  [unwired: 1 in]
            n2810 = call <vilib>:"Move Pen.vi"("new position"=w2222, "picture"=w2147) -> ("new picture"=w2221:picture)  [unwired: 3 in]
            n2811 = Bundle(w2224, w2226) -> (w2227:cluster{i32, i32})  [unwired: 1 in]
            n2812 = Bundle(w2155, w2158) -> (w2157:cluster{i32, i32})  [unwired: 1 in]
            n2813 = call <vilib>:"Draw Line.vi"("picture"=w2221, "end point"=w2227, "color(black)"=u32 16448250, "pen"=T1 {"Width"=3, "Style"=enum."Solid"}) -> ("new picture"=w2146:picture)  [unwired: 5 in]
            n2814 = Multiply(x=w2143, y=10) -> (x*y=w2191:i32)
            n2815 = Multiply(x=w2143, y=10) -> (x*y=w2200:i32)
            n2816 = Add(x=w2145, y=0) -> (x+y=w2189:i32)
            n2817 = Multiply(x=w2143, y=10) -> (x*y=w2181:i32)
            n2818 = Add(x=w2144, y=w2191) -> (x+y=w2192:i32)
            n2819 = Add(x=w2145, y=w2200) -> (x+y=w2201:i32)
            n2820 = Add(x=w2144, y=0) -> (x+y=w2203:i32)
            n2821 = Add(x=w2145, y=w2181) -> (x+y=w2178:i32)
            n2822 = Add(x=w2144, y=w2181) -> (x+y=w2180:i32)
            n2823 = Add(x=w2189, y=w2191) -> (x+y=w2188:i32)
            n2824 = Bundle(w2189, w2192) -> (w2187:cluster{i32, i32})  [unwired: 1 in]
            n2825 = Add(x=w2203, y=w2200) -> (x+y=w2202:i32)
            n2826 = Add(x=w2180, y=w2181) -> (x+y=w2179:i32)
            n2827 = Bundle(w2201, w2203) -> (w2198:cluster{i32, i32})  [unwired: 1 in]
            n2828 = Bundle(w2178, w2180) -> (w2176:cluster{i32, i32})  [unwired: 1 in]
            n2829 = call <vilib>:"Move Pen.vi"("new position"=w2187, "picture"=w2146) -> ("new picture"=w2186:picture)  [unwired: 3 in]
            n2830 = Bundle(w2188, w2192) -> (w2190:cluster{i32, i32})  [unwired: 1 in]
            n2831 = Bundle(w2201, w2202) -> (w2199:cluster{i32, i32})  [unwired: 1 in]
            n2832 = Bundle(w2178, w2179) -> (w2177:cluster{i32, i32})  [unwired: 1 in]
            n2833 = call <vilib>:"Draw Line.vi"("picture"=w2186, "end point"=w2190, "color(black)"=u32 16448250, "pen"=T1 {"Width"=3, "Style"=enum."Solid"}) -> ("new picture"=w2142:picture)  [unwired: 5 in]
            n2834 = call <vilib>:"Move Pen.vi"("new position"=w2210, "picture"=w2142) -> ("new picture"=w2209:picture)  [unwired: 3 in]
            n2835 = call <vilib>:"Draw Line.vi"("picture"=w2209, "end point"=w2211, "color(black)"=u32 16448250, "pen"=T1 {"Width"=3, "Style"=enum."Solid"}) -> ("new picture"=w2141:picture)  [unwired: 5 in]
            n2836 = call <vilib>:"Move Pen.vi"("new position"=w2198, "picture"=w2141) -> ("new picture"=w2197:picture)  [unwired: 3 in]
            n2837 = call <vilib>:"Draw Line.vi"("picture"=w2197, "end point"=w2199, "color(black)"=u32 16448250, "pen"=T1 {"Width"=3, "Style"=enum."Solid"}) -> ("new picture"=w2140:picture)  [unwired: 5 in]
            n2838 = call <vilib>:"Move Pen.vi"("new position"=w2166, "picture"=w2140) -> ("new picture"=w2165:picture)  [unwired: 3 in]
            n2839 = call <vilib>:"Draw Line.vi"("picture"=w2165, "end point"=w2167, "color(black)"=u32 16448250, "pen"=T1 {"Width"=3, "Style"=enum."Solid"}) -> ("new picture"=w2139:picture)  [unwired: 5 in]
            n2840 = call <vilib>:"Move Pen.vi"("new position"=w2176, "picture"=w2139) -> ("new picture"=w2175:picture)  [unwired: 3 in]
            n2841 = call <vilib>:"Draw Line.vi"("picture"=w2175, "end point"=w2177, "color(black)"=u32 16448250, "pen"=T1 {"Width"=3, "Style"=enum."Solid"}) -> ("new picture"=w2138:picture)  [unwired: 5 in]
            n2842 = call <vilib>:"Move Pen.vi"("new position"=w2154, "picture"=w2138) -> ("new picture"=w2153:picture)  [unwired: 3 in]
            n2843 = call <vilib>:"Draw Line.vi"("picture"=w2153, "end point"=w2157, "color(black)"=u32 16448250, "pen"=T1 {"Width"=3, "Style"=enum."Solid"}) -> ("new picture"=w2137:picture)  [unwired: 5 in]
          }
          frame 9 {
            n2844 = Add(x=w2234, y=0) -> (x+y=w2278:i32)
            n2845 = Add(x=w2233, y=0) -> (x+y=w2279:i32)
            n2846 = Add(x=w2234, y=0) -> (x+y=w2290:i32)
            n2847 = Add(x=w2233, y=0) -> (x+y=w2291:i32)
            n2848 = Multiply(x=w2232, y=10) -> (x*y=w2277:i32)
            n2849 = Multiply(x=w2232, y=10) -> (x*y=w2288:i32)
            n2850 = Add(x=w2279, y=w2277) -> (x+y=w2280:i32)
            n2851 = Add(x=w2290, y=w2288) -> (x+y=w2289:i32)
            n2852 = Bundle(w2278, w2279) -> (w2275:cluster{i32, i32})  [unwired: 1 in]
            n2853 = Bundle(w2290, w2291) -> (w2287:cluster{i32, i32})  [unwired: 1 in]
            n2854 = Bundle(w2278, w2280) -> (w2276:cluster{i32, i32})  [unwired: 1 in]
            n2855 = call <vilib>:"Move Pen.vi"("new position"=w2287, "picture"=w2236) -> ("new picture"=w2286:picture)  [unwired: 3 in]
            n2856 = Bundle(w2289, w2291) -> (w2292:cluster{i32, i32})  [unwired: 1 in]
            n2857 = Multiply(x=w2232, y=10) -> (x*y=w2246:i32)
            n2858 = Add(x=w2234, y=w2246) -> (x+y=w2243:i32)
            n2859 = Add(x=w2233, y=w2246) -> (x+y=w2245:i32)
            n2860 = Add(x=w2245, y=w2246) -> (x+y=w2244:i32)
            n2861 = Bundle(w2243, w2245) -> (w2241:cluster{i32, i32})  [unwired: 1 in]
            n2862 = call <vilib>:"Draw Line.vi"("picture"=w2286, "end point"=w2292, "color(black)"=u32 16448250, "pen"=T1 {"Width"=3, "Style"=enum."Solid"}) -> ("new picture"=w2235:picture)  [unwired: 5 in]
            n2863 = Bundle(w2243, w2244) -> (w2242:cluster{i32, i32})  [unwired: 1 in]
            n2864 = Multiply(x=w2232, y=10) -> (x*y=w2265:i32)
            n2865 = Add(x=w2234, y=w2265) -> (x+y=w2266:i32)
            n2866 = Add(x=w2233, y=0) -> (x+y=w2268:i32)
            n2867 = Multiply(x=w2232, y=10) -> (x*y=w2256:i32)
            n2868 = Add(x=w2234, y=0) -> (x+y=w2254:i32)
            n2869 = Add(x=w2233, y=w2256) -> (x+y=w2257:i32)
            n2870 = Add(x=w2268, y=w2265) -> (x+y=w2267:i32)
            n2871 = Add(x=w2254, y=w2256) -> (x+y=w2253:i32)
            n2872 = Bundle(w2266, w2268) -> (w2263:cluster{i32, i32})  [unwired: 1 in]
            n2873 = Bundle(w2254, w2257) -> (w2252:cluster{i32, i32})  [unwired: 1 in]
            n2874 = Bundle(w2266, w2267) -> (w2264:cluster{i32, i32})  [unwired: 1 in]
            n2875 = call <vilib>:"Move Pen.vi"("new position"=w2252, "picture"=w2235) -> ("new picture"=w2251:picture)  [unwired: 3 in]
            n2876 = Bundle(w2253, w2257) -> (w2255:cluster{i32, i32})  [unwired: 1 in]
            n2877 = call <vilib>:"Draw Line.vi"("picture"=w2251, "end point"=w2255, "color(black)"=u32 16448250, "pen"=T1 {"Width"=3, "Style"=enum."Solid"}) -> ("new picture"=w2231:picture)  [unwired: 5 in]
            n2878 = call <vilib>:"Move Pen.vi"("new position"=w2275, "picture"=w2231) -> ("new picture"=w2274:picture)  [unwired: 3 in]
            n2879 = call <vilib>:"Draw Line.vi"("picture"=w2274, "end point"=w2276, "color(black)"=u32 16448250, "pen"=T1 {"Width"=3, "Style"=enum."Solid"}) -> ("new picture"=w2230:picture)  [unwired: 5 in]
            n2880 = call <vilib>:"Move Pen.vi"("new position"=w2263, "picture"=w2230) -> ("new picture"=w2262:picture)  [unwired: 3 in]
            n2881 = call <vilib>:"Draw Line.vi"("picture"=w2262, "end point"=w2264, "color(black)"=u32 16448250, "pen"=T1 {"Width"=3, "Style"=enum."Solid"}) -> ("new picture"=w2229:picture)  [unwired: 5 in]
            n2882 = call <vilib>:"Move Pen.vi"("new position"=w2241, "picture"=w2229) -> ("new picture"=w2240:picture)  [unwired: 3 in]
            n2883 = call <vilib>:"Draw Line.vi"("picture"=w2240, "end point"=w2242, "color(black)"=u32 16448250, "pen"=T1 {"Width"=3, "Style"=enum."Solid"}) -> ("new picture"=w2228:picture)  [unwired: 5 in]
          }
        }
        n2884 = local read "Sound playing"() -> (w221:bool)
        n2885 = local read "Voice File"() -> (w222:path)
        n2886 = case shown="True" w221 {
          tunnel: w222 -> [_ w5525]
          tunnel: w220 -> [_ w5524]
          tunnel: w219 -> [_ w5523]
          frame False {
          }
          frame True {
            n2887 = flat-sequence {
              tunnel: w5525 -> [w5530]
              tunnel: w5524 -> [w5529]
              tunnel: w5523 -> [w5528]
              frame #0 {
                n2888 = local read "Sample No. x"() -> (w5527:i32)
                n2889 = Increment(x=w5527) -> (x+1=w5526:i32)
                n2890 = local write "Sample No. x"(w5526) -> ()
              }
              frame #1 {
                w5532 = T7 0 items=["Absolute"=0, "Relative"=2] ("position mode")
                n2891 = local read "Sample No. x"() -> (w5535:i32)
                n2892 = Multiply(x=w5535, y=480) -> (x*y=w5533:i32)
                n2893 = call-poly <vilib>:"Sound File Open.vi"("path"=w5530) -> ("error out"=w5537:errorcluster, "sound file refnum"=w5540:T8)  [unwired: 9 in]
                n2894 = call-poly <vilib>:"Sound File Read.vi"("number of samples/ch (-1: all)"=480, "error in (no error)"=w5537, "position offset"=w5533, "position mode"=w5532, "sound file refnum"=w5540) -> ("error out"=w5531:errorcluster, "data"=w5539:waveform(dbl)[], "sound file refnum out"=w5538:T8)  [unwired: 2 in, 2 out]
                n2895 = call <vilib>:"Sound File Close.vi"("error in (no error)"=w5531, "sound file refnum"=w5538) -> ()  [unwired: 9 in, 1 out]
                n2896 = call-poly <vilib>:"Sound Output Write.vi"("error in (no error)"=w5529, "data"=w5539, "task ID"=w5528) -> ()  [unwired: 7 in, 2 out]
              }
            }
          }
        }
        n2897 = case shown="False" w111 {
          tunnel: w117 -> [_ w347]
          tunnel: w116 -> [_ w346]
          tunnel: w115 -> [w338 w345]
          tunnel: [w338 w339] -> w114
          frame False {
          }
          frame True {
            n2898 = case shown="2" w347 {
              tunnel: 640 -> [w1009 w1083 w1113 w1181 w1246 w1298 w1366 w1443 w1499 w1589]
              tunnel: 10 -> [w1008 w1082 w1112 w1180 w1245 w1297 w1365 w1442 w1498 w1588]
              tunnel: 3 -> [w1007 w1081 w1111 w1179 w1244 w1296 w1364 w1441 w1497 w1587]
              tunnel: w345 -> [w1010 w1085 w1115 w1182 w1247 w1300 w1368 w1445 w1501 w1582]
              tunnel: [w1001 w1080 w1107 w1174 w1240 w1292 w1359 w1438 w1491 w1583] -> w354
              frame 0, Default {
                n2899 = Add(x=w1009, y=0) -> (x+y=w1065:i32)
                n2900 = Add(x=w1008, y=0) -> (x+y=w1066:i32)
                n2901 = Multiply(x=w1007, y=10) -> (x*y=w1064:i32)
                n2902 = Add(x=w1009, y=0) -> (x+y=w1031:i32)
                n2903 = Multiply(x=w1007, y=10) -> (x*y=w1034:i32)
                n2904 = Add(x=w1008, y=w1034) -> (x+y=w1032:i32)
                n2905 = Add(x=w1066, y=w1064) -> (x+y=w1067:i32)
                n2906 = Add(x=w1032, y=w1034) -> (x+y=w1033:i32)
                n2907 = Bundle(w1065, w1066) -> (w1062:cluster{i32, i32})  [unwired: 1 in]
                n2908 = Bundle(w1031, w1032) -> (w1029:cluster{i32, i32})  [unwired: 1 in]
                n2909 = Bundle(w1065, w1067) -> (w1063:cluster{i32, i32})  [unwired: 1 in]
                n2910 = Bundle(w1031, w1033) -> (w1030:cluster{i32, i32})  [unwired: 1 in]
                n2911 = Multiply(x=w1007, y=10) -> (x*y=w1022:i32)
                n2912 = Multiply(x=2, y=w1022) -> (x*y=w1023:i32)
                n2913 = Add(x=w1009, y=0) -> (x+y=w1077:i32)
                n2914 = Add(x=w1008, y=0) -> (x+y=w1078:i32)
                n2915 = Add(x=w1009, y=0) -> (x+y=w1019:i32)
                n2916 = Add(x=w1008, y=w1023) -> (x+y=w1021:i32)
                n2917 = Multiply(x=w1007, y=10) -> (x*y=w1075:i32)
                n2918 = Add(x=w1019, y=w1022) -> (x+y=w1018:i32)
                n2919 = Add(x=w1077, y=w1075) -> (x+y=w1076:i32)
                n2920 = Bundle(w1077, w1078) -> (w1074:cluster{i32, i32})  [unwired: 1 in]
                n2921 = Bundle(w1019, w1021) -> (w1017:cluster{i32, i32})  [unwired: 1 in]
                n2922 = call <vilib>:"Move Pen.vi"("new position"=w1074, "picture"=w1010) -> ("new picture"=w1073:picture)  [unwired: 3 in]
                n2923 = Bundle(w1076, w1078) -> (w1079:cluster{i32, i32})  [unwired: 1 in]
                n2924 = Bundle(w1018, w1021) -> (w1020:cluster{i32, i32})  [unwired: 1 in]
                n2925 = Multiply(x=w1007, y=10) -> (x*y=w1052:i32)
                n2926 = Add(x=w1009, y=w1052) -> (x+y=w1053:i32)
                n2927 = Add(x=w1008, y=0) -> (x+y=w1055:i32)
                n2928 = Multiply(x=w1007, y=10) -> (x*y=w1044:i32)
                n2929 = Add(x=w1009, y=w1044) -> (x+y=w1041:i32)
                n2930 = Add(x=w1008, y=w1044) -> (x+y=w1043:i32)
                n2931 = Add(x=w1055, y=w1052) -> (x+y=w1054:i32)
                n2932 = Bundle(w1053, w1055) -> (w1050:cluster{i32, i32})  [unwired: 1 in]
                n2933 = call <vilib>:"Draw Line.vi"("picture"=w1073, "end point"=w1079, "color(black)"=u32 16448250, "pen"=T1 {"Width"=3, "Style"=enum."Solid"}) -> ("new picture"=w1006:picture)  [unwired: 5 in]
                n2934 = call <vilib>:"Move Pen.vi"("new position"=w1062, "picture"=w1006) -> ("new picture"=w1061:picture)  [unwired: 3 in]
                n2935 = call <vilib>:"Draw Line.vi"("picture"=w1061, "end point"=w1063, "color(black)"=u32 16448250, "pen"=T1 {"Width"=3, "Style"=enum."Solid"}) -> ("new picture"=w1005:picture)  [unwired: 5 in]
                n2936 = Add(x=w1043, y=w1044) -> (x+y=w1042:i32)
                n2937 = Bundle(w1041, w1043) -> (w1039:cluster{i32, i32})  [unwired: 1 in]
                n2938 = call <vilib>:"Move Pen.vi"("new position"=w1050, "picture"=w1005) -> ("new picture"=w1049:picture)  [unwired: 3 in]
                n2939 = Bundle(w1053, w1054) -> (w1051:cluster{i32, i32})  [unwired: 1 in]
                n2940 = Bundle(w1041, w1042) -> (w1040:cluster{i32, i32})  [unwired: 1 in]
                n2941 = call <vilib>:"Draw Line.vi"("picture"=w1049, "end point"=w1051, "color(black)"=u32 16448250, "pen"=T1 {"Width"=3, "Style"=enum."Solid"}) -> ("new picture"=w1004:picture)  [unwired: 5 in]
                n2942 = call <vilib>:"Move Pen.vi"("new position"=w1029, "picture"=w1004) -> ("new picture"=w1028:picture)  [unwired: 3 in]
                n2943 = call <vilib>:"Draw Line.vi"("picture"=w1028, "end point"=w1030, "color(black)"=u32 16448250, "pen"=T1 {"Width"=3, "Style"=enum."Solid"}) -> ("new picture"=w1003:picture)  [unwired: 5 in]
                n2944 = call <vilib>:"Move Pen.vi"("new position"=w1039, "picture"=w1003) -> ("new picture"=w1038:picture)  [unwired: 3 in]
                n2945 = call <vilib>:"Draw Line.vi"("picture"=w1038, "end point"=w1040, "color(black)"=u32 16448250, "pen"=T1 {"Width"=3, "Style"=enum."Solid"}) -> ("new picture"=w1002:picture)  [unwired: 5 in]
                n2946 = call <vilib>:"Move Pen.vi"("new position"=w1017, "picture"=w1002) -> ("new picture"=w1016:picture)  [unwired: 3 in]
                n2947 = call <vilib>:"Draw Line.vi"("picture"=w1016, "end point"=w1020, "color(black)"=u32 16448250, "pen"=T1 {"Width"=3, "Style"=enum."Solid"}) -> ("new picture"=w1001:picture)  [unwired: 5 in]
              }
              frame 1 {
                n2948 = Multiply(x=w1081, y=10) -> (x*y=w1103:i32)
                n2949 = Add(x=w1083, y=w1103) -> (x+y=w1104:i32)
                n2950 = Add(x=w1082, y=0) -> (x+y=w1106:i32)
                n2951 = Add(x=w1106, y=w1103) -> (x+y=w1105:i32)
                n2952 = Bundle(w1104, w1106) -> (w1101:cluster{i32, i32})  [unwired: 1 in]
                n2953 = call <vilib>:"Move Pen.vi"("new position"=w1101, "picture"=w1085) -> ("new picture"=w1100:picture)  [unwired: 3 in]
                n2954 = Bundle(w1104, w1105) -> (w1102:cluster{i32, i32})  [unwired: 1 in]
                n2955 = call <vilib>:"Draw Line.vi"("picture"=w1100, "end point"=w1102, "color(black)"=u32 16448250, "pen"=T1 {"Width"=3, "Style"=enum."Solid"}) -> ("new picture"=w1084:picture)  [unwired: 5 in]
                n2956 = Multiply(x=w1081, y=10) -> (x*y=w1095:i32)
                n2957 = Add(x=w1083, y=w1095) -> (x+y=w1092:i32)
                n2958 = Add(x=w1082, y=w1095) -> (x+y=w1094:i32)
                n2959 = Add(x=w1094, y=w1095) -> (x+y=w1093:i32)
                n2960 = Bundle(w1092, w1094) -> (w1090:cluster{i32, i32})  [unwired: 1 in]
                n2961 = call <vilib>:"Move Pen.vi"("new position"=w1090, "picture"=w1084) -> ("new picture"=w1089:picture)  [unwired: 3 in]
                n2962 = Bundle(w1092, w1093) -> (w1091:cluster{i32, i32})  [unwired: 1 in]
                n2963 = call <vilib>:"Draw Line.vi"("picture"=w1089, "end point"=w1091, "color(black)"=u32 16448250, "pen"=T1 {"Width"=3, "Style"=enum."Solid"}) -> ("new picture"=w1080:picture)  [unwired: 5 in]
              }
              frame 2 {
                n2964 = Multiply(x=w1111, y=10) -> (x*y=w1149:i32)
                n2965 = Add(x=w1113, y=0) -> (x+y=w1147:i32)
                n2966 = Add(x=w1112, y=w1149) -> (x+y=w1150:i32)
                n2967 = Add(x=w1113, y=0) -> (x+y=w1171:i32)
                n2968 = Add(x=w1112, y=0) -> (x+y=w1172:i32)
                n2969 = Multiply(x=w1111, y=10) -> (x*y=w1169:i32)
                n2970 = Add(x=w1147, y=w1149) -> (x+y=w1146:i32)
                n2971 = Add(x=w1171, y=w1169) -> (x+y=w1170:i32)
                n2972 = Bundle(w1147, w1150) -> (w1145:cluster{i32, i32})  [unwired: 1 in]
                n2973 = Bundle(w1171, w1172) -> (w1168:cluster{i32, i32})  [unwired: 1 in]
                n2974 = Bundle(w1146, w1150) -> (w1148:cluster{i32, i32})  [unwired: 1 in]
                n2975 = call <vilib>:"Move Pen.vi"("new position"=w1168, "picture"=w1115) -> ("new picture"=w1167:picture)  [unwired: 3 in]
                n2976 = Bundle(w1170, w1172) -> (w1173:cluster{i32, i32})  [unwired: 1 in]
                n2977 = Multiply(x=w1111, y=10) -> (x*y=w1127:i32)
                n2978 = Multiply(x=2, y=w1127) -> (x*y=w1128:i32)
                n2979 = Add(x=w1113, y=0) -> (x+y=w1124:i32)
                n2980 = Add(x=w1112, y=w1128) -> (x+y=w1126:i32)
                n2981 = Add(x=w1124, y=w1127) -> (x+y=w1123:i32)
                n2982 = Bundle(w1124, w1126) -> (w1122:cluster{i32, i32})  [unwired: 1 in]
                n2983 = call <vilib>:"Draw Line.vi"("picture"=w1167, "end point"=w1173, "color(black)"=u32 16448250, "pen"=T1 {"Width"=3, "Style"=enum."Solid"}) -> ("new picture"=w1114:picture)  [unwired: 5 in]
                n2984 = Bundle(w1123, w1126) -> (w1125:cluster{i32, i32})  [unwired: 1 in]
                n2985 = Multiply(x=w1111, y=10) -> (x*y=w1158:i32)
                n2986 = Add(x=w1113, y=0) -> (x+y=w1136:i32)
                n2987 = Add(x=w1113, y=w1158) -> (x+y=w1159:i32)
                n2988 = Add(x=w1112, y=0) -> (x+y=w1161:i32)
                n2989 = Multiply(x=w1111, y=10) -> (x*y=w1139:i32)
                n2990 = Add(x=w1112, y=w1139) -> (x+y=w1137:i32)
                n2991 = Add(x=w1137, y=w1139) -> (x+y=w1138:i32)
                n2992 = Add(x=w1161, y=w1158) -> (x+y=w1160:i32)
                n2993 = Bundle(w1136, w1137) -> (w1134:cluster{i32, i32})  [unwired: 1 in]
                n2994 = Bundle(w1159, w1161) -> (w1156:cluster{i32, i32})  [unwired: 1 in]
                n2995 = call <vilib>:"Move Pen.vi"("new position"=w1156, "picture"=w1114) -> ("new picture"=w1155:picture)  [unwired: 3 in]
                n2996 = Bundle(w1136, w1138) -> (w1135:cluster{i32, i32})  [unwired: 1 in]
                n2997 = Bundle(w1159, w1160) -> (w1157:cluster{i32, i32})  [unwired: 1 in]
                n2998 = call <vilib>:"Draw Line.vi"("picture"=w1155, "end point"=w1157, "color(black)"=u32 16448250, "pen"=T1 {"Width"=3, "Style"=enum."Solid"}) -> ("new picture"=w1110:picture)  [unwired: 5 in]
                n2999 = call <vilib>:"Move Pen.vi"("new position"=w1145, "picture"=w1110) -> ("new picture"=w1144:picture)  [unwired: 3 in]
                n3000 = call <vilib>:"Draw Line.vi"("picture"=w1144, "end point"=w1148, "color(black)"=u32 16448250, "pen"=T1 {"Width"=3, "Style"=enum."Solid"}) -> ("new picture"=w1109:picture)  [unwired: 5 in]
                n3001 = call <vilib>:"Move Pen.vi"("new position"=w1134, "picture"=w1109) -> ("new picture"=w1133:picture)  [unwired: 3 in]
                n3002 = call <vilib>:"Draw Line.vi"("picture"=w1133, "end point"=w1135, "color(black)"=u32 16448250, "pen"=T1 {"Width"=3, "Style"=enum."Solid"}) -> ("new picture"=w1108:picture)  [unwired: 5 in]
                n3003 = call <vilib>:"Move Pen.vi"("new position"=w1122, "picture"=w1108) -> ("new picture"=w1121:picture)  [unwired: 3 in]
                n3004 = call <vilib>:"Draw Line.vi"("picture"=w1121, "end point"=w1125, "color(black)"=u32 16448250, "pen"=T1 {"Width"=3, "Style"=enum."Solid"}) -> ("new picture"=w1107:picture)  [unwired: 5 in]
              }
              frame 3 {
                n3005 = Multiply(x=w1179, y=10) -> (x*y=w1215:i32)
                n3006 = Add(x=w1181, y=0) -> (x+y=w1213:i32)
                n3007 = Add(x=w1180, y=w1215) -> (x+y=w1216:i32)
                n3008 = Add(x=w1181, y=0) -> (x+y=w1237:i32)
                n3009 = Add(x=w1180, y=0) -> (x+y=w1238:i32)
                n3010 = Multiply(x=w1179, y=10) -> (x*y=w1235:i32)
                n3011 = Add(x=w1213, y=w1215) -> (x+y=w1212:i32)
                n3012 = Add(x=w1237, y=w1235) -> (x+y=w1236:i32)
                n3013 = Bundle(w1213, w1216) -> (w1211:cluster{i32, i32})  [unwired: 1 in]
                n3014 = Bundle(w1237, w1238) -> (w1234:cluster{i32, i32})  [unwired: 1 in]
                n3015 = call <vilib>:"Move Pen.vi"("new position"=w1234, "picture"=w1182) -> ("new picture"=w1233:picture)  [unwired: 3 in]
                n3016 = Bundle(w1212, w1216) -> (w1214:cluster{i32, i32})  [unwired: 1 in]
                n3017 = Bundle(w1236, w1238) -> (w1239:cluster{i32, i32})  [unwired: 1 in]
                n3018 = Multiply(x=w1179, y=10) -> (x*y=w1194:i32)
                n3019 = Multiply(x=2, y=w1194) -> (x*y=w1195:i32)
                n3020 = Add(x=w1181, y=0) -> (x+y=w1191:i32)
                n3021 = Add(x=w1180, y=w1195) -> (x+y=w1193:i32)
                n3022 = Add(x=w1191, y=w1194) -> (x+y=w1190:i32)
                n3023 = call <vilib>:"Draw Line.vi"("picture"=w1233, "end point"=w1239, "color(black)"=u32 16448250, "pen"=T1 {"Width"=3, "Style"=enum."Solid"}) -> ("new picture"=w1178:picture)  [unwired: 5 in]
                n3024 = Bundle(w1191, w1193) -> (w1189:cluster{i32, i32})  [unwired: 1 in]
                n3025 = Bundle(w1190, w1193) -> (w1192:cluster{i32, i32})  [unwired: 1 in]
                n3026 = Multiply(x=w1179, y=10) -> (x*y=w1205:i32)
                n3027 = Add(x=w1181, y=w1205) -> (x+y=w1202:i32)
                n3028 = Add(x=w1180, y=w1205) -> (x+y=w1204:i32)
                n3029 = Multiply(x=w1179, y=10) -> (x*y=w1224:i32)
                n3030 = Add(x=w1181, y=w1224) -> (x+y=w1225:i32)
                n3031 = Add(x=w1180, y=0) -> (x+y=w1227:i32)
                n3032 = Add(x=w1204, y=w1205) -> (x+y=w1203:i32)
                n3033 = Bundle(w1202, w1204) -> (w1200:cluster{i32, i32})  [unwired: 1 in]
                n3034 = Add(x=w1227, y=w1224) -> (x+y=w1226:i32)
                n3035 = Bundle(w1225, w1227) -> (w1222:cluster{i32, i32})  [unwired: 1 in]
                n3036 = Bundle(w1202, w1203) -> (w1201:cluster{i32, i32})  [unwired: 1 in]
                n3037 = call <vilib>:"Move Pen.vi"("new position"=w1222, "picture"=w1178) -> ("new picture"=w1221:picture)  [unwired: 3 in]
                n3038 = Bundle(w1225, w1226) -> (w1223:cluster{i32, i32})  [unwired: 1 in]
                n3039 = call <vilib>:"Draw Line.vi"("picture"=w1221, "end point"=w1223, "color(black)"=u32 16448250, "pen"=T1 {"Width"=3, "Style"=enum."Solid"}) -> ("new picture"=w1177:picture)  [unwired: 5 in]
                n3040 = call <vilib>:"Move Pen.vi"("new position"=w1211, "picture"=w1177) -> ("new picture"=w1210:picture)  [unwired: 3 in]
                n3041 = call <vilib>:"Draw Line.vi"("picture"=w1210, "end point"=w1214, "color(black)"=u32 16448250, "pen"=T1 {"Width"=3, "Style"=enum."Solid"}) -> ("new picture"=w1176:picture)  [unwired: 5 in]
                n3042 = call <vilib>:"Move Pen.vi"("new position"=w1200, "picture"=w1176) -> ("new picture"=w1199:picture)  [unwired: 3 in]
                n3043 = call <vilib>:"Draw Line.vi"("picture"=w1199, "end point"=w1201, "color(black)"=u32 16448250, "pen"=T1 {"Width"=3, "Style"=enum."Solid"}) -> ("new picture"=w1175:picture)  [unwired: 5 in]
                n3044 = call <vilib>:"Move Pen.vi"("new position"=w1189, "picture"=w1175) -> ("new picture"=w1188:picture)  [unwired: 3 in]
                n3045 = call <vilib>:"Draw Line.vi"("picture"=w1188, "end point"=w1192, "color(black)"=u32 16448250, "pen"=T1 {"Width"=3, "Style"=enum."Solid"}) -> ("new picture"=w1174:picture)  [unwired: 5 in]
              }
              frame 4 {
                n3046 = Add(x=w1246, y=0) -> (x+y=w1289:i32)
                n3047 = Add(x=w1245, y=0) -> (x+y=w1290:i32)
                n3048 = Multiply(x=w1244, y=10) -> (x*y=w1288:i32)
                n3049 = Add(x=w1290, y=w1288) -> (x+y=w1291:i32)
                n3050 = Bundle(w1289, w1290) -> (w1286:cluster{i32, i32})  [unwired: 1 in]
                n3051 = call <vilib>:"Move Pen.vi"("new position"=w1286, "picture"=w1247) -> ("new picture"=w1285:picture)  [unwired: 3 in]
                n3052 = Bundle(w1289, w1291) -> (w1287:cluster{i32, i32})  [unwired: 1 in]
                n3053 = Multiply(x=w1244, y=10) -> (x*y=w1267:i32)
                n3054 = Add(x=w1246, y=0) -> (x+y=w1265:i32)
                n3055 = Add(x=w1245, y=w1267) -> (x+y=w1268:i32)
                n3056 = Add(x=w1265, y=w1267) -> (x+y=w1264:i32)
                n3057 = Bundle(w1265, w1268) -> (w1263:cluster{i32, i32})  [unwired: 1 in]
                n3058 = call <vilib>:"Draw Line.vi"("picture"=w1285, "end point"=w1287, "color(black)"=u32 16448250, "pen"=T1 {"Width"=3, "Style"=enum."Solid"}) -> ("new picture"=w1241:picture)  [unwired: 5 in]
                n3059 = Multiply(x=w1244, y=10) -> (x*y=w1257:i32)
                n3060 = Add(x=w1246, y=w1257) -> (x+y=w1254:i32)
                n3061 = Add(x=w1245, y=w1257) -> (x+y=w1256:i32)
                n3062 = Bundle(w1264, w1268) -> (w1266:cluster{i32, i32})  [unwired: 1 in]
                n3063 = Add(x=w1256, y=w1257) -> (x+y=w1255:i32)
                n3064 = Bundle(w1254, w1256) -> (w1252:cluster{i32, i32})  [unwired: 1 in]
                n3065 = Multiply(x=w1244, y=10) -> (x*y=w1276:i32)
                n3066 = Add(x=w1246, y=w1276) -> (x+y=w1277:i32)
                n3067 = Add(x=w1245, y=0) -> (x+y=w1279:i32)
                n3068 = Add(x=w1279, y=w1276) -> (x+y=w1278:i32)
                n3069 = Bundle(w1254, w1255) -> (w1253:cluster{i32, i32})  [unwired: 1 in]
                n3070 = Bundle(w1277, w1279) -> (w1274:cluster{i32, i32})  [unwired: 1 in]
                n3071 = call <vilib>:"Move Pen.vi"("new position"=w1274, "picture"=w1241) -> ("new picture"=w1273:picture)  [unwired: 3 in]
                n3072 = Bundle(w1277, w1278) -> (w1275:cluster{i32, i32})  [unwired: 1 in]
                n3073 = call <vilib>:"Draw Line.vi"("picture"=w1273, "end point"=w1275, "color(black)"=u32 16448250, "pen"=T1 {"Width"=3, "Style"=enum."Solid"}) -> ("new picture"=w1243:picture)  [unwired: 5 in]
                n3074 = call <vilib>:"Move Pen.vi"("new position"=w1263, "picture"=w1243) -> ("new picture"=w1262:picture)  [unwired: 3 in]
                n3075 = call <vilib>:"Draw Line.vi"("picture"=w1262, "end point"=w1266, "color(black)"=u32 16448250, "pen"=T1 {"Width"=3, "Style"=enum."Solid"}) -> ("new picture"=w1242:picture)  [unwired: 5 in]
                n3076 = call <vilib>:"Move Pen.vi"("new position"=w1252, "picture"=w1242) -> ("new picture"=w1251:picture)  [unwired: 3 in]
                n3077 = call <vilib>:"Draw Line.vi"("picture"=w1251, "end point"=w1253, "color(black)"=u32 16448250, "pen"=T1 {"Width"=3, "Style"=enum."Solid"}) -> ("new picture"=w1240:picture)  [unwired: 5 in]
              }
              frame 5 {
                n3078 = Multiply(x=w1296, y=10) -> (x*y=w1333:i32)
                n3079 = Add(x=w1298, y=0) -> (x+y=w1331:i32)
                n3080 = Add(x=w1297, y=w1333) -> (x+y=w1334:i32)
                n3081 = Add(x=w1298, y=0) -> (x+y=w1356:i32)
                n3082 = Add(x=w1297, y=0) -> (x+y=w1357:i32)
                n3083 = Add(x=w1331, y=w1333) -> (x+y=w1330:i32)
                n3084 = Multiply(x=w1296, y=10) -> (x*y=w1354:i32)
                n3085 = Bundle(w1331, w1334) -> (w1329:cluster{i32, i32})  [unwired: 1 in]
                n3086 = Add(x=w1356, y=w1354) -> (x+y=w1355:i32)
                n3087 = Bundle(w1356, w1357) -> (w1353:cluster{i32, i32})  [unwired: 1 in]
                n3088 = Bundle(w1330, w1334) -> (w1332:cluster{i32, i32})  [unwired: 1 in]
                n3089 = call <vilib>:"Move Pen.vi"("new position"=w1353, "picture"=w1300) -> ("new picture"=w1352:picture)  [unwired: 3 in]
                n3090 = Bundle(w1355, w1357) -> (w1358:cluster{i32, i32})  [unwired: 1 in]
                n3091 = Multiply(x=w1296, y=10) -> (x*y=w1312:i32)
                n3092 = Multiply(x=2, y=w1312) -> (x*y=w1313:i32)
                n3093 = Add(x=w1298, y=0) -> (x+y=w1309:i32)
                n3094 = Add(x=w1297, y=w1313) -> (x+y=w1311:i32)
                n3095 = Add(x=w1309, y=w1312) -> (x+y=w1308:i32)
                n3096 = Bundle(w1309, w1311) -> (w1307:cluster{i32, i32})  [unwired: 1 in]
                n3097 = call <vilib>:"Draw Line.vi"("picture"=w1352, "end point"=w1358, "color(black)"=u32 16448250, "pen"=T1 {"Width"=3, "Style"=enum."Solid"}) -> ("new picture"=w1299:picture)  [unwired: 5 in]
                n3098 = Bundle(w1308, w1311) -> (w1310:cluster{i32, i32})  [unwired: 1 in]
                n3099 = Multiply(x=w1296, y=10) -> (x*y=w1323:i32)
                n3100 = Add(x=w1298, y=0) -> (x+y=w1344:i32)
                n3101 = Add(x=w1297, y=0) -> (x+y=w1345:i32)
                n3102 = Add(x=w1298, y=w1323) -> (x+y=w1320:i32)
                n3103 = Add(x=w1297, y=w1323) -> (x+y=w1322:i32)
                n3104 = Multiply(x=w1296, y=10) -> (x*y=w1343:i32)
                n3105 = Add(x=w1345, y=w1343) -> (x+y=w1346:i32)
                n3106 = Add(x=w1322, y=w1323) -> (x+y=w1321:i32)
                n3107 = Bundle(w1344, w1345) -> (w1341:cluster{i32, i32})  [unwired: 1 in]
                n3108 = Bundle(w1320, w1322) -> (w1318:cluster{i32, i32})  [unwired: 1 in]
                n3109 = call <vilib>:"Move Pen.vi"("new position"=w1341, "picture"=w1299) -> ("new picture"=w1340:picture)  [unwired: 3 in]
                n3110 = Bundle(w1344, w1346) -> (w1342:cluster{i32, i32})  [unwired: 1 in]
                n3111 = Bundle(w1320, w1321) -> (w1319:cluster{i32, i32})  [unwired: 1 in]
                n3112 = call <vilib>:"Draw Line.vi"("picture"=w1340, "end point"=w1342, "color(black)"=u32 16448250, "pen"=T1 {"Width"=3, "Style"=enum."Solid"}) -> ("new picture"=w1295:picture)  [unwired: 5 in]
                n3113 = call <vilib>:"Move Pen.vi"("new position"=w1329, "picture"=w1295) -> ("new picture"=w1328:picture)  [unwired: 3 in]
                n3114 = call <vilib>:"Draw Line.vi"("picture"=w1328, "end point"=w1332, "color(black)"=u32 16448250, "pen"=T1 {"Width"=3, "Style"=enum."Solid"}) -> ("new picture"=w1294:picture)  [unwired: 5 in]
                n3115 = call <vilib>:"Move Pen.vi"("new position"=w1318, "picture"=w1294) -> ("new picture"=w1317:picture)  [unwired: 3 in]
                n3116 = call <vilib>:"Draw Line.vi"("picture"=w1317, "end point"=w1319, "color(black)"=u32 16448250, "pen"=T1 {"Width"=3, "Style"=enum."Solid"}) -> ("new picture"=w1293:picture)  [unwired: 5 in]
                n3117 = call <vilib>:"Move Pen.vi"("new position"=w1307, "picture"=w1293) -> ("new picture"=w1306:picture)  [unwired: 3 in]
                n3118 = call <vilib>:"Draw Line.vi"("picture"=w1306, "end point"=w1310, "color(black)"=u32 16448250, "pen"=T1 {"Width"=3, "Style"=enum."Solid"}) -> ("new picture"=w1292:picture)  [unwired: 5 in]
              }
              frame 6 {
                n3119 = Multiply(x=w1364, y=10) -> (x*y=w1402:i32)
                n3120 = Multiply(x=w1364, y=10) -> (x*y=w1412:i32)
                n3121 = Add(x=w1366, y=w1402) -> (x+y=w1399:i32)
                n3122 = Add(x=w1365, y=w1402) -> (x+y=w1401:i32)
                n3123 = Add(x=w1366, y=0) -> (x+y=w1410:i32)
                n3124 = Add(x=w1365, y=w1412) -> (x+y=w1413:i32)
                n3125 = Add(x=w1366, y=0) -> (x+y=w1435:i32)
                n3126 = Add(x=w1365, y=0) -> (x+y=w1436:i32)
                n3127 = Multiply(x=w1364, y=10) -> (x*y=w1433:i32)
                n3128 = Add(x=w1410, y=w1412) -> (x+y=w1409:i32)
                n3129 = Add(x=w1401, y=w1402) -> (x+y=w1400:i32)
                n3130 = Bundle(w1399, w1401) -> (w1397:cluster{i32, i32})  [unwired: 1 in]
                n3131 = Bundle(w1410, w1413) -> (w1408:cluster{i32, i32})  [unwired: 1 in]
                n3132 = Add(x=w1435, y=w1433) -> (x+y=w1434:i32)
                n3133 = Bundle(w1435, w1436) -> (w1432:cluster{i32, i32})  [unwired: 1 in]
                n3134 = Bundle(w1399, w1400) -> (w1398:cluster{i32, i32})  [unwired: 1 in]
                n3135 = Bundle(w1409, w1413) -> (w1411:cluster{i32, i32})  [unwired: 1 in]
                n3136 = call <vilib>:"Move Pen.vi"("new position"=w1432, "picture"=w1368) -> ("new picture"=w1431:picture)  [unwired: 3 in]
                n3137 = Bundle(w1434, w1436) -> (w1437:cluster{i32, i32})  [unwired: 1 in]
                n3138 = call <vilib>:"Draw Line.vi"("picture"=w1431, "end point"=w1437, "color(black)"=u32 16448250, "pen"=T1 {"Width"=3, "Style"=enum."Solid"}) -> ("new picture"=w1367:picture)  [unwired: 5 in]
                n3139 = Multiply(x=w1364, y=10) -> (x*y=w1380:i32)
                n3140 = Multiply(x=2, y=w1380) -> (x*y=w1381:i32)
                n3141 = Add(x=w1366, y=0) -> (x+y=w1389:i32)
                n3142 = Multiply(x=w1364, y=10) -> (x*y=w1392:i32)
                n3143 = Add(x=w1365, y=w1392) -> (x+y=w1390:i32)
                n3144 = Add(x=w1366, y=0) -> (x+y=w1377:i32)
                n3145 = Add(x=w1365, y=w1381) -> (x+y=w1379:i32)
                n3146 = Add(x=w1366, y=0) -> (x+y=w1423:i32)
                n3147 = Add(x=w1365, y=0) -> (x+y=w1424:i32)
                n3148 = Multiply(x=w1364, y=10) -> (x*y=w1422:i32)
                n3149 = Add(x=w1390, y=w1392) -> (x+y=w1391:i32)
                n3150 = Add(x=w1377, y=w1380) -> (x+y=w1376:i32)
                n3151 = Add(x=w1424, y=w1422) -> (x+y=w1425:i32)
                n3152 = Bundle(w1389, w1390) -> (w1387:cluster{i32, i32})  [unwired: 1 in]
                n3153 = Bundle(w1377, w1379) -> (w1375:cluster{i32, i32})  [unwired: 1 in]
                n3154 = Bundle(w1423, w1424) -> (w1420:cluster{i32, i32})  [unwired: 1 in]
                n3155 = Bundle(w1389, w1391) -> (w1388:cluster{i32, i32})  [unwired: 1 in]
                n3156 = Bundle(w1376, w1379) -> (w1378:cluster{i32, i32})  [unwired: 1 in]
                n3157 = call <vilib>:"Move Pen.vi"("new position"=w1420, "picture"=w1367) -> ("new picture"=w1419:picture)  [unwired: 3 in]
                n3158 = Bundle(w1423, w1425) -> (w1421:cluster{i32, i32})  [unwired: 1 in]
                n3159 = call <vilib>:"Draw Line.vi"("picture"=w1419, "end point"=w1421, "color(black)"=u32 16448250, "pen"=T1 {"Width"=3, "Style"=enum."Solid"}) -> ("new picture"=w1363:picture)  [unwired: 5 in]
                n3160 = call <vilib>:"Move Pen.vi"("new position"=w1408, "picture"=w1363) -> ("new picture"=w1407:picture)  [unwired: 3 in]
                n3161 = call <vilib>:"Draw Line.vi"("picture"=w1407, "end point"=w1411, "color(black)"=u32 16448250, "pen"=T1 {"Width"=3, "Style"=enum."Solid"}) -> ("new picture"=w1362:picture)  [unwired: 5 in]
                n3162 = call <vilib>:"Move Pen.vi"("new position"=w1387, "picture"=w1362) -> ("new picture"=w1386:picture)  [unwired: 3 in]
                n3163 = call <vilib>:"Draw Line.vi"("picture"=w1386, "end point"=w1388, "color(black)"=u32 16448250, "pen"=T1 {"Width"=3, "Style"=enum."Solid"}) -> ("new picture"=w1361:picture)  [unwired: 5 in]
                n3164 = call <vilib>:"Move Pen.vi"("new position"=w1397, "picture"=w1361) -> ("new picture"=w1396:picture)  [unwired: 3 in]
                n3165 = call <vilib>:"Draw Line.vi"("picture"=w1396, "end point"=w1398, "color(black)"=u32 16448250, "pen"=T1 {"Width"=3, "Style"=enum."Solid"}) -> ("new picture"=w1360:picture)  [unwired: 5 in]
                n3166 = call <vilib>:"Move Pen.vi"("new position"=w1375, "picture"=w1360) -> ("new picture"=w1374:picture)  [unwired: 3 in]
                n3167 = call <vilib>:"Draw Line.vi"("picture"=w1374, "end point"=w1378, "color(black)"=u32 16448250, "pen"=T1 {"Width"=3, "Style"=enum."Solid"}) -> ("new picture"=w1359:picture)  [unwired: 5 in]
              }
              frame 7 {
                n3168 = Add(x=w1443, y=0) -> (x+y=w1476:i32)
                n3169 = Add(x=w1442, y=0) -> (x+y=w1477:i32)
                n3170 = Multiply(x=w1441, y=10) -> (x*y=w1475:i32)
                n3171 = Add(x=w1477, y=w1475) -> (x+y=w1478:i32)
                n3172 = Add(x=w1443, y=0) -> (x+y=w1488:i32)
                n3173 = Add(x=w1442, y=0) -> (x+y=w1489:i32)
                n3174 = Bundle(w1476, w1477) -> (w1473:cluster{i32, i32})  [unwired: 1 in]
                n3175 = Multiply(x=w1441, y=10) -> (x*y=w1486:i32)
                n3176 = Add(x=w1488, y=w1486) -> (x+y=w1487:i32)
                n3177 = Bundle(w1488, w1489) -> (w1485:cluster{i32, i32})  [unwired: 1 in]
                n3178 = Bundle(w1476, w1478) -> (w1474:cluster{i32, i32})  [unwired: 1 in]
                n3179 = call <vilib>:"Move Pen.vi"("new position"=w1485, "picture"=w1445) -> ("new picture"=w1484:picture)  [unwired: 3 in]
                n3180 = Bundle(w1487, w1489) -> (w1490:cluster{i32, i32})  [unwired: 1 in]
                n3181 = call <vilib>:"Draw Line.vi"("picture"=w1484, "end point"=w1490, "color(black)"=u32 16448250, "pen"=T1 {"Width"=3, "Style"=enum."Solid"}) -> ("new picture"=w1444:picture)  [unwired: 5 in]
                n3182 = Multiply(x=w1441, y=10) -> (x*y=w1463:i32)
                n3183 = Add(x=w1443, y=w1463) -> (x+y=w1464:i32)
                n3184 = Add(x=w1442, y=0) -> (x+y=w1466:i32)
                n3185 = Multiply(x=w1441, y=10) -> (x*y=w1455:i32)
                n3186 = Add(x=w1443, y=w1455) -> (x+y=w1452:i32)
                n3187 = Add(x=w1442, y=w1455) -> (x+y=w1454:i32)
                n3188 = Add(x=w1466, y=w1463) -> (x+y=w1465:i32)
                n3189 = Bundle(w1464, w1466) -> (w1461:cluster{i32, i32})  [unwired: 1 in]
                n3190 = Add(x=w1454, y=w1455) -> (x+y=w1453:i32)
                n3191 = Bundle(w1452, w1454) -> (w1450:cluster{i32, i32})  [unwired: 1 in]
                n3192 = Bundle(w1464, w1465) -> (w1462:cluster{i32, i32})  [unwired: 1 in]
                n3193 = call <vilib>:"Move Pen.vi"("new position"=w1450, "picture"=w1444) -> ("new picture"=w1449:picture)  [unwired: 3 in]
                n3194 = Bundle(w1452, w1453) -> (w1451:cluster{i32, i32})  [unwired: 1 in]
                n3195 = call <vilib>:"Draw Line.vi"("picture"=w1449, "end point"=w1451, "color(black)"=u32 16448250, "pen"=T1 {"Width"=3, "Style"=enum."Solid"}) -> ("new picture"=w1440:picture)  [unwired: 5 in]
                n3196 = call <vilib>:"Move Pen.vi"("new position"=w1473, "picture"=w1440) -> ("new picture"=w1472:picture)  [unwired: 3 in]
                n3197 = call <vilib>:"Draw Line.vi"("picture"=w1472, "end point"=w1474, "color(black)"=u32 16448250, "pen"=T1 {"Width"=3, "Style"=enum."Solid"}) -> ("new picture"=w1439:picture)  [unwired: 5 in]
                n3198 = call <vilib>:"Move Pen.vi"("new position"=w1461, "picture"=w1439) -> ("new picture"=w1460:picture)  [unwired: 3 in]
                n3199 = call <vilib>:"Draw Line.vi"("picture"=w1460, "end point"=w1462, "color(black)"=u32 16448250, "pen"=T1 {"Width"=3, "Style"=enum."Solid"}) -> ("new picture"=w1438:picture)  [unwired: 5 in]
              }
              frame 8 {
                n3200 = Add(x=w1499, y=0) -> (x+y=w1567:i32)
                n3201 = Add(x=w1498, y=0) -> (x+y=w1568:i32)
                n3202 = Add(x=w1499, y=0) -> (x+y=w1522:i32)
                n3203 = Multiply(x=w1497, y=10) -> (x*y=w1566:i32)
                n3204 = Multiply(x=w1497, y=10) -> (x*y=w1525:i32)
                n3205 = Add(x=w1498, y=w1525) -> (x+y=w1523:i32)
                n3206 = Add(x=w1499, y=0) -> (x+y=w1579:i32)
                n3207 = Add(x=w1498, y=0) -> (x+y=w1580:i32)
                n3208 = Multiply(x=w1497, y=10) -> (x*y=w1577:i32)
                n3209 = Add(x=w1568, y=w1566) -> (x+y=w1569:i32)
                n3210 = Add(x=w1523, y=w1525) -> (x+y=w1524:i32)
                n3211 = Bundle(w1567, w1568) -> (w1564:cluster{i32, i32})  [unwired: 1 in]
                n3212 = Bundle(w1522, w1523) -> (w1520:cluster{i32, i32})  [unwired: 1 in]
                n3213 = Multiply(x=w1497, y=10) -> (x*y=w1513:i32)
                n3214 = Multiply(x=2, y=w1513) -> (x*y=w1514:i32)
                n3215 = Add(x=w1579, y=w1577) -> (x+y=w1578:i32)
                n3216 = Bundle(w1579, w1580) -> (w1576:cluster{i32, i32})  [unwired: 1 in]
                n3217 = Add(x=w1499, y=0) -> (x+y=w1510:i32)
                n3218 = Add(x=w1498, y=w1514) -> (x+y=w1512:i32)
                n3219 = Add(x=w1510, y=w1513) -> (x+y=w1509:i32)
                n3220 = Bundle(w1567, w1569) -> (w1565:cluster{i32, i32})  [unwired: 1 in]
                n3221 = Bundle(w1522, w1524) -> (w1521:cluster{i32, i32})  [unwired: 1 in]
                n3222 = Bundle(w1510, w1512) -> (w1508:cluster{i32, i32})  [unwired: 1 in]
                n3223 = call <vilib>:"Move Pen.vi"("new position"=w1576, "picture"=w1501) -> ("new picture"=w1575:picture)  [unwired: 3 in]
                n3224 = Bundle(w1578, w1580) -> (w1581:cluster{i32, i32})  [unwired: 1 in]
                n3225 = Bundle(w1509, w1512) -> (w1511:cluster{i32, i32})  [unwired: 1 in]
                n3226 = call <vilib>:"Draw Line.vi"("picture"=w1575, "end point"=w1581, "color(black)"=u32 16448250, "pen"=T1 {"Width"=3, "Style"=enum."Solid"}) -> ("new picture"=w1500:picture)  [unwired: 5 in]
                n3227 = Multiply(x=w1497, y=10) -> (x*y=w1545:i32)
                n3228 = Multiply(x=w1497, y=10) -> (x*y=w1554:i32)
                n3229 = Add(x=w1499, y=0) -> (x+y=w1543:i32)
                n3230 = Multiply(x=w1497, y=10) -> (x*y=w1535:i32)
                n3231 = Add(x=w1498, y=w1545) -> (x+y=w1546:i32)
                n3232 = Add(x=w1499, y=w1554) -> (x+y=w1555:i32)
                n3233 = Add(x=w1498, y=0) -> (x+y=w1557:i32)
                n3234 = Add(x=w1499, y=w1535) -> (x+y=w1532:i32)
                n3235 = Add(x=w1498, y=w1535) -> (x+y=w1534:i32)
                n3236 = Add(x=w1543, y=w1545) -> (x+y=w1542:i32)
                n3237 = Bundle(w1543, w1546) -> (w1541:cluster{i32, i32})  [unwired: 1 in]
                n3238 = Add(x=w1557, y=w1554) -> (x+y=w1556:i32)
                n3239 = Add(x=w1534, y=w1535) -> (x+y=w1533:i32)
                n3240 = Bundle(w1555, w1557) -> (w1552:cluster{i32, i32})  [unwired: 1 in]
                n3241 = Bundle(w1532, w1534) -> (w1530:cluster{i32, i32})  [unwired: 1 in]
                n3242 = call <vilib>:"Move Pen.vi"("new position"=w1541, "picture"=w1500) -> ("new picture"=w1540:picture)  [unwired: 3 in]
                n3243 = Bundle(w1542, w1546) -> (w1544:cluster{i32, i32})  [unwired: 1 in]
                n3244 = Bundle(w1555, w1556) -> (w1553:cluster{i32, i32})  [unwired: 1 in]
                n3245 = Bundle(w1532, w1533) -> (w1531:cluster{i32, i32})  [unwired: 1 in]
                n3246 = call <vilib>:"Draw Line.vi"("picture"=w1540, "end point"=w1544, "color(black)"=u32 16448250, "pen"=T1 {"Width"=3, "Style"=enum."Solid"}) -> ("new picture"=w1496:picture)  [unwired: 5 in]
                n3247 = call <vilib>:"Move Pen.vi"("new position"=w1564, "picture"=w1496) -> ("new picture"=w1563:picture)  [unwired: 3 in]
                n3248 = call <vilib>:"Draw Line.vi"("picture"=w1563, "end point"=w1565, "color(black)"=u32 16448250, "pen"=T1 {"Width"=3, "Style"=enum."Solid"}) -> ("new picture"=w1495:picture)  [unwired: 5 in]
                n3249 = call <vilib>:"Move Pen.vi"("new position"=w1552, "picture"=w1495) -> ("new picture"=w1551:picture)  [unwired: 3 in]
                n3250 = call <vilib>:"Draw Line.vi"("picture"=w1551, "end point"=w1553, "color(black)"=u32 16448250, "pen"=T1 {"Width"=3, "Style"=enum."Solid"}) -> ("new picture"=w1494:picture)  [unwired: 5 in]
                n3251 = call <vilib>:"Move Pen.vi"("new position"=w1520, "picture"=w1494) -> ("new picture"=w1519:picture)  [unwired: 3 in]
                n3252 = call <vilib>:"Draw Line.vi"("picture"=w1519, "end point"=w1521, "color(black)"=u32 16448250, "pen"=T1 {"Width"=3, "Style"=enum."Solid"}) -> ("new picture"=w1493:picture)  [unwired: 5 in]
                n3253 = call <vilib>:"Move Pen.vi"("new position"=w1530, "picture"=w1493) -> ("new picture"=w1529:picture)  [unwired: 3 in]
                n3254 = call <vilib>:"Draw Line.vi"("picture"=w1529, "end point"=w1531, "color(black)"=u32 16448250, "pen"=T1 {"Width"=3, "Style"=enum."Solid"}) -> ("new picture"=w1492:picture)  [unwired: 5 in]
                n3255 = call <vilib>:"Move Pen.vi"("new position"=w1508, "picture"=w1492) -> ("new picture"=w1507:picture)  [unwired: 3 in]
                n3256 = call <vilib>:"Draw Line.vi"("picture"=w1507, "end point"=w1511, "color(black)"=u32 16448250, "pen"=T1 {"Width"=3, "Style"=enum."Solid"}) -> ("new picture"=w1491:picture)  [unwired: 5 in]
              }
              frame 9 {
                n3257 = Add(x=w1589, y=0) -> (x+y=w1632:i32)
                n3258 = Add(x=w1588, y=0) -> (x+y=w1633:i32)
                n3259 = Add(x=w1589, y=0) -> (x+y=w1644:i32)
                n3260 = Add(x=w1588, y=0) -> (x+y=w1645:i32)
                n3261 = Multiply(x=w1587, y=10) -> (x*y=w1631:i32)
                n3262 = Multiply(x=w1587, y=10) -> (x*y=w1642:i32)
                n3263 = Add(x=w1633, y=w1631) -> (x+y=w1634:i32)
                n3264 = Add(x=w1644, y=w1642) -> (x+y=w1643:i32)
                n3265 = Bundle(w1632, w1633) -> (w1629:cluster{i32, i32})  [unwired: 1 in]
                n3266 = Bundle(w1644, w1645) -> (w1641:cluster{i32, i32})  [unwired: 1 in]
                n3267 = Bundle(w1632, w1634) -> (w1630:cluster{i32, i32})  [unwired: 1 in]
                n3268 = call <vilib>:"Move Pen.vi"("new position"=w1641, "picture"=w1582) -> ("new picture"=w1640:picture)  [unwired: 3 in]
                n3269 = Bundle(w1643, w1645) -> (w1646:cluster{i32, i32})  [unwired: 1 in]
                n3270 = Multiply(x=w1587, y=10) -> (x*y=w1600:i32)
                n3271 = Add(x=w1589, y=w1600) -> (x+y=w1597:i32)
                n3272 = Add(x=w1588, y=w1600) -> (x+y=w1599:i32)
                n3273 = Add(x=w1599, y=w1600) -> (x+y=w1598:i32)
                n3274 = Bundle(w1597, w1599) -> (w1595:cluster{i32, i32})  [unwired: 1 in]
                n3275 = call <vilib>:"Draw Line.vi"("picture"=w1640, "end point"=w1646, "color(black)"=u32 16448250, "pen"=T1 {"Width"=3, "Style"=enum."Solid"}) -> ("new picture"=w1590:picture)  [unwired: 5 in]
                n3276 = Bundle(w1597, w1598) -> (w1596:cluster{i32, i32})  [unwired: 1 in]
                n3277 = Multiply(x=w1587, y=10) -> (x*y=w1619:i32)
                n3278 = Add(x=w1589, y=w1619) -> (x+y=w1620:i32)
                n3279 = Add(x=w1588, y=0) -> (x+y=w1622:i32)
                n3280 = Multiply(x=w1587, y=10) -> (x*y=w1610:i32)
                n3281 = Add(x=w1589, y=0) -> (x+y=w1608:i32)
                n3282 = Add(x=w1588, y=w1610) -> (x+y=w1611:i32)
                n3283 = Add(x=w1622, y=w1619) -> (x+y=w1621:i32)
                n3284 = Add(x=w1608, y=w1610) -> (x+y=w1607:i32)
                n3285 = Bundle(w1620, w1622) -> (w1617:cluster{i32, i32})  [unwired: 1 in]
                n3286 = Bundle(w1608, w1611) -> (w1606:cluster{i32, i32})  [unwired: 1 in]
                n3287 = Bundle(w1620, w1621) -> (w1618:cluster{i32, i32})  [unwired: 1 in]
                n3288 = call <vilib>:"Move Pen.vi"("new position"=w1606, "picture"=w1590) -> ("new picture"=w1605:picture)  [unwired: 3 in]
                n3289 = Bundle(w1607, w1611) -> (w1609:cluster{i32, i32})  [unwired: 1 in]
                n3290 = call <vilib>:"Draw Line.vi"("picture"=w1605, "end point"=w1609, "color(black)"=u32 16448250, "pen"=T1 {"Width"=3, "Style"=enum."Solid"}) -> ("new picture"=w1586:picture)  [unwired: 5 in]
                n3291 = call <vilib>:"Move Pen.vi"("new position"=w1629, "picture"=w1586) -> ("new picture"=w1628:picture)  [unwired: 3 in]
                n3292 = call <vilib>:"Draw Line.vi"("picture"=w1628, "end point"=w1630, "color(black)"=u32 16448250, "pen"=T1 {"Width"=3, "Style"=enum."Solid"}) -> ("new picture"=w1585:picture)  [unwired: 5 in]
                n3293 = call <vilib>:"Move Pen.vi"("new position"=w1617, "picture"=w1585) -> ("new picture"=w1616:picture)  [unwired: 3 in]
                n3294 = call <vilib>:"Draw Line.vi"("picture"=w1616, "end point"=w1618, "color(black)"=u32 16448250, "pen"=T1 {"Width"=3, "Style"=enum."Solid"}) -> ("new picture"=w1584:picture)  [unwired: 5 in]
                n3295 = call <vilib>:"Move Pen.vi"("new position"=w1595, "picture"=w1584) -> ("new picture"=w1594:picture)  [unwired: 3 in]
                n3296 = call <vilib>:"Draw Line.vi"("picture"=w1594, "end point"=w1596, "color(black)"=u32 16448250, "pen"=T1 {"Width"=3, "Style"=enum."Solid"}) -> ("new picture"=w1583:picture)  [unwired: 5 in]
              }
            }
            n3297 = case shown="9" w346 {
              tunnel: 680 -> [w363 w437 w467 w535 w600 w652 w720 w797 w853 w942]
              tunnel: 10 -> [w362 w436 w466 w534 w599 w651 w719 w796 w852 w941]
              tunnel: 3 -> [w361 w435 w465 w533 w598 w650 w718 w795 w851 w940]
              tunnel: w354 -> [w364 w439 w469 w536 w601 w654 w722 w799 w855 w944]
              tunnel: [w355 w434 w461 w528 w594 w646 w713 w792 w845 w936] -> w340
              frame 0, Default {
                n3298 = Add(x=w363, y=0) -> (x+y=w419:i32)
                n3299 = Add(x=w362, y=0) -> (x+y=w420:i32)
                n3300 = Multiply(x=w361, y=10) -> (x*y=w418:i32)
                n3301 = Add(x=w363, y=0) -> (x+y=w385:i32)
                n3302 = Multiply(x=w361, y=10) -> (x*y=w388:i32)
                n3303 = Add(x=w362, y=w388) -> (x+y=w386:i32)
                n3304 = Add(x=w420, y=w418) -> (x+y=w421:i32)
                n3305 = Add(x=w386, y=w388) -> (x+y=w387:i32)
                n3306 = Bundle(w419, w420) -> (w416:cluster{i32, i32})  [unwired: 1 in]
                n3307 = Bundle(w385, w386) -> (w383:cluster{i32, i32})  [unwired: 1 in]
                n3308 = Bundle(w419, w421) -> (w417:cluster{i32, i32})  [unwired: 1 in]
                n3309 = Bundle(w385, w387) -> (w384:cluster{i32, i32})  [unwired: 1 in]
                n3310 = Multiply(x=w361, y=10) -> (x*y=w376:i32)
                n3311 = Multiply(x=2, y=w376) -> (x*y=w377:i32)
                n3312 = Add(x=w363, y=0) -> (x+y=w431:i32)
                n3313 = Add(x=w362, y=0) -> (x+y=w432:i32)
                n3314 = Add(x=w363, y=0) -> (x+y=w373:i32)
                n3315 = Add(x=w362, y=w377) -> (x+y=w375:i32)
                n3316 = Multiply(x=w361, y=10) -> (x*y=w429:i32)
                n3317 = Add(x=w373, y=w376) -> (x+y=w372:i32)
                n3318 = Add(x=w431, y=w429) -> (x+y=w430:i32)
                n3319 = Bundle(w431, w432) -> (w428:cluster{i32, i32})  [unwired: 1 in]
                n3320 = Bundle(w373, w375) -> (w371:cluster{i32, i32})  [unwired: 1 in]
                n3321 = call <vilib>:"Move Pen.vi"("new position"=w428, "picture"=w364) -> ("new picture"=w427:picture)  [unwired: 3 in]
                n3322 = Bundle(w430, w432) -> (w433:cluster{i32, i32})  [unwired: 1 in]
                n3323 = Bundle(w372, w375) -> (w374:cluster{i32, i32})  [unwired: 1 in]
                n3324 = Multiply(x=w361, y=10) -> (x*y=w406:i32)
                n3325 = Add(x=w363, y=w406) -> (x+y=w407:i32)
                n3326 = Add(x=w362, y=0) -> (x+y=w409:i32)
                n3327 = Multiply(x=w361, y=10) -> (x*y=w398:i32)
                n3328 = Add(x=w363, y=w398) -> (x+y=w395:i32)
                n3329 = Add(x=w362, y=w398) -> (x+y=w397:i32)
                n3330 = Add(x=w409, y=w406) -> (x+y=w408:i32)
                n3331 = Bundle(w407, w409) -> (w404:cluster{i32, i32})  [unwired: 1 in]
                n3332 = call <vilib>:"Draw Line.vi"("picture"=w427, "end point"=w433, "color(black)"=u32 16448250, "pen"=T1 {"Width"=3, "Style"=enum."Solid"}) -> ("new picture"=w360:picture)  [unwired: 5 in]
                n3333 = call <vilib>:"Move Pen.vi"("new position"=w416, "picture"=w360) -> ("new picture"=w415:picture)  [unwired: 3 in]
                n3334 = call <vilib>:"Draw Line.vi"("picture"=w415, "end point"=w417, "color(black)"=u32 16448250, "pen"=T1 {"Width"=3, "Style"=enum."Solid"}) -> ("new picture"=w359:picture)  [unwired: 5 in]
                n3335 = Add(x=w397, y=w398) -> (x+y=w396:i32)
                n3336 = Bundle(w395, w397) -> (w393:cluster{i32, i32})  [unwired: 1 in]
                n3337 = call <vilib>:"Move Pen.vi"("new position"=w404, "picture"=w359) -> ("new picture"=w403:picture)  [unwired: 3 in]
                n3338 = Bundle(w407, w408) -> (w405:cluster{i32, i32})  [unwired: 1 in]
                n3339 = Bundle(w395, w396) -> (w394:cluster{i32, i32})  [unwired: 1 in]
                n3340 = call <vilib>:"Draw Line.vi"("picture"=w403, "end point"=w405, "color(black)"=u32 16448250, "pen"=T1 {"Width"=3, "Style"=enum."Solid"}) -> ("new picture"=w358:picture)  [unwired: 5 in]
                n3341 = call <vilib>:"Move Pen.vi"("new position"=w383, "picture"=w358) -> ("new picture"=w382:picture)  [unwired: 3 in]
                n3342 = call <vilib>:"Draw Line.vi"("picture"=w382, "end point"=w384, "color(black)"=u32 16448250, "pen"=T1 {"Width"=3, "Style"=enum."Solid"}) -> ("new picture"=w357:picture)  [unwired: 5 in]
                n3343 = call <vilib>:"Move Pen.vi"("new position"=w393, "picture"=w357) -> ("new picture"=w392:picture)  [unwired: 3 in]
                n3344 = call <vilib>:"Draw Line.vi"("picture"=w392, "end point"=w394, "color(black)"=u32 16448250, "pen"=T1 {"Width"=3, "Style"=enum."Solid"}) -> ("new picture"=w356:picture)  [unwired: 5 in]
                n3345 = call <vilib>:"Move Pen.vi"("new position"=w371, "picture"=w356) -> ("new picture"=w370:picture)  [unwired: 3 in]
                n3346 = call <vilib>:"Draw Line.vi"("picture"=w370, "end point"=w374, "color(black)"=u32 16448250, "pen"=T1 {"Width"=3, "Style"=enum."Solid"}) -> ("new picture"=w355:picture)  [unwired: 5 in]
              }
              frame 1 {
                n3347 = Multiply(x=w435, y=10) -> (x*y=w457:i32)
                n3348 = Add(x=w437, y=w457) -> (x+y=w458:i32)
                n3349 = Add(x=w436, y=0) -> (x+y=w460:i32)
                n3350 = Add(x=w460, y=w457) -> (x+y=w459:i32)
                n3351 = Bundle(w458, w460) -> (w455:cluster{i32, i32})  [unwired: 1 in]
                n3352 = call <vilib>:"Move Pen.vi"("new position"=w455, "picture"=w439) -> ("new picture"=w454:picture)  [unwired: 3 in]
                n3353 = Bundle(w458, w459) -> (w456:cluster{i32, i32})  [unwired: 1 in]
                n3354 = call <vilib>:"Draw Line.vi"("picture"=w454, "end point"=w456, "color(black)"=u32 16448250, "pen"=T1 {"Width"=3, "Style"=enum."Solid"}) -> ("new picture"=w438:picture)  [unwired: 5 in]
                n3355 = Multiply(x=w435, y=10) -> (x*y=w449:i32)
                n3356 = Add(x=w437, y=w449) -> (x+y=w446:i32)
                n3357 = Add(x=w436, y=w449) -> (x+y=w448:i32)
                n3358 = Add(x=w448, y=w449) -> (x+y=w447:i32)
                n3359 = Bundle(w446, w448) -> (w444:cluster{i32, i32})  [unwired: 1 in]
                n3360 = call <vilib>:"Move Pen.vi"("new position"=w444, "picture"=w438) -> ("new picture"=w443:picture)  [unwired: 3 in]
                n3361 = Bundle(w446, w447) -> (w445:cluster{i32, i32})  [unwired: 1 in]
                n3362 = call <vilib>:"Draw Line.vi"("picture"=w443, "end point"=w445, "color(black)"=u32 16448250, "pen"=T1 {"Width"=3, "Style"=enum."Solid"}) -> ("new picture"=w434:picture)  [unwired: 5 in]
              }
              frame 2 {
                n3363 = Multiply(x=w465, y=10) -> (x*y=w503:i32)
                n3364 = Add(x=w467, y=0) -> (x+y=w501:i32)
                n3365 = Add(x=w466, y=w503) -> (x+y=w504:i32)
                n3366 = Add(x=w467, y=0) -> (x+y=w525:i32)
                n3367 = Add(x=w466, y=0) -> (x+y=w526:i32)
                n3368 = Multiply(x=w465, y=10) -> (x*y=w523:i32)
                n3369 = Add(x=w501, y=w503) -> (x+y=w500:i32)
                n3370 = Add(x=w525, y=w523) -> (x+y=w524:i32)
                n3371 = Bundle(w501, w504) -> (w499:cluster{i32, i32})  [unwired: 1 in]
                n3372 = Bundle(w525, w526) -> (w522:cluster{i32, i32})  [unwired: 1 in]
                n3373 = Bundle(w500, w504) -> (w502:cluster{i32, i32})  [unwired: 1 in]
                n3374 = call <vilib>:"Move Pen.vi"("new position"=w522, "picture"=w469) -> ("new picture"=w521:picture)  [unwired: 3 in]
                n3375 = Bundle(w524, w526) -> (w527:cluster{i32, i32})  [unwired: 1 in]
                n3376 = Multiply(x=w465, y=10) -> (x*y=w481:i32)
                n3377 = Multiply(x=2, y=w481) -> (x*y=w482:i32)
                n3378 = Add(x=w467, y=0) -> (x+y=w478:i32)
                n3379 = Add(x=w466, y=w482) -> (x+y=w480:i32)
                n3380 = Add(x=w478, y=w481) -> (x+y=w477:i32)
                n3381 = Bundle(w478, w480) -> (w476:cluster{i32, i32})  [unwired: 1 in]
                n3382 = call <vilib>:"Draw Line.vi"("picture"=w521, "end point"=w527, "color(black)"=u32 16448250, "pen"=T1 {"Width"=3, "Style"=enum."Solid"}) -> ("new picture"=w468:picture)  [unwired: 5 in]
                n3383 = Bundle(w477, w480) -> (w479:cluster{i32, i32})  [unwired: 1 in]
                n3384 = Multiply(x=w465, y=10) -> (x*y=w512:i32)
                n3385 = Add(x=w467, y=0) -> (x+y=w490:i32)
                n3386 = Add(x=w467, y=w512) -> (x+y=w513:i32)
                n3387 = Add(x=w466, y=0) -> (x+y=w515:i32)
                n3388 = Multiply(x=w465, y=10) -> (x*y=w493:i32)
                n3389 = Add(x=w466, y=w493) -> (x+y=w491:i32)
                n3390 = Add(x=w491, y=w493) -> (x+y=w492:i32)
                n3391 = Add(x=w515, y=w512) -> (x+y=w514:i32)
                n3392 = Bundle(w490, w491) -> (w488:cluster{i32, i32})  [unwired: 1 in]
                n3393 = Bundle(w513, w515) -> (w510:cluster{i32, i32})  [unwired: 1 in]
                n3394 = call <vilib>:"Move Pen.vi"("new position"=w510, "picture"=w468) -> ("new picture"=w509:picture)  [unwired: 3 in]
                n3395 = Bundle(w490, w492) -> (w489:cluster{i32, i32})  [unwired: 1 in]
                n3396 = Bundle(w513, w514) -> (w511:cluster{i32, i32})  [unwired: 1 in]
                n3397 = call <vilib>:"Draw Line.vi"("picture"=w509, "end point"=w511, "color(black)"=u32 16448250, "pen"=T1 {"Width"=3, "Style"=enum."Solid"}) -> ("new picture"=w464:picture)  [unwired: 5 in]
                n3398 = call <vilib>:"Move Pen.vi"("new position"=w499, "picture"=w464) -> ("new picture"=w498:picture)  [unwired: 3 in]
                n3399 = call <vilib>:"Draw Line.vi"("picture"=w498, "end point"=w502, "color(black)"=u32 16448250, "pen"=T1 {"Width"=3, "Style"=enum."Solid"}) -> ("new picture"=w463:picture)  [unwired: 5 in]
                n3400 = call <vilib>:"Move Pen.vi"("new position"=w488, "picture"=w463) -> ("new picture"=w487:picture)  [unwired: 3 in]
                n3401 = call <vilib>:"Draw Line.vi"("picture"=w487, "end point"=w489, "color(black)"=u32 16448250, "pen"=T1 {"Width"=3, "Style"=enum."Solid"}) -> ("new picture"=w462:picture)  [unwired: 5 in]
                n3402 = call <vilib>:"Move Pen.vi"("new position"=w476, "picture"=w462) -> ("new picture"=w475:picture)  [unwired: 3 in]
                n3403 = call <vilib>:"Draw Line.vi"("picture"=w475, "end point"=w479, "color(black)"=u32 16448250, "pen"=T1 {"Width"=3, "Style"=enum."Solid"}) -> ("new picture"=w461:picture)  [unwired: 5 in]
              }
              frame 3 {
                n3404 = Multiply(x=w533, y=10) -> (x*y=w569:i32)
                n3405 = Add(x=w535, y=0) -> (x+y=w567:i32)
                n3406 = Add(x=w534, y=w569) -> (x+y=w570:i32)
                n3407 = Add(x=w535, y=0) -> (x+y=w591:i32)
                n3408 = Add(x=w534, y=0) -> (x+y=w592:i32)
                n3409 = Multiply(x=w533, y=10) -> (x*y=w589:i32)
                n3410 = Add(x=w567, y=w569) -> (x+y=w566:i32)
                n3411 = Add(x=w591, y=w589) -> (x+y=w590:i32)
                n3412 = Bundle(w567, w570) -> (w565:cluster{i32, i32})  [unwired: 1 in]
                n3413 = Bundle(w591, w592) -> (w588:cluster{i32, i32})  [unwired: 1 in]
                n3414 = call <vilib>:"Move Pen.vi"("new position"=w588, "picture"=w536) -> ("new picture"=w587:picture)  [unwired: 3 in]
                n3415 = Bundle(w566, w570) -> (w568:cluster{i32, i32})  [unwired: 1 in]
                n3416 = Bundle(w590, w592) -> (w593:cluster{i32, i32})  [unwired: 1 in]
                n3417 = Multiply(x=w533, y=10) -> (x*y=w548:i32)
                n3418 = Multiply(x=2, y=w548) -> (x*y=w549:i32)
                n3419 = Add(x=w535, y=0) -> (x+y=w545:i32)
                n3420 = Add(x=w534, y=w549) -> (x+y=w547:i32)
                n3421 = Add(x=w545, y=w548) -> (x+y=w544:i32)
                n3422 = call <vilib>:"Draw Line.vi"("picture"=w587, "end point"=w593, "color(black)"=u32 16448250, "pen"=T1 {"Width"=3, "Style"=enum."Solid"}) -> ("new picture"=w532:picture)  [unwired: 5 in]
                n3423 = Bundle(w545, w547) -> (w543:cluster{i32, i32})  [unwired: 1 in]
                n3424 = Bundle(w544, w547) -> (w546:cluster{i32, i32})  [unwired: 1 in]
                n3425 = Multiply(x=w533, y=10) -> (x*y=w559:i32)
                n3426 = Add(x=w535, y=w559) -> (x+y=w556:i32)
                n3427 = Add(x=w534, y=w559) -> (x+y=w558:i32)
                n3428 = Multiply(x=w533, y=10) -> (x*y=w578:i32)
                n3429 = Add(x=w535, y=w578) -> (x+y=w579:i32)
                n3430 = Add(x=w534, y=0) -> (x+y=w581:i32)
                n3431 = Add(x=w558, y=w559) -> (x+y=w557:i32)
                n3432 = Bundle(w556, w558) -> (w554:cluster{i32, i32})  [unwired: 1 in]
                n3433 = Add(x=w581, y=w578) -> (x+y=w580:i32)
                n3434 = Bundle(w579, w581) -> (w576:cluster{i32, i32})  [unwired: 1 in]
                n3435 = Bundle(w556, w557) -> (w555:cluster{i32, i32})  [unwired: 1 in]
                n3436 = call <vilib>:"Move Pen.vi"("new position"=w576, "picture"=w532) -> ("new picture"=w575:picture)  [unwired: 3 in]
                n3437 = Bundle(w579, w580) -> (w577:cluster{i32, i32})  [unwired: 1 in]
                n3438 = call <vilib>:"Draw Line.vi"("picture"=w575, "end point"=w577, "color(black)"=u32 16448250, "pen"=T1 {"Width"=3, "Style"=enum."Solid"}) -> ("new picture"=w531:picture)  [unwired: 5 in]
                n3439 = call <vilib>:"Move Pen.vi"("new position"=w565, "picture"=w531) -> ("new picture"=w564:picture)  [unwired: 3 in]
                n3440 = call <vilib>:"Draw Line.vi"("picture"=w564, "end point"=w568, "color(black)"=u32 16448250, "pen"=T1 {"Width"=3, "Style"=enum."Solid"}) -> ("new picture"=w530:picture)  [unwired: 5 in]
                n3441 = call <vilib>:"Move Pen.vi"("new position"=w554, "picture"=w530) -> ("new picture"=w553:picture)  [unwired: 3 in]
                n3442 = call <vilib>:"Draw Line.vi"("picture"=w553, "end point"=w555, "color(black)"=u32 16448250, "pen"=T1 {"Width"=3, "Style"=enum."Solid"}) -> ("new picture"=w529:picture)  [unwired: 5 in]
                n3443 = call <vilib>:"Move Pen.vi"("new position"=w543, "picture"=w529) -> ("new picture"=w542:picture)  [unwired: 3 in]
                n3444 = call <vilib>:"Draw Line.vi"("picture"=w542, "end point"=w546, "color(black)"=u32 16448250, "pen"=T1 {"Width"=3, "Style"=enum."Solid"}) -> ("new picture"=w528:picture)  [unwired: 5 in]
              }
              frame 4 {
                n3445 = Add(x=w600, y=0) -> (x+y=w643:i32)
                n3446 = Add(x=w599, y=0) -> (x+y=w644:i32)
                n3447 = Multiply(x=w598, y=10) -> (x*y=w642:i32)
                n3448 = Add(x=w644, y=w642) -> (x+y=w645:i32)
                n3449 = Bundle(w643, w644) -> (w640:cluster{i32, i32})  [unwired: 1 in]
                n3450 = call <vilib>:"Move Pen.vi"("new position"=w640, "picture"=w601) -> ("new picture"=w639:picture)  [unwired: 3 in]
                n3451 = Bundle(w643, w645) -> (w641:cluster{i32, i32})  [unwired: 1 in]
                n3452 = Multiply(x=w598, y=10) -> (x*y=w621:i32)
                n3453 = Add(x=w600, y=0) -> (x+y=w619:i32)
                n3454 = Add(x=w599, y=w621) -> (x+y=w622:i32)
                n3455 = Add(x=w619, y=w621) -> (x+y=w618:i32)
                n3456 = Bundle(w619, w622) -> (w617:cluster{i32, i32})  [unwired: 1 in]
                n3457 = call <vilib>:"Draw Line.vi"("picture"=w639, "end point"=w641, "color(black)"=u32 16448250, "pen"=T1 {"Width"=3, "Style"=enum."Solid"}) -> ("new picture"=w595:picture)  [unwired: 5 in]
                n3458 = Multiply(x=w598, y=10) -> (x*y=w611:i32)
                n3459 = Add(x=w600, y=w611) -> (x+y=w608:i32)
                n3460 = Add(x=w599, y=w611) -> (x+y=w610:i32)
                n3461 = Bundle(w618, w622) -> (w620:cluster{i32, i32})  [unwired: 1 in]
                n3462 = Add(x=w610, y=w611) -> (x+y=w609:i32)
                n3463 = Bundle(w608, w610) -> (w606:cluster{i32, i32})  [unwired: 1 in]
                n3464 = Multiply(x=w598, y=10) -> (x*y=w630:i32)
                n3465 = Add(x=w600, y=w630) -> (x+y=w631:i32)
                n3466 = Add(x=w599, y=0) -> (x+y=w633:i32)
                n3467 = Add(x=w633, y=w630) -> (x+y=w632:i32)
                n3468 = Bundle(w608, w609) -> (w607:cluster{i32, i32})  [unwired: 1 in]
                n3469 = Bundle(w631, w633) -> (w628:cluster{i32, i32})  [unwired: 1 in]
                n3470 = call <vilib>:"Move Pen.vi"("new position"=w628, "picture"=w595) -> ("new picture"=w627:picture)  [unwired: 3 in]
                n3471 = Bundle(w631, w632) -> (w629:cluster{i32, i32})  [unwired: 1 in]
                n3472 = call <vilib>:"Draw Line.vi"("picture"=w627, "end point"=w629, "color(black)"=u32 16448250, "pen"=T1 {"Width"=3, "Style"=enum."Solid"}) -> ("new picture"=w597:picture)  [unwired: 5 in]
                n3473 = call <vilib>:"Move Pen.vi"("new position"=w617, "picture"=w597) -> ("new picture"=w616:picture)  [unwired: 3 in]
                n3474 = call <vilib>:"Draw Line.vi"("picture"=w616, "end point"=w620, "color(black)"=u32 16448250, "pen"=T1 {"Width"=3, "Style"=enum."Solid"}) -> ("new picture"=w596:picture)  [unwired: 5 in]
                n3475 = call <vilib>:"Move Pen.vi"("new position"=w606, "picture"=w596) -> ("new picture"=w605:picture)  [unwired: 3 in]
                n3476 = call <vilib>:"Draw Line.vi"("picture"=w605, "end point"=w607, "color(black)"=u32 16448250, "pen"=T1 {"Width"=3, "Style"=enum."Solid"}) -> ("new picture"=w594:picture)  [unwired: 5 in]
              }
              frame 5 {
                n3477 = Multiply(x=w650, y=10) -> (x*y=w687:i32)
                n3478 = Add(x=w652, y=0) -> (x+y=w685:i32)
                n3479 = Add(x=w651, y=w687) -> (x+y=w688:i32)
                n3480 = Add(x=w652, y=0) -> (x+y=w710:i32)
                n3481 = Add(x=w651, y=0) -> (x+y=w711:i32)
                n3482 = Add(x=w685, y=w687) -> (x+y=w684:i32)
                n3483 = Multiply(x=w650, y=10) -> (x*y=w708:i32)
                n3484 = Bundle(w685, w688) -> (w683:cluster{i32, i32})  [unwired: 1 in]
                n3485 = Add(x=w710, y=w708) -> (x+y=w709:i32)
                n3486 = Bundle(w710, w711) -> (w707:cluster{i32, i32})  [unwired: 1 in]
                n3487 = Bundle(w684, w688) -> (w686:cluster{i32, i32})  [unwired: 1 in]
                n3488 = call <vilib>:"Move Pen.vi"("new position"=w707, "picture"=w654) -> ("new picture"=w706:picture)  [unwired: 3 in]
                n3489 = Bundle(w709, w711) -> (w712:cluster{i32, i32})  [unwired: 1 in]
                n3490 = Multiply(x=w650, y=10) -> (x*y=w666:i32)
                n3491 = Multiply(x=2, y=w666) -> (x*y=w667:i32)
                n3492 = Add(x=w652, y=0) -> (x+y=w663:i32)
                n3493 = Add(x=w651, y=w667) -> (x+y=w665:i32)
                n3494 = Add(x=w663, y=w666) -> (x+y=w662:i32)
                n3495 = Bundle(w663, w665) -> (w661:cluster{i32, i32})  [unwired: 1 in]
                n3496 = call <vilib>:"Draw Line.vi"("picture"=w706, "end point"=w712, "color(black)"=u32 16448250, "pen"=T1 {"Width"=3, "Style"=enum."Solid"}) -> ("new picture"=w653:picture)  [unwired: 5 in]
                n3497 = Bundle(w662, w665) -> (w664:cluster{i32, i32})  [unwired: 1 in]
                n3498 = Multiply(x=w650, y=10) -> (x*y=w677:i32)
                n3499 = Add(x=w652, y=0) -> (x+y=w698:i32)
                n3500 = Add(x=w651, y=0) -> (x+y=w699:i32)
                n3501 = Add(x=w652, y=w677) -> (x+y=w674:i32)
                n3502 = Add(x=w651, y=w677) -> (x+y=w676:i32)
                n3503 = Multiply(x=w650, y=10) -> (x*y=w697:i32)
                n3504 = Add(x=w699, y=w697) -> (x+y=w700:i32)
                n3505 = Add(x=w676, y=w677) -> (x+y=w675:i32)
                n3506 = Bundle(w698, w699) -> (w695:cluster{i32, i32})  [unwired: 1 in]
                n3507 = Bundle(w674, w676) -> (w672:cluster{i32, i32})  [unwired: 1 in]
                n3508 = call <vilib>:"Move Pen.vi"("new position"=w695, "picture"=w653) -> ("new picture"=w694:picture)  [unwired: 3 in]
                n3509 = Bundle(w698, w700) -> (w696:cluster{i32, i32})  [unwired: 1 in]
                n3510 = Bundle(w674, w675) -> (w673:cluster{i32, i32})  [unwired: 1 in]
                n3511 = call <vilib>:"Draw Line.vi"("picture"=w694, "end point"=w696, "color(black)"=u32 16448250, "pen"=T1 {"Width"=3, "Style"=enum."Solid"}) -> ("new picture"=w649:picture)  [unwired: 5 in]
                n3512 = call <vilib>:"Move Pen.vi"("new position"=w683, "picture"=w649) -> ("new picture"=w682:picture)  [unwired: 3 in]
                n3513 = call <vilib>:"Draw Line.vi"("picture"=w682, "end point"=w686, "color(black)"=u32 16448250, "pen"=T1 {"Width"=3, "Style"=enum."Solid"}) -> ("new picture"=w648:picture)  [unwired: 5 in]
                n3514 = call <vilib>:"Move Pen.vi"("new position"=w672, "picture"=w648) -> ("new picture"=w671:picture)  [unwired: 3 in]
                n3515 = call <vilib>:"Draw Line.vi"("picture"=w671, "end point"=w673, "color(black)"=u32 16448250, "pen"=T1 {"Width"=3, "Style"=enum."Solid"}) -> ("new picture"=w647:picture)  [unwired: 5 in]
                n3516 = call <vilib>:"Move Pen.vi"("new position"=w661, "picture"=w647) -> ("new picture"=w660:picture)  [unwired: 3 in]
                n3517 = call <vilib>:"Draw Line.vi"("picture"=w660, "end point"=w664, "color(black)"=u32 16448250, "pen"=T1 {"Width"=3, "Style"=enum."Solid"}) -> ("new picture"=w646:picture)  [unwired: 5 in]
              }
              frame 6 {
                n3518 = Multiply(x=w718, y=10) -> (x*y=w756:i32)
                n3519 = Multiply(x=w718, y=10) -> (x*y=w766:i32)
                n3520 = Add(x=w720, y=w756) -> (x+y=w753:i32)
                n3521 = Add(x=w719, y=w756) -> (x+y=w755:i32)
                n3522 = Add(x=w720, y=0) -> (x+y=w764:i32)
                n3523 = Add(x=w719, y=w766) -> (x+y=w767:i32)
                n3524 = Add(x=w720, y=0) -> (x+y=w789:i32)
                n3525 = Add(x=w719, y=0) -> (x+y=w790:i32)
                n3526 = Multiply(x=w718, y=10) -> (x*y=w787:i32)
                n3527 = Add(x=w764, y=w766) -> (x+y=w763:i32)
                n3528 = Add(x=w755, y=w756) -> (x+y=w754:i32)
                n3529 = Bundle(w753, w755) -> (w751:cluster{i32, i32})  [unwired: 1 in]
                n3530 = Bundle(w764, w767) -> (w762:cluster{i32, i32})  [unwired: 1 in]
                n3531 = Add(x=w789, y=w787) -> (x+y=w788:i32)
                n3532 = Bundle(w789, w790) -> (w786:cluster{i32, i32})  [unwired: 1 in]
                n3533 = Bundle(w753, w754) -> (w752:cluster{i32, i32})  [unwired: 1 in]
                n3534 = Bundle(w763, w767) -> (w765:cluster{i32, i32})  [unwired: 1 in]
                n3535 = call <vilib>:"Move Pen.vi"("new position"=w786, "picture"=w722) -> ("new picture"=w785:picture)  [unwired: 3 in]
                n3536 = Bundle(w788, w790) -> (w791:cluster{i32, i32})  [unwired: 1 in]
                n3537 = call <vilib>:"Draw Line.vi"("picture"=w785, "end point"=w791, "color(black)"=u32 16448250, "pen"=T1 {"Width"=3, "Style"=enum."Solid"}) -> ("new picture"=w721:picture)  [unwired: 5 in]
                n3538 = Multiply(x=w718, y=10) -> (x*y=w734:i32)
                n3539 = Multiply(x=2, y=w734) -> (x*y=w735:i32)
                n3540 = Add(x=w720, y=0) -> (x+y=w743:i32)
                n3541 = Multiply(x=w718, y=10) -> (x*y=w746:i32)
                n3542 = Add(x=w719, y=w746) -> (x+y=w744:i32)
                n3543 = Add(x=w720, y=0) -> (x+y=w731:i32)
                n3544 = Add(x=w719, y=w735) -> (x+y=w733:i32)
                n3545 = Add(x=w720, y=0) -> (x+y=w777:i32)
                n3546 = Add(x=w719, y=0) -> (x+y=w778:i32)
                n3547 = Multiply(x=w718, y=10) -> (x*y=w776:i32)
                n3548 = Add(x=w744, y=w746) -> (x+y=w745:i32)
                n3549 = Add(x=w731, y=w734) -> (x+y=w730:i32)
                n3550 = Add(x=w778, y=w776) -> (x+y=w779:i32)
                n3551 = Bundle(w743, w744) -> (w741:cluster{i32, i32})  [unwired: 1 in]
                n3552 = Bundle(w731, w733) -> (w729:cluster{i32, i32})  [unwired: 1 in]
                n3553 = Bundle(w777, w778) -> (w774:cluster{i32, i32})  [unwired: 1 in]
                n3554 = Bundle(w743, w745) -> (w742:cluster{i32, i32})  [unwired: 1 in]
                n3555 = Bundle(w730, w733) -> (w732:cluster{i32, i32})  [unwired: 1 in]
                n3556 = call <vilib>:"Move Pen.vi"("new position"=w774, "picture"=w721) -> ("new picture"=w773:picture)  [unwired: 3 in]
                n3557 = Bundle(w777, w779) -> (w775:cluster{i32, i32})  [unwired: 1 in]
                n3558 = call <vilib>:"Draw Line.vi"("picture"=w773, "end point"=w775, "color(black)"=u32 16448250, "pen"=T1 {"Width"=3, "Style"=enum."Solid"}) -> ("new picture"=w717:picture)  [unwired: 5 in]
                n3559 = call <vilib>:"Move Pen.vi"("new position"=w762, "picture"=w717) -> ("new picture"=w761:picture)  [unwired: 3 in]
                n3560 = call <vilib>:"Draw Line.vi"("picture"=w761, "end point"=w765, "color(black)"=u32 16448250, "pen"=T1 {"Width"=3, "Style"=enum."Solid"}) -> ("new picture"=w716:picture)  [unwired: 5 in]
                n3561 = call <vilib>:"Move Pen.vi"("new position"=w741, "picture"=w716) -> ("new picture"=w740:picture)  [unwired: 3 in]
                n3562 = call <vilib>:"Draw Line.vi"("picture"=w740, "end point"=w742, "color(black)"=u32 16448250, "pen"=T1 {"Width"=3, "Style"=enum."Solid"}) -> ("new picture"=w715:picture)  [unwired: 5 in]
                n3563 = call <vilib>:"Move Pen.vi"("new position"=w751, "picture"=w715) -> ("new picture"=w750:picture)  [unwired: 3 in]
                n3564 = call <vilib>:"Draw Line.vi"("picture"=w750, "end point"=w752, "color(black)"=u32 16448250, "pen"=T1 {"Width"=3, "Style"=enum."Solid"}) -> ("new picture"=w714:picture)  [unwired: 5 in]
                n3565 = call <vilib>:"Move Pen.vi"("new position"=w729, "picture"=w714) -> ("new picture"=w728:picture)  [unwired: 3 in]
                n3566 = call <vilib>:"Draw Line.vi"("picture"=w728, "end point"=w732, "color(black)"=u32 16448250, "pen"=T1 {"Width"=3, "Style"=enum."Solid"}) -> ("new picture"=w713:picture)  [unwired: 5 in]
              }
              frame 7 {
                n3567 = Add(x=w797, y=0) -> (x+y=w830:i32)
                n3568 = Add(x=w796, y=0) -> (x+y=w831:i32)
                n3569 = Multiply(x=w795, y=10) -> (x*y=w829:i32)
                n3570 = Add(x=w831, y=w829) -> (x+y=w832:i32)
                n3571 = Add(x=w797, y=0) -> (x+y=w842:i32)
                n3572 = Add(x=w796, y=0) -> (x+y=w843:i32)
                n3573 = Bundle(w830, w831) -> (w827:cluster{i32, i32})  [unwired: 1 in]
                n3574 = Multiply(x=w795, y=10) -> (x*y=w840:i32)
                n3575 = Add(x=w842, y=w840) -> (x+y=w841:i32)
                n3576 = Bundle(w842, w843) -> (w839:cluster{i32, i32})  [unwired: 1 in]
                n3577 = Bundle(w830, w832) -> (w828:cluster{i32, i32})  [unwired: 1 in]
                n3578 = call <vilib>:"Move Pen.vi"("new position"=w839, "picture"=w799) -> ("new picture"=w838:picture)  [unwired: 3 in]
                n3579 = Bundle(w841, w843) -> (w844:cluster{i32, i32})  [unwired: 1 in]
                n3580 = call <vilib>:"Draw Line.vi"("picture"=w838, "end point"=w844, "color(black)"=u32 16448250, "pen"=T1 {"Width"=3, "Style"=enum."Solid"}) -> ("new picture"=w798:picture)  [unwired: 5 in]
                n3581 = Multiply(x=w795, y=10) -> (x*y=w817:i32)
                n3582 = Add(x=w797, y=w817) -> (x+y=w818:i32)
                n3583 = Add(x=w796, y=0) -> (x+y=w820:i32)
                n3584 = Multiply(x=w795, y=10) -> (x*y=w809:i32)
                n3585 = Add(x=w797, y=w809) -> (x+y=w806:i32)
                n3586 = Add(x=w796, y=w809) -> (x+y=w808:i32)
                n3587 = Add(x=w820, y=w817) -> (x+y=w819:i32)
                n3588 = Bundle(w818, w820) -> (w815:cluster{i32, i32})  [unwired: 1 in]
                n3589 = Add(x=w808, y=w809) -> (x+y=w807:i32)
                n3590 = Bundle(w806, w808) -> (w804:cluster{i32, i32})  [unwired: 1 in]
                n3591 = Bundle(w818, w819) -> (w816:cluster{i32, i32})  [unwired: 1 in]
                n3592 = call <vilib>:"Move Pen.vi"("new position"=w804, "picture"=w798) -> ("new picture"=w803:picture)  [unwired: 3 in]
                n3593 = Bundle(w806, w807) -> (w805:cluster{i32, i32})  [unwired: 1 in]
                n3594 = call <vilib>:"Draw Line.vi"("picture"=w803, "end point"=w805, "color(black)"=u32 16448250, "pen"=T1 {"Width"=3, "Style"=enum."Solid"}) -> ("new picture"=w794:picture)  [unwired: 5 in]
                n3595 = call <vilib>:"Move Pen.vi"("new position"=w827, "picture"=w794) -> ("new picture"=w826:picture)  [unwired: 3 in]
                n3596 = call <vilib>:"Draw Line.vi"("picture"=w826, "end point"=w828, "color(black)"=u32 16448250, "pen"=T1 {"Width"=3, "Style"=enum."Solid"}) -> ("new picture"=w793:picture)  [unwired: 5 in]
                n3597 = call <vilib>:"Move Pen.vi"("new position"=w815, "picture"=w793) -> ("new picture"=w814:picture)  [unwired: 3 in]
                n3598 = call <vilib>:"Draw Line.vi"("picture"=w814, "end point"=w816, "color(black)"=u32 16448250, "pen"=T1 {"Width"=3, "Style"=enum."Solid"}) -> ("new picture"=w792:picture)  [unwired: 5 in]
              }
              frame 8 {
                n3599 = Add(x=w853, y=0) -> (x+y=w921:i32)
                n3600 = Add(x=w852, y=0) -> (x+y=w922:i32)
                n3601 = Add(x=w853, y=0) -> (x+y=w876:i32)
                n3602 = Multiply(x=w851, y=10) -> (x*y=w920:i32)
                n3603 = Multiply(x=w851, y=10) -> (x*y=w879:i32)
                n3604 = Add(x=w852, y=w879) -> (x+y=w877:i32)
                n3605 = Add(x=w853, y=0) -> (x+y=w933:i32)
                n3606 = Add(x=w852, y=0) -> (x+y=w934:i32)
                n3607 = Multiply(x=w851, y=10) -> (x*y=w931:i32)
                n3608 = Add(x=w922, y=w920) -> (x+y=w923:i32)
                n3609 = Add(x=w877, y=w879) -> (x+y=w878:i32)
                n3610 = Bundle(w921, w922) -> (w918:cluster{i32, i32})  [unwired: 1 in]
                n3611 = Bundle(w876, w877) -> (w874:cluster{i32, i32})  [unwired: 1 in]
                n3612 = Multiply(x=w851, y=10) -> (x*y=w867:i32)
                n3613 = Multiply(x=2, y=w867) -> (x*y=w868:i32)
                n3614 = Add(x=w933, y=w931) -> (x+y=w932:i32)
                n3615 = Bundle(w933, w934) -> (w930:cluster{i32, i32})  [unwired: 1 in]
                n3616 = Add(x=w853, y=0) -> (x+y=w864:i32)
                n3617 = Add(x=w852, y=w868) -> (x+y=w866:i32)
                n3618 = Add(x=w864, y=w867) -> (x+y=w863:i32)
                n3619 = Bundle(w921, w923) -> (w919:cluster{i32, i32})  [unwired: 1 in]
                n3620 = Bundle(w876, w878) -> (w875:cluster{i32, i32})  [unwired: 1 in]
                n3621 = Bundle(w864, w866) -> (w862:cluster{i32, i32})  [unwired: 1 in]
                n3622 = call <vilib>:"Move Pen.vi"("new position"=w930, "picture"=w855) -> ("new picture"=w929:picture)  [unwired: 3 in]
                n3623 = Bundle(w932, w934) -> (w935:cluster{i32, i32})  [unwired: 1 in]
                n3624 = Bundle(w863, w866) -> (w865:cluster{i32, i32})  [unwired: 1 in]
                n3625 = call <vilib>:"Draw Line.vi"("picture"=w929, "end point"=w935, "color(black)"=u32 16448250, "pen"=T1 {"Width"=3, "Style"=enum."Solid"}) -> ("new picture"=w854:picture)  [unwired: 5 in]
                n3626 = Multiply(x=w851, y=10) -> (x*y=w899:i32)
                n3627 = Multiply(x=w851, y=10) -> (x*y=w908:i32)
                n3628 = Add(x=w853, y=0) -> (x+y=w897:i32)
                n3629 = Multiply(x=w851, y=10) -> (x*y=w889:i32)
                n3630 = Add(x=w852, y=w899) -> (x+y=w900:i32)
                n3631 = Add(x=w853, y=w908) -> (x+y=w909:i32)
                n3632 = Add(x=w852, y=0) -> (x+y=w911:i32)
                n3633 = Add(x=w853, y=w889) -> (x+y=w886:i32)
                n3634 = Add(x=w852, y=w889) -> (x+y=w888:i32)
                n3635 = Add(x=w897, y=w899) -> (x+y=w896:i32)
                n3636 = Bundle(w897, w900) -> (w895:cluster{i32, i32})  [unwired: 1 in]
                n3637 = Add(x=w911, y=w908) -> (x+y=w910:i32)
                n3638 = Add(x=w888, y=w889) -> (x+y=w887:i32)
                n3639 = Bundle(w909, w911) -> (w906:cluster{i32, i32})  [unwired: 1 in]
                n3640 = Bundle(w886, w888) -> (w884:cluster{i32, i32})  [unwired: 1 in]
                n3641 = call <vilib>:"Move Pen.vi"("new position"=w895, "picture"=w854) -> ("new picture"=w894:picture)  [unwired: 3 in]
                n3642 = Bundle(w896, w900) -> (w898:cluster{i32, i32})  [unwired: 1 in]
                n3643 = Bundle(w909, w910) -> (w907:cluster{i32, i32})  [unwired: 1 in]
                n3644 = Bundle(w886, w887) -> (w885:cluster{i32, i32})  [unwired: 1 in]
                n3645 = call <vilib>:"Draw Line.vi"("picture"=w894, "end point"=w898, "color(black)"=u32 16448250, "pen"=T1 {"Width"=3, "Style"=enum."Solid"}) -> ("new picture"=w850:picture)  [unwired: 5 in]
                n3646 = call <vilib>:"Move Pen.vi"("new position"=w918, "picture"=w850) -> ("new picture"=w917:picture)  [unwired: 3 in]
                n3647 = call <vilib>:"Draw Line.vi"("picture"=w917, "end point"=w919, "color(black)"=u32 16448250, "pen"=T1 {"Width"=3, "Style"=enum."Solid"}) -> ("new picture"=w849:picture)  [unwired: 5 in]
                n3648 = call <vilib>:"Move Pen.vi"("new position"=w906, "picture"=w849) -> ("new picture"=w905:picture)  [unwired: 3 in]
                n3649 = call <vilib>:"Draw Line.vi"("picture"=w905, "end point"=w907, "color(black)"=u32 16448250, "pen"=T1 {"Width"=3, "Style"=enum."Solid"}) -> ("new picture"=w848:picture)  [unwired: 5 in]
                n3650 = call <vilib>:"Move Pen.vi"("new position"=w874, "picture"=w848) -> ("new picture"=w873:picture)  [unwired: 3 in]
                n3651 = call <vilib>:"Draw Line.vi"("picture"=w873, "end point"=w875, "color(black)"=u32 16448250, "pen"=T1 {"Width"=3, "Style"=enum."Solid"}) -> ("new picture"=w847:picture)  [unwired: 5 in]
                n3652 = call <vilib>:"Move Pen.vi"("new position"=w884, "picture"=w847) -> ("new picture"=w883:picture)  [unwired: 3 in]
                n3653 = call <vilib>:"Draw Line.vi"("picture"=w883, "end point"=w885, "color(black)"=u32 16448250, "pen"=T1 {"Width"=3, "Style"=enum."Solid"}) -> ("new picture"=w846:picture)  [unwired: 5 in]
                n3654 = call <vilib>:"Move Pen.vi"("new position"=w862, "picture"=w846) -> ("new picture"=w861:picture)  [unwired: 3 in]
                n3655 = call <vilib>:"Draw Line.vi"("picture"=w861, "end point"=w865, "color(black)"=u32 16448250, "pen"=T1 {"Width"=3, "Style"=enum."Solid"}) -> ("new picture"=w845:picture)  [unwired: 5 in]
              }
              frame 9 {
                n3656 = Add(x=w942, y=0) -> (x+y=w986:i32)
                n3657 = Add(x=w941, y=0) -> (x+y=w987:i32)
                n3658 = Add(x=w942, y=0) -> (x+y=w998:i32)
                n3659 = Add(x=w941, y=0) -> (x+y=w999:i32)
                n3660 = Multiply(x=w940, y=10) -> (x*y=w985:i32)
                n3661 = Multiply(x=w940, y=10) -> (x*y=w996:i32)
                n3662 = Add(x=w987, y=w985) -> (x+y=w988:i32)
                n3663 = Add(x=w998, y=w996) -> (x+y=w997:i32)
                n3664 = Bundle(w986, w987) -> (w983:cluster{i32, i32})  [unwired: 1 in]
                n3665 = Bundle(w998, w999) -> (w995:cluster{i32, i32})  [unwired: 1 in]
                n3666 = Bundle(w986, w988) -> (w984:cluster{i32, i32})  [unwired: 1 in]
                n3667 = call <vilib>:"Move Pen.vi"("new position"=w995, "picture"=w944) -> ("new picture"=w994:picture)  [unwired: 3 in]
                n3668 = Bundle(w997, w999) -> (w1000:cluster{i32, i32})  [unwired: 1 in]
                n3669 = Multiply(x=w940, y=10) -> (x*y=w954:i32)
                n3670 = Add(x=w942, y=w954) -> (x+y=w951:i32)
                n3671 = Add(x=w941, y=w954) -> (x+y=w953:i32)
                n3672 = Add(x=w953, y=w954) -> (x+y=w952:i32)
                n3673 = Bundle(w951, w953) -> (w949:cluster{i32, i32})  [unwired: 1 in]
                n3674 = call <vilib>:"Draw Line.vi"("picture"=w994, "end point"=w1000, "color(black)"=u32 16448250, "pen"=T1 {"Width"=3, "Style"=enum."Solid"}) -> ("new picture"=w943:picture)  [unwired: 5 in]
                n3675 = Bundle(w951, w952) -> (w950:cluster{i32, i32})  [unwired: 1 in]
                n3676 = Multiply(x=w940, y=10) -> (x*y=w973:i32)
                n3677 = Add(x=w942, y=w973) -> (x+y=w974:i32)
                n3678 = Add(x=w941, y=0) -> (x+y=w976:i32)
                n3679 = Multiply(x=w940, y=10) -> (x*y=w964:i32)
                n3680 = Add(x=w942, y=0) -> (x+y=w962:i32)
                n3681 = Add(x=w941, y=w964) -> (x+y=w965:i32)
                n3682 = Add(x=w976, y=w973) -> (x+y=w975:i32)
                n3683 = Add(x=w962, y=w964) -> (x+y=w961:i32)
                n3684 = Bundle(w974, w976) -> (w971:cluster{i32, i32})  [unwired: 1 in]
                n3685 = Bundle(w962, w965) -> (w960:cluster{i32, i32})  [unwired: 1 in]
                n3686 = Bundle(w974, w975) -> (w972:cluster{i32, i32})  [unwired: 1 in]
                n3687 = call <vilib>:"Move Pen.vi"("new position"=w960, "picture"=w943) -> ("new picture"=w959:picture)  [unwired: 3 in]
                n3688 = Bundle(w961, w965) -> (w963:cluster{i32, i32})  [unwired: 1 in]
                n3689 = call <vilib>:"Draw Line.vi"("picture"=w959, "end point"=w963, "color(black)"=u32 16448250, "pen"=T1 {"Width"=3, "Style"=enum."Solid"}) -> ("new picture"=w939:picture)  [unwired: 5 in]
                n3690 = call <vilib>:"Move Pen.vi"("new position"=w983, "picture"=w939) -> ("new picture"=w982:picture)  [unwired: 3 in]
                n3691 = call <vilib>:"Draw Line.vi"("picture"=w982, "end point"=w984, "color(black)"=u32 16448250, "pen"=T1 {"Width"=3, "Style"=enum."Solid"}) -> ("new picture"=w938:picture)  [unwired: 5 in]
                n3692 = call <vilib>:"Move Pen.vi"("new position"=w971, "picture"=w938) -> ("new picture"=w970:picture)  [unwired: 3 in]
                n3693 = call <vilib>:"Draw Line.vi"("picture"=w970, "end point"=w972, "color(black)"=u32 16448250, "pen"=T1 {"Width"=3, "Style"=enum."Solid"}) -> ("new picture"=w937:picture)  [unwired: 5 in]
                n3694 = call <vilib>:"Move Pen.vi"("new position"=w949, "picture"=w937) -> ("new picture"=w948:picture)  [unwired: 3 in]
                n3695 = call <vilib>:"Draw Line.vi"("picture"=w948, "end point"=w950, "color(black)"=u32 16448250, "pen"=T1 {"Width"=3, "Style"=enum."Solid"}) -> ("new picture"=w936:picture)  [unwired: 5 in]
              }
            }
            n3696 = call <vilib>:"Draw Rectangle.vi"("picture"=w340, "rect"=T2 {"left"=620, "top"=65, "right"=625, "bottom"=70}, "fill?(F)"=TRUE, "color(black)"=u32 16448250, "pen"=T3 {"Width"=1, "Style"=enum."Solid"}) -> ("new picture"=w339:picture)  [unwired: 4 in]
          }
        }
        "2D Picture" <- w114
      }
    }
  }
